vi "UHR-Fleezers Control (host) - 10.8MV_trial4.vi"() -> ()   [LabVIEW 2012]
uses:
  <vilib>/Utility/miscctls.llb/LVPoint32TypeDef.ctl
  <vilib>/Utility/miscctls.llb/LVMinMaxIncTypeDef.ctl
  <vilib>/userdefined/High Color/nirio_resource_hc.ctl
  <vilib>/Platform/TimedLoop/XDataNode/timing_clust.ctl
  <vilib>/Platform/TimedLoop/XDataNode/nitl_modes.ctl
  <vilib>/Platform/TimedLoop/XDataNode/wakeup.ctl
  <vilib>/FPGAPlugInAG/PCIe-7852R/niLvFpga_Open_PCIe-7852R.vi
  <vilib>/FPGAPlugInAG/PCIe-7852R/niLvFpga_Reset_PCIe-7852R.vi
  <vilib>/Utility/error.llb/Error Cluster From Error Code.vi
  <vilib>/rvi/errors/niLvFpgaAdjustHostInterfaceError.vi
  <vilib>/FPGAPlugInAG/PCIe-7852R/niLvFpga_Run_PCIe-7852R.vi
  <vilib>/Analysis/baseanly.llb/Mean (DBL).vi
  <vilib>/express/express analysis/Spectral/Block/exnSpectralBlock spectral measurements PSD poly.vi
  <vilib>/express/express analysis/Spectral/Block/exnSpectralBlock spectral measurements PSD WFM.vi
  <vilib>/Waveform/WDTOps.llb/WDT Append Waveforms DBL.vi
  <vilib>/FPGAPlugInAG/PCIe-7852R/niLvFpga_Abort_PCIe-7852R.vi
  <vilib>/FPGAPlugInAG/PCIe-7852R/niLvFpga_Close_PCIe-7852R.vi
  openfpgaref.8.6.ctl
  <vilib>/Platform/TimedLoop/XDataNode/XDataNode.xnode
  <vilib>/rvi/interface/nirviOpenFPGA/nirviOpenFPGA.xnode
  FPGA Bitfiles/UHR-FleezersInst_FPGATarget_UHR-FleezersCont_0F5B06C4.lvbitx
  UHR-Fleezers Control (fpga) - 10.3.vi
  <vilib>/rvi/interface/nirviMethod/nirviMethod.xnode
  <vilib>/rvi/interface/nirviReadWriteControl/nirviReadWriteControl.xnode
  <vilib>/express/express analysis/Spectral/XNode/ExpressSpectralMeasurementsBlockNode.xnode
  <vilib>/rvi/interface/nirviCloseFPGA/nirviCloseFPGA.xnode
  <vilib>/Analysis/NI_AALBase.lvlib
  <vilib>/Platform/TimedLoop/XDataNode/XDNodeRunTimeDep.lvlib
  <vilib>/vision/NI_Vision_Development_Module.lvlib
  NiFpgaLv.dll
  <vilib>/FPGAPlugInAG/PCIe-7852R/niLvFpga_ConfigureFifo_PCIe-7852R.vi
  <vilib>/rvi/errors/niLvFpgaMergeErrorWithErrorCode.vi
  <vilib>/FPGAPlugInAG/PCIe-7852R/niLvFpga_ReadFifo_PCIe-7852R.vi
panel:
  out "Location Matrix 3":string[][](array[string])=[["N.D.\r\n", "N.D.\r\n", "N.D.\r\n"], ["0.19233\r\n", "0.00156\r\n", "0.20615\r\n"], ["N.D.\r\n", "N.D.\r\n", "N.D.\r\n"], ["N.D.\r\n", "N.D.\r\n", "N.D.\r\n"]]
  out "Location Matrix 2":string[][](array[string])=[["N.D.\r\n", "N.D.\r\n", "N.D.\r\n"], ["0.19233\r\n", "0.00156\r\n", "0.20615\r\n"], ["N.D.\r\n", "N.D.\r\n", "N.D.\r\n"], ["N.D.\r\n", "N.D.\r\n", "N.D.\r\n"]]
  out "X Motion 2":string
  out "Location path":path=path "C:/Users/cwicker/Desktop/UHR-Fleezers Instrument - Charlie/Locations.txt"
  out "Location Matrix":string[][](array[string])=[["N.D.\r\n", "N.D.\r\n", "N.D.\r\n"], ["N.D.\r\n", "N.D.\r\n", "N.D.\r\n"], ["N.D.\r\n", "N.D.\r\n", "N.D.\r\n"], ["N.D.\r\n", "N.D.\r\n", "N.D.\r\n"]]
  in  "radius":i32=10 min=1 max=20
  in  "clear markers":bool
  in  "trap\nmarkers?":bool
  in  "Sample Channel Flow":bool
  in  "Pump 3 contents":string="Bottom: ADig beads" caption="contents"
  in  "Pump 1 contents":string="Top: DNA beads" caption="contents"
  in  "Scripts":T1(tab)
  in  "Take Stepping Data":bool
  in  "Got DNA bead":bool
  in  "Got ADig bead":bool
  in  "Cap 1 Flow ON":bool=TRUE
  in  "Move Cap. 1 (DNA Top)":bool
  in  "Cal/Data Acq. Spot":bool
  in  "Dump Beads":bool
  in  "Cap 1 T ON":bool=TRUE
  in  "Cap 1 Samp Flow ON":bool=TRUE
  in  "Offset 2 Set":dbl=2.0
  in  "Offset 1 Set":dbl=1.0
  in  "Cal @ (MHz)":dbl=20.0
  in  "W/ Offset 1":bool=TRUE
  in  "Offset 1 Start (MHz)":dbl=13.0
  in  "W/ Offset 2":bool
  in  "Offset 2 Start (MHz)":dbl=16.0
  in  "Pause at Closest Delta (s)":dbl
  in  "Move to Delta 2 (MHz)":dbl=41.0
  in  "Attempt Limit":dbl=30.0 caption="Limit"
  out "Attempts":dbl=1.0
  in  "Wait Before Save (s)":u32=1
  in  "Fish for Tether":bool
  in  "Closest Delta (MHz)":dbl=13.0 step=0.25
  in  "Stop F (pN)":dbl=10.0
  in  "Then...":string(combo)="2"
  in  "Move to Delta 1 (MHz)":dbl=15.0
  in  "Tether Alarm?":bool=TRUE
  out "Tether":bool
  in  "TA Cancel Save?":bool=TRUE
  in  "TA Green Off?":bool=TRUE
  in  "Raster Set Upon Tether":u32=1
  in  "Save at end (5, 6)":bool
  in  "N Steps":dbl=20.0
  in  "Step Size (nm)":dbl=0.34
  in  "Save ave factor":dbl=1.0
  in  "Dip Trap Delta 1 (MHz)":dbl=15.0
  in  "Move Trap Before?":bool
  in  "Save Data After?":bool
  in  "Green ON After?":bool
  in  "Dip Trap Delta 2 (MHz)":dbl=15.0
  in  "Move Trap After?":bool
  in  "Duration (s)":dbl=1.0
  in  "Dip for Protein":bool
  in  "APD to Watch":bool
  out "Duration (s)":dbl
  in  "Action":string(combo)="Yank"
  in  "Fl. Triggered...":bool
  in  "Fl. Delta Thresh. (kHz)":dbl=0.6
  out "Waiting":bool
  out "Fl. High":bool
  in  "N pts to average":u16=6
  in  "Yank Delay (s)":dbl=3.5
  in  "Yank to Delta Array (MHz)":dbl[](array[numeric])=[16.3, 15.85, 14.85]
  in  "N Array El":u8=3 min=1 step=1
  in  "Random Choice":bool=TRUE
  in  "Force Yank":bool
  in  "Force Reset":bool
  in  "Y change (mm)":dbl
  in  "Profile":bool
  out "Sigma/Mean 2":dbl=nan caption="Sigma/Mean" format="%#_2g"
  out "Rate sigma (Hz) 2":dbl caption="Sigma (Hz)" format="%0.2f"
  out "APD 2 Rate (Hz)":dbl format="%#_3p"
  out "Primary Video Display":T2(plugin-control)
  out "Waveform Graph":dbl[](graph) caption="APD Line Scan"
  in  "Inject Top":bool caption="Inject Pump 3"
  in  "Inject Bottom":bool caption="Inject Pump 1"
  out "Messages":string="3:52 PM\tUHR-Fleezers ready.\r"
  in  "APD Ave N":dbl=10.0
  out "Int. Time (s)":dbl=3.0
  in  "Stop All":bool
  out "Sigma/Mean":dbl=nan format="%#_2g"
  out "Rate sigma (Hz)":dbl caption="Sigma (Hz)" format="%0.2f"
  in  "Tab Control 6":T3(tab)
  in  "APD 2 Offset":dbl
  in  "APD 1 Offset":dbl
  out "RMS (Ang)":dbl=nan format="%_2g"
  in  "Bead Sep. Int. Time (s)":dbl=5.0 caption="Int. Time (s)"
  in  "Below (kHz)":dbl=0.5
  in  "Above (kHz)":dbl=2.0
  in  "Adjust Scale\nto Mean":bool
  in  "Rescale on Mean":bool
  in  "Offset (nm)":dbl
  out "Mean":dbl=0.003832945286164026 caption="Mean (V)" format="%#_3g"
  out "Force":waveform(dbl)[](graph)=[{"t0"=timestamp(68.39999999999971 s since 1904-01-01), "dt"=0.15, "Y"=[0.006501650011455353, 0.007613704960620254], "attributes"=variant("NI_ChannelName"=variant(string "T1 X"))}, {"t0"=timestamp(68.39999999999971 s since 1904-01-01), "dt"=0.15, "Y"=[-0.0011233638669916534, -9.306230558884231e-05], "attributes"=variant("NI_ChannelName"=variant(string "T2 X"))}]
  out "APD Chart":waveform(dbl)[](graph)=[{"t0"=timestamp(68.39999999999971 s since 1904-01-01), "dt"=0.02, "Y"=[0.0, 0.0, 0.0, 0.0, 0.0, 0.0, 0.0, 0.0, 0.0, 0.0, 0.0, 0.0, 0.0, 0.0, 0.0], "attributes"=variant("NI_ChannelName"=variant(string "APD 1"))}, {"t0"=timestamp(68.39999999999971 s since 1904-01-01), "dt"=0.02, "Y"=[0.0, 0.0, 0.0, 0.0, 0.0, 0.0, 0.0, 0.0, 0.0, 0.0, 0.0, 0.0, 0.0, 0.0, 0.0], "attributes"=variant("NI_ChannelName"=variant(string "APD 2"))}]
  in  "Calibration":u16(ring) items=["None", "Position", "Force"]
  out "T1 X":dbl=0.007057677486037804 caption="T1 X (V)" format="%0.2f"
  out "T2 X":dbl=-0.0006082130862902479 caption="T2 X (V)" format="%0.2f"
  out "Bead Separation":waveform(dbl)(graph)={"t0"=timestamp(68.39999999999971 s since 1904-01-01), "dt"=0.15, "Y"=[nan, nan], "attributes"=variant("NI_ChannelName"=variant(string "T1 X"))}
  in  "Amplitude (nm)":dbl=3.0
  out "Bead Mean (nm)":dbl=nan caption="Mean (nm)" format="%0.2f"
  out "Difference":dbl=0.006449464399747556 caption="Difference (V)" format="%.2g"
  in  "Take Detection Laser\nImage":bool
  out "APD 2":T2(plugin-control) caption="APD 2 (Cy5)"
  in  "Flip Green Filter":bool
  in  "Set X Only":bool
  in  "Set Y Only":bool
  out "APD 1":T2(plugin-control) caption="APD 1 (Cy3)"
  out "Detection Laser Y":T2(plugin-control)
  out "Pointer Y (V)":dbl format="%_3g"
  out "Pointer X (V)":dbl format="%_3g"
  in  "Set Confocal Spot (X-Y)":bool
  out "Detection Laser X":T2(plugin-control)
  out "Saved APD":dbl[][](graph) caption="Most Recent Time Trace"
  out "Trap Delta Graph":dbl[](graph) caption="Most Recent Time Trace"
  out "Save APD Deriv":dbl[][](graph) caption="Most Recent Time Trace"
  out "Delta Fl. 1":dbl
  out "Delta Fl. 2":dbl
  out "All Signals":waveform(dbl)[](graph)=[{"t0"=timestamp(68.39999999999971 s since 1904-01-01), "dt"=0.02, "Y"=[0.0, 0.0, 0.0, 0.0, 0.0, 0.0, 0.0, 0.0, 0.0, 0.0, 0.0, 0.0, 0.0, 0.0, 0.0], "attributes"=variant("NI_ChannelName"=variant(string "APD 1"))}, {"t0"=timestamp(68.39999999999971 s since 1904-01-01), "dt"=0.02, "Y"=[0.0, 0.0, 0.0, 0.0, 0.0, 0.0, 0.0, 0.0, 0.0, 0.0, 0.0, 0.0, 0.0, 0.0, 0.0], "attributes"=variant("NI_ChannelName"=variant(string "APD 2"))}, {"t0"=timestamp(68.39999999999971 s since 1904-01-01), "dt"=0.15, "Y"=[-0.02616851084212992, -0.0255133251155073], "attributes"=variant("NI_ChannelName"=variant(string "T1 Y"))}, {"t0"=timestamp(68.39999999999971 s since 1904-01-01), "dt"=0.15, "Y"=[0.006501650011455353, 0.007613704960620254], "attributes"=variant("NI_ChannelName"=variant(string "T1 X"))}, {"t0"=timestamp(68.39999999999971 s since 1904-01-01), "dt"=0.15, "Y"=[5.238432721945855, 5.23694863734855], "attributes"=variant("NI_ChannelName"=variant(string "T1 Sum"))}, {"t0"=timestamp(68.39999999999971 s since 1904-01-01), "dt"=0.15, "Y"=[-0.011935220655057682, -0.011271872990085285], "attributes"=variant("NI_ChannelName"=variant(string "T2 Y"))}, {"t0"=timestamp(68.39999999999971 s since 1904-01-01), "dt"=0.15, "Y"=[-0.0011233638669916534, -9.306230558884231e-05], "attributes"=variant("NI_ChannelName"=variant(string "T2 X"))}, {"t0"=timestamp(68.39999999999971 s since 1904-01-01), "dt"=0.15, "Y"=[5.494853022858362, 5.494846064638206], "attributes"=variant("NI_ChannelName"=variant(string "T2 Sum"))}, {"t0"=timestamp(68.39999999999971 s since 1904-01-01), "dt"=0.15, "Y"=[0.28818490745989345, 0.2884769879609513], "attributes"=variant("NI_ChannelName"=variant(string "T1 FB X"))}, {"t0"=timestamp(68.39999999999971 s since 1904-01-01), "dt"=0.15, "Y"=[1.7389615771965699, 1.7392489089632854], "attributes"=variant("NI_ChannelName"=variant(string "T2 FB Sum"))}, {"t0"=timestamp(68.39999999999971 s since 1904-01-01), "dt"=0.15, "Y"=[0.33831454944946326, 0.3385055215953781], "attributes"=variant("NI_ChannelName"=variant(string "T2 FB X"))}, {"t0"=timestamp(68.39999999999971 s since 1904-01-01), "dt"=0.15, "Y"=[2.000203253273112, 2.000828547013765], "attributes"=variant("NI_ChannelName"=variant(string "T2 FB Sum"))}, {"t0"=timestamp(68.39999999999971 s since 1904-01-01), "dt"=0.15, "Y"=[-10.000305185094591, -10.000305185094591], "attributes"=variant("NI_ChannelName"=variant(string "PSD Y"))}, {"t0"=timestamp(68.39999999999971 s since 1904-01-01), "dt"=0.15, "Y"=[-10.000305185094591, -10.000305185094591], "attributes"=variant("NI_ChannelName"=variant(string "PSD X"))}, {"t0"=timestamp(68.39999999999971 s since 1904-01-01), "dt"=0.15, "Y"=[-0.0074939725943783285, -0.007506576738791921], "attributes"=variant("NI_ChannelName"=variant(string "PSD Sum"))}]
  in  "Signals to Plot":i32(listbox)
  out "Trap Disp. Freq. (Hz)":dbl=6.666666666666667 caption="Freq. (Hz)" format="%#_6p"
  out "Display Period (s)":dbl=0.15 caption="Period (s)" format="%#_6p"
  in  "Trap Disp. Downsample":dbl=10000.0 caption="Downsample" max=20000.0
  in  "APD Disp. Scale":dbl=0.1 caption="Scale (Divide,\nfor above plot only)"
  in  "APD Disp. Downsample":dbl=2.0 caption="Integrate" min=1.0 max=30.0 step=1.0
  out "APD Display Freq. (Hz)":dbl=50.0 caption="Freq. (Hz)"
  out "APD Display Period (s)":dbl=0.02 caption="Period (s)"
  out "FFT 1":cluster{"f0":dbl, "df":dbl, "magnitude":dbl[]}[](graph)=[{"f0"=0.0, "df"=16.666666666666668, "magnitude"=[-331.1367572010275, -79.05506245821404, -86.61411242440559, -88.4728176091699, -90.3181253945935, -94.12566333707997, -92.52740723119955, -94.92192587982518, -99.60936585245742, -96.87568627870715, -94.02570383337763, -83.8058550151726, -97.57441397235512, -101.59968530846606, -101.523049255742, -103.35038532190343, -101.58594091014982, -102.96098031851216, -91.39759462745924, -103.75019963279499, -104.45030075054324, -103.04245334279298, -104.0720279134107, -106.06482372394834, -103.69131867828104, -104.40395035115309, -105.96420043276396, -107.6735556337804, -106.673030006608, -107.34889066208132, -108.05626565233933, -106.25659018850432, -105.29934513380842, -105.43096056709592, -108.3728498841465, -106.0555440144992, -105.78001282181421, -107.48741857324953, -108.67624970548897, -105.39976667156175, -105.91413119232612, -109.4222808198164, -107.0898971593174, -107.91164191890915, -108.26032038855709, -107.58332347164534, -108.23559688234297, -108.01271040303237, -107.66511723652701, -106.51901583170391, -109.27249501469946, -108.55647681594805, -107.93499259231463, -107.05068166453935, -109.13641475410455, -109.29679733781423, -108.19360835527803, -109.57747591546632, -109.58364591011674, -110.47061433372711, -109.8144340420426, -108.79067462293897, -107.54887553357234, -107.99559866705923, -108.85023923652685, -109.68733225238618, -108.51101278437793, -108.51620475114115, -108.22212402200637, -104.63726950302143, -110.2989919678048, -107.61796444414897, -108.68882962798736, -104.79193983043893, -103.59504263746938, -93.64633660288543, -101.9191640501395, -105.73717393151816, -108.92572458793902, -107.43962662800902, -107.79595323081325, -107.0923101993207, -108.17603277205289, -107.87074270713183, -109.20899066381877, -108.61832060412445, -109.10072003106593, -105.76480632823524, -108.60877649218978, -109.67541158970121, -110.2286232768028, -109.84952155309578, -109.33772024076384, -109.95251642394683, -110.14777282585466, -109.13825677905699, -110.05989365698167, -109.39359990189426, -110.56255614635295, -109.66477183197163, -108.9397158528824, -110.26529907650465, -109.20049464984628, -108.20183857013548, -109.09752250184418, -108.00440442238454, -108.35465963524055, -111.16774134451799, -110.34812550238405, -108.94506763426756, -108.72845542102493, -109.41512344014713, -112.44661664432377, -110.35437330889101, -111.32939440655925, -109.42989530434981, -110.98084669076195, -111.92160561143541, -108.57755551751093, -111.40042616180912, -110.15284955891853, -112.21455132279115, -111.40787773511747, -108.82949641635288, -110.13442122547907, -111.42229298204664, -112.06314940885191, -110.6015308813694, -109.51144097251623, -111.15989713761475, -110.25535755335385, -109.65868178057926, -110.51649885452997, -109.77194745285269, -108.4234206864394, -109.50892632093968, -109.46471287444389, -107.92241289271415, -109.72283805386196, -108.63426821579918, -110.37316681536255, -111.09713996884652, -110.32903619589223, -105.32012665515045, -107.36858557554393, -108.00382215905725, -110.06430686942338, -108.81666625979916, -110.01277074453823, -110.94194741225512, -109.65934609082873, -107.80979136006962, -112.81333866824724, -111.61474300955487, -109.83998277184975, -109.45953946904639, -109.79640584952526, -108.19172301667324, -109.28894656674316, -107.61471301278785, -108.83814006090513, -109.08866847726084, -108.20250571862371, -107.96222236861584, -107.03811197900873, -108.93533000393974, -107.74482548035408, -110.79811544577694, -111.1387476496877, -107.42970105883512, -109.18442281176472, -108.73546184641192, -108.71800246690864, -108.51945944378063, -108.06825856571285, -107.27210712368412, -108.12304695877637, -107.84933283677306, -109.73682373154998, -109.32284761503395, -109.31328817453769, -106.68762108642842, -109.79203616876461, -109.9020278896408, -110.27080024357275, -108.54152101558762, -111.00464391726017, -112.42244020766577, -110.82707315747889, -111.00344011890857, -109.90461839395674, -109.42877207451863, -109.73549298167016, -111.67494793393293, -108.85799077901427, -108.5348443278263, -109.803781083881, -108.30644755543659, -108.5079527456017, -111.2055351312823, -108.53089994340155, -108.01739789012176, -108.70360662855235, -107.95873456794631, -109.58297170693093, -108.9372401694271, -110.15921663527153, -109.22399119911955, -110.89883651739237, -108.92840112258382, -110.0545300523626, -109.05961065387005, -109.45831398589371, -108.61239387653227, -110.13001256174265, -108.80060224137931, -109.46327400696283, -108.0177965824709, -109.29727944627197, -110.3237255895986, -109.03258262543821, -110.97880178489321, -109.70034895077919, -111.16405638194153, -109.17324451464711, -109.65698250854277, -108.96750235822178, -112.00534231585624, -108.69274607723942, -108.98110446396657, -108.40723795464795, -111.44459094807324, -111.74799245277113, -111.1601960491512, -108.92048232753773, -110.30506377784799, -111.33145973979093, -110.91850998672503, -110.33684985776448, -108.90206518366908, -109.28458878227542, -108.98773986023751, -110.85813863075646, -109.00041591105906, -110.84543686681204, -109.84382395806176, -109.69722434763266, -108.50915601095721, -107.80829925826895, -110.59736107582401, -109.75377770317087, -109.3992084496136, -110.51151565846742, -112.49753959826434, -109.7299632589479, -109.54070743868353, -109.90314341132164, -111.05974202976806, -109.03766862152392, -109.46667095459878, -109.52800799036197, -111.3163121356807, -110.07817134522178, -108.69251657453547, -109.40472158898045, -109.71400709815576, -110.60534468715097, -109.46937396724682, -107.70342491418788, -109.86331122597839, -108.64971387994616, -110.90117371097081, -108.34928840565928, -110.04172889660904, -111.52979926554961, -110.34759300823305, -109.62712781837159, -109.24131154553284, -110.23196152450447, -108.68509612326807, -108.0246905483419, -106.61876139289784, -101.5519630114271, -80.57695480953835, -102.03744443354402, -107.1449217193017, -110.0695213407169, -106.61597783999268, -110.79221011808191, -109.58974545931426, -109.1149802216988, -109.20993813088597, -109.63768480465863, -110.10428394219181, -109.08445084271477, -108.83472375362581, -109.69508502050168, -108.05588796178941, -110.62586360101581, -109.95315261676905, -107.52208264977473, -108.80708007514875, -110.43484881098874, -110.45942171588936, -107.83804717866751, -109.98973910294193, -109.3496496054193, -108.425252911127, -110.94579264380809, -108.54181722177951, -108.67696070083541, -108.4150202151644, -109.24973583101504, -112.0454922608961, -111.29046597340738, -110.75018248960077, -109.38326363603683, -109.2033340336957, -109.45076170874889, -109.52878049853727, -109.32340869724774, -110.98123395128233, -110.75736340635505, -109.7218385823809, -107.97422606064993, -109.77313701758703, -110.95948744392717, -110.08996774172691, -108.51011830110778, -109.78063140243836, -110.65996628628228, -109.83684298615616, -110.33329049188029, -110.13755118968292, -110.3717925645783, -108.55302219178951, -106.86811628734195, -108.6302156589162, -108.75341391045045, -108.32589578384841, -108.70061474734084, -112.30742263527534, -109.16842570592085, -109.29767035534508, -108.87829025017463, -108.2255616391397, -108.4316108616088, -108.82995906929271, -110.40135575415563, -109.51623498946435, -109.79409808792403, -107.03832759632121, -108.36534528684132, -109.72010868372905, -107.90933028179892, -106.95643597294047, -111.29929166165778, -110.23001135794706, -108.98838015381585, -109.79115357104436, -108.18627479511115, -108.14988122174307, -109.12074063466532, -109.41904850488358, -111.40409873721113, -108.83156790193294, -108.77032248953847, -108.88363158686694, -108.47515048290681, -105.94172147874599, -109.38146940214403, -109.21277078848794, -108.11309390545507, -110.70840012427504, -109.5504457849329, -109.52330684534209, -110.06776026911132, -108.21949434182314, -111.21266686269992, -108.78581501170974, -108.43115799297222, -109.63260325780062, -109.84070220619535, -109.72041980780126, -110.29615941882527, -110.60316734262464, -108.79165446414692, -110.95840439895592, -109.64926233107009, -109.16526769544322, -108.65292362430982, -109.56113898129935, -109.85693046339026, -108.92316027325207, -109.79492493553914, -109.38157962945887, -110.24545136266825, -109.30031463492487, -109.0795429936869, -111.4091719525013, -108.63499083917162, -108.43863465339358, -109.23207864880891, -111.21947487191643, -109.24525201480154, -109.56842406077318, -109.46711940800672, -111.91389548262572, -108.15655736690546, -108.71882059966947, -111.26328503478568, -110.95027143873176, -108.4853106242357, -110.36902802777546, -109.9314203579182, -108.77686164101732, -108.71871020068312, -111.04829661168574, -109.95072655339462, -109.88221342875462, -109.53241732756136, -108.2625005404823, -108.00677030040697, -110.19659317581693, -108.93858924796267, -109.46817875483995, -110.78063992017232, -111.11066570318451, -110.78774336696706, -109.19199744617812, -108.54914256407436, -109.28414960420909, -110.64143585101183, -110.5855350821307, -109.47578632252726, -108.89705360836223, -109.89214013612292, -107.93271261027171, -109.32631601340563, -108.60274611341092, -109.40110159872573, -110.889237682208, -110.01391165813328, -109.99747108785071, -108.65542819213674, -110.37211847668736, -110.44656500845738, -110.8128133834973, -108.8909299260433, -110.19551227077532, -111.37647266643523, -110.83802189730321, -109.98519377913681, -110.52378970770522, -108.16970420057817, -110.70974729773344, -110.76836765494402, -110.26884275594577, -109.22041044268806, -109.87809744746195, -107.76823252107832, -109.12119474042969, -110.28066108731146, -108.55000033509207, -110.18152097767907, -110.73030521152278, -111.49470908029893, -110.2320929919509, -110.03370979233021, -109.79181668155233, -108.6673501209991, -109.86695766650877, -107.88926518046961, -110.95525003776572, -109.18130359755742, -110.42618009658618, -107.90341931158893, -111.44736855661769, -110.72634267386593, -109.29945988519303, -107.67889101961411, -108.81148059987765, -109.13375212757057, -109.8122873383549, -109.80176697684155, -109.96342275204768, -109.90406635707086, -108.75674342748256, -110.12362902701081, -109.82151095527837, -108.62543344241836, -110.09171852771195, -110.21434637862887, -109.97254504855631, -109.27043209093468, -111.35149588204125, -110.12399876776051, -111.65983675538546, -109.28788875768564, -110.86554069990251, -111.26990906470603, -108.60956517491746, -111.49613890850938, -111.79685722966795, -109.26269485364045, -110.38555615546439, -109.40641023162068, -110.966136593156, -108.78892524584494, -110.29340727375603, -111.44032043281035, -109.95212021173755, -109.79233511584334, -112.41184021118175, -109.73687851881148, -108.65493879781806, -110.76132988919045, -108.43230346094671, -110.32968175895853, -110.29890782023821, -108.77609076424456, -110.3298662333555, -109.47734504217333, -108.2677295732245, -109.21234363352882, -107.83278941978479, -108.85136784424789, -108.43241251530755, -109.76609391460555, -108.53204373005357, -110.9660641972934, -110.3152512161094, -110.72570499399905, -109.23877906286317, -111.72407743101837, -109.20311421918561, -108.06021800233717, -109.29288625761943, -108.78395253409145, -111.85250172876302, -108.78827588901797, -109.79775055719482, -109.12089297455859, -109.49896359356035, -110.34432647103819, -107.94700097960238, -109.30489238477631, -108.89170290869342, -108.82574563272509, -110.11024077194833, -107.37946433552314, -109.60167933458756, -107.80625057819019, -110.11489057210264, -107.35436859378505, -105.69819484613895, -109.11280625683739, -109.27770293057978, -107.7053735252589, -109.75022444894368, -109.3310543596577, -107.87683693707739, -108.19931495338068, -109.26462246191564, -106.71885779297867, -100.00018022217961, -92.54434511397295, -107.20472143807373, -107.39203415155283, -110.04461177268398, -108.48860496315312, -109.0057168110333, -108.37627790492552, -108.4108380728248, -109.65509454313073, -109.64243000632982, -97.04219069306761, -109.0928856629964, -107.9760697315632, -107.52611064047497, -108.87702814778996, -109.08437599027614, -110.70097118837974, -109.00969860961283, -110.38275386163214, -110.0699155421545, -106.91498895181175, -106.22178738309017, -109.36827866896039, -107.59953130968307, -109.19516217272808, -108.31502495393616, -109.384158926223, -107.11670654202719, -108.09436312738853, -110.14559230873704, -109.84997663447679, -107.83465335309926, -108.60947100624459, -108.9932479423645, -109.17174810371898, -108.79457339828916, -109.40909327982367, -109.6328723628302, -109.51081854476179, -107.63054408568418, -109.63728404010122, -108.51163794839918, -107.55002282725216, -108.97796212764939, -107.24648164623483, -112.21470452291085, -108.74294024554423, -109.62070777514892, -108.05768666239368, -109.8224946685739, -109.34575507446003, -108.53536952609525, -109.60789300457671, -107.56681538208278, -109.22777325016398, -108.79047910308894, -110.10332477250668, -108.00206387955672, -108.45604004720035, -109.00645795765472, -109.81039564269616, -108.92785144634745, -108.3978471520567, -107.94411095685999, -110.53486519304262, -108.8773780319227, -109.03345093296107, -107.30746693745031, -108.54277704832029, -108.77629108166091, -108.91111762599647, -107.74965195880401, -109.97375370738439, -109.76326492689246, -107.91717581777407, -109.0730556927617, -107.66804873204664, -110.40438871064791, -108.05794247751498, -108.80206615156494, -107.51329354700796, -108.83687012994949, -107.57713176895379, -107.94774159581414, -109.41894615439651, -107.10869425078764, -110.51480854078629, -108.92221367099775, -109.91358786461535, -110.1744263092835, -109.30795472883494, -107.91359710691006, -109.77888185049835, -109.52060975706438, -108.66686651982212, -108.71041801553639, -110.13619546359467, -108.87957097273856, -109.72150387215271, -109.00776068810654, -109.70251113927438, -110.75769213896399, -108.53234896741436, -109.69439526582246, -110.15412541604617, -108.25183374628219, -107.97402569656481, -110.34920156998648, -108.45106995186384, -108.82031145748209, -111.38690005057539, -107.01968459818563, -110.3044500039584, -110.8755481852125, -111.08915057663255, -107.94824988655199, -110.21669144934839, -109.90539774633154, -109.58985438756767, -110.12258796623348, -109.41689951612143, -109.31128210476795, -109.00258476567323, -109.11093063041056, -108.83347064311234, -108.32685287566952, -109.44770946560935, -108.40145063144861, -109.68448193892085, -108.76525439243828, -107.62837139034596, -107.39300298848994, -109.36993934990318, -109.2465218489418, -106.66307369796812, -110.15891092764934, -109.57151745419041, -108.92425698310808, -109.8036704717834, -108.79751146756549, -109.25926431818017, -108.46260574057584, -109.1967554647261, -110.63319560262356, -109.02343067385144, -111.22073171487528, -109.4731095097105, -109.69335000085164, -109.48782989577005, -107.95204227683271, -108.19468255763758, -111.36195112053247, -109.55696116543685, -110.3130767640534, -108.9621824253354, -109.99735074896789, -109.20198058456344, -108.12100614259485, -111.27227490807289, -110.09248554008288, -109.14395535060149, -110.80882692379708, -109.22632926901655, -108.64497210802793, -111.00030482190711, -111.1317849358033, -107.43140429257826, -107.9783302193555, -109.2639893652291, -108.97008485446163, -108.66556668859064, -108.12995785876932, -109.73001061107855, -108.09691302413727, -110.68391499215569, -112.78583642012705, -108.7093037763389, -110.67868795924797, -109.0190959349128, -108.36247198231372, -109.82829353258869, -108.24916379311045, -109.84154533905823, -108.55470160833775, -109.75438989348815, -108.82865632118325, -107.63622268162582, -111.00943492886312, -110.81824358463759, -109.46028423652966, -107.52479398900992, -108.99087806823736, -109.94494831750349, -110.26788355564504, -109.8954055022304, -106.9478122391182, -108.91705388158901, -107.76095584490312, -109.28456723055147, -109.7982307261767, -108.98552661346622, -109.98937979783426, -110.57907422426224, -108.68113463944836, -108.06257240208589, -110.0707224529617, -109.19515280354733, -109.35868842818849, -110.37311467065695, -109.0404734478992, -108.16686395270187, -108.61859220485148, -109.19986437876149, -108.19707189725302, -110.06564239663074, -108.87850403465154, -110.63824157544798, -107.36918104067212, -108.7008736325543, -110.9359398265406, -111.08529123080929, -108.44209934821818, -109.79529621208783, -108.38917887958179, -108.169117639508, -109.24332926356216, -110.50584058811704, -109.63592524002665, -109.32261039377495, -109.16720880524552, -109.3084314664462, -109.5812223978583, -107.70213196487856, -108.0557884982431, -110.67058020007828, -111.68459781023608, -109.66270627185824, -110.52536245663693, -109.70208409132103, -108.78645420809342, -109.23122088059863, -109.24601474121832, -111.25604763816514, -109.50225851581177, -107.32434217163818, -109.28548556764925, -107.59972621660836, -110.46928774723048, -109.25950101547609, -110.32016453935465, -107.78482761561703, -107.89462895091089, -107.51366154391481, -108.08036891159172, -109.53371809947035, -101.2452927166745, -109.32763325689056, -107.52166868423687, -109.89648659445174, -109.11350200980485, -109.81336712738089, -110.02799517445062, -108.02767143538516, -107.97850220501483, -109.50772934896838, -109.31069875721964, -108.49991657749598, -105.60880911233095, -109.79128597340213, -106.91084537903113, -107.84880087118997, -109.63628170511824, -109.03203967193224, -110.64186113413658, -110.98027990365594, -112.33841002907062, -111.01793075565425, -108.58025797022215, -110.4259296883756, -110.38643255981424, -108.93051671115133, -110.97544177116494, -108.63883100482677, -108.37581711765226, -108.90240163126536, -107.94688047875466, -109.9482937437732, -110.09097112364414, -110.09805032265376, -111.44307114024532, -109.15483789122554, -110.9713708217832, -107.8548737634672, -111.41418477109195, -109.45699779859628, -97.03595099331734, -109.16746744169623, -109.66209204485918, -112.57048704774604, -109.73989735035725, -108.16252575067017, -110.7546980664636, -108.91536673403449, -109.20509151422344, -111.0260632167785, -109.62924582406518, -110.45466277291722, -110.2973970018937, -109.67550222925419, -108.84481022020094, -107.23686414357573, -111.79004633370906, -109.85453094194085, -109.45617270081004, -110.73920606732504, -108.90879956851099, -109.67774425528265, -109.4745715721361, -110.18080454693559, -109.26079184315502, -109.41692499885505, -109.02240975088358, -107.80833423058168, -109.32657361431549, -107.87138278655101, -110.910364670719, -109.70067156846706, -108.55301754282077, -109.4243252157005, -109.77567725161107, -107.83737232063925, -110.36509412773016, -109.6371048811367, -109.49430894422814, -108.55509251499753, -108.03996302911446, -110.4385715838736, -110.08864436068788, -109.48922484379962, -109.90865554258562, -109.7491963238264, -110.04796094537969, -107.413043439116, -108.54229076126079, -108.2522516728666, -109.75464941327974, -110.26795832300996, -109.28073673851144, -108.62990200974927, -109.89408067552287, -109.09160284731726, -109.90740624925795, -109.92534708896517, -109.79578862362752, -109.97278346890566, -107.80679350393824, -112.81728446281548, -108.09689504419987, -109.89549991422173, -108.43930976031248, -109.95153099843282, -108.18277483720716, -111.89607792605433, -109.52567003805, -109.17125106979698, -109.64300739407085, -108.21045178846524, -109.64036472149706, -109.02324448538845, -109.039163008889, -110.41006510134076, -109.50289952116489, -110.4732620447796, -110.08777181504614, -110.15589511434341, -109.55705089158471, -109.2547682932589, -110.86823885471617, -109.96330502176939, -109.85995369810554, -110.63211290903473, -112.08007783432191, -110.24725218052279, -107.62861148917592, -110.08691795849435, -108.89793794632287, -111.07702220466341, -109.46946126482341, -109.19747345337464, -110.70018609416007, -109.66366205691908, -110.78032312133551, -108.05724200456513, -108.195661625627, -110.90724508408255, -110.08307674771669, -110.76863516643007, -110.46620425061583, -109.16986788877276, -109.61921294239114, -108.51159432329543, -109.96308336765689, -107.38178944242856, -111.95930944846394, -109.3329826827624, -109.59119636368249, -108.83148571828912, -110.46194288788257, -105.87694286145472, -107.985886302892, -109.2975019660806, -111.05138725716857, -109.60005889204612, -110.92871351729086, -110.73480546964537, -108.41587420326718, -109.84275465824477, -108.8249071047676, -107.65358887817105, -108.3254150042995, -111.47362100321767, -112.7287536850025, -108.8217125660507, -109.50232320231771, -110.29587061625348, -109.30644535112089, -107.69178032077258, -110.84522325672016, -109.3735891463141, -109.12506388923123, -109.65582307934665, -111.11427272192576, -112.19827973435466, -109.11306367925813, -108.19203577968261, -107.89831568266465, -108.85805249169313, -109.51100049661844, -111.71546684086955, -109.53880495724334, -107.07739286222231, -110.66836728754211, -111.5415170557177, -110.16051267940297, -110.6107546662698, -111.36389129556191, -107.77888179117923, -110.34160392509817, -109.61287125994414, -110.23791773883013, -111.00669159903549, -110.97165069538953, -109.43965413392434, -110.6813161690388, -110.31441293654314, -111.96129906273796, -108.15998218707462, -110.08095912053633, -109.41084567452768, -109.28774416263552, -110.80159950384204, -110.41956747809755, -108.85005186267244, -107.9069227847757, -108.84249369063123, -109.92569208845894, -109.34109797584448, -109.41334788055491, -108.76462023086997, -108.22069272136177, -107.0786679601274, -108.30206755098202, -108.57613406368954, -110.83330887636482, -111.93966942736989, -109.76373713473264, -108.25782074884941, -108.16490627215555, -109.93351470267982, -110.75525684428368, -108.22814762283093, -109.73442331991602, -107.53145627482685, -108.27195221226805, -110.33032779278457, -109.48951857415828, -108.12599093700939, -107.97627415508097, -108.81426859968796, -111.21764717894752, -109.80856212352333, -110.92658779118501, -109.71551885834796, -110.38682741010847, -108.87671328341361, -109.68368600774755, -108.35359806351899, -111.7519400010676, -109.89407081573103, -108.24301180922755, -110.00646944788126, -108.6685299083706, -107.52856885980722, -111.7622363038509, -111.0025144494897, -108.64719599357296, -110.62968467177518, -108.821509935539, -107.94915453463719, -111.53070432277694, -109.87282048586256, -110.71167589371663, -109.79225006081626, -109.96203471712074, -110.29921092232489, -110.10644439440416, -111.28815007382043, -111.19165661703703, -108.46024117100558, -110.22528296512183, -110.32184972386672, -110.05120383416072, -109.78792549362107, -109.00355659956696, -108.85989369286315, -113.00899556732638, -110.91756826567867, -111.25016866167897, -111.84225040552181, -110.54451635944174, -110.72722829912917, -109.60759702177283, -110.49362602516815, -108.74419542915284, -110.3379671069179, -109.66259088220754, -110.45956400953156, -109.13956157147233, -109.27130155486806, -110.83015602667983, -109.17970724944131, -109.09662765889193, -108.0447366108107, -108.9536269357457, -110.35663108940085, -108.73418835472056, -113.42965806805827, -111.81270536656905, -110.06155590173537, -108.76582224646269, -106.7488061675813, -108.5700320158723, -111.11038264410035, -110.41435767488723, -109.12763443489911, -109.30517580756394, -111.61251165371237, -109.8116632664339, -109.36845864976851, -109.00390009629231, -110.54359197165573, -109.52629258465976, -110.75932197632896, -109.50903215359567, -107.42652056246085, -107.81146496533543, -103.22224383145215, -108.53803076819163, -109.78623360072066, -109.66306634612869, -110.80245829141279, -111.87835085452016, -102.27372781471168, -111.27763038431458, -108.45838423437681, -108.79077917058028, -109.31951755762685, -110.05415097017186, -109.5535934823387, -111.62732254641111, -110.73478247119641, -109.9468722686683, -110.39698367573979, -109.30612942398305, -109.7578384694043, -109.34817295524313, -105.56944757301993, -110.1940418750125, -109.27076023513962, -111.03491935225027, -112.2980497521063, -110.65725497955563, -109.0567530102422, -110.31700596563523, -109.64508026365678, -109.6190471404421, -110.52566833759428, -109.68595899227789, -109.7431160985074, -110.4798230300751, -109.45506977604765, -110.69504157940786, -110.63067849573177, -108.06456949500138, -107.99354148885966, -108.11349194720599, -109.15944121207349, -110.61766925164031, -110.14145801314527, -110.67420842201165, -111.91532881806512, -112.15901550030345, -109.94774413630104, -109.2819568305201, -110.94623189179737, -110.17685430287735, -110.39082916961016, -109.53953238698966, -110.76940623620611, -109.89327922318515, -109.10275695043765, -110.21445972656734, -110.58968777252528, -110.57016757660259, -109.59208496373341, -109.07946946465374, -109.10762003745964, -110.36892993974607, -109.81864495218393, -112.12972189864566, -109.26185849434863, -111.56305819991357, -111.36019621828058, -110.3397604159226, -109.58675612753163, -110.58041217474447, -106.34739062044932, -108.6722699609389, -110.03906060709869, -109.16794717548382, -109.65012481802809, -109.35377624077988, -110.51889143862303, -110.03397458059777, -110.7981307056636, -110.56653507062292, -107.61367005067231, -109.99279736988825, -111.79875182878175, -108.60382315996031, -109.71381533228038, -108.60388131505613, -107.0933685540362, -107.86037690830757, -108.40980028847238, -108.83869602763895, -110.76921375395764, -109.96766364716046, -110.8256171465781, -110.13805084291067, -108.5349140035878, -110.57158437465219, -110.8920694413417, -108.71646695477324, -108.33274238445665, -108.96152108305608, -111.03750932994224, -109.48915027983756, -110.29725207211165, -110.79527247268442, -109.47969936716117, -109.79306701834035, -110.16840035577498, -110.29840230783668, -109.15306387075587, -110.72651274964761, -109.08881658764956, -110.8349724030761, -110.64653625576447, -111.40392562616867, -109.94581588927414, -108.85136340231294, -109.77228546607624, -111.48297395390018, -109.7334001251941, -109.30537415590783, -109.63937411233408, -109.69785848648013, -109.3523781030017, -112.04667421182404, -111.56311816195343, -108.18548447362308, -110.63388993686104, -111.39768634137992, -109.87157345395542, -108.6734208287271, -109.46213300216168, -111.75774769437145, -110.10245994173216, -109.52385139033495, -110.96513097775451, -111.8709319163154, -111.54948269614047, -110.29760900080463, -108.52168175904663, -111.09033925738258, -111.14752744054172, -108.83074523709202, -109.05704141259113, -111.74377805749482, -109.57200906899736, -108.84121318623825, -110.86657990204343, -109.54363603755047, -110.89448416316372, -109.58965570570145, -110.21012263847972, -110.4063470702923, -109.5021950342969, -110.33648801598177, -110.90551031296536, -109.69205870504638, -109.8648503154861, -110.28183391384131, -109.65970942950766, -108.43615680946908, -111.11790511866548, -110.89043476451553, -113.64898442872548, -113.08004494963895, -110.81525412051718, -113.91009875719509, -110.95802128672312, -110.40944585634135, -110.33464695414992, -109.98984645778987, -110.18795067005652, -110.62364351231234, -110.44029833291248, -109.01598585569788, -110.95430216511514, -109.77987141110621, -108.54452361812068, -111.41780266439777, -110.47172771858405, -109.06084635984516, -109.30794593246578, -108.8764083815745, -108.18222749506985, -110.31330487887435, -109.04176821738014, -108.8558386035048, -109.47888284507395, -110.01459604573937, -110.48596659065309, -112.6781342298378, -109.85522803775775, -109.0569534499285, -109.08991286548698, -110.89485727880403, -109.18715778948663, -111.50381433568144, -111.3545424730884, -110.07710926239977, -111.99977850157067, -109.47444853853723, -109.81605328527645, -110.74995213151195, -112.56834665925544, -108.52052472391404, -110.89121213995557, -112.02004142355113, -108.66413739656008, -111.10053848695652, -110.41241079991636, -111.80152991764473, -110.21746151515111, -110.63265128607344, -109.483042128511, -112.78639954059729, -109.47114195846122, -109.23309637902875, -108.97133643967169, -110.08909147812822, -111.01105271457081, -111.18602432128249, -110.04633990216801, -109.53453538673071, -108.81939452082017, -111.13486114285661, -111.65877073200598, -111.63763706753498, -112.14107810664572, -113.6231865196724, -109.31743865878806, -109.18551713085722, -108.74951309653638, -109.28206426212142, -112.36687029711229, -110.10933061193728, -111.29501093502684, -108.19021080564794, -109.34497312126749, -110.37228033937312, -108.63277512903049, -110.61033993911002, -111.2975761598062, -111.49780004751436, -109.91019436685814, -109.32789992989028, -111.4482538110117, -110.1538439123475, -110.66347034043578, -110.05055133068794, -108.53002033538341, -111.7522199783972, -113.49108651193104, -108.03793940563418, -110.07108694011555, -110.83958739865201, -109.62805629409038, -112.69637731014087, -109.57996950503268, -110.104850643722, -108.83376203949506, -108.69400304840181, -110.59434352922563, -110.69121011800921, -110.18694553784364, -111.90598571547098, -110.30230802494223, -109.66810649416752, -112.6017099000434, -111.00296745333219, -110.64462650261785, -111.4775358707403, -111.98753241268494, -112.26574909791167, -112.04796822399412, -110.65853064447325, -109.6623218025264, -109.40559579075378, -110.42174451813142, -109.18991987957241, -111.02050178263048, -112.77950487440032, -110.42443751566815, -111.35440372400903, -108.5263524245987, -105.07498063939795, -107.15444425741984, -110.4508720018025, -110.25163264819463, -111.1383261104107, -109.91171620173931, -110.52200560606038, -110.5299174299573, -109.34628087255733, -110.26101817411786, -109.65071853372183, -109.66953335961068, -110.83590602054682, -110.980546313788, -109.4110066989163, -111.47223607390256, -110.00281523859483, -109.4088722967626, -109.00401922839337, -109.59655302543185, -109.7359970854586, -111.46016206343049, -110.23478747568004, -109.29441275295858, -109.82941912510167, -110.43088525283673, -108.21649744751299, -108.70220592702613, -105.2334473604296, -110.60620657984927, -107.97533820921146, -110.7664079806058, -110.56406610911355, -111.76465470250328, -108.84172809688911, -111.03661078143631, -109.85351980370237, -110.70091167176791, -109.52380717508088, -108.4356492672842, -112.25498760397127, -110.69648730540193, -110.36748838594507, -109.99090797924349, -111.2678642544111, -110.42541694325627, -111.4575545259775, -109.3211175669008, -112.7465573314208, -109.56208667784249, -111.59733497772172, -109.42295730962105, -108.55804089331346, -108.71397903286748, -110.09188290952392, -108.90810063278326, -110.31333217069538, -109.69794714542728, -109.06210020835357, -112.42465112160288, -111.74630553904855, -109.99304310093493, -108.93867687355595, -113.1669287525049, -109.09193568851137, -109.27500368450697, -108.99643325722404, -110.53962759110647, -111.2052088429852, -110.05855563908841, -110.30763723153481, -110.03411001268613, -109.6161415052669, -110.6304714466923, -110.17116005754627, -109.0753171640551, -110.92564270851628, -109.60831770517053, -110.25913363817017, -107.76644895378317, -109.2619309023068, -107.64198246311884, -107.37056168314048, -107.31978563121643, -107.68171928702894, -104.57515288104209, -104.75187637758803, -105.27246893266054, -106.96524396060869, -105.93920355631757, -103.66449995825586, -104.08476660009461, -104.53081578265315, -103.0148493379086, -106.74751670818362, -104.92309629919443, -103.98320340724693, -104.81633219413234, -105.77996356028235, -107.12559309216644, -107.28196039053535, -108.84583578337953, -109.4494696919565, -109.15525441177898, -109.7634811359225, -110.79433338587495, -108.44440079452527, -108.79597700117748, -109.98590735173822, -110.72144284267539, -109.30550753718086, -109.70072152916897, -109.65801130162137, -109.65949265997646, -109.82238573025273, -110.30669821947491, -109.83394128869384, -108.90433312205332, -110.664046708231, -110.39926453734134, -110.37725911098757, -112.12508639032839, -110.26795666332589, -108.98741993218054, -107.76168841100478, -109.82334992872889, -110.83516363498563, -112.60649745671253, -111.1960726449926, -111.03919163866381, -112.05129034965563, -108.83187987662883, -109.57240688505179, -109.32857861150738, -109.54934849013647, -108.29359879300195, -111.5179112931669, -109.52702486426027, -109.95429980789645, -110.7011078611564, -109.43204524997455, -105.56031249677113, -107.70609254346495, -108.78303653454363, -108.11457060956113, -110.44215460317537, -110.78267897406572, -110.33119812901934, -109.34449539666907, -108.82636558484161, -107.1834151347969, -108.83808254322192, -108.2542825327446, -108.80298057862501, -107.59922121598055, -108.9131916496929, -109.51519107961856, -107.7704986323755, -108.79678029009878, -111.13791068210752, -110.402746275919, -111.31702623823912, -108.49812727557243, -110.63723264798182, -109.32890666586829, -110.29721723278237, -111.66560929315017, -111.04227698307153, -111.36927505376269, -112.5203298417673, -109.93967930487354, -110.14533835678606, -110.3868348991775, -110.85413569165249, -108.44519725537315, -107.93391978795047, -109.82778679299085, -109.79311153223738, -109.25261055399044, -111.47738679135526, -111.11775495397512, -108.65898844492045, -110.26505495390529, -111.02017977446526, -110.34817965403467, -107.55161094495372, -110.21667403085983, -112.43970497917284, -110.70535338255132, -110.79438078890512, -109.81809822502822, -108.99167960596515, -106.5556893069368, -97.51736665041192, -105.29926513345109, -108.72453297392224, -108.23203912463346, -109.50324111400698, -110.9939986929772, -108.05367524487318, -108.37339392211176, -109.8553291283933, -110.46179639493138, -112.48795697163695, -111.88145079973545, -110.8678969738583, -110.62677605624849, -111.83824818603244, -109.76798658735359, -109.6654742351465, -112.58543522753767, -110.3406716250781, -109.55013159400883, -108.00481229232405, -109.90793236599207, -111.28597960985334, -110.54144527494444, -110.14704702870655, -111.2652554338908, -110.97520848958668, -108.63647576273343, -110.52472680617548, -113.16137826273847, -109.62457037485827, -109.53869420402964, -110.71399284283449, -108.55435337782664, -108.09492728294455, -112.2373886856363, -110.3693019226993, -111.65116752865308, -111.3223986412311, -109.67734725401074, -111.36420709226297, -109.14293108556625, -110.5982939020188, -110.29596476096043, -112.69847120697035, -108.39052787054206, -109.06205229490357, -110.00045399262885, -110.71775009467346, -110.69530760167493, -112.54144940754935, -109.55755373438097, -107.88943697845929, -109.98578587243783, -110.14202980613851, -110.80051915904802, -109.11327182471621, -109.50637030500913, -109.77023677605327, -109.98552825925917, -110.40235854896, -109.37603004890141, -111.36989177909379, -110.8399811877331, -109.30394670937987, -112.2769814990538, -109.10893172594731, -109.17733972841754, -108.35968166480572, -112.64492569586005, -110.13779257328873, -110.64439690778532, -108.45446935516622, -108.97325006911116, -110.54637968933774, -110.66412364132371, -111.38627695224784, -109.8942998516069, -110.36392017322382, -109.92355133054227, -109.61886697310419, -109.71969465343778, -109.85627196259388, -112.1407808286419, -111.1013489416651, -110.70428953307596, -109.3454280179969, -110.22984684615578, -109.53826801613613, -107.83673208330934, -108.72742563398342, -109.5745872123195, -108.83031823548816, -110.89059911076627, -109.87842545384129, -109.21980161063786, -109.07140273870678, -109.04628915564135, -108.79255665097845, -105.20875397856382, -110.0838008881032, -109.68293832806683, -111.24644641302518, -110.01257579497496, -110.99281477454484, -108.99296184719546, -110.96495665514604, -110.70404386182749, -108.25078498739035, -100.77667501455139, -107.61479263900088, -110.06600976399395, -110.02035637581871, -111.45524052052504, -109.975541184397, -111.07333860975358, -108.4808974233161, -109.59513524582242, -110.74711589861774, -109.50005300854993, -105.23071652566294, -111.81094849223531, -109.0168079712372, -111.89029991620679, -109.90672274216391, -109.30959446424889, -108.23718655264584, -110.10868108588909, -109.21139771899594, -110.33333323577992, -110.25792318324204, -110.67825932924109, -112.33148517950511, -108.9724848367048, -110.78371843797613, -111.40913868573313, -110.2930522718577, -111.9538408094371, -108.63639312641844, -112.4462941079034, -110.40266356498321, -108.66617580940074, -109.44306834729083, -111.08962916641603, -110.52132608161017, -110.53757698855654, -111.5587344449704, -109.77722315102946, -110.40060629757771, -109.45395807961631, -108.77558572395142, -109.0151938598724, -109.80739619986889, -108.9332873172888, -112.49933978358132, -111.28667321897437, -110.40629082858706, -109.9829216820938, -108.85102919990373, -110.84179127037925, -110.27309817549309, -109.88857884367955, -112.24517967927224, -110.23377125710859, -111.26951227953063, -110.09782138347559, -109.77508406986834, -110.55359722398646, -110.09534729906368, -109.96333904888587, -110.29372855476366, -111.36651812163072, -109.97141184588116, -110.16701683369045, -112.8562627359291, -110.66651146857079, -108.78873821095968, -108.59208174618087, -110.31784275318834, -109.43177042415276, -112.80272887161644, -111.79874205007107, -111.08216899537892, -110.73699224045636, -111.04738767291953, -110.43395896705012, -111.62106163510778, -111.32599933330843, -110.29360981749807, -109.66562228449096, -109.21316193790335, -110.06363162177448, -110.54480468587292, -109.31791670875509, -112.65386492377107, -109.91857609999171, -110.57233605624137, -110.7597333064856, -111.49767138733276, -109.36548654843229, -112.34145274183716, -110.52831153822652, -111.55802243871352, -111.81399803046556, -110.17680125962372, -111.23811621944807, -110.48042049674514, -112.43786993562033, -109.56507357271987, -110.67030752598993, -110.86377249100713, -109.06001892813467, -111.37023727930494, -109.52881096984436, -112.95107295160436, -110.49467818026214, -109.29804210589607, -109.89270706931751, -109.46354468058833, -112.10350702955014, -111.06083529077077, -110.49996587015904, -111.1617248913634, -108.84725633199014, -111.42852695852422, -110.01433866707184, -109.11616968390972, -110.76961079765468, -111.80403513904453, -109.84442686379181, -109.65447921666167, -111.3378640555306, -110.8882647652338, -112.58014202075226, -109.67128881545659, -111.73429980763389, -110.82258070774773, -110.71895931098041, -112.5117489008152, -109.16182299471309, -109.71651258790612, -109.7770618808562, -111.94294809571427, -111.1629115541574, -109.57489224865171, -109.8402445779754, -111.17931450307283, -110.09045865447595, -109.23658206733491, -112.54929616847242, -110.5150381158864, -111.32296447909377, -111.64472156295191, -111.65832771066007, -111.03359562742956, -110.85303206770837, -110.80655337650862, -109.3712696310075, -110.57313454785879, -111.18525355670417, -111.67423695430561, -112.00829831274282, -111.08915434609605, -110.3298290221436, -108.68552957386795, -112.11377370993225, -110.80288297661977, -110.33640536217185, -109.5907971201988, -107.9195263775506, -108.50223113159429, -111.91191347156142, -110.29585599512956, -109.50902788911351, -110.76819145749467, -108.86899533416589, -112.09963049260891, -110.13374376572433, -110.15881393584463, -110.87392107947531, -109.18658540731009, -109.72734703956934, -110.18732487568724, -108.76554115185057, -109.94122289815374, -110.39583285609643, -111.09540935727229, -110.6618176357367, -111.6281345666718, -109.69686483639367, -110.31633402076315, -110.61246951748903, -111.73300235294965, -111.34221378834899, -109.46708370903485, -110.70412671997354, -110.7007891485379, -110.31685483435038, -111.03016917417074, -110.94517365625376, -109.46580797053619, -111.20935248224806, -109.20661126636224, -109.50147037097533, -110.14241781654353, -109.8510950344643, -111.3794198224028, -111.28966889207122, -110.43347441663424, -109.86759980279523, -111.92101892013198, -109.31594011390644, -112.92253433794441, -110.74000829597605, -110.3690783911604, -111.9386136764295, -111.04196305034188, -110.41800427558245, -110.94287511448232, -111.66035388807579, -107.53723747644062, -110.68014818358719, -111.86628806511304, -110.12097497430523, -109.69880468221378, -111.4312783987915, -109.18240866486639, -111.45649839248873, -110.1242345454651, -113.75911576151633, -112.71747598882953, -110.9614554157337, -110.92294419716129, -110.87229098694876, -111.09943759113875, -109.48107247947176, -108.62783006742795, -110.8108025857779, -111.63342408317932, -112.0221522906341, -109.96411229549527, -111.29821085030613, -110.04566676239914, -108.41674583097112, -107.50256474992416, -108.68086611003493, -110.3738906060137, -108.86763212826641, -109.81681043446049, -111.04539822346567, -111.73290882980949, -109.75238769150758, -110.55268275367449, -110.48423701377924, -112.1116140908134, -109.53952175199518, -108.538611608547, -111.3788321484912, -110.36378736224961, -110.37712171023523, -109.82150687920334, -109.17046632238393, -105.1169578108227, -110.84067642540583, -112.91626789016587, -111.32030958133453, -108.93375913686056, -112.44450956563915, -111.1596840012794, -110.17380444915341, -109.634859036508, -110.68819277718731, -110.0648098825346, -108.87385575091399, -111.99676414571755, -111.32585405719519, -110.59892045991457, -110.32589048340424, -111.1172696292077, -109.79946399891651, -110.10030723919304, -110.71841081343656, -112.23013150012054, -108.94400401141407, -109.71044551701596, -111.77560214164039, -109.68779520039777, -110.96119601299907, -113.66477058855787, -110.17794649102234, -110.30159876509862, -110.11953836266514]}, ...(2 in all)]
  out "FFT 2":cluster{"f0":dbl, "df":dbl, "magnitude":dbl[]}[](graph)=[{"f0"=0.0, "df"=16.666666666666668, "magnitude"=[-324.19011195451765, -78.1272953812706, -85.85545438627958, -89.30587144190069, -92.90590394398903, -93.63083388385274, -91.8644929119412, -95.26924857401164, -97.0710469181336, -98.01148078956652, -99.33043660296804, -95.58776817681839, -99.9570097527269, -101.45494093095093, -101.51838334751548, -101.00386616525799, -103.01963069818913, -103.20223925731209, -103.53783076500916, -103.48065647812659, -103.97797518531912, -104.58942778240602, -104.46991277190502, -104.59813972158683, -104.56685024229951, -104.69893799348945, -105.05669000016238, -106.17061117835001, -106.43303821862656, -107.39468286383597, -106.2899368267905, -105.7863846168199, -105.17170638885071, -104.53818172761852, -106.70340956723133, -106.55444321137247, -106.67654843051936, -107.79888413750199, -107.86424326005849, -106.09722609215336, -107.71648639013972, -107.79500725395155, -106.17330953637067, -105.43663624517525, -108.04970689199158, -109.92106271611999, -106.2505251183406, -110.60221373795562, -107.11377887451098, -108.4126937286195, -108.37794745021417, -113.22457316369011, -106.38281814065472, -107.55385617652075, -108.93026538982782, -106.19334142366085, -108.90462602264525, -107.63084712174981, -109.12192537022624, -107.90627042480016, -109.44472079190832, -108.91731458372392, -105.74102972706788, -105.74407510394178, -107.5989477192235, -106.2838630137392, -107.46190542725505, -107.38881299750702, -109.08024783239452, -104.97871836903269, -106.65424712290651, -107.04966019632134, -106.16202578092883, -102.98374199247179, -99.1568704142098, -87.07383781389657, -96.41471411313154, -102.65176579899618, -107.65674867775193, -102.85397890306213, -107.58658613411464, -104.79044898833125, -106.65282019869865, -108.65027966345534, -109.46169054950127, -108.69969979291741, -110.4048706652988, -108.81020193837274, -109.42808902484134, -108.85398463561398, -108.3849716744813, -109.1844457168716, -109.32787859535676, -111.01992124870878, -106.64843449415699, -108.9926343573667, -111.59837822080355, -110.57121677672183, -111.17280164669164, -110.68901970586144, -111.69013245592781, -109.90200577018311, -109.3554172126163, -110.7515368822992, -109.2863324212524, -109.66209701262974, -108.50795548698007, -110.58126481096504, -112.36093896766921, -109.78612141282203, -108.85120530917233, -109.91424431080952, -109.84698632196245, -110.93960894966105, -109.77214706089354, -110.30762971422381, -108.77791302937449, -110.79522659679036, -108.47242514643455, -111.20629758187835, -109.05996769621125, -111.13574821570619, -107.79388178889101, -111.5768481279296, -110.52058839597171, -111.58729762739313, -108.99000864386126, -111.6585121505227, -110.50715371958135, -108.87151956974363, -110.30486244367107, -108.32392040018144, -108.1769507919999, -110.43198471512189, -109.81454097966842, -110.26717009815644, -110.82924135076777, -110.34103661156989, -110.0692667126265, -109.34555682020833, -109.1694484721415, -109.9940980324044, -110.81940616215803, -108.21162003366862, -107.97087538330561, -107.55312461506225, -110.60339321606872, -110.09004629292225, -109.05860430198882, -113.1412749514818, -109.81628200948371, -108.62343219429849, -109.48172424209761, -110.85978755785311, -109.47778611557064, -108.81728552967951, -107.47864241666747, -107.61735128422292, -109.62511618983821, -110.32417726356636, -108.24287897478176, -108.60460879530194, -110.2181558494026, -107.95550802888957, -110.80234484950323, -111.09955733353904, -109.43923052503506, -108.98949130235951, -110.05778199870154, -110.36224432927585, -108.13523430027999, -110.681114579241, -110.49106131529867, -108.73493328004297, -110.07663907252234, -109.9968931372618, -112.10715231091008, -108.80994125105168, -111.63774865669372, -111.54355694032755, -111.64024217585788, -109.34986300492378, -108.88053713185408, -111.14370830146245, -111.17327416167232, -110.36311492990576, -109.99414559884396, -112.96912007380595, -111.43191437097785, -111.71327312809349, -108.77202323682606, -110.25970374932486, -112.59574277180732, -109.77247894866957, -110.09219852365874, -111.7197662726775, -109.85454092697009, -110.06789440397942, -110.38055758638309, -111.04251386932805, -111.54279434240568, -109.74385329575985, -110.98924544863415, -111.17898077762852, -110.98364252730245, -110.75024385843372, -109.24766708578407, -109.67753987004863, -110.6537235844391, -111.84436313010086, -109.12654337292446, -109.65519521121124, -111.1845162935778, -110.5009101465602, -110.22980642268818, -110.88540043278346, -110.29249073109453, -108.80459864528464, -107.49372141121728, -108.50353962704821, -110.00730069533373, -112.012876492648, -109.01283702976382, -109.07442203290057, -108.2961442983685, -111.60962842680907, -108.84312815413224, -108.6276642979969, -108.75132871638827, -109.30004903844721, -107.20359872252604, -109.12175943862074, -110.43914247337625, -109.55954680842791, -110.37116786618797, -108.55907813251434, -110.19249995041955, -106.95269845697632, -111.07027929458712, -110.1073996792702, -110.61729280468039, -109.6419175310234, -109.47995019876329, -109.66602827275211, -110.01953864498805, -108.45989120418268, -109.79778555296474, -109.94663827736616, -109.52410616839379, -110.58014441463794, -110.09182359045897, -111.0487262011397, -110.49609187214915, -110.6114701312941, -111.17752423063314, -109.74965389041003, -108.58973724447526, -108.84292130035902, -108.90689510645983, -110.69840140049361, -111.30494362640982, -111.00224390075273, -110.50848328538423, -111.59232911931113, -109.30826761863756, -108.44510893127558, -109.63744704504391, -108.95037574307332, -111.36486409910674, -112.74508631930381, -111.03952454593811, -110.57133212903979, -110.59969855145111, -108.25570461975128, -110.44617635200193, -110.32190307214704, -110.95204704643322, -112.0595421753479, -110.45342552693265, -112.50183987758867, -110.08217804938009, -108.90353583389084, -107.02032313792242, -88.3334978919524, -107.92027625495886, -109.83148570028482, -110.30427997450572, -110.92855407802753, -109.67404674397338, -111.03606345823586, -110.58277018943096, -109.77692362669393, -109.39170901729935, -110.20711662408928, -109.41601946806779, -110.34213214925832, -111.2283900972803, -111.51682597931386, -110.47069117801351, -110.93808974285523, -111.11277478000933, -112.50698886748012, -112.12918507523611, -110.46316790252011, -109.9387334819968, -109.78723249688426, -107.13037722044297, -108.16132376075751, -109.07255491017162, -108.85068428558272, -110.28038153100799, -107.77611023481016, -110.69754506886444, -110.09495581837979, -109.21214884561816, -112.62718526248648, -109.22048725312992, -109.17793923163308, -110.87372121410577, -109.71902632604333, -112.61041177225496, -109.6374750969677, -110.74738952366951, -108.93404661877067, -109.84938675700889, -112.25316361679832, -110.30788094875312, -109.26929069321925, -111.20853536783942, -110.05212566057608, -111.72448131932816, -111.55474439772887, -111.81988954424324, -108.44452452934028, -109.21897824914645, -109.55634869894358, -111.36318572800242, -110.05777399011298, -109.64458567712875, -108.73315084760529, -108.93332091319675, -108.4816455312154, -108.80120578498936, -108.1804470361839, -109.7177707524778, -109.31977709844544, -109.33603116022124, -111.46120546572519, -111.7480378245176, -109.17907150677627, -110.47970652472505, -109.73718750984082, -109.7935026884937, -110.40458408612054, -110.91781389491092, -108.39352075861481, -108.27512197925346, -109.59155075404814, -110.40183121737397, -109.25423373270381, -108.37769008625712, -107.91335995938509, -109.5576520703013, -107.27392145737491, -110.98592762117059, -108.41809950647861, -111.48163889400448, -109.70961684769624, -109.22952568656495, -109.76504719131209, -108.86928627177666, -107.97855299877004, -109.8412204399902, -109.6690048999326, -112.28329030175193, -111.54977099314607, -109.55689540119126, -107.93716711232997, -109.84247640855929, -111.5098351445789, -109.14317615215809, -110.28319116384824, -110.57901069942578, -107.2890252845352, -109.66754569546274, -110.15708115946433, -108.83782190109405, -111.60783857760667, -111.46884385151185, -109.21985333366634, -109.63605494317056, -110.87999187262697, -112.26992029775087, -111.05491095860552, -109.22795442529183, -108.99135781712076, -110.46475190704264, -109.35746113713218, -109.29125989270668, -107.40922407684049, -109.24391685563656, -110.41554602144217, -110.68952735085914, -110.62457364102458, -110.39856310555466, -108.84256124354566, -110.01614601335088, -109.8071306678428, -110.2804500736802, -108.76205061238203, -110.3962440297242, -108.98253716257014, -109.32990745926702, -111.17276766165281, -110.41113652364085, -110.36616199963426, -112.09767002991742, -108.43599666470733, -110.91876588140981, -109.05329272502944, -107.07198690769708, -108.72934463903034, -108.6666471996132, -108.97529973794413, -109.68895260146817, -109.2658844652487, -109.75690097249196, -109.38585024123027, -110.17593039468063, -107.87223111061134, -108.15261097418302, -110.09277437980633, -110.8665497655964, -108.43061614348413, -110.3052458526819, -109.22446919161898, -110.51909692711594, -110.06620699121913, -109.53439413051383, -110.31952463872884, -111.4732125902982, -110.41443606663168, -109.9579358088152, -109.930778061577, -108.5473214465574, -109.34719220288939, -109.16964653934396, -110.04824158176345, -109.42616539603762, -108.3556027482992, -110.62331917617789, -111.3652147859356, -110.12362012120938, -110.13175448595814, -111.20110099151856, -111.50643914621541, -108.11659117128028, -111.06037600347967, -109.03822892917451, -108.25678204604324, -110.82608024151122, -109.15887945314851, -109.88255674562845, -111.18322672526185, -110.95836040044516, -107.91535345885436, -110.66285812468733, -109.61906549925033, -109.58059721670746, -109.65198009505977, -109.65950565672951, -108.95264505276342, -109.23343669003113, -110.74308548011575, -106.39170014998685, -109.61471203101753, -108.24258770956924, -109.84609566640096, -107.83834185503922, -108.93052854090027, -107.55568820082641, -109.758551082242, -110.65892780872205, -111.99907420485852, -110.71043004141137, -110.62257237494617, -109.15610413532767, -106.87403836327807, -108.19175324576331, -110.27819583792918, -110.23918003777561, -108.29703377268754, -110.07182881114713, -109.60256111108491, -111.00394752430006, -110.30750337485472, -108.78309624082331, -109.24103013025798, -108.76979253891403, -109.91618737478264, -108.83915940855513, -110.92536150834754, -109.72250903746432, -108.96533939688658, -111.08949280651164, -109.20335070860871, -109.37826578362439, -109.77953166722301, -110.1867310744785, -110.07114559821346, -110.7003631567182, -107.86455899696074, -108.94113264174617, -109.35999427135138, -109.33627364788704, -108.96588828808375, -109.08716536982254, -108.73575375369026, -109.47770132070654, -109.83726171472907, -110.73516506891792, -110.56827134787686, -107.65667508354096, -109.30200115708924, -109.28406803847896, -110.55374624323233, -111.2017766725333, -108.50851279608973, -109.79494403619485, -109.08320018013063, -110.21850624918747, -108.4652936555984, -108.74837610538873, -108.81326140648238, -108.83830180036702, -108.785270477003, -110.01845876259073, -108.76030368637825, -108.57879884880157, -110.6610608456059, -108.74669367794318, -111.55956030460833, -110.22906685783455, -110.48411613865359, -109.48060880085136, -112.77556331479562, -108.2676071206087, -108.8571136162698, -108.56944905160177, -109.16406757131058, -111.42259299295839, -108.25216316582294, -110.48487127684025, -109.69532331373831, -108.13992755196784, -109.2987762526628, -109.82536192480795, -111.28650061088359, -109.12820736404241, -109.37960655471406, -108.96014976926716, -107.97535047619023, -112.31953123574708, -109.06198330523004, -107.52722515967098, -107.31555373665437, -99.89671790804692, -107.44442600896275, -110.6549218761941, -108.02265794322076, -109.63582761762919, -110.00574746987859, -109.51565124961209, -109.3550083591902, -110.4541529175301, -107.85799722437162, -105.1197113090786, -110.25038075579738, -110.39710812865657, -109.3618876098789, -107.6131301952152, -109.21529527621463, -108.7995754403799, -108.48347353145697, -106.45678488065816, -109.60427918561142, -110.81194387812535, -109.52215044127382, -109.88751598659705, -109.30205143590227, -110.74984456751768, -109.03952092986351, -110.69170786328897, -110.39236248162467, -108.65456161733339, -107.60439764386904, -109.97367926606955, -110.2754359970249, -108.81546418006434, -106.99691398176165, -108.42047325825182, -107.24499915944605, -109.28116135603187, -108.70650358781573, -108.05516916105047, -107.20893100196241, -112.07029265690055, -109.38099990478445, -111.53461820465232, -108.11312509555277, -108.76714028655223, -109.89565008459624, -107.71879172001115, -108.08434857420214, -108.79142773619792, -107.25153085963885, -110.05595039449301, -109.31604222314259, -109.94405791565286, -109.04715370361387, -108.89278831045846, -108.84682466376424, -110.0067927716526, -107.63768959294084, -108.98109382020348, -111.4720219575084, -110.76023788797733, -108.78599647633777, -106.59726674064618, -108.66715709719243, -107.99134359630926, -110.11396713841884, -107.21091759882775, -108.08576824949941, -108.80217666857972, -111.72949572713338, -107.33126296136014, -107.33731660097102, -108.04470462977443, -109.42963925921418, -111.03517778720736, -109.55293581015796, -107.99948151285162, -106.59480934999681, -107.63777243313498, -108.96490626068824, -108.8948210299064, -108.30870516747477, -109.13612869658097, -109.59971429402015, -110.2571461001396, -108.7655464686992, -109.81144209568883, -109.80796806645141, -109.20948481699544, -108.68653880881129, -109.26329796696166, -109.22428132233863, -110.12571678351438, -109.14615461144786, -107.08261621308327, -109.11338327144382, -107.75421565039201, -107.45291780756361, -109.00477000647248, -107.41031480478154, -109.98948062864928, -107.45953654921264, -106.37522884807879, -107.7786128523167, -108.03610987358499, -108.05926797128022, -108.59400205554164, -109.89620453365603, -109.03811240487515, -109.96909236705363, -109.28212981785472, -109.6772152101994, -108.26493868190678, -110.55558039199732, -106.6252818398841, -110.19075011176416, -109.56520012524705, -109.8023423576176, -111.2697570480663, -108.26752571816566, -112.00337375484828, -109.85709226796116, -109.36922081321148, -108.8424844298318, -111.2512302139209, -110.61775974680471, -110.22501328999012, -107.76874906708105, -110.71023653476604, -109.4025656165291, -107.66667684986125, -107.59759854092948, -107.94763263251238, -107.3888591871119, -108.62692803125044, -109.18012867988286, -107.78662871481455, -108.5072814073944, -109.50348958982907, -109.95177634938378, -107.78756251182895, -108.03865042797304, -110.1814993556385, -109.34937567548833, -109.52162025123161, -109.50819015441117, -108.20953105254624, -110.52154040214435, -109.3324404469266, -109.2696617050831, -109.54675609195674, -108.5940367000989, -109.40184828664549, -108.2518305610941, -108.55972691669434, -109.03647225394408, -108.48166656251695, -107.42023429066523, -109.42453054302521, -110.09532345960083, -108.78315822119662, -109.97508586102265, -108.22687406536997, -109.17110028890058, -110.15390449992647, -107.88577458651508, -108.28851074361447, -108.52030295163331, -110.03496861709483, -109.40014319167584, -107.73048113044877, -108.17571683963915, -110.34839852994926, -108.55894048192191, -108.74107339998285, -111.17734138993401, -110.22946440841412, -109.45511941802884, -108.0657300641843, -109.33797363184166, -106.95974095511333, -107.93068343723691, -109.78867669512647, -107.2087297624043, -109.542665021243, -110.05035859052961, -110.30235238883523, -109.20586170783808, -109.2796396673401, -109.14260673746566, -108.22019460542734, -109.99011886871159, -109.89103038547285, -110.36964772493243, -108.62340319923602, -109.06779821699769, -109.21830861066148, -107.7402395759509, -107.7178850938205, -113.45665085929117, -109.24039191621704, -109.30387033426037, -107.61849760982835, -109.41430582703529, -109.11482836392241, -111.89328423764577, -111.84653367963301, -109.00674896486915, -109.84488648739638, -109.41914760797953, -108.53442910169935, -109.66883322968232, -107.68762956301386, -109.82583101109167, -107.83405397804887, -108.78052031141966, -107.37842078941692, -105.40843158543845, -108.81430898189338, -109.57374640194516, -109.41111270322058, -108.82621700188898, -110.2552502368822, -110.23903890097205, -110.52171662278697, -108.21249857906324, -109.97268479379733, -108.20088823960992, -108.85682002802234, -110.11642849164285, -109.94087886999255, -111.63180946270296, -108.20899499456195, -106.73341567332112, -109.90003508676807, -110.14688274481229, -109.62259307329889, -107.57811196819495, -106.88584597822792, -109.16132624528932, -109.78677836397806, -108.59319344451784, -108.55877448618652, -109.46883711353044, -108.47309455543844, -108.09487065732198, -109.82219079158135, -109.63780237877428, -109.28348848877269, -107.62893405379826, -109.46986737961593, -108.03089712610223, -110.3931917410696, -106.06970126043262, -109.41866550703786, -105.31710372440419, -109.20218082282653, -108.28467118008108, -108.80026326744611, -107.40729224715713, -111.07322915141532, -107.1057186510818, -107.98286374205958, -108.51298722989311, -108.69632670891366, -107.96509231988331, -108.15882223414738, -106.85862416470376, -109.70705792539056, -108.64519930633055, -106.78708421443504, -109.43552377900174, -109.4474526498122, -109.10135248755788, -111.43316642580763, -109.33457343739448, -110.23547887071898, -108.95690647379442, -109.21159903769149, -108.12969562680841, -110.82751409340537, -108.55724349027832, -109.8796329603075, -108.50369978374582, -107.43145467247209, -108.60003323209516, -108.77155705999647, -109.33806063660796, -108.37500858898439, -109.65641721611547, -109.81905873737344, -108.03483220769625, -110.48028107566635, -108.60527372219985, -109.28768201151478, -99.8804125587218, -108.8913334544964, -108.23534920737794, -111.07646463287153, -108.59029790589766, -110.3405916586831, -107.66387718565608, -108.73793152614131, -110.61440166477816, -108.76211382544581, -110.23236978486065, -109.10669297094852, -109.15247609779597, -109.00539004923506, -110.14424353412238, -110.55445060661157, -109.48721312920799, -108.17040942305823, -108.77592227268228, -108.77130256578067, -107.82494496098512, -109.57266989523707, -108.75767497229612, -108.13688624150026, -107.8280716764963, -105.676279602552, -107.6370316684844, -109.73508547021689, -109.25365178573009, -108.86767843317584, -109.70969944273735, -108.91917504090888, -109.97734866522867, -112.17308993943783, -110.28356299479682, -110.7927103729386, -110.30837645846702, -107.56364161860179, -109.50188349731121, -109.36065627483853, -109.75389877587511, -109.81713476007774, -108.14524057525358, -109.43832376796216, -110.89342891210596, -108.15657882822792, -106.84106061627887, -107.83091759905821, -108.61794662682962, -109.57142366843581, -109.85402645528154, -110.12877022469837, -109.19414429724044, -110.56168468006764, -108.74720588273881, -107.90448559921305, -108.54421401507743, -105.06700039841249, -109.17937358052484, -108.94317576365822, -107.79410219455083, -109.24955437598658, -108.23334395173994, -108.98759227946937, -107.05986359444529, -107.20956512998849, -109.00295831471958, -109.43119556916457, -108.93348410522628, -108.99932477701081, -106.6448790859128, -109.06877251308666, -107.67053918439544, -109.15052780608639, -110.16878033319385, -106.55101141640301, -108.02811045752685, -111.52173447126572, -110.16854119242062, -110.93164036911654, -111.25979320890855, -108.82629030379024, -108.52004501839738, -107.09697056562636, -108.94233383169858, -107.37962568194772, -109.1239201710643, -108.93949898577122, -110.62573772949195, -110.09592372075662, -107.56136391005947, -110.45600430869621, -108.79481000016084, -109.41462449554598, -109.30248158488335, -108.70735295493108, -109.9174743694956, -109.94232543385962, -110.71725446170196, -110.0346196158573, -110.34814317845934, -110.6651078322521, -107.55409880424479, -108.71734776861287, -109.50902203986271, -110.40207542979611, -108.7847687630861, -111.10599488129682, -109.30824728923263, -108.20134064331717, -110.55959112431609, -107.77099734327174, -110.23862843385446, -108.48520797666865, -108.54205896654946, -107.79288769037599, -109.84022250170581, -108.02758364115576, -109.35132492327935, -108.87009749667932, -109.86905123364855, -109.19826752168308, -106.835240323691, -109.37910022114056, -110.80633973102931, -109.12703823829597, -111.07432699570984, -111.8064506085314, -110.09349947650527, -108.66467295777367, -108.75119108236053, -112.63983351316729, -110.90940743670113, -110.27973159222081, -109.57141664526549, -108.61645363771719, -109.31742355616147, -109.5839599160637, -110.01188998365383, -110.01923429741011, -108.94779759137936, -108.26169431000017, -109.24553201026085, -109.95709526422822, -110.68677343596859, -108.7678734483002, -110.47090469179284, -110.31604700116512, -110.10256600741997, -109.76634647265719, -110.8830805828562, -109.94609564072982, -109.20662382740542, -108.12492970530919, -110.5274435478767, -108.02351960398035, -110.6264936805739, -107.14559226383577, -109.13821777857531, -111.05324489472586, -110.15190797512811, -107.96366234783144, -110.03950681967147, -109.17476300510336, -110.41251816187909, -111.39219865477246, -111.32530426869943, -109.97369363558423, -108.98666403063845, -109.62049358645565, -109.58130494498671, -111.72738873188874, -110.39825891106616, -108.57430325757545, -111.28625510212446, -108.77421250595326, -109.75025415031793, -109.51948456745635, -108.82129398637998, -109.81362137198361, -107.86292494316123, -107.49318292857053, -109.66948564589373, -109.54288390056654, -107.99912445612077, -110.3497559614379, -108.00549349666127, -110.01361420523357, -108.4977916421456, -109.67078387286976, -109.85678367732866, -112.01237658746248, -108.4855625950998, -110.84880875737286, -110.9178674382154, -110.44187536727453, -108.75076921971127, -110.04946286646651, -109.99780941000827, -110.14242932305507, -109.56343773672316, -109.6278993388131, -108.77419573790174, -109.10543670530926, -109.7801848627463, -110.30733124104881, -113.13440550301436, -109.32709134514755, -109.74136656933283, -110.01525283266193, -109.43924662938396, -110.25325289253, -107.75460576671303, -110.60057027395933, -110.71458404922404, -110.15788509050662, -110.69167485018224, -110.96006652476157, -111.01156633983031, -111.6058448010008, -109.51364005052672, -109.76058205940885, -108.43421621088261, -109.47973949170208, -109.25533250208288, -109.47422603921065, -111.36411644613841, -107.27566171102698, -110.45098686173688, -109.93589296291184, -109.03803734663714, -110.53118128434016, -110.2408872254969, -110.0532234862915, -109.94185495614619, -110.2662004220774, -109.51094016962288, -108.5210104215432, -108.13691752270934, -110.18460088390265, -108.32609309150783, -109.89652230508281, -109.80923900768477, -109.01917388968883, -110.01248300968739, -109.43415605440147, -108.09823485138017, -107.40637725320931, -109.40632232658412, -111.97981999127656, -111.16609811629485, -111.64500793960192, -110.99793748693381, -109.55531276386903, -110.2535662621666, -108.17429802469516, -109.09425673355422, -110.23187110421917, -110.55358397926925, -109.93461124753053, -109.55604345832225, -109.44569510408274, -109.72185151080762, -109.52963702944834, -109.2303630328152, -109.74819502244243, -109.3932530349457, -109.17096788339686, -110.46153727064616, -113.1073731246639, -109.43753070459397, -108.13332547768168, -109.42294574929969, -108.45798401969856, -110.29453435046327, -112.66249403705643, -108.78314667434937, -105.9634478773668, -109.14327524669528, -108.50645190860273, -100.81571594994128, -104.4482859840643, -110.68926237051092, -109.12362553230196, -109.45234390564677, -107.91461416156068, -110.67788819353727, -110.05744935668449, -111.78333392154664, -106.83628914455993, -110.11115457346548, -109.13434608275826, -110.80006861194663, -110.35323502651462, -112.29149906501372, -109.01656376530778, -109.30871662948859, -109.79736315392456, -109.17848983603582, -108.09752397056482, -111.6039030763455, -109.27008844877828, -110.84475733314184, -109.72393917557073, -111.31060762894991, -110.78858793807466, -107.12841545099752, -109.54510865218204, -105.2805426080281, -106.28514149354733, -109.50656759582803, -110.14700878401054, -110.49737016725709, -109.19811547071924, -109.92527399676051, -110.7961615015146, -109.7447227818197, -109.49432012009893, -108.714081576733, -110.09766801550917, -109.08448507943001, -110.36154838733857, -109.86328656267403, -109.21144237434696, -112.4145136888034, -108.57567151011159, -109.66748589540896, -109.72985837578446, -109.29989238126763, -109.85868902806475, -111.01778182304162, -111.23625326328558, -110.01270868104203, -109.27067928081415, -109.71171312410247, -109.28697459293629, -110.67868067201007, -110.91353786857455, -111.21479955051575, -109.11315965407708, -109.40418681804496, -107.80511819596003, -107.37201025889816, -111.81969609169838, -109.89875624306032, -110.29328043898657, -109.74853280072202, -111.39527865400605, -109.47746221101964, -111.75141177452517, -109.31325306583483, -109.30117448911659, -109.3997781364162, -109.45356931295724, -109.60585285774386, -111.33951689512735, -107.74187210470228, -109.62706021606415, -108.72139655505221, -109.79552836110567, -110.64354037499807, -110.96138240913136, -110.02215059889615, -110.92978442698893, -110.0620778287114, -110.85019647293322, -111.77397403227091, -109.81257196800128, -109.15643451383403, -110.72777566469594, -108.7463769025616, -109.80959395914073, -111.24500986151126, -110.48863498350322, -110.30863780110901, -109.79331354195703, -110.34087081762074, -109.45183222569266, -109.6440990067103, -111.15034876658994, -112.14912485578341, -111.8886180186196, -110.57054820211916, -111.07556239924551, -110.5872832735073, -110.28912501038172, -108.91501133754849, -111.44575118962761, -109.90799859177967, -109.74421995550023, -108.70941446115883, -110.28822893097275, -109.70039554000401, -110.33701797570251, -110.79445894683306, -109.57694314608153, -108.816904416038, -109.66517126767175, -109.39501469321644, -110.85775022889956, -109.3689402795614, -112.09107318723095, -110.67985626248422, -110.32971146814747, -112.08166943494875, -109.93955548712543, -109.31722953035252, -110.2062913031861, -108.22565380081006, -110.680898028151, -111.95386604441454, -110.83354130587097, -108.5873626748948, -111.97536144124408, -109.23944159551515, -111.57859477689586, -110.80135186615524, -110.4800953731021, -110.14040729648133, -109.25873050390551, -108.87000960474569, -110.97091597211167, -110.15787270199012, -111.62434537618091, -108.5421625277294, -110.42258666403919, -110.96896115868603, -108.98253068925274, -109.54245055160168, -110.28051096122468, -109.48060498658319, -109.77618362117276, -111.64513838754992, -111.13945484239875, -110.18094280356001, -110.43757222770748, -110.81588360154201, -110.11656805555333, -108.47936291282355, -109.16476249859961, -109.3549985917136, -110.77753190334253, -111.46065694661178, -110.40387985996301, -109.95673803226478, -111.58660981285446, -108.59894875229345, -109.37333363882607, -110.26849699991793, -109.30500469266264, -109.23789020998296, -110.82000706486865, -109.25927538839868, -111.03285659417519, -111.08899832832414, -110.69361682858042, -109.45187168573815, -109.9614018482838, -109.70209527974106, -112.11903952100165, -109.59713611623246, -110.70292028698111, -110.12743849746808, -110.63315585514292, -108.60450276298175, -109.32832664986026, -109.99753023477764, -109.46644696130294, -109.1781290160558, -111.58830180575129, -111.67229040267557, -111.3750024136205, -108.33616679452298, -109.99797067800029, -110.50892429124391, -108.66074740829372, -111.17094662568759, -109.87538933985836, -109.152526628291, -110.44623159817101, -110.21603106403009, -110.64376935639365, -109.36897426842583, -108.67303022227141, -109.89327693080823, -111.50442955563923, -111.37532237834381, -109.38132821290205, -109.73509680539144, -110.53918379735906, -111.22869870340647, -109.39977573957616, -110.3674665334106, -110.5366125953241, -109.99025356764304, -109.97300035646616, -109.87631077033762, -109.64608829594286, -113.02486102973394, -108.26250283140733, -109.62234918138763, -111.18766216512655, -110.33666026406992, -110.5808115327039, -108.2971671321189, -110.10964334161903, -110.61254021379767, -109.89852549557533, -110.16562049054073, -109.41433790018287, -111.2453823439446, -110.45554802599901, -113.11454453784393, -110.7333866145056, -110.00858191882439, -108.54745315874294, -110.08430415376903, -111.9006972727596, -110.3031506154679, -110.26331790366497, -109.36797925566673, -109.04860552478912, -111.83514212681175, -111.38960737633833, -109.01429665187288, -110.96404839103826, -108.95488871107163, -109.09652004914592, -111.884304581971, -110.57566691021339, -111.95113404442795, -110.13677174050159, -108.10078686353354, -107.69442565416006, -112.42676605669463, -109.12681161784135, -109.23120766087519, -110.57649395555585, -110.22143082743162, -108.40065951773644, -109.46923168308618, -111.39095086729745, -110.46375658526013, -111.45145283328486, -112.22610823637353, -110.61090190564383, -112.22250292674809, -111.7379343196361, -110.18530386733481, -108.93867365671692, -111.89304844956082, -109.06146134986984, -110.98405731832798, -109.76366821333497, -108.08326795663608, -109.95041147835065, -112.94140614324155, -111.79814935135965, -108.07337559063119, -109.13733403265212, -111.74906646037496, -111.12228668433455, -110.02899450462209, -110.22237716929811, -109.0224776891049, -110.18135850497721, -113.32516073881047, -111.3576490243877, -110.60510094465171, -109.6935518470342, -110.36313473154901, -111.95933240129618, -109.49625308071019, -109.18827910216122, -110.54311407822692, -108.4811035913567, -112.81280225723607, -108.86530665787413, -110.85796435061886, -110.40059714639627, -108.19250716343407, -108.96956521802292, -108.61281798886506, -109.78061525370413, -111.58885511891798, -109.06279169160345, -111.43043988466789, -111.63169336321079, -109.54702536206447, -109.62860636296405, -109.47865811135546, -108.02265793654806, -109.97461304995515, -110.72549884050886, -111.57309413919933, -110.03317891949746, -110.39570411598524, -110.27606115470397, -110.63294457306095, -110.71821689302902, -110.38076268941819, -111.51223508887897, -110.40703572670697, -112.24933273737743, -109.74954300082398, -108.46020292937696, -111.05315219575881, -110.38635148390118, -109.58268303790976, -112.34211536832117, -108.45894118755307, -108.96463982695337, -110.56040438523046, -110.67803313671729, -111.07349872375121, -110.42184162876096, -111.82081126435692, -108.85923651136297, -112.57723799596502, -113.65690874668172, -112.62314325834605, -110.70357529341362, -110.959925221544, -111.26336183001875, -108.1350700630152, -107.94545932312926, -111.17610778209841, -110.20386728310686, -108.55646511121591, -109.8400922569145, -111.73466587035968, -110.47272877573613, -108.33011124048193, -107.93042857580332, -108.60928277989103, -109.25240966798974, -108.96403833602028, -106.94222615757475, -109.37086694261907, -106.72743097285155, -109.03160193412796, -107.3549903889451, -106.8543848510082, -107.83503929060929, -106.30745467433752, -108.36915807168845, -107.13065938379303, -107.84769200880969, -106.08004345082777, -108.15244601930225, -108.37254117816573, -106.57863034819223, -108.1283698227614, -108.19776505569902, -107.58283412238643, -108.17365133196301, -108.6794309781181, -107.91552140588759, -111.60122989270022, -107.04360635941174, -111.55535949001795, -109.39870426166594, -109.55937904851662, -111.81389508925734, -109.88957041098786, -110.84764586896561, -110.59130246272693, -111.15944135223884, -110.19496154041607, -111.51861903129362, -110.74798816525838, -111.37312965175558, -110.10842817220238, -110.73198099204856, -111.36708667993291, -110.30840247819665, -110.11744489669044, -110.55237850846444, -108.2073528237766, -112.70750856801911, -110.99917956040802, -109.84949484779976, -111.3403161887679, -110.08924435263565, -110.17749213365616, -112.10849123224503, -110.94270741299202, -109.29350963424746, -110.33477486966507, -112.19620157705627, -111.45484078395934, -111.86858843505124, -110.22491147345858, -108.96177661263177, -108.67862820579893, -107.55155410582937, -108.27984439169573, -108.72682528077233, -110.64231212183269, -109.32873093119183, -112.98564364754564, -110.78933114228725, -108.50921025910479, -107.91087245586935, -112.57350030929283, -111.75871577457525, -108.42095298945462, -112.31266064114303, -110.1295657579673, -109.67444664474456, -110.33749884929306, -109.16098218724147, -109.63554874360221, -109.15892392675141, -111.90580809179818, -108.81196712336858, -111.42223552606656, -109.90571484965518, -109.99739812086352, -111.64103850263211, -111.31463957090885, -110.61247447444549, -110.20960333715526, -110.1707327818923, -109.70412636554525, -110.97278093107532, -110.24386747740314, -109.81378546061525, -110.83784085086458, -109.77357954318757, -111.22663832948885, -111.14563050139252, -110.87152231402447, -110.34246044319893, -109.97174570657546, -110.23599592972218, -111.08206161770731, -110.0073315341242, -111.11748366902188, -112.04005964728601, -109.81290191679287, -109.68543639040858, -112.01143296194752, -110.13641850530031, -108.19348942447623, -109.7534468948808, -109.36697824644176, -97.56454580435337, -104.97829040517887, -108.1539132982256, -110.048991273122, -107.46172505860011, -110.49269280640675, -109.94209901400029, -109.38576869679022, -111.43699124347364, -110.89973083498887, -111.2994445418276, -109.25144782032437, -113.25676258473536, -110.82078737428088, -109.97779571182073, -113.36294799183014, -111.38584551238931, -112.17267897274873, -108.56430946159155, -112.06841286528645, -110.36822473102735, -109.54758527532016, -110.48190506674653, -110.03535695860182, -109.3951469796576, -112.41910682256774, -111.38124138857238, -109.37850389100952, -111.65544568836181, -111.55876881606889, -109.3029209617236, -109.20030046194076, -108.82610577621037, -110.53329453526098, -109.96090595542142, -109.67834229432077, -110.62303603007352, -109.8388817181171, -109.22430039793213, -108.92749786663613, -110.05794249283548, -109.58534943218437, -110.50493887507297, -109.96373022997366, -111.0645036323456, -111.28501675364454, -109.77386932343008, -108.8952247140968, -110.09242801628717, -112.90943444063141, -110.72299296247249, -109.39094335967056, -110.95165384057718, -109.59809519359453, -110.4978602309597, -109.67109981692639, -111.2489619905986, -110.0937750887109, -109.76771021128954, -108.32976315018955, -111.3058145792439, -111.09464974601362, -110.99797900696136, -109.174315000222, -109.630351559617, -110.26289147175856, -110.22688407202517, -109.96748050100612, -112.13247633583758, -110.59994952890855, -110.93023020153811, -109.22457750926695, -110.26162558926984, -110.09713110375579, -111.73858994918328, -109.78183160058515, -109.7603471824367, -110.96016892586911, -111.23309626937036, -109.83093663960678, -114.05354944347246, -111.58202863059464, -110.42281828744524, -110.9521484732059, -112.5120328206343, -111.614891937737, -109.84428787405484, -111.61119567831453, -110.43095563229411, -111.71833448430398, -110.01132196809407, -109.37558169247951, -109.14091380022785, -110.42663661754088, -110.3598013572826, -109.78207135281417, -109.94058843992468, -109.88210328447205, -108.6217811850147, -107.17834387173707, -110.6447226986756, -111.10704778101115, -111.24396771977769, -110.47849395539598, -110.75150631628034, -109.67662689396347, -109.23145032835053, -108.83780193265358, -109.43468321661163, -102.22521103859944, -106.90009867479111, -108.91580608784525, -109.58671397003187, -110.56692028436989, -108.75103142680105, -111.00795573084157, -110.75039085328763, -109.48222099288613, -111.8621134816908, -110.26507966786443, -108.885924716389, -109.30841399453053, -112.3188631425597, -111.05677697153163, -108.8268571902449, -109.63028152237679, -114.82339015806369, -107.03435216376964, -111.34847692589166, -109.61354114874855, -112.32687758049907, -109.59816404231358, -111.64248480241805, -111.84075757907273, -110.44017657636552, -110.15181635726277, -111.93813663582833, -109.11826378836209, -109.99779889778326, -109.927119030584, -109.4389650887841, -111.52448814187727, -111.38736268499642, -110.51920914917922, -108.64230614681055, -108.90307263595304, -110.57246891832371, -109.65575340646116, -109.80359672370373, -108.83368585528197, -111.09385004343437, -108.83430005497769, -112.37784208819113, -109.50005381621696, -109.67421750136593, -111.39664088797532, -109.70867599669316, -109.52498993629875, -111.12341349673187, -110.0484037026941, -109.55138667646308, -111.06614422098669, -109.4785941493091, -110.25724082617013, -110.93950616855716, -110.53487953881397, -111.45722057988401, -110.32393446412904, -110.34361936710438, -108.6610336097813, -109.53631603696368, -108.06930707969195, -107.68056561368934, -108.73860971027449, -108.87111384617579, -108.40433837098611, -110.55999576884835, -106.83832061167207, -108.28786975902513, -109.18482905697472, -107.81071696594883, -107.91047268802457, -108.79613111673706, -111.05361322310213, -109.97897453479862, -109.12920563729425, -111.20538391490288, -109.26286135293664, -111.31400407177502, -109.92167984752287, -110.70854322826071, -108.59406515713611, -109.69371333227458, -109.36664873267313, -110.35521729513704, -110.40667924006368, -112.0181844636846, -111.01529188207431, -110.59246505728431, -109.95068312717868, -110.75807466894047, -109.58596443762707, -111.12127793384956, -109.59041634463125, -111.56255571372793, -110.43405578864342, -108.39660324329928, -111.1420710307505, -113.64788483868595, -111.67645688353934, -111.36878760365944, -109.68523694561108, -110.11608766310304, -109.25670490330123, -110.73546181099229, -111.77855039399805, -107.9662794718261, -109.67483334602832, -109.891258579519, -110.24757768183042, -109.50202895993814, -110.07763831916637, -109.96891925839451, -110.97268925927641, -109.31698133827767, -112.27933593506792, -110.36206721075725, -109.47379463718867, -110.27836850941338, -110.63738280998388, -111.3611682777485, -110.72689155959884, -111.55480904927032, -111.16689658479412, -110.35555645743601, -111.56609319131051, -110.88279459952174, -114.73607246523177, -109.95813757295693, -107.64639932425493, -111.26486783320321, -112.03946356928121, -111.8915972448334, -110.35245920812773, -110.83155104803564, -110.67437747473863, -110.9959682920065, -110.7815352345103, -111.13722283763049, -112.54797265493127, -110.06894780898469, -111.65186554925783, -111.83545188116254, -110.65894756123697, -108.48458025065264, -112.43760714427981, -114.1368408201927, -110.40065777895025, -110.1066998945526, -108.60654239598591, -110.5716060205154, -110.74257357180736, -111.1136089342442, -111.53539811075092, -113.2559601458872, -109.2003227548348, -110.42285840441025, -111.4086884998834, -111.61503050693868, -110.8194303494779, -108.9701587059964, -112.58521089509063, -110.10873915265242, -112.43440038319561, -110.03468788439882, -111.57896603236308, -110.21939233582523, -109.03614470500777, -110.11738923539659, -109.55359574898291, -110.416473622654, -109.4626868574157, -111.17164025076731, -110.3579689035081, -109.04338716157822, -112.36157114517567, -109.32125615922843, -112.71105693789394, -110.11019129547768, -108.96439402555632, -111.107663418839, -111.48306369859839, -110.9317530461794, -107.98628540532181, -111.1636972328743, -110.47837837583148, -109.04649309175733, -110.27110334963734, -111.35803630614352, -110.77259078859605, -111.46352820533895, -111.16789261049541, -109.2376344776325, -111.6795794983659, -111.74292205167644, -109.40835022991612, -111.02163652600731, -108.79482078001607, -110.6718658416566, -111.08747067599332, -112.15383726791498, -109.47049126158717, -109.061574046483, -111.23993049318979, -111.02521156588335, -109.46012868444186, -110.13918914826291, -112.08180381836377, -110.61929875223015, -111.4424805369965, -111.43420275069585, -109.71347556238717, -110.24726273025648, -109.7860268673935, -109.94126895018422, -111.41948668868926, -108.90555991781676, -110.81242861886172, -109.65007052722677, -112.12672329335953, -110.01123170946096, -111.13980448279096, -113.92013682657084, -108.6000853867411, -110.66793592761913, -110.61237681642844, -110.00839105230496, -109.38083187034974, -109.46119372195675, -110.3708067287448, -108.55518656223285, -113.33935987443276, -111.92184778392033, -111.80820718236087, -107.36852757311246, -109.51077803361602, -110.066791721019, -108.756710558672, -107.91391289865918, -110.72851430959301, -111.39074956442978, -112.928843679455, -109.87348280521556, -112.21371750380071, -110.82495902297394, -109.94006136010094, -110.58757785050143, -110.2790091349881, -111.43884888223081, -108.09540986530712, -109.63783244641691, -110.19577975613292, -110.01690033746098, -112.75938920157155, -109.27158857362184, -111.19519821680541, -110.14381902425255, -110.45955291199236, -111.55660330002316, -110.75604254261134, -111.02122553784838, -111.6490091060193, -110.93362819419399, -110.49033159684308, -110.70789549836027, -110.41991882034145, -110.0264093421208, -109.18432746063652, -110.15292268755287, -112.40733942236504, -111.32869665965416, -110.95418667871114, -111.14291568823575, -111.75555369152653, -112.98146297069803, -109.73870744292117, -111.33806139459435, -110.18838799491355, -112.60408243005732, -110.26112648646833, -110.58257045107274, -109.75155437454112]}, ...(2 in all)]
  in  "FFT 1 Choice 1":u16(ring) items=["T1 Y", "T1 X", "T1 Sum", "T2 Y", "T2 X", "T2 Sum", "T1 FB X", "T1 FB Sum", "T2 FB X", "T2 FB Sum", "PSD Y", "PSD X", "PSD Y Sum", "none"]
  in  "FFT 2 Choice 1":u16(ring)=3 items=["T1 Y", "T1 X", "T1 Sum", "T2 Y", "T2 X", "T2 Sum", "T1 FB X", "T1 FB Sum", "T2 FB X", "T2 FB Sum", "PSD Y", "PSD X", "PSD Y Sum", "none"]
  in  "FFT 1 Choice 2":u16(ring)=1 items=["T1 Y", "T1 X", "T1 Sum", "T2 Y", "T2 X", "T2 Sum", "T1 FB X", "T1 FB Sum", "T2 FB X", "T2 FB Sum", "PSD Y", "PSD X", "PSD Y Sum", "none"]
  in  "FFT 2 Choice 2":u16(ring)=4 items=["T1 Y", "T1 X", "T1 Sum", "T2 Y", "T2 X", "T2 Sum", "T1 FB X", "T1 FB Sum", "T2 FB X", "T2 FB Sum", "PSD Y", "PSD X", "PSD Y Sum", "none"]
  in  "Compute FFT":bool
  in  "Reset FFT":bool
  in  "# Spectra to Ave.":dbl=25.0
  out "Ave. Time (s)":dbl=1.5
  out "1 Channel":waveform(dbl)(graph)={"t0"=timestamp(0 s since 1904-01-01), "dt"=1.4999999999999999e-05, "Y"=array[20000 elements], "attributes"=variant("NI_ChannelName"=variant(string "T1 Y"))}
  out "Slow mean":dbl=nan format="%0.2f"
  in  "Slow mean N ave.":dbl=1.0 min=1.0 step=1.0
  out "Mean Intensity":dbl=nan
  out "Sigma":dbl=nan
  out "Sigma/Mean":dbl=nan
  in  "Subtract mean":bool
  in  "High Res. Display":u16(ring) items=["T1 Y", "T1 X", "T1 Sum", "T2 Y", "T2 X", "T2 Sum", "T1 FB X", "T1 FB Sum", "T2 FB X", "T2 FB Sum", "PSD Y", "PSD X", "PSD Y Sum"]
  out "APD 1 Rate (Hz)":dbl format="%#_3p"
  in  "Tab Control":T4(tab)
  out "Stage Moving":bool
  in  "Read Cal":bool
  in  "Confocal Linescan":bool
  in  "Speed (nm/s)":dbl=100.0
  in  "Furthest Withdraw (MHz)":dbl=15.0
  in  "Confocal Image":bool
  in  "Round T1 X":bool caption="Round"
  in  "T1 offset_x (mV)":dbl=nan format="%#_2g"
  in  "T1 kappa_x (pN/nm)":dbl=nan min=0.0 step=0.001 format="%#_2g"
  out "Time (s)":dbl=6.12
  out "Total Time (s)":dbl=60.0
  in  "Start Saving":bool
  in  "Cal sets to save":u32=50 min=1 step=1
  in  "Comment (data description)":string="testing confocal setup"
  out "Calibrating Trap...":bool
  in  "Trap 2 (ON/OFF)":bool=TRUE
  in  "Trap 1 (ON/OFF)":bool=TRUE
  in  "Save Calibration":bool
  in  "N sets to save":u32=200 caption="N Sets"
  in  "Save N Sets":bool
  out "Save file name":path=path "C:/Data/110526/110526_022.dat"
  in  "Save ave N":dbl=500.0 caption="Averaging Factor"
  out "Saving...":bool
  in  "Stop Saving":bool
  out "Progress":u16(slide) scale=0.0..100.0
  out "Manipulating Trap":bool
  out "Buffer Status":dbl(slide) scale=0.0..1.0
  out "Overflow (data lost)":bool
  in  "Reset":bool
  out "Data Rate (Hz)":dbl=66666.66666666667 caption="Trap Data Rate (Hz)" format="%#_3p"
  out "Data Period (s)":dbl=1.4999999999999999e-05 caption="Trap Data Period (s)" format="%#_6p"
  out "Save Data Rate (Hz)":dbl=133.33333333333334 caption="Rate (Hz)" format="%#_6p"
  out "Save Data Period (s)":dbl=0.0075 caption="Period (s)" format="%#_6p"
  in  "T1 alpha_x (nm/V)":dbl=nan step=10.0 format="%#_3g"
  in  "T2 alpha_x (nm/V)":dbl=nan step=10.0 format="%#_3g"
  in  "T2 kappa_x (pN/nm)":dbl=nan min=0.0 step=0.001 format="%#_2g"
  in  "T2 offset_x (mV)":dbl=nan format="%#_2g"
  in  "BD 1 Frequency 2 (MHz)":dbl=80.0 caption="T2 X (MHz)" min=50.0 max=100.0 step=1.0 format="%#_6p"
  in  "Green Laser ON/Interlacing":bool=TRUE
  in  "Round T2 X":bool caption="Round"
  in  "AO1":dbl(slide) caption="Confocal Y (V)" min=0.0 max=10.0 step=0.01 scale=0.0..10.0 scale format="%_1f"
  in  "AO2":dbl(slide) caption="Confocal X (V)" min=0.0 max=10.0 step=0.01 scale=0.0..10.0 scale format="%_1f"
  in  "Trap Raster Scan":bool
  out "Raster Scanning...":bool
  in  "Trap Delta (MHz)":dbl=15.0 step=1.0
  in  "Trap Intensity\nSetpoints (V)":cluster{"Set 1":dbl, "Set 2":dbl}={"Set 1"=5.2, "Set 2"=6.6}
  in  "Index":dbl=1.0 caption="Save File Index" min=1.0 step=1.0
  in  "BD 1 Frequency 1 (MHz)":dbl=65.0 caption="T1 X (MHz)" min=50.0 max=100.0 step=1.0 format="%#_6p"
  out "Current Position":dbl[](array[numeric])=[4.2944, 4.91027471, 2.9278058] format="%7_7g"
  in  "Position Label 5":string="upper flow spot" caption="5"
  in  "Position 1 Label":string="Top capillary (SA beads)" caption="1"
  in  "Position 2 Label":string="Bottom capillary (AD) beads)" caption="2"
  in  "Position 3 Label":string="lower flow spot (ATP)" caption="3"
  in  "Position 4 Label":string="Dump beads" caption="4"
  out "Pump 3 cont disp":string="Left: ADig beads"
  out "Pump 1 cont disp":string="Right: DNA beads "
  in  "Ch 1 Inject Rate (ul/h)":dbl=50.0
  in  "Pump write delay (ms)":dbl=300.0
  in  "All Pump Parameters":T5={"Pump 1"={"Diameter (mm)"=4.61, "Units"=4.0, "Volume"=100.0, "Rate"=50.0}, "Pump 2"={"Diameter (mm)"=4.61, "Units"=3.0, "Volume"=0.0, "Rate"=0.0}, "Pump 3"={"Diameter (mm)"=4.61, "Units"=4.0, "Volume"=100.0, "Rate"=250.0}}
  in  "Ch 2 Inject Volume (uL)":dbl=100.0
  in  "Pump pause delay (ms)":u32
  in  "Ch 3 Inject Volume (uL)":dbl=100.0
  in  "Ch 3 Inject Rate (ul/h)":dbl=250.0
  in  "Flush Center Ch Volume (uL)":dbl=15.0
  in  "Flush Center Ch Rate (ul/m)":dbl=100.0
  in  "Inject Valve B":bool caption="Inject Pump 2\n(Flush Center)"
  in  "Total Volume\nFlushed (uL)":dbl
  in  "Tab Control 2":T6(tab)=enum."Feedback on Trap Intensity"
  in  "Restart RF":bool
  out "Total Counts (ticks)":u32=600
  in  "Trap ON/OFF X or Y Amp?":bool=TRUE
  in  "Oscillate Set 2":bool
  in  "Trap 1 ON":bool=TRUE
  in  "Number Interlace Sets":u8=3 min=1 max=3
  in  "DIO count 3 (ticks)":u32=200
  in  "DIO count 2 (ticks)":u32=200
  in  "DIO count 1 (ticks)":u32=200
  in  "BD 2 Amplitude 3 (%)":dbl min=0.0 max=75.0 step=1.0
  in  "BD 2 Amplitude 2 (%)":dbl min=0.0 max=75.0 step=1.0
  in  "BD 2 Amplitude 1 (%)":dbl min=0.0 max=75.0 step=1.0
  in  "BD 1 Amplitude 3 (%)":dbl min=0.0 max=75.0 step=1.0
  in  "BD 1 Amplitude 2 (%)":dbl=50.0 min=0.0 max=75.0 step=1.0
  in  "BD 1 Amplitude 1 (%)":dbl=50.0 min=0.0 max=75.0 step=1.0
  in  "BD 2 Frequency 3 (MHz)":dbl=26.0 min=50.0 max=100.0 step=1.0 format="%#_6p"
  in  "BD 1 Frequency 3 (MHz)":dbl=70.0 min=50.0 max=100.0 step=1.0 format="%#_6p"
  in  "BD 2 Frequency 2 (MHz)":dbl=26.0 min=50.0 max=100.0 step=1.0 format="%#_6p"
  in  "BD 2 Frequency 1 (MHz)":dbl=26.0 min=50.0 max=100.0 step=1.0 format="%#_6p"
  in  "Not-Interlacing Set":enum32{"Set 1", "Set 2", "Set 3"}(radio)
  in  "Interlace":bool=TRUE
  in  "Trap 2 ON":bool=TRUE
  in  "Trap 3 ON":bool
  in  "Scan axis 2":bool=TRUE
  in  "Osc. freq. (Hz)":dbl=0.25
  in  "Osc. amp. (MHz)":dbl=2.0 format="%1_3g"
  out "Coords":T7
  in  "Manipulation Scaling":cluster{"Horizontal":dbl, "Vertical":dbl}={"Horizontal"=0.075, "Vertical"=0.01}
  in  "Freq or Amp switch first":bool=TRUE
  in  "Swap F1 and F2":bool
  in  "Freq switch delay":u16
  in  "Amp switch delay":u16=5
  in  "Period":i64=2
  in  "MCL Step Increment (V_int)":dbl=3.0
  out "Time to Finish All (min)":dbl=0.122877 format="%#_2p"
  in  "Scan Speed (nm/s)":dbl=100.0
  in  "Scan Range (nm)":dbl=369.00000000000034
  in  "Step Size (nm)":dbl=1.0
  in  "MCL/AOM Scale Tweak":dbl=1.0
  in  "MCL Step Position Ratio":dbl=0.5
  in  "Move MCL Also?":bool=TRUE
  out "Final sep (nm)":dbl=114.0
  out "Initial sep (nm)":dbl=2943.0
  out "Save index":dbl=22.0
  out "Final delta (MHz)":dbl=18.0
  out "Initial delta (MHz)":dbl=41.0
  out "Final freq. (MHz)":dbl=62.0
  out "Initial freq. (MHz)":dbl=65.0
  in  "Saved AOD Raster Scan Parameter Sets":T8(array[cluster])=[{"Scan Range AOD (nm) 2"=500.0, "Step Size AOD (nm) 2"=1.0, "Scan Speed AOD (nm/s) 2"=100.0, "Number of scans (AOD) 2"=1, "Label"="offset curve"}, {"Scan Range AOD (nm) 2"=420.0, "Step Size AOD (nm) 2"=1.0, "Scan Speed AOD (nm/s) 2"=100.0, "Number of scans (AOD) 2"=1, "Label"="hp raster check"}, {"Scan Range AOD (nm) 2"=6.8, "Step Size AOD (nm) 2"=0.34, "Scan Speed AOD (nm/s) 2"=0.34, "Number of scans (AOD) 2"=1, "Label"="3.4 kbp - 1 bp steps"}]
  in  "Load parameters":bool
  out "Scan Range (MHz)":dbl=-3.0000000000000027
  in  "Restart DMA? (AOD)":bool=TRUE caption="Restart DMA?"
  out "Incr. int (AOD)":i64=-7759651845
  out "Time/Scan (s) (AOD)":dbl=3.68631 format="%#_2p"
  out "Data points/scans":dbl=491508.0
  out "Data points/scan (f/b)":dbl=491508.0
  in  "Save scans":bool=TRUE
  out "AOD Scan I":u64 caption="Scan I"
  in  "Continuous AOD Scanning":bool caption="Continuous Scanning"
  in  "Abort AOD Scan":bool caption="Abort Scan"
  in  "Scan BD":bool=TRUE
  out "Cycles/step (AOD)":u64=666 format="%.3p"
  in  "Number of F/B Scans (AOD)":u16=1 min=1
  out "Scan steps (AOD)":u64=369
  out "Scan Increment (MHz)":dbl=-0.008152173913043485
  out "AOD Scanning":bool caption="Scanning"
  in  "Start AOD Scan":bool caption="Start Scan"
  out "N sets should be saved":dbl=24.5754
  out "Progress 2":u16(slide) caption="Progress" scale=0.0..100.0
  in  "Abort save 2":bool caption="Abort save"
  in  "Trap 1 Bead Size (nm)":dbl=2100.0
  in  "Trap 2 Bead Size (nm)":dbl=2100.0
  out "MCL Count":dbl=230502201.82069838
  in  "All FB On/Off":bool
  in  "AI2 to Setpoint":cluster{"Set 1":bool, "Set 2":bool}
  out "AI2 (V)":cluster{"Set 1":dbl, "Set 2":dbl}={"Set 1"=5.203711050752282, "Set 2"=5.442060609759819}
  in  "Reset Feedback":cluster{"Set 1":bool, "Set 2":bool}
  in  "PID Gains":T9={"Set 1"={"proportional gain (Kc)"=0, "integral gain (Kc*Ts/Ti)"=5, "derivative gain (Kc*Td/Ts)"=0}, "Set 2"={"proportional gain (Kc)"=0, "integral gain (Kc*Ts/Ti)"=5, "derivative gain (Kc*Td/Ts)"=0}}
  in  "Feedback On/Off":cluster{"Set 1":bool, "Set 2":bool}={"Set 1"=TRUE, "Set 2"=TRUE}
  in  "Set SP to Reading":bool
  out "Trap X (AI1)":T10={"Trap 1"=0.00885009765625, "Trap 2"=0.001068115234375}
  in  "Trap Pos FB SP":fxp<+/-,16,1>=-0.092803955078125 caption="Setpoint"
  in  "Trap Pos. FB ON":bool
  in  "Reset Trap Pos. FB":bool
  out "Trap Positions":waveform(dbl)[](graph)=[{"t0"=timestamp(68.39999999999971 s since 1904-01-01), "dt"=0.15, "Y"=[3.495870259939693e-12, 3.495870259939693e-12], "attributes"=variant("NI_ChannelName"=variant(string "Trap 1 Pos."))}, {"t0"=timestamp(68.39999999999971 s since 1904-01-01), "dt"=0.15, "Y"=[-1.7479351299698465e-12, -1.7479351299698465e-12], "attributes"=variant("NI_ChannelName"=variant(string "Trap 2 Pos."))}]
  in  "Tab Control 8":enum32{"Main Setting", "Details"}(tab)
  in  "Trap Pos FB Int Count":u16=100
  in  "Trap Pos. FB Gains":T11={"proportional gain (Kc)"=10.0, "integral gain (Kc*Ts/Ti)"=10.0, "derivative gain (Kc*Td/Ts)"=0.0} {"proportional gain (Kc)" format="%.11g"; "integral gain (Kc*Ts/Ti)" format="%.11g"; "derivative gain (Kc*Td/Ts)" format="%.11g"}
  in  "Trap Pos. FB Offset Factor":i64
  in  "Trap Pos FB Negate Action":bool
  in  "Trap Pos. FB Mult Factor":i64=33554432
  in  "Trap Pos. AI1 X Pre-scale":u16
  in  "Trap Pos. FB Range":T12={"output high"=0.999969482421875, "output low"=-1.0}
  out "Trap Pos FB Int Signal":fxp<+/-,24,9> format="%.18g"
  out "Trap Pos FB Int-Norm Signal":fxp<+/-,16,1> format="%.16g"
  in  "Set SP Using...":bool
  in  "Trap Pos FB Monitor\nT1 or T2":bool
  out "Trap X AI1 (DMA)":T13={"Set 1"=0.007598876953125, "Set 2"=-9.1552734375e-05}
  in  "N El. to Ave.":dbl=10000.0
  out "Trap Pos FB Action":i64
  out "Action (%)":dbl(knob) scale=-100.0..100.0
  in  "Trap Pos. FB Out Scale 2^n":u8=23 caption="Action Scale"
  out "Mean T1 Position (nm)":dbl=3.495870259939693e-12 caption="Mean T1 (nm)" format="%0.2f"
  out "Trap 1 Position RMS (A)":dbl caption="RMS (Ang)"
  in  "Tab Control 3":enum32{"Timing", "MCL Scan", "Analog Out"}(tab)
  out "APD 2 Gate Late Counter":u32
  out "APD 2 Gate Relative Phase":i16
  in  "Phase Adj. (APD 2 Gate)":i16=20
  in  "Initial Phase Adjustment (APD 2 Gate)":i16=55
  out "APD 1 Gate Late Counter":u32
  in  "- phase (APD 1 Gate)":bool
  in  "+ phase (APD 1 Gate)":bool
  out "APD 1 Gate Relative Phase":i16
  in  "Phase Adj. (APD 1 Gate)":i16=20
  in  "Initial Phase Adjustment (APD 1 Gate)":i16=60
  in  "Save APD Data\nwith Trap Data":bool=TRUE
  out "APD FIFO Elements Remaining":u32
  in  "- phase (APD Acq)":bool
  in  "+ phase (APD Acq)":bool
  out "APD Acq Late Counter":u32
  out "APD Acq Relative Phase":i16
  in  "Phase Adj. (APD Acq)":i16=20
  in  "Initial Phase Adjustment (APD Acq)":i16
  in  "Invert APD Gate":bool caption="Invert Gate"
  in  "APD Gate OFF Count":u32=450 caption="Gate OFF Count"
  in  "APD Gate ON Count":u32=150 caption="Gate ON Count"
  in  "APD Gate":enum32{"ON", "OFF", "Interlace"}(radio)=enum."Interlace"
  in  "APD Integration Time (s)":dbl=0.01 caption="Integration Time (s)"
  out "APD Acq Rate (Hz)":dbl=100.0 caption="Rate (Hz)"
  out "APD Samples/FIFO Acq.":dbl=30.0
  out "APD Elements/DMA read":u32=60
  out "APD Int. Count":u32=400000 format="%.0p"
  in  "+ phase (APD 2 Gate)":bool
  in  "- phase (APD 2 Gate)":bool
  in  "Tab Control 5":enum32{"PSD X", "PSD Y", "Other Data Channel"}(tab)
  out "Data map":dbl[][](graph)
  in  "Channel":i32=4
  in  "Abort MCL Scan":bool
  out "MCL Scan I":u64
  out "MCL Scanning":bool
  in  "Start MCL Scan":bool
  out "wait to reset values":bool
  in  "Tab Control 4":enum32{"Scan Settings", "MCL FPGA Loop Timing"}(tab)
  out "Total Time (s)":dbl=48.0
  in  "Scan lines (y)":u64=20
  in  "Fast Scan Dir":bool=TRUE
  in  "2D or 1D Scan":bool=TRUE
  out "Initial X":dbl
  out "Initial Y":dbl
  out "Time/f+b scan (s) (MCL)":dbl=2.4 caption="Time/scan (s)"
  in  "Number of scans (MCL)":u64=1 caption="Scans"
  in  "Scan steps (MCL)":u64=40 caption="Scan steps (x)"
  in  "N APD Samp/step":dbl=3.0
  in  "Scan Range (V)\n(of steps)":dbl=3.5
  in  "Restart DMA? (MCL)":bool=TRUE caption="Restart DMA?"
  in  "Continuous MCL Scanning":bool caption="Cont. Scanning"
  in  "Center Scan":bool=TRUE
  in  "Save Data (MCL)":bool=TRUE caption="Save Data"
  out "Actual Incr. int (MCL)":i16=294 caption="Incr. int"
  out "Desired incr (int)":dbl=294.0628205128205
  out "Desired Scan Incr (V)":dbl=0.08974358974358974
  out "N sets should be saved (MCL)":dbl=160.0 caption="N sets should be saved"
  out "Data points/scans (MCL)":dbl=4800.0 caption="Data points/scans"
  out "Data points/scan (f+b)":dbl=240.0 caption="points/scan (f+b)"
  out "Cycles/step (MCL)":u64=2000 caption="Cycles/step" format="%.0p"
  out "Actual MCL Inc (V)":dbl=0.08972441785943175
  in  "Phase adjust (MCL)":i16 caption="Phase adjust"
  out "Relative Phase (MCL)":i16 caption="Relative Phase"
  in  "Initial Phase Adj. (MCL)":i16 caption="Initial Phase Adj."
  in  "Update Count (MCL)":u32=600
  in  "+ phase (MCL)":bool
  in  "- phase (MCL)":bool
  out "MCL Late Counter":u32
  in  "APD 1 AO Mult.":i16=1 min=1
  in  "APD 2 AO Mult.":i16=1 min=1
  in  "Tab Control 7":enum32{"Green FB Signals", "Slow MCL Scan"}(tab)
  out "Green FB Plot":dbl(graph)=-10.00030518509476
  out "MCL Scan 2":cluster{"Begin (V)":dbl, dbl, dbl[]}(graph)
  out "MCL Scan":cluster{"Begin (V)":dbl, dbl, dbl[]}(graph)
  in  "Green laser mode":enum32{"Laser ON", "Laser OFF", "Interlace"}(radio)
  in  "GI Frequency, ON count":u32=150 min=1 step=1
  in  "Invert GI":bool
  out "GI Late Counter":u32
  in  "Phase adj. (GI)":i16=5
  out "GI relative phase":i16
  in  "+ phase (GI)":bool
  in  "Initial Phase Adjustment (GI)":i16=19
  in  "GI Frequency, OFF count":u32=450 min=1 step=1
  in  "- phase (GI)":bool
  out "Green FB Signals (V)":cluster{"Y":dbl, "X":dbl, "Sum":dbl}={"Y"=-0.999969482421875, "X"=1.0, "Sum"=-10.00030518509476}
  out "Relative phase (Green FB)":i16
  in  "+ phase (Green FB)":bool
  in  "- phase (Green FB)":bool
  in  "Green FB Count":u32=600
  in  "Phase adj. (Green FB)":i16=10
  in  "Initial Phase Adjustment (Green FB)":i16=50
  in  "Green FB On/Off":bool
  in  "Current When FB OFF (%)":dbl=10.0 min=0.0 max=100.0 step=1.0
  in  "Green int current ON count adj":u32=150
  in  "Green FB Gains":T14={"proportional gain (Kc)"=10, "integral gain (Kc*Ts/Ti)"=5, "derivative gain (Kc*Td/Ts)"=0}
  in  "Green FB Setpoint (mV)":dbl=100.0
  in  "- phase (GI) 2":bool
  in  "Initial Phase Adjustment (GI) 2":i16=-100
  in  "+ phase (GI) 2":bool
  out "GI relative phase 2":i16
  in  "Phase adj. (GI) 2":i16=20
  out "GI Late Counter 2":u32
  in  "Trap Position FIFO Depth":u32=300000 format="%.0p"
  in  "# Samples/trap":u32=20000 format="%.0p"
  out "Trap AI Elements/DMA read":u32=320000 format="%.0p"
  out "Ave. Rate (Hz)":dbl=200000.0 format="%#_6p"
  out "Trap AI FIFO El. Rem.":u32 format="%.0p"
  in  "Phase adj. (AI1)":i16
  out "Relative phase (AI1)":i16
  in  "+ phase (AI1)":bool
  in  "- phase (AI1)":bool
  out "Late Counter (AI1)":u32
  in  "Initial Phase Adjustment (AI1)":i16=180
  out "AI rate (Hz)":dbl=200000.0 format="%#_6p"
  in  "AI Count (ticks)":u32=200
  out "# Samples/channel":u32=40000 format="%.0p"
  in  "Trap AI FIFO Depth":u32=340000 format="%.0p"
  in  "Detector Type":string(combo)="UCB Fleezers 052511"
  in  "N Acq Sets (Traps + Fl.)":i16=3
  in  "Sets to FIFO (Traps)":T15={"Set 1"=TRUE, "Set 2"=TRUE, "Set 3"=FALSE}
  in  "FPGA Ave.":dbl=1.0 min=1.0 step=1.0
  out "Ave. Period (s)":dbl=5e-06 format="%#_6p"
  out "DMA Update Period (s)":dbl=0.3
  out "FPGA Averaging":bool
  out "Trap Sets":u32=2
  out "Counts/DMA":dbl=12000000.0 format="%#_6p"
  out "Trap Pos FIFO El Remaining":u32=153
  out "Trap Pos Elements/DMA read":u32=120000 format="%.0p"
  out "Trap AI FIFO Timeout":u16
  out "Trap Pos FIFO Timeout":u16
  out "Waveform Chart":i32(graph)=320000
  out "error out 2":errorcluster
  in  "Lost Tether Alarm Threshold (pN)":dbl=0.5
  in  "AOM X Cal (nm/MHz)":dbl=123.0
  in  "MCL X Cal (nm/V)":dbl=1070.0
  out "X RF Amplitude Limits (%)":T16={"Minimum"=0.0, "Maximum"=75.0, "Increment"=1.0}
  out "X RF Frequency Limits (MHz)":T16={"Minimum"=50.0, "Maximum"=100.0, "Increment"=1.0}
  out "Y RF Frequency Limits (MHz)":T16={"Minimum"=50.0, "Maximum"=100.0, "Increment"=1.0}
  out "Y RF Amplitude Limits (%)":T16={"Minimum"=0.0, "Maximum"=75.0, "Increment"=1.0}
  in  "Manip. X?":bool=TRUE
  in  "Manip. Y?":bool
  in  "Force Manip Abort":bool
  out "Read cal error":errorcluster
  in  "DAQ Delay (ms)":u32=1000
  in  "Start Scan":bool
  in  "Scan axis":bool
  in  "Osc. amp. (V)":dbl=5.0
  in  "Osc. center (V)":dbl=5.0
  in  "Osc. freq. (Hz) 2":dbl=1.0
  in  "MCL Mode":u16(ring) items=["Manual Positioning", "Sinusoidal Wave", "Linear Scan"]
  in  "Begin (V)":dbl
  in  "End (V)":dbl=10.0
  in  "N Points":dbl=20.0
  in  "Delay to Interlace (s)":dbl
  in  "Delayed Interlace Start":bool
  in  "Read Lateness and Rel Phase":bool
  out "Vec Mean of T1 T2":dbl[](array[numeric])=[0.003812506939223503, 0.003853383633104548]
  in  "Cal read wait (s)":u32=5
  out "Time tether formed":timestamp=timestamp(3371146929.513132 s since 1904-01-01)
  in  "Chemyx Syringe Pump Serial Port":refnum<visa-resource-name>="ASRL3::INSTR"
  in  "Limit Min (MHz)":dbl=10.0 caption="Min (MHz)"
  in  "Limit Max (MHz)":dbl=16.0 caption="Max (MHz)"
  in  "Limits Enable":bool=TRUE caption="Enable"
  out "AI labels":string[](array[string])=["T1 Y", "T1 X", "T1 Sum", "T2 Y", "T2 X", "T2 Sum", "T1 FB X", "T2 FB Sum", "T2 FB X", "T2 FB Sum", "PSD Y", "PSD X", "PSD Sum"]
  in  "Save Trap Pos. Data":bool=TRUE
  in  "ESP Port":refnum<visa-resource-name>="COM22"
  in  "Locations":i32(listbox)=1
  out "Selected Location":cluster{"x":string, "y":string, "z":string}={"x"="N.D.\r\n", "y"="N.D.\r\n", "z"="N.D.\r\n"}
  in  "Capture":bool
  in  "Save":bool
  in  "Goto Top (F6)":bool
  in  "Goto Exp (F8)":bool
  in  "Goto Bottom (F7)":bool
  in  "Axis 3":string="0.00500\r\n"
  in  "Axis 2":string="0.00500\r\n"
  in  "Axis 1":string="0.00500\r\n"
  in  "Axis 3":string="0.20000\r\n"
  in  "Axis 2":string="0.20000\r\n"
  in  "Axis 1":string="0.20000\r\n"
  in  "Activate Joystick":bool
  in  "ESP ZL-Limit":string="-0.09900"
  in  "ESP ZR-Limit":string="0.09900"
  out "Z Pos Pos":string="1\r\n"
  out "Y Pos":string="0.00000\r\n"
  out "X Pos":string="0.00000\r\n"
  in  "error in":errorcluster
  out "error out":errorcluster
  out "Z motion":string="0.00000\r\n"
  out "Y Motion":string="1\r\n"
  out "X Motion":string="1\r\n"
  # "After"
  # "During"
  # "Trap On?"
  # "BD Flow ON?"
  # "Samp Flow ON?"
  # "1"
  # "2"
  # "Trap Display:"
  # "APD Display:"
  # "originally 10k"
  # "Trap Manipulation"
  # "DAQ"
  # "Data Saving"
  # "F9"
  # "Bead Calibration"
  # "F10"
  # "F4"
  # "Press F12 to move stage\nwith the mouse. F12 to cancel."
  # "F5"
  # "F6"
  # "F7"
  # "F8"
  # "Harvard Pump\n(sample channel for flow exp)"
  # "Chemyx Pump 2"
  # "Units: \n1 = ml/m\n2 = ml/h\n3 = ul/m\n4 = ul/h"
  # "Rate param is ul/h\nVolume param is ul"
  # "X"
  # "Y"
  # "Oscillate Set 2 freq. (debugging)"
  # "BD 1"
  # "BD 2"
  # "AOD Raster Scan"
  # "Approx. trap separations"
  # "X"
  # "Y"
  # "DON'T TURN ON\nUNTIL YOU CLOSE\nTHE LOOP"
  # "FPGA\nreading"
  # "DMA\ntransfer"
  # "APD Gates"
  # "APD 2"
  # "APD 1"
  # "X"
  # "2D"
  # "Y"
  # "1D"
  # "Green Laser Interlacing"
  # "Green FB Measurement"
  # "Digital Gate"
  # "Current Analog Control"
  # "was 87"
  # "originally 600k"
  # "Total AI Rates (NOT rates/trap)"
  # "originally 20k"
  # "(Samples/trap x Trap Sets)"
  # "(Samples/channel x\n8 if averaging (8 channels)\n4 if no averaging)"
  # "Trap 1"
  # "Trap 2"
  # "Flour./Trap 3"
  # "External Video Window"
  # "MCL Position Debugging"
  # "Temporary Control Storage\n(these used to be somewhere else, still want to keep them)"
  # "Y"
  # "X"
  # "Trap Position Difference Limits"
  # "Joystick Control"
  # "Setting Limit for the z-axis"
  # "Current Location"
  # "Save Positions of Cambers"
  # "Errors detected in determing Current Location"
  # "High Jog Velocity"
  # "Low Jog Velocity"
  # "Select the chamber to go to"
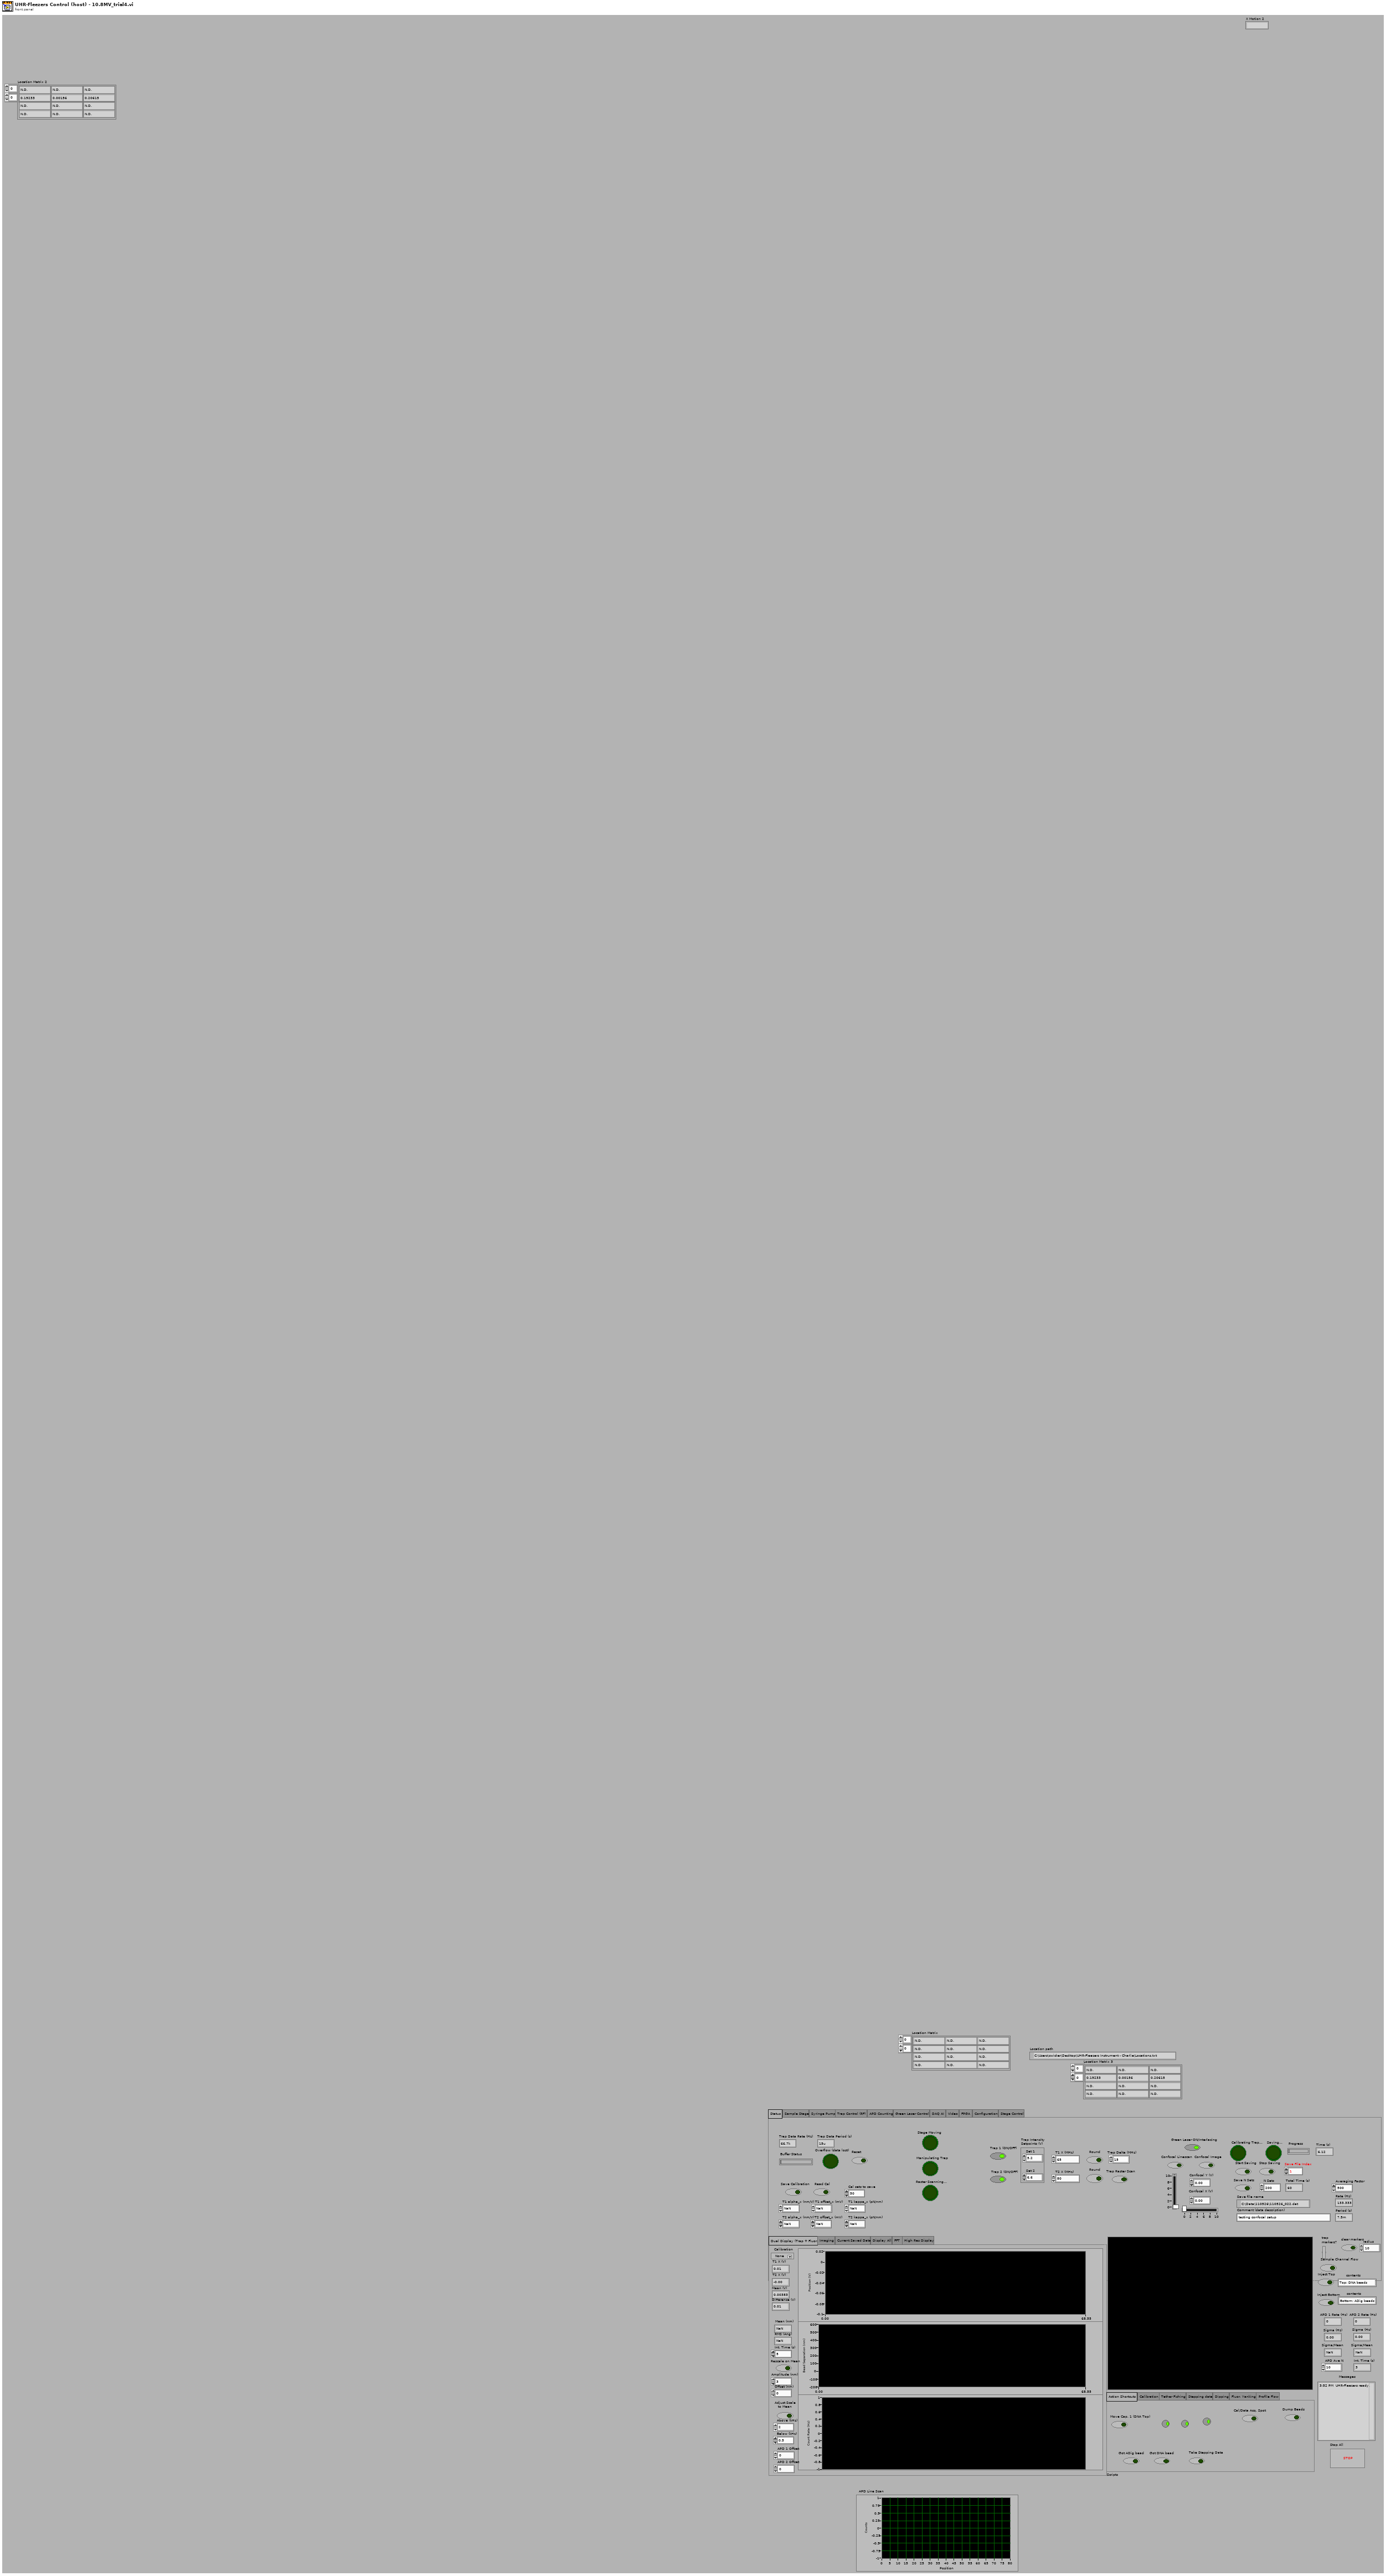
[diagram p1: front panel]
types:
  T1 = enum32{"Action Shortcuts", "Calibration", "Tether Fishing", "Stepping data", "Dipping", "Fluor. Yanking", "Profile Flow"}
  T2 = typedef "IMAQ Image.ctl" = refnum<image>
  T3 = enum32{"Dual Display (Trap + Fluor.)", "Imaging", "Current Saved Data", "Display All", "FFT", "High Res Display"}
  T4 = enum32{"Status", "Sample Stage", "Syringe Pump", "Trap Control (RF)", "APD Counting", "Green Laser Control", "DAQ AI", "Video", "FPGA", "Configuration", "Stage Control"}
  T5 = cluster{"Pump 1":cluster{"Diameter (mm)":dbl, "Units":dbl, "Volume":dbl, "Rate":dbl}, "Pump 2":cluster{"Diameter (mm)":dbl, "Units":dbl, "Volume":dbl, "Rate":dbl}, "Pump 3":cluster{"Diameter (mm)":dbl, "Units":dbl, "Volume":dbl, "Rate":dbl}}
  T6 = enum32{"IR Laser Interlacing (Direct RF Board Control Method)", "AOD Raster Scan", "Feedback on Trap Intensity", "Feedback on Trap Position"}
  T7 = typedef "LVPoint32TypeDef.ctl" = cluster{"Horizontal":i32, "Vertical":i32}
  T8 = cluster{"Scan Range AOD (nm) 2":dbl, "Step Size AOD (nm) 2":dbl, "Scan Speed AOD (nm/s) 2":dbl, "Number of scans (AOD) 2":u16, "Label":string}[]
  T9 = cluster{"Set 1":cluster{"proportional gain (Kc)":i16, "integral gain (Kc*Ts/Ti)":i16, "derivative gain (Kc*Td/Ts)":i16}, "Set 2":cluster{"proportional gain (Kc)":i16, "integral gain (Kc*Ts/Ti)":i16, "derivative gain (Kc*Td/Ts)":i16}}
  T10 = cluster{"Trap 1":fxp<+/-,16,1>, "Trap 2":fxp<+/-,16,1>}
  T11 = cluster{"proportional gain (Kc)":fxp<+/-,16,8>, "integral gain (Kc*Ts/Ti)":fxp<+/-,16,8>, "derivative gain (Kc*Td/Ts)":fxp<+/-,16,8>}
  T12 = cluster{"output high":fxp<+/-,16,1>, "output low":fxp<+/-,16,1>}
  T13 = cluster{"Set 1":fxp<+/-,16,1>, "Set 2":fxp<+/-,16,1>}
  T14 = cluster{"proportional gain (Kc)":i16, "integral gain (Kc*Ts/Ti)":i16, "derivative gain (Kc*Td/Ts)":i16}
  T15 = cluster{"Set 1":bool, "Set 2":bool, "Set 3":bool}
  T16 = typedef "LVMinMaxIncTypeDef.ctl" = cluster{"Minimum":dbl, "Maximum":dbl, "Increment":dbl}
  T17 = typedef "Image Type" = u32
  T18 = typedef "nirio_resource_hc.ctl" = tag
  T19 = typedef "openfpgaref.8.6.ctl" = refnum<k20>
  T20 = enum16{"CONNECT", "INITIALIZE VALVES", "DISCONNECT", "MOVE VALVE"}
  T21 = cluster{"New Image":T2, "New Image":T2, "New Image":T2, "New Image":T2}
  T22 = cluster{"Location Matrix[0]":string, "Location Matrix[1]":string, "Location Matrix[2]":string}
  T23 = enum16{"open", "replace", "create", "open or create", "replace or create", "replace or create with confirmation"}
  T24 = typedef "XDNodeRunTimeDep.lvlib/timing_clust.ctl" = cluster{"Expected End [f-1]":u64, "Actual End [f-1]":u64, "Finished Late? [f-1]":bool, "Expected End [i-1]":u64, "Actual End [i-1]":u64, "Finished Late? [i-1]":bool, "Expected Start [i]":u64, "Actual Start [i]":u64, "Expected Start [f]":u64, "Actual Start [f]":u64, "Source Name":string, "Structure Name":string, "Period":i64, "Deadline":i64, "Offset":i64, "Start":i64, "Priority":i32, "Timeout":i32, "Mode":T25, "Wakeup Reason":T26, "Error":errorcluster, "Source Type":string, "Secondary Source Type":string, "Global End Time":u64, "Global Start Time":u64, "Frame Duration":u64, "Iteration Duration":u64, "Assigned CPU":i32, "I/O Scan Engine Mode":u32}
  T25 = typedef "XDNodeRunTimeDep.lvlib/nitl_modes.ctl" = enum32{"No Change", "Process missed periods, maintain original phase", "Discard missed periods, maintain original phase", "Process missed periods, ignore original phase", "Discard missed periods, ignore original phase"}
  T26 = typedef "XDNodeRunTimeDep.lvlib/wakeup.ctl" = enum32{"Normal", "Aborted", "Asynchronous wakeup", "Timing source error", "Timed loop error", "Timeout"}
  T27 = cluster{"[0]":i32, "[1]":i32, "[2]":i32, "[3]":i32}
  T28 = cluster{"[0]":i32, "[1]":i32, "[2]":i32, "[3]":i32}[]
  T29 = enum16{"big-endian, network order", "native, host order", "little-endian"}
  T30 = cluster{"Scan Range AOD (nm) 2":dbl, "Step Size AOD (nm) 2":dbl, "Scan Speed AOD (nm/s) 2":dbl, "Number of scans (AOD) 2":u16, "Label":string}
  T31 = cluster{"[0]":dbl, "[1]":dbl, "[2]":dbl, "[3]":dbl, "[4]":dbl, "[5]":dbl}
  T32 = cluster{"Diameter (mm)":dbl, "Units":dbl, "Volume":dbl, "Rate":dbl}
  T33 = cluster{"Left":i32, "Top":i32, "Width":u32, "Height":u32}
  T34 = cluster{cluster{"Left":i32, "Top":i32, "Width":u32, "Height":u32}}[]
  T35 = enum32{"Normal Display", "Dual Display (APD)", "FFT", "High Res Display"}
  T36 = cluster{"Origin Pixel":cluster{"X":sgl, "Y":sgl}, "Angle Relative to Horizontal (deg)":sgl, "Axis Reference":u32}
  T37 = typedef "Simple Grid Descriptor" = cluster{"X Step":sgl, "Y Step":sgl, "Unit":T38}
  T38 = typedef "Image Unit" = enum32{"Undefined", "Angström", "Micrometer", "Millimeter", "Centimeter", "Meter", "Kilometer", "Microinch", "Inch", "Feet", "Nautical miles", "Standard miles", "Steps"}
  T39 = cluster{"averaging mode":u16, "weighting mode":u16, "number of averages":u32}
  T40 = cluster{"dB On (F)":bool, "unwrap phase (F)":bool, "convert to degree (F)":bool}
  T41 = cluster{string, string, string, string, string, string, string, string}
  T42 = cluster{string, string, string, string, string, string, string, string, string, string, string, string}
  T43 = cluster{string, string, string, string, string, string, string, string, string, string, string, string, string}
  T44 = cluster{string, string, string, string, string, string, string, string, string, string, string, string, string, string}
  T45 = cluster{"BD 1 Frequency 1 (MHz)":dbl, "BD 1 Frequency 2 (MHz)":dbl}
  T46 = cluster{"f0":dbl, "df":dbl, "magnitude":dbl[]}[][]
  T47 = cluster{"Green FB Ch 0":i16, "Green FB Ch 1":i16, "Green FB Ch 2":i16}
  T48 = cluster{"Green FB Ch 0":dbl, "Green FB Ch 1":dbl, "Green FB Ch 2":dbl}
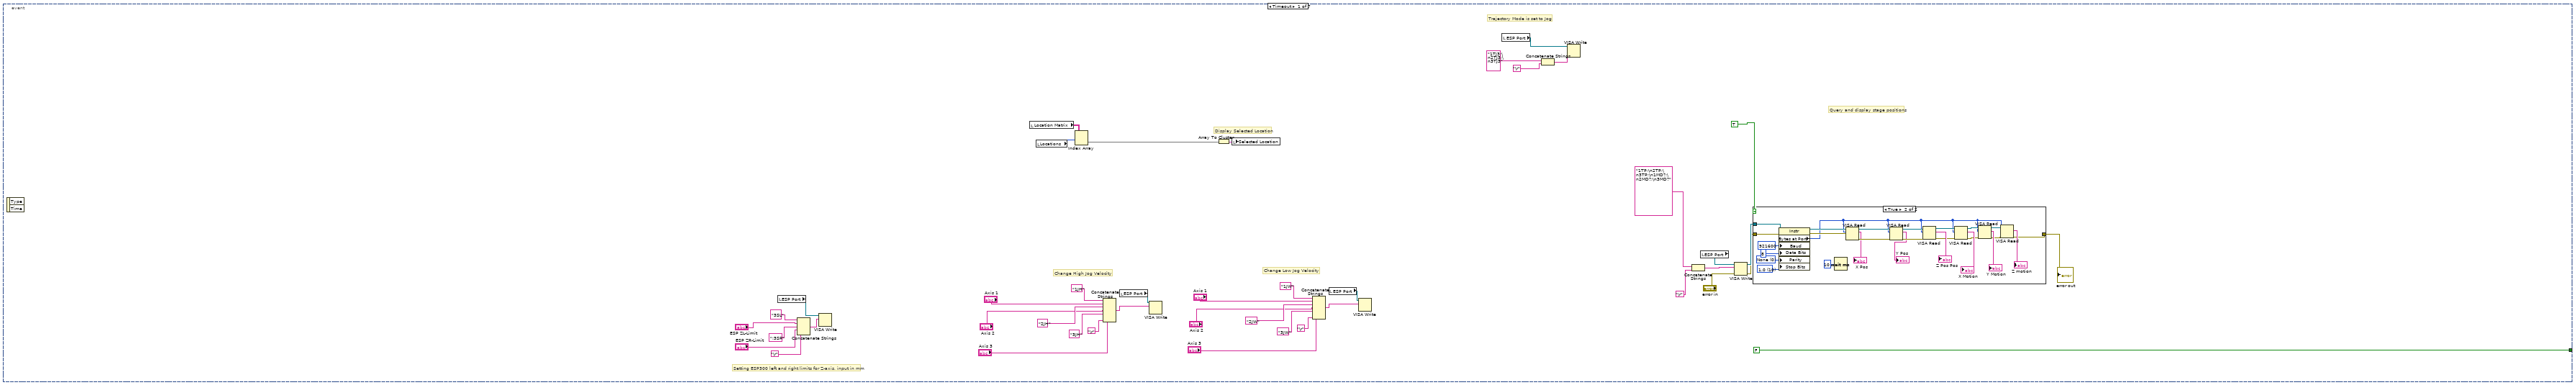
[diagram p2: hidden frame]
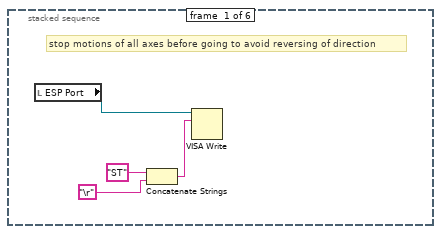
[diagram p4: hidden frame]
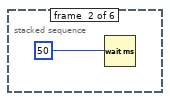
[diagram p5: hidden frame]
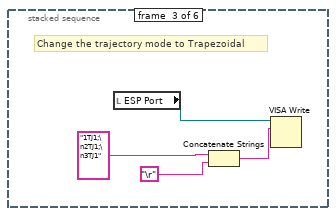
[diagram p6: hidden frame]
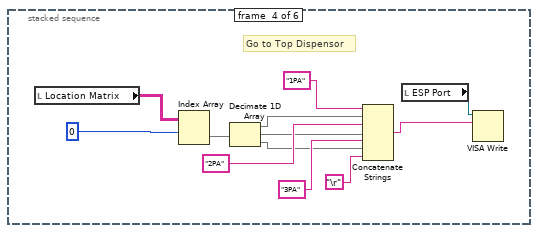
[diagram p7: hidden frame]
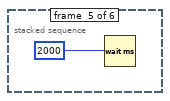
[diagram p8: hidden frame]
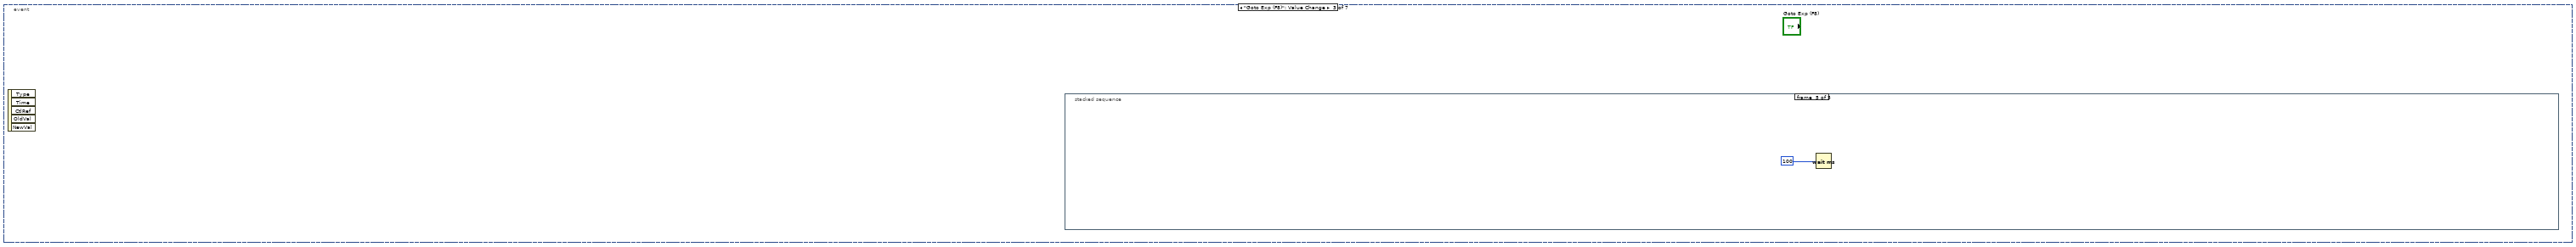
[diagram p9: hidden frame]
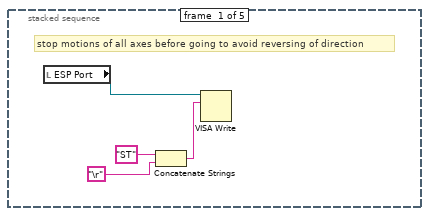
[diagram p10: hidden frame]
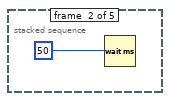
[diagram p11: hidden frame]
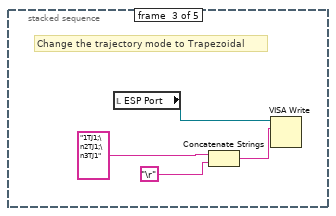
[diagram p12: hidden frame]
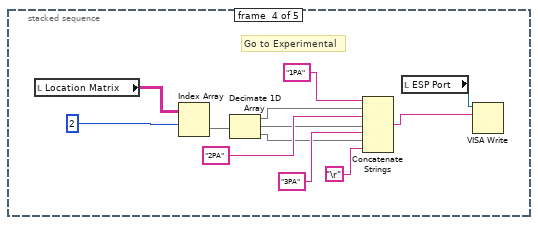
[diagram p13: hidden frame]
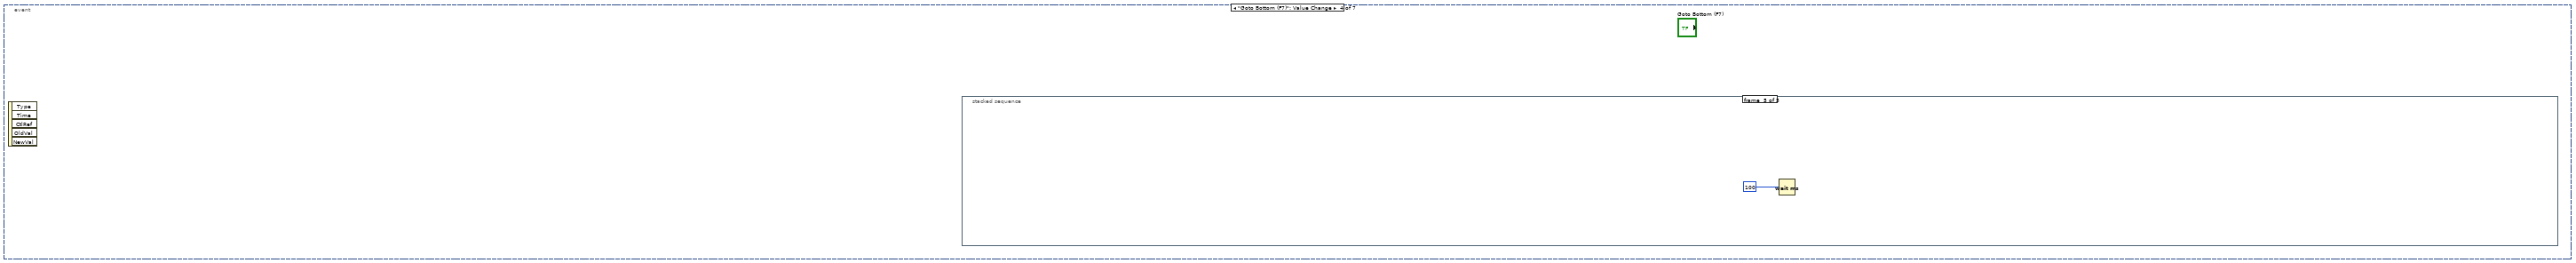
[diagram p14: hidden frame]
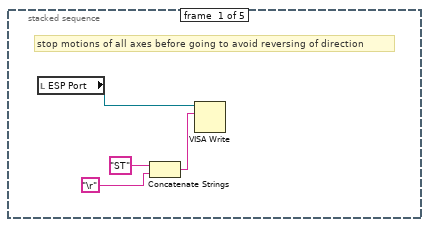
[diagram p15: hidden frame]
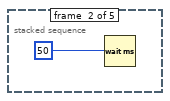
[diagram p16: hidden frame]
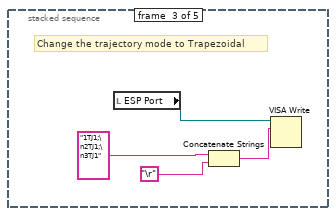
[diagram p17: hidden frame]
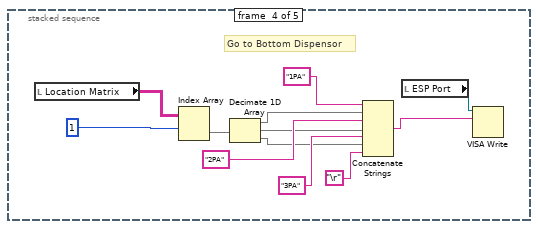
[diagram p18: hidden frame]
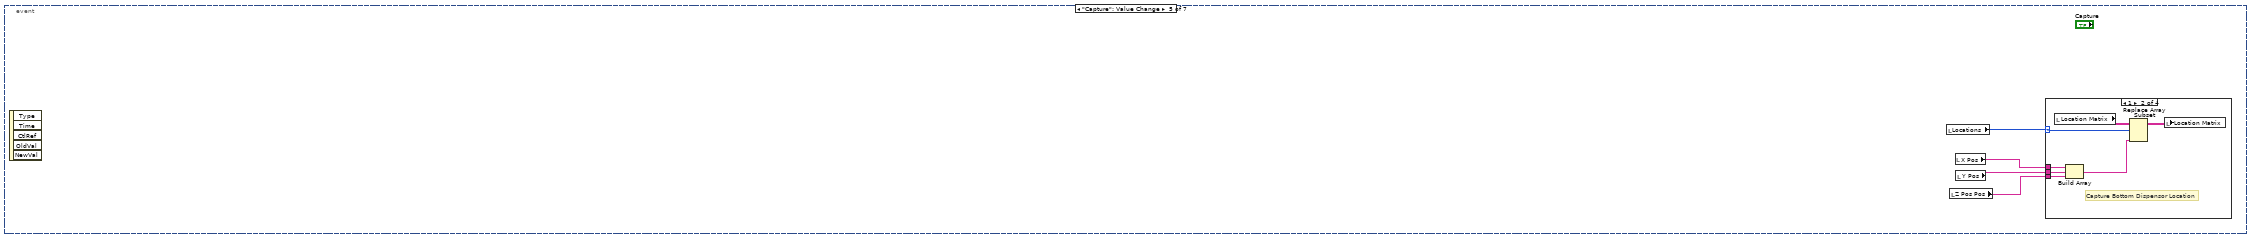
[diagram p19: hidden frame]
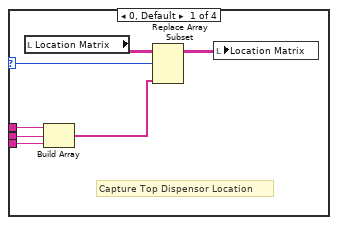
[diagram p20: hidden frame]
diagram:
  w64 = T17 2 items=["Grayscale (U8)", "Grayscale (I16)", "Grayscale (SGL)", "Complex (CSG)", "RGB (U32)", "HSL (U32)", "RGB (U64)", "Grayscale (U16)"] ("Image Type")
  w121 = cluster{"output high":i16, "output low":i16} {"output high"=3000, "output low"=0} ("FB output range 1")
  w196 = 10.0 ("y")
  w195 = 32767.0 ("y")
  w211 = 6.0  # clock mult.
  w212 = 49152000.0  # TCXO frequ.
  # "Initialize location matrix"
  n1 = Build Array("DIO count 1 (ticks)", "DIO count 2 (ticks)", "DIO count 3 (ticks)") -> (w110:u32[])
  n2 = Multiply(x="APD Integration Time (s)", y=40000000.0) -> (x*y=w128:dbl)
  n3 = Reciprocal(x="APD Integration Time (s)") -> (1/x=w125:dbl)
  n4 = local write "APD Acq Rate (Hz)"(w125) -> ()
  n5 = local read "AO1"() -> (w190:dbl)
  n6 = local read "AO2"() -> (w189:dbl)
  n7 = To Unsigned Long Integer(number=w128) -> (unsigned 32bit integer=w127:u32)
  "APD Int. Count" <- w127
  n8 = local read "Scan Increment (MHz)"() -> (w207:dbl)
  n9 = local read "Continuous MCL Scanning"() -> (w177:bool)
  n10 = local read "Fast Scan Dir"() -> (w176:bool)
  n11 = local read "Trap Intensity\nSetpoints (V)"() -> (w226:cluster{"Set 1":dbl, "Set 2":dbl})
  n12 = local read "Number of scans (MCL)"() -> (w178:u64)
  n13 = Multiply(x=w190, y=w195) -> (x*y=w192:dbl)
  n14 = Multiply(x=w189, y=w195) -> (x*y=w194:dbl)
  n15 = Divide(x=w192, y=w196) -> (x/y=w191:dbl)
  n16 = Divide(x=w194, y=w196) -> (x/y=w193:dbl)
  n17 = To Word Integer(number=w191) -> (16bit integer=w188:i16)
  n18 = To Word Integer(number=w193) -> (16bit integer=w187:i16)
  n19 = Not(x=w176) -> (.not. x?=w171:bool)
  n20 = local read "Cycles/step (MCL)"() -> (w179:u64)
  n21 = Multiply(x=w207, y=1000.0) -> (x*y=w214:dbl)
  n22 = local read "Scan steps (MCL)"() -> (w180:u64)
  n23 = local write "Trap Pos FIFO Timeout"(u16 0 ("Trap Pos FIFO Timeout")) -> ()
  n24 = local read "Desired Scan Incr (V)"() -> (w182:dbl)
  n25 = Scale By Power Of 2(n=48, x=w214) -> (x*2^n=w215:dbl)
  n26 = Multiply(x=w212, y=w211) -> (x*y=w210:dbl)
  n27 = Divide(x=w215, y=w210) -> (x/y=w209:dbl)
  n28 = local read "Number Interlace Sets"() -> (w103:u8)
  n29 = Split 1D Array(array=w110, index=w103) -> (first subarray=w112:u32[])  [unwired: 1 out]
  n30 = Add Array Elements(numeric array=w112) -> (sum=w111:u32)
  n31 = property on="AI Count (ticks)" class="DigNum (strict)"("Val(Sgnl)"="AI Count (ticks)") -> ()  [unwired: 2 in, 2 out]
  n32 = local read "# Samples/channel"() -> (w199:u32)
  n33 = local read "Number of F/B Scans (AOD)"() -> (w200:u16)
  n34 = To Quad Integer(1:w209) -> (0:w206:i64)
  n35 = local read "Not-Interlacing Set"() -> (w102:enum32{"Set 1", "Set 2", "Set 3"})
  n36 = To Unsigned Byte Integer(number=w102) -> (unsigned 8bit integer=w108:u8)
  n37 = Index Array(array=w110, index=w108) -> (element=w109:u32)
  n38 = local read "Feedback On/Off"() -> (w229:cluster{"Set 1":bool, "Set 2":bool})
  n39 = local read "PID Gains"() -> (w221:T9)
  n40 = Divide(x=40000000.0, y="AI Count (ticks)") -> (x/y=w168:dbl)
  n41 = Multiply(x=w182, y=32767.0) -> (x*y=w184:dbl)
  n42 = local read "Scan steps (AOD)"() -> (w205:u64)
  n43 = local read "All FB On/Off"() -> (w230:bool)
  n44 = local read "Cycles/step (AOD)"() -> (w204:u64)
  n45 = local write "AI rate (Hz)"(w168) -> ()
  n46 = Divide(x=w184, y=10.0) -> (x/y=w183:dbl)
  n47 = Multiply(x=w205, y=w204) -> (x*y=w203:u64)
  n48 = Multiply(x=3276.7, y=w226) -> (x*y=w225:cluster{"Set 1":dbl, "Set 2":dbl})
  n49 = To Word Integer(number=w183) -> (16bit integer=w181:i16)
  n50 = Multiply(x=w203, y=u64 2) -> (x*y=w201:u64)
  n51 = local read "Sets to FIFO (Traps)"() -> (w233:T15)
  n52 = Divide(x=w168, y="FPGA Ave.") -> (x/y=w169:dbl)
  n53 = To Word Integer(number=w225) -> (16bit integer=w224:cluster{"Set 1":i16, "Set 2":i16})
  n54 = xnode "Open FPGA VI Reference"("resource name"=T18 "750kHzDAQ") -> ("FPGA VI Reference Out"=w218:T19)  [unwired: 1 in, 1 out]
  n55 = Unbundle By Name(w221) -> ("Set 1"=w220:T14, "Set 2"=w219:T14)
  n56 = Multiply(x=w201, y=w200) -> (x*y=w198:u64)
  n57 = local write "Ave. Rate (Hz)"(w169) -> ()
  n58 = Divide(x=w198, y=w199) -> (x/y=w197:dbl)
  n59 = Unbundle By Name(w224) -> ("Set 1"=w223:i16, "Set 2"=w222:i16)
  n60 = local read "2D or 1D Scan"() -> (w122:bool)
  n61 = local write "Data points/scans"(w198) -> ()
  n62 = local read "Scan BD"() -> (w216:bool)
  n63 = And(x=w229, y=w230) -> (x .and. y?=w228:cluster{"Set 1":bool, "Set 2":bool})
  n64 = local write "Data points/scan (f/b)"(w201) -> ()
  n65 = Reciprocal(x=w169) -> (1/x=w170:dbl)
  n66 = local read "N Acq Sets (Traps + Fl.)"() -> (w161:i16)
  n67 = local write "N sets should be saved"(w197) -> ()
  n68 = Unbundle By Name(w228) -> ("Set 1"=w232:bool, "Set 2"=w231:bool)
  n69 = local read "Interlace"() -> (w104:bool)
  n70 = Select(t=w111, s=w104, f=w109) -> (s? t:f=w101:u32)
  n71 = local write "Update Count (MCL)"(w101) -> ()
  n72 = local write "Total Counts (ticks)"(w101) -> ()
  n73 = xnode "Invoke Method"("FPGA VI Reference In"=w218) -> ("FPGA VI Reference Out"=w120:T19, "error out"=w139:errorcluster)  [unwired: 1 in]
  n74 = local write "Ave. Period (s)"(w170) -> ()
  n75 = property on="2D or 1D Scan" class="Bool (strict)"("Val(Sgnl)"=w122) -> ()  [unwired: 2 in, 2 out]
  n76 = xnode "Read/Write Control"("FPGA VI Reference In"=w119, "error in"=w139, "ai count"="AI Count (ticks)", "Interlace ON/OFF"=w104, "Number Interlace Cycles"=w103, "AI1 Sets to FIFO"=w233, "FB On/Off Set 1"=w232, "FB On/Off Set 2"=w231, "Interlace Off Parameters"=w102, "FB Setpoint Set 1"=w223, "FB Setpoint Set 2"=w222, "FB Gains Set 1"=w220, "FB Gains Set 2"=w219, "FB output range 1"=w121, "FB output range 2"=w121, "Cycles per step"=w204, "Scan BD"=w216, "Number of scans"=w200, "Scan steps"=w205, "Scan freq.  increment"=w206, "AO1"=w188, "AO2"=w187, "Scan freq.  increment (MCL)"=w181, "Scan steps (MCL)"=w180, "Cycles per step (MCL)"=w179, "Number of scans (MCL)"=w178, "MCL count"=w101, "Cont. Scan (MCL)"=w177, "MCL Scan Axis"=w171, "1D or 2D Scan?"=w122, "N of AI1 Int Acq Sets"=w161, "Freq or Amp switch first"="Freq or Amp switch first", "Freq switch delay"="Freq switch delay", "Amp switch delay"="Amp switch delay", "Swap F1 and F2"="Swap F1 and F2", "APD Acq Rate Count"=w127, "APD to FIFO"=FALSE, "APD Gate Operating Mode"="APD Gate", "APD Gate ON Count"="APD Gate ON Count", "APD Gate OFF Count"="APD Gate OFF Count", "Invert APD Gate"="Invert APD Gate", "DIO count 1 (ticks)"="DIO count 1 (ticks)", "DIO count 2 (ticks)"="DIO count 2 (ticks)", "DIO count 3 (ticks)"="DIO count 3 (ticks)", "APD 1 AO scale factor"="APD 1 AO Mult.", "APD 2 AO scale factor"="APD 2 AO Mult.") -> ("FPGA VI Reference Out"=w96:T19, "error out"=w98:errorcluster)  [unwired: 1 in]
  n77 = local read "Green Laser ON/Interlacing"() -> (w99:bool)
  n78 = local read "Green laser mode"() -> (w100:enum32{"Laser ON", "Laser OFF", "Interlace"})
  n79 = local read "GI Frequency, OFF count"() -> (w92:u32)
  n80 = local read "GI Frequency, ON count"() -> (w91:u32)
  n81 = Multiply(x="Current When FB OFF (%)", y=655.35) -> (x*y=w82:dbl)
  n82 = local read "Green FB Count"() -> (w90:u32)
  n83 = Multiply(x="Green FB Setpoint (mV)", y=3.2767) -> (x*y=w79:dbl)
  n84 = To Unsigned Word Integer(number=w82) -> (unsigned 16bit integer=w80:u16)
  n85 = local read "Invert GI"() -> (w94:bool)
  n86 = To Word Integer(number=w79) -> (16bit integer=w77:i16)
  n87 = case shown="True" w99 {
    tunnel: w100 -> [_ w253]
    tunnel: [enum32{"Laser ON", "Laser OFF", "Interlace"}."Laser OFF" ("Green laser mode") w253] -> w93
    frame False {
    }
    frame True {
    }
  }
  n88 = local read "Trap Pos. AI1 X Pre-scale"() -> (w48:u16)
  n89 = local read "Trap Pos FB Monitor\nT1 or T2"() -> (w55:bool)
  n90 = local read "Trap Pos FB Int Count"() -> (w43:u16)
  n91 = local read "Trap Pos FB Negate Action"() -> (w54:bool)
  n92 = local read "Trap Pos. FB Offset Factor"() -> (w53:i64)
  n93 = local read "Trap Pos. FB Mult Factor"() -> (w52:i64)
  n94 = local read "Trap Pos. FB Gains"() -> (w50:T11)
  n95 = local read "Trap Pos. FB Range"() -> (w51:T12)
  n96 = xnode "Read/Write Control"("FPGA VI Reference In"=w96, "error in"=w98, "Green interlace ON count 2"=w91, "Green interlace OFF count 2"=w92, "Invert GI 2"=w94, "Operating Mode 2"=w93, "Green FB Gains"="Green FB Gains", "Green FB Setpoint"=w77, "Green FB On/Off"="Green FB On/Off", "Current Out"=w80, "Green int current ON count adj"="Green int current ON count adj", "Green FB Count"=w90, "Operating Mode"=w93, "Green interlace OFF count"=w92, "Green interlace ON count"=w91, "Invert GI"=w94, "Trap Pos FB Monitor T1 or T2"=w55, "Trap Pos FB Negate Action"=w54, "Trap Pos. FB Offset Factor"=w53, "Trap Pos. FB Mult Factor"=w52, "Trap Pos. FB Range"=w51, "Trap Pos. FB Gains"=w50, "Force feedback"=FALSE, "AI1 X Scale"=w48, "Trap Pos to FIFO"=TRUE, "Trap Pos FB Int Count"=w43) -> ("FPGA VI Reference Out"=w95:T19, "error out"=w97:errorcluster)
  n97 = xnode "Invoke Method"("FPGA VI Reference In"=w95, "error in"=w97, "Requested Depth"="Trap AI FIFO Depth") -> ("FPGA VI Reference Out"=w58:T19, "error out"=w57:errorcluster)  [unwired: 1 out]
  n98 = xnode "Invoke Method"("FPGA VI Reference In"=w58, "error in"=w57, "Requested Depth"="Trap Position FIFO Depth") -> ("FPGA VI Reference Out"=w45:T19, "error out"=w44:errorcluster)  [unwired: 1 out]
  n99 = flat-sequence {
    tunnel: w120 -> [w258]
    tunnel: [w258] -> w119
    tunnel: [w257] -> w118
    tunnel: [w256] -> w117
    tunnel: [w254] -> w115
    tunnel: [w255] -> w116
    frame #0 {
      w255 = T16 {"Minimum"=50.0, "Maximum"=100.0, "Increment"=1.0} ("Min Max Inc")
      w254 = T16 {"Minimum"=0.0, "Maximum"=75.0, "Increment"=1.0} ("Data Entry Limits")
      w257 = T16 {"Minimum"=50.0, "Maximum"=100.0, "Increment"=1.0} ("Min Max Inc")
      w256 = T16 {"Minimum"=0.0, "Maximum"=75.0, "Increment"=1.0} ("Data Entry Limits")
      n100 = property on="BD 2 Frequency 1 (MHz)" class="DigNum (strict)"("Data Range"=w255) -> ()  [unwired: 2 in, 2 out]
      n101 = property on="BD 2 Frequency 3 (MHz)" class="DigNum (strict)"("Data Range"=w255) -> ()  [unwired: 2 in, 2 out]
      n102 = property on="BD 2 Frequency 2 (MHz)" class="DigNum (strict)"("Data Range"=w255) -> ()  [unwired: 2 in, 2 out]
      n103 = property on="BD 1 Frequency 1 (MHz)" class="DigNum (strict)"("Data Range"=w257) -> ()  [unwired: 2 in, 2 out]
      n104 = property on="BD 1 Frequency 2 (MHz)" class="DigNum (strict)"("Data Range"=w257) -> ()  [unwired: 2 in, 2 out]
      n105 = property on="BD 1 Frequency 3 (MHz)" class="DigNum (strict)"("Data Range"=w257) -> ()  [unwired: 2 in, 2 out]
      n106 = property on="BD 2 Amplitude 1 (%)" class="DigNum (strict)"("Data Range"=w254) -> ()  [unwired: 2 in, 2 out]
      n107 = property on="BD 2 Amplitude 2 (%)" class="DigNum (strict)"("Data Range"=w254) -> ()  [unwired: 2 in, 2 out]
      n108 = property on="BD 2 Amplitude 3 (%)" class="DigNum (strict)"("Data Range"=w254) -> ()  [unwired: 2 in, 2 out]
      n109 = property on="BD 1 Amplitude 3 (%)" class="DigNum (strict)"("Data Range"=w256) -> ()  [unwired: 2 in, 2 out]
      n110 = property on="BD 1 Amplitude 2 (%)" class="DigNum (strict)"("Data Range"=w256) -> ()  [unwired: 2 in, 2 out]
      n111 = property on="BD 1 Amplitude 1 (%)" class="DigNum (strict)"("Data Range"=w256) -> ()  [unwired: 2 in, 2 out]
      "X RF Frequency Limits (MHz)" <- w257
      "X RF Amplitude Limits (%)" <- w256
      "Y RF Amplitude Limits (%)" <- w254
      "Y RF Frequency Limits (MHz)" <- w255
    }
  }
  n112 = xnode "Invoke Method"("FPGA VI Reference In"=w45, "error in"=w44) -> ("FPGA VI Reference Out"=w22:T19, "error out"=w21:errorcluster)  [unwired: 1 in]
  n113 = flat-sequence "Initial FPGA Loop Relative Phase Adjustment" {
    tunnel: "Initial Phase Adjustment (APD 2 Gate)" -> [w260]
    tunnel: "Initial Phase Adjustment (GI) 2" -> [w261]
    tunnel: "Initial Phase Adj. (MCL)" -> [w262]
    tunnel: w21 -> [w263]
    tunnel: w22 -> [w264]
    tunnel: "Initial Phase Adjustment (GI)" -> [w265]
    tunnel: "Initial Phase Adjustment (AI1)" -> [w266]
    tunnel: [w266] -> w31
    tunnel: [w265] -> w30
    tunnel: [w264] -> w29
    tunnel: [w263] -> w28
    tunnel: [w262] -> w27
    tunnel: [w261] -> w26
    tunnel: [w260] -> w25
    tunnel: [w278] -> w145
    tunnel: [w272] -> w143
    tunnel: "Initial Phase Adjustment (APD Acq)" -> [w271]
    tunnel: "Initial Phase Adjustment (APD 1 Gate)" -> [w270]
    tunnel: "Initial Phase Adjustment (Green FB)" -> [w269]
    tunnel: w31 -> [w277]
    tunnel: w30 -> [w276]
    tunnel: w29 -> [w275]
    tunnel: w28 -> [w274]
    tunnel: w27 -> [w273]
    tunnel: w26 -> [w268]
    tunnel: w25 -> [w267]
    tunnel: w145 -> [w280]
    tunnel: [w281] -> w144
    tunnel: w143 -> [w281]
    tunnel: [w280] -> w142
    tunnel: w144 -> [w284]
    tunnel: w142 -> [w283]
    tunnel: [w286] -> w141
    tunnel: [w285] -> w140
    tunnel: [w288] -> w20
    tunnel: [w289] -> w23
    tunnel: w141 -> [w289]
    tunnel: w140 -> [w288]
    frame #0 {
      n114 = Wait (ms)(milliseconds to wait=u32 1000) -> ()  [unwired: 1 out]
    }
    frame #1 {
      n115 = xnode "Read/Write Control"("FPGA VI Reference In"=w275, "error in"=w274, "Phase count adjustment"=w277, "Phase count adjustment (GI)"=w276, "Phase count adjustment (MCL)"=w273, "Phase Count Adjustment (APD Acq)"=w271, "Phase count adjustment (APD 1 Gate)"=w270, "Phase count adjustment (APD 2 Gate)"=w267, "Phase count adjustment (Green FB)"=w269, "Phase count adjustment (GI) 2"=w268) -> ("FPGA VI Reference Out"=w272:T19, "error out"=w278:errorcluster)
    }
    frame #2 {
      n116 = Wait (ms)(milliseconds to wait=u32 1000) -> ()  [unwired: 1 out]
    }
    frame #3 {
      w282 = TRUE
      n117 = xnode "Read/Write Control"("FPGA VI Reference In"=w284, "error in"=w283, "+ phase"=w282, "+ phase (GI)"=w282, "+ phase (MCL)"=w282, "+ phase (APD Acq)"=w282, "+ phase (APD 1 Gate)"=w282, "+ phase (APD 2 Gate)"=w282, "+ phase (Green FB)"=w282, "+ phase (GI) 2"=w282) -> ("FPGA VI Reference Out"=w285:T19, "error out"=w286:errorcluster)
    }
    frame #4 {
      n118 = Wait (ms)(milliseconds to wait=u32 1000) -> ()  [unwired: 1 out]
    }
  }
  n119 = local read "Phase adj. (Green FB)"() -> (w113:i16)
  n120 = local read "Phase adj. (GI) 2"() -> (w83:i16)
  n121 = local read "Phase adjust (MCL)"() -> (w172:i16)
  n122 = local read "Phase adj. (AI1)"() -> (w174:i16)
  n123 = local read "Phase adj. (GI)"() -> (w173:i16)
  n124 = xnode "Read/Write Control"("FPGA VI Reference In"=w20, "error in"=w23, "Phase count adjustment"=w174, "Phase count adjustment (GI)"=w173, "Phase count adjustment (MCL)"=w172, "Phase Count Adjustment (APD Acq)"="Phase Adj. (APD Acq)", "Phase count adjustment (APD 1 Gate)"="Phase Adj. (APD 1 Gate)", "Phase count adjustment (APD 2 Gate)"="Phase Adj. (APD 2 Gate)", "Phase count adjustment (Green FB)"=w113, "Phase count adjustment (GI) 2"=w83) -> ("FPGA VI Reference Out"=w19:T19, "error out"=w18:errorcluster)
  n125 = call "Initialize RF boards - interlace 3.vi"("error in"=w18, "FPGA VI Reference In"=w19) -> ("FPGA VI Reference Out"=w150:T19)  [unwired: 1 out]
  n126 = call "set RF board frequency - interlace.vi"("Board 2 Frequency Limits"=w116, "Board 1 Frequency Limits"=w118, "FPGA VI Reference In"=w150, "Board 2 Frequency 3 (MHz)"="BD 2 Frequency 3 (MHz)", "Board 1 Frequency 3 (MHz)"="BD 1 Frequency 3 (MHz)", "Board 2 Frequency 2 (MHz)"="BD 2 Frequency 2 (MHz)", "Board 2 Frequency 1 (MHz)"="BD 2 Frequency 1 (MHz)", "Board 1 Frequency 2 (MHz)"="BD 1 Frequency 2 (MHz)", "Board 1 Frequency 1  (MHz)"="BD 1 Frequency 1 (MHz)") -> ("error out"=w244:errorcluster, "FPGA VI Reference Out"=w245:T19)  [unwired: 1 in]
  n127 = call "set RF board amplitude - interlace.vi"("Board 2 Amplitude Limits"=w115, "Board 1 Amplitude Limits"=w117, "error in"=w244, "FPGA VI Reference In"=w245, "Board 2 Amplitude 3 (%)"="BD 2 Amplitude 3 (%)", "Board 1 Amplitude 3 (%)"="BD 1 Amplitude 3 (%)", "Board 2 Amplitude 2 (%)"="BD 2 Amplitude 2 (%)", "Board 2 Amplitude 1 (%)"="BD 2 Amplitude 1 (%)", "Board 1 Amplitude 2 (%)"="BD 1 Amplitude 2 (%)", "Board 1 Amplitude 1 (%)"="BD 1 Amplitude 1 (%)") -> ("error out"=w16:errorcluster, "FPGA VI Reference Out"=w17:T19)
  n128 = flat-sequence {
    tunnel: w17 -> [w298]
    tunnel: w16 -> [w297]
    tunnel: [w296] -> w237
    tunnel: [w295] -> w236
    tunnel: [w302] -> w235
    tunnel: w237 -> [w302]
    tunnel: [w301] -> w234
    tunnel: w236 -> [w301]
    tunnel: w235 -> [w311]
    tunnel: w234 -> [w310]
    tunnel: [w309] -> w12
    tunnel: [w304] -> w11
    tunnel: [w314] -> w40
    tunnel: [w318] -> w24
    tunnel: w12 -> [w318]
    tunnel: w11 -> [w313]
    frame #0 {
      n129 = local read "Trap 1 (ON/OFF)"() -> (w290:bool)
      n130 = xnode "Read/Write Control"("FPGA VI Reference In"=w298, "error in"=w297, "Direct RF Box  Communication"=FALSE) -> ("FPGA VI Reference Out"=w296:T19, "error out"=w295:errorcluster)
      n131 = local write "Saving..."(FALSE ("Saving Data")) -> ()
      n132 = local write "Stop All"(FALSE ("Stop All")) -> ()
      n133 = local write "Index"(1.0 ("Index")) -> ()
      n134 = property on="Trap 1 ON" class="Bool (strict)"("Value"=w290) -> ()  [unwired: 2 in, 2 out]
      "Manipulating Trap" <- FALSE ("Manipulating Trap")
    }
    frame #1 {
      n135 = local read "Trap 2 (ON/OFF)"() -> (w300:bool)
      n136 = Wait (ms)(milliseconds to wait=u32 50) -> ()  [unwired: 1 out]
      n137 = property on="Trap 2 ON" class="Bool (strict)"("Val(Sgnl)"=w300) -> ()  [unwired: 2 in, 2 out]
    }
    frame #2 {
      n138 = local read "Scan Range (nm)"() -> (w305:dbl)
      n139 = xnode "Read/Write Control"("FPGA VI Reference In"=w311, "error in"=w310, "FPGA Controls  RF Box"=TRUE ("Direct RF Box  Communication")) -> ("FPGA VI Reference Out"=w309:T19, "error out"=w304:errorcluster)
      n140 = call "Update messages.vi"("Message to add"="UHR-Fleezers ready.", "Old message string"="") -> ("New message string"=w308:string)
      n141 = local write "Messages"(w308) -> ()
      n142 = property on="Scan Range (nm)" class="DigNum (strict)"("Val(Sgnl)"=w305) -> ()  [unwired: 2 in, 2 out]
    }
    frame #3 {
      n143 = call "hamilton_controller.vi"("error in"=w313, "action"=T20."CONNECT") -> ("error out"=w315:errorcluster)  [unwired: 9 in]
      n144 = call "hamilton_controller.vi"("error in"=w315, "action"=T20."INITIALIZE VALVES") -> ("error out"=w314:errorcluster)  [unwired: 9 in]
    }
  }
  n145 = Subtract(x="BD 1 Frequency 1 (MHz)", y="BD 1 Frequency 2 (MHz)") -> (x-y=w160:dbl)
  n146 = Subtract(x="BD 2 Frequency 1 (MHz)", y="BD 2 Frequency 2 (MHz)") -> (x-y=w159:dbl)
  n147 = Square(x=w159) -> (x^2=w157:dbl)
  n148 = Square(x=w160) -> (x^2=w158:dbl)
  n149 = Add(x=w158, y=w157) -> (x+y=w156:dbl)
  n150 = Square Root(x=w156) -> (sqrt(x)=w155:dbl)
  n151 = local write "Trap Delta (MHz)"(w155) -> ()
  n152 = Current VI's Path() -> (path=w1:path)
  n153 = Strip Path(path=w1) -> (stripped path=w2:path)  [unwired: 1 out]
  n154 = Build Path(base path=w2, name or relative path="Locations.txt") -> (appended path=→"Location path":path)
  n155 = Concatenate Strings("N.D.", "\r\n") -> (w5:string)
  n156 = Initialize Array(w5, 4, 3) -> (w8:string[][])
  n157 = local write "Location Matrix"(w8) -> ()
  n158 = call "IMAQ Create"("Image Name"="APD 1 Image", "Image Type"=w64) -> ("New Image"=w63:T2)  [unwired: 3 in, 1 out]
  n159 = call "IMAQ Create"("Image Name"="APD 2 Image", "Image Type"=w64) -> ("New Image"=w62:T2)  [unwired: 3 in, 1 out]
  n160 = call "IMAQ Create"("Image Name"="Det. X Image", "Image Type"=w64) -> ("New Image"=w61:T2)  [unwired: 3 in, 1 out]
  n161 = call "IMAQ Create"("Image Name"="Det. Y Image", "Image Type"=w64) -> ("New Image"=w60:T2)  [unwired: 3 in, 1 out]
  n162 = Bundle("New Image"=w63, "New Image"=w62, "New Image"=w61, "New Image"=w60) -> (w59:T21)  [unwired: 1 in]
  n163 = while {
    stop <- w319 stop-if-true
    n164 = event shown="[1] \"Goto Top (F6)\": Value Change" {
      selector: _ -> [_ _ _ _ _ _ _]
      dyn-events: _ -> [_ _ _ _ _ _ _]
      timeout: 10 -> [_ _ _ _ _ _ _]
      tunnel: [FALSE _ _ _ _ _ _] -> w319
      event Timeout {
        # "Query and display stage positions"
        # "Trajectory Mode is set to Jog"
        # "Setting ESP300 left and right limits for Z-axis, input in mm"
        # "Change Low Jog Velocity"
        # "Change High Jog Velocity"
        # "Display Selected Location"
        n165 = event-data() -> ()  [unwired: 1 in, 2 out]
        n166 = local read "ESP Port"() -> (w340:refnum<visa-resource-name>)
        n167 = Concatenate Strings("3SL" ("Substring"), "ESP ZL-Limit", ";3SR", "ESP ZR-Limit", "\r") -> (w339:string)
        n168 = VISA Write(VISA resource name=w340, write buffer=w339) -> ()  [unwired: 1 in, 3 out]
        n169 = local read "Location Matrix"() -> (w363:string[][])
        n170 = local read "Locations"() -> (w362:i32)
        n171 = Index Array(array=w363, index (row)=w362) -> (element=w361:string[])  [unwired: 1 in]
        n172 = Concatenate Strings("1JH" ("Substring"), "Axis 1", "2JH" ("Substring"), "Axis 2", "3JH" ("Substring"), "Axis 3", "\r") -> (w358:string)
        n173 = local read "ESP Port"() -> (w357:refnum<visa-resource-name>)
        n174 = VISA Write(VISA resource name=w357, write buffer=w358) -> ()  [unwired: 1 in, 3 out]
        n175 = Array To Cluster(array=w361) -> (cluster=w360:T22)
        n176 = local write "Selected Location"(w360) -> ()
        n177 = Concatenate Strings("1JW" ("Substring"), "Axis 1", "2JW" ("Substring"), "Axis 2", "3JW" ("Substring"), "Axis 3", "\r") -> (w349:string)
        n178 = local read "ESP Port"() -> (w348:refnum<visa-resource-name>)
        n179 = VISA Write(VISA resource name=w348, write buffer=w349) -> ()  [unwired: 1 in, 3 out]
        n180 = local read "ESP Port"() -> (w330:refnum<visa-resource-name>)
        n181 = Concatenate Strings("1TJ3;\n2TJ3;\n3TJ3" ("Substring"), "\r") -> (w333:string)
        n182 = VISA Write(VISA resource name=w330, write buffer=w333) -> ()  [unwired: 1 in, 3 out]
        n183 = Concatenate Strings("1TP;\n2TP;\n3TP;\n1MD?;\n2MD?;\n3MD?" ("Substring"), "\r") -> (w324:string)
        n184 = local read "ESP Port"() -> (w327:refnum<visa-resource-name>)
        n185 = VISA Write(VISA resource name=w327, write buffer=w324, error in (no error)="error in") -> (VISA resource name out=w325:refnum<visa-resource-name>, error out=w323:errorcluster)  [unwired: 1 out]
        n186 = case shown="True" TRUE ("Case Constant\n(See Context Help)") {
          tunnel: w325 -> [_ w383]
          tunnel: w323 -> [w364 w382]
          tunnel: [w364 w366] -> w329
          frame False {
          }
          frame True {
            w376 = u16 10 items=["1.0"=10, "1.5"=15, "2.0"=20] ("Serial Settings:Stop Bits")
            w377 = u16 0 items=["None", "Odd", "Even", "Mark", "Space"] ("Serial Settings:Parity")
            n187 = property class="Instr"(reference=w383, error in=w382, "Baud"=u32 921600 ("Serial Settings:Baud Rate"), "Data Bits"=u16 8 ("Serial Settings:Data Bits"), "Parity"=w377, "Stop Bits"=w376) -> (reference out=w381:refnum<visa-resource-name>, error out=w380:errorcluster, "Bytes at Port"=w365:u32)
            n188 = Wait (ms)(milliseconds to wait=u32 10) -> ()  [unwired: 1 out]
            n189 = VISA Read(VISA resource name=w381, byte count=w365, error in (no error)=w380) -> (VISA resource name out=w389:refnum<visa-resource-name>, read buffer=→"X Pos":string, error out=w390:errorcluster)  [unwired: 1 out]
            n190 = VISA Read(VISA resource name=w389, byte count=w365, error in (no error)=w390) -> (VISA resource name out=w387:refnum<visa-resource-name>, read buffer=→"Y Pos":string, error out=w388:errorcluster)  [unwired: 1 out]
            n191 = VISA Read(VISA resource name=w387, byte count=w365, error in (no error)=w388) -> (VISA resource name out=w375:refnum<visa-resource-name>, read buffer=→"Z Pos Pos":string, error out=w374:errorcluster)  [unwired: 1 out]
            n192 = VISA Read(VISA resource name=w375, byte count=w365, error in (no error)=w374) -> (VISA resource name out=w371:refnum<visa-resource-name>, read buffer=→"X Motion":string, error out=w372:errorcluster)  [unwired: 1 out]
            n193 = VISA Read(VISA resource name=w371, byte count=w365, error in (no error)=w372) -> (VISA resource name out=w370:refnum<visa-resource-name>, read buffer=→"Y Motion":string, error out=w368:errorcluster)  [unwired: 1 out]
            n194 = VISA Read(VISA resource name=w370, byte count=w365, error in (no error)=w368) -> (read buffer=→"Z motion":string, error out=w366:errorcluster)  [unwired: 2 out]
          }
        }
        "error out" <- w329
      }
      event "Goto Top (F6)": Value Change {
        n195 = event-data() -> ()  [unwired: 1 in, 5 out]
        n196 = stacked-sequence {
          frame #0 {
            # "stop motions of all axes before going to avoid reversing of direction"
            n197 = local read "ESP Port"() -> (w395:refnum<visa-resource-name>)
            n198 = Concatenate Strings("ST" ("Substring"), "\r") -> (w392:string)
            n199 = VISA Write(VISA resource name=w395, write buffer=w392) -> ()  [unwired: 1 in, 3 out]
          }
          frame #1 {
            n200 = Wait (ms)(milliseconds to wait=u32 50) -> ()  [unwired: 1 out]
          }
          frame #2 {
            # "Change the trajectory mode to Trapezoidal"
            n201 = local read "ESP Port"() -> (w400:refnum<visa-resource-name>)
            n202 = Concatenate Strings("1TJ1;\n2TJ1;\n3TJ1" ("Substring"), "\r") -> (w397:string)
            n203 = VISA Write(VISA resource name=w400, write buffer=w397) -> ()  [unwired: 1 in, 3 out]
          }
          frame #3 {
            # "Go to Top Dispensor"
            n204 = local read "Location Matrix"() -> (w412:string[][])
            n205 = Index Array(array=w412, index (row)=0) -> (element=w408:string[])  [unwired: 1 in]
            n206 = Decimate 1D Array(w408) -> (w406:string[], w404:string[], w402:string[])
            n207 = Concatenate Strings("1PA" ("Substring"), w406, "2PA" ("Substring"), w404, "3PA" ("Substring"), w402, "\r") -> (w410:string)
            n208 = local read "ESP Port"() -> (w409:refnum<visa-resource-name>)
            n209 = VISA Write(VISA resource name=w409, write buffer=w410) -> ()  [unwired: 1 in, 3 out]
          }
          frame #4 {
            n210 = Wait (ms)(milliseconds to wait=u32 2000) -> ()  [unwired: 1 out]
          }
          frame #5 {
            n211 = local read "Location Matrix"() -> (→"Location Matrix 3":string[][])
          }
        }
      }
      event "Goto Exp (F8)": Value Change {
        n212 = event-data() -> ()  [unwired: 1 in, 5 out]
        n213 = stacked-sequence {
          frame #0 {
            # "stop motions of all axes before going to avoid reversing of direction"
            n214 = local read "ESP Port"() -> (w418:refnum<visa-resource-name>)
            n215 = Concatenate Strings("ST" ("Substring"), "\r") -> (w415:string)
            n216 = VISA Write(VISA resource name=w418, write buffer=w415) -> ()  [unwired: 1 in, 3 out]
          }
          frame #1 {
            n217 = Wait (ms)(milliseconds to wait=u32 50) -> ()  [unwired: 1 out]
          }
          frame #2 {
            # "Change the trajectory mode to Trapezoidal"
            n218 = local read "ESP Port"() -> (w423:refnum<visa-resource-name>)
            n219 = Concatenate Strings("1TJ1;\n2TJ1;\n3TJ1" ("Substring"), "\r") -> (w420:string)
            n220 = VISA Write(VISA resource name=w423, write buffer=w420) -> ()  [unwired: 1 in, 3 out]
          }
          frame #3 {
            # "Go to Experimental"
            n221 = local read "Location Matrix"() -> (w435:string[][])
            n222 = Index Array(array=w435, index (row)=2) -> (element=w431:string[])  [unwired: 1 in]
            n223 = Decimate 1D Array(w431) -> (w429:string[], w427:string[], w425:string[])
            n224 = Concatenate Strings("1PA" ("Substring"), w429, "2PA" ("Substring"), w427, "3PA" ("Substring"), w425, "\r") -> (w433:string)
            n225 = local read "ESP Port"() -> (w432:refnum<visa-resource-name>)
            n226 = VISA Write(VISA resource name=w432, write buffer=w433) -> ()  [unwired: 1 in, 3 out]
          }
          frame #4 {
            n227 = Wait (ms)(milliseconds to wait=u32 100) -> ()  [unwired: 1 out]
          }
        }
      }
      event "Goto Bottom (F7)": Value Change {
        n228 = event-data() -> ()  [unwired: 1 in, 5 out]
        n229 = stacked-sequence {
          frame #0 {
            # "stop motions of all axes before going to avoid reversing of direction"
            n230 = local read "ESP Port"() -> (w440:refnum<visa-resource-name>)
            n231 = Concatenate Strings("ST" ("Substring"), "\r") -> (w437:string)
            n232 = VISA Write(VISA resource name=w440, write buffer=w437) -> ()  [unwired: 1 in, 3 out]
          }
          frame #1 {
            n233 = Wait (ms)(milliseconds to wait=u32 50) -> ()  [unwired: 1 out]
          }
          frame #2 {
            # "Change the trajectory mode to Trapezoidal"
            n234 = local read "ESP Port"() -> (w445:refnum<visa-resource-name>)
            n235 = Concatenate Strings("1TJ1;\n2TJ1;\n3TJ1" ("Substring"), "\r") -> (w442:string)
            n236 = VISA Write(VISA resource name=w445, write buffer=w442) -> ()  [unwired: 1 in, 3 out]
          }
          frame #3 {
            # "Go to Bottom Dispensor"
            n237 = local read "Location Matrix"() -> (w457:string[][])
            n238 = Index Array(array=w457, index (row)=1) -> (element=w453:string[])  [unwired: 1 in]
            n239 = Decimate 1D Array(w453) -> (w451:string[], w449:string[], w447:string[])
            n240 = Concatenate Strings("1PA" ("Substring"), w451, "2PA" ("Substring"), w449, "3PA" ("Substring"), w447, "\r") -> (w455:string)
            n241 = local read "ESP Port"() -> (w454:refnum<visa-resource-name>)
            n242 = VISA Write(VISA resource name=w454, write buffer=w455) -> ()  [unwired: 1 in, 3 out]
          }
          frame #4 {
            n243 = Wait (ms)(milliseconds to wait=u32 100) -> ()  [unwired: 1 out]
          }
        }
      }
      event "Capture": Value Change {
        n244 = event-data() -> ()  [unwired: 1 in, 5 out]
        n245 = local read "Locations"() -> (w459:i32)
        n246 = local read "Z Pos Pos"() -> (w460:string)
        n247 = local read "X Pos"() -> (w462:string)
        n248 = local read "Y Pos"() -> (w461:string)
        n249 = case shown="1" w459 {
          selector: w459 -> [w466 w473 w480 w487]
          tunnel: w462 -> [w469 w476 w483 w490]
          tunnel: w461 -> [w468 w475 w482 w489]
          tunnel: w460 -> [w467 w474 w481 w488]
          frame 0, Default {
            # "Capture Top Dispensor Location"
            n250 = local read "Location Matrix"() -> (w465:string[][])
            n251 = Build Array(w469, w468, w467) -> (w464:string[])
            n252 = Replace Array Subset(array=w465, new element=w464, index (row)=w466) -> (w463:string[][])  [unwired: 1 in]
            n253 = local write "Location Matrix"(w463) -> ()
          }
          frame 1 {
            # "Capture Bottom Dispensor Location"
            n254 = local read "Location Matrix"() -> (w472:string[][])
            n255 = Build Array(w476, w475, w474) -> (w471:string[])
            n256 = Replace Array Subset(array=w472, new element=w471, index (row)=w473) -> (w470:string[][])  [unwired: 1 in]
            n257 = local write "Location Matrix"(w470) -> ()
          }
          frame 2 {
            # "Capture Experimental Region Location"
            n258 = local read "Location Matrix"() -> (w479:string[][])
            n259 = Build Array(w483, w482, w481) -> (w478:string[])
            n260 = Replace Array Subset(array=w479, new element=w478, index (row)=w480) -> (w477:string[][])  [unwired: 1 in]
            n261 = local write "Location Matrix"(w477) -> ()
          }
          frame 3 {
            # "Capture Other Location"
            n262 = local read "Location Matrix"() -> (w486:string[][])
            n263 = Build Array(w490, w489, w488) -> (w485:string[])
            n264 = Replace Array Subset(array=w486, new element=w485, index (row)=w487) -> (w484:string[][])  [unwired: 1 in]
            n265 = local write "Location Matrix"(w484) -> ()
          }
        }
      }
      event "Save": Value Change {
        # "reshape Location Matrix to 1-D array to write"
        n266 = event-data() -> ()  [unwired: 1 in, 5 out]
        n267 = local read "Location Matrix"() -> (w494:string[][])
        n268 = local read "Location path"() -> (w491:path)
        n269 = Reshape Array(w494, 12) -> (w492:string[])
        n270 = Write to Text File(file (use dialog)=w491, text=w492) -> ()  [unwired: 2 in, 3 out]
      }
      event "Activate Joystick": Value Change {
        n271 = event-data() -> ()  [unwired: 1 in, 5 out]
        n272 = case shown="True" "Activate Joystick" {
          frame False {
          }
          frame True {
            # "Change the trajectory mode to Jog"
            n273 = local read "ESP Port"() -> (w499:refnum<visa-resource-name>)
            n274 = Concatenate Strings("1TJ3;\n2TJ3;\n3TJ3" ("Substring"), "\r") -> (w496:string)
            n275 = VISA Write(VISA resource name=w499, write buffer=w496) -> ()  [unwired: 1 in, 3 out]
          }
        }
      }
    }
  }
  n276 = disable-structure shown="Disabled" {
    disable-tunnel: w24 -> [w528 _]
    frame Disabled {
      w523 = T17 0 items=["Grayscale (U8)", "Grayscale (I16)", "Grayscale (SGL)", "Complex (CSG)", "RGB (U32)", "HSL (U32)", "RGB (U64)", "Grayscale (U16)"] ("Image Type")
      n277 = call <vilib>:"IMAQ Init.vi"("Interface Name"="img0") -> ("error out"=w525:errorcluster, "IMAQ Session Out"=w527:refnum<k11>)  [unwired: 9 in]
      n278 = call <vilib>:"IMAQ Grab Setup.vi"("error in (no error)"=w525, "IMAQ Session In"=w527) -> ("error out"=w521:errorcluster, "IMAQ Session Out"=w522:refnum<k11>)  [unwired: 8 in]
      n279 = call "IMAQ Create"("Image Name"="untitled", "Image Type"=w523) -> ("New Image"=w520:T2)  [unwired: 3 in, 1 out]
      n280 = call <vilib>:"Application Directory.vi"() -> ("Application Directory"=w507:path)
      n281 = Build Path(base path=w507, name or relative path="_trap_screen_positions") -> (appended path=w515:path)
      n282 = Open/Create/Replace File(file path (use dialog)=w515, operation (0:open)=T23."open or create", access (0:read/write)=enum16{"read/write", "read-only", "write-only"}."read/write") -> (refnum out=w517:refnum<file>)  [unwired: 3 in, 2 out]
      n283 = local read "Trap Sets"() -> (w509:u32)
      n284 = for "Load trap positions on video screen from file." {
        N: w509 -> [_]
        tunnel: [w535] -> w510
        tunnel: w517 -> [w534]
        tunnel: [w531] -> w506 mode=indexing
        w533 = 4
        n285 = for {
          N: w533 -> [_]
          tunnel: [w539] -> w535
          tunnel: w534 -> [w538]
          tunnel: w533 -> [w537]
          tunnel: [w536] -> w532 mode=indexing
          n286 = Read from Binary File(5:w537, 11:w538) -> (2:w536:i32, 3:w539:refnum<file>)  [unwired: 4 in, 2 out]
        }
        n287 = Array To Cluster(array=w532) -> (cluster=w531:T27)
      }
      n288 = node-c288() -> (w530:T24)  [unwired: 4 in]
      n289 = timed-loop "acquire video and stage position" {
        timing: w530 -> [_]
        timing-out: [_] -> w529
        tunnel: w522 -> [w558]
        tunnel: w521 -> [w557]
        tunnel: w520 -> [w556]
        tunnel: [w555] -> w502
        tunnel: [w552] -> w503
        tunnel: [w553] -> w501
        tunnel: w528 -> [_]
        shift-right: [w549] -> w519
        shift-left: w506 -> [w550]
        tunnel: w509 -> [w547]
        stop <- w554 stop-if-true
        n290 = node-c288() -> ()  [unwired: 1 in, 1 out]
        n291 = event shown="[2] \"Primary Video Display\": Mouse Down" {
          selector: _ -> [_ _ _ _]
          dyn-events: _ -> [_ _ _ _]
          timeout: 10 -> [_ _ _ _]
          tunnel: w558 -> [w569 w584 w593 w612]
          tunnel: w557 -> [w568 w586 w591 w614]
          tunnel: w556 -> [w567 w585 w592 w613]
          tunnel: [w566 w584 w593 w612] -> w555
          tunnel: [w559 w588 FALSE FALSE] -> w554
          tunnel: [w563 w586 w591 w614] -> w553
          tunnel: [w562 w585 w592 w613] -> w552
          tunnel: "radius" -> [_ _ w598 _]
          tunnel: w550 -> [w560 w587 w596 _]
          tunnel: [w560 w587 w597 cluster{i32, i32, i32, i32}[] []] -> w549
          tunnel: w547 -> [_ _ w589 _]
          event Timeout {
            n292 = event-data() -> ()  [unwired: 1 in, 2 out]
            n293 = call <vilib>:"IMAQ Grab Acquire.vi"("error in (no error)"=w568, "Image In"=w567, "IMAQ Session In"=w569) -> ("error out"=w564:errorcluster, "Image Out"=w565:T2, "IMAQ Session Out"=w566:refnum<k11>)  [unwired: 5 in, 1 out]
            n294 = case shown="True" "trap\nmarkers?" {
              tunnel: w560 -> [_ w577]
              tunnel: w565 -> [w571 w576]
              tunnel: w564 -> [w570 w575]
              tunnel: [w570 w574] -> w563
              tunnel: [w571 w572] -> w562
              frame False {
              }
              frame True {
                n295 = for {
                  tunnel: w577 -> [w583] mode=indexing
                  shift-right: [w581] -> w572
                  shift-left: w576 -> [w582]
                  tunnel: w575 -> [w580]
                  tunnel: [w579] -> w574
                  tunnel: u32 16711680 ("Color") -> [w578]
                  n296 = call "IMAQ Overlay Oval"("Color"=w578, "error in (no error)"=w580, "Bounding Rectangle"=w583, "Image"=w582) -> ("error out"=w579:errorcluster, "Image Out"=w581:T2)  [unwired: 6 in]
                }
              }
            }
            "Primary Video Display" <- w562
            n297 = Unbundle By Name(w564) -> ("status"=w559:bool)
          }
          event "Stop All": Value Change {
            n298 = event-data() -> ()  [unwired: 1 in, 5 out]
            n299 = local read "Stop All"() -> (w588:bool)
          }
          event "Primary Video Display": Mouse Down {
            n300 = event-data() -> ()  [unwired: 1 in, 7 out]
            n301 = Array Size(array=w596) -> (size(s)=w595:i32)
            n302 = Less?(x=w595, y=w589) -> (x < y?=w594:bool)
            n303 = case shown="True" w594 {
              tunnel: w598 -> [_ w608]
              tunnel: w596 -> [w599 w602]
              tunnel: [w599 w601] -> w597
              frame False {
              }
              frame True {
                n304 = property on="Primary Video Display" class="ImageControl"() -> ("Last Mouse Position"=w600:cluster{"X":i32, "Y":i32})  [unwired: 2 in, 2 out]
                n305 = Unbundle By Name(w600) -> ("X"=w610:i32, "Y"=w609:i32)
                n306 = Add(x=w609, y=w608) -> (x+y=w606:i32)
                n307 = Subtract(x=w609, y=w608) -> (x-y=w604:i32)
                n308 = Add(x=w610, y=w608) -> (x+y=w605:i32)
                n309 = Subtract(x=w610, y=w608) -> (x-y=w607:i32)
                n310 = Bundle(w607, w606, w605, w604) -> (w603:cluster{i32, i32, i32, i32})  [unwired: 1 in]
                n311 = Build Array (concatenate)(w602, w603) -> (w601:T28)
              }
            }
          }
          event "clear markers": Value Change {
            n312 = event-data() -> ()  [unwired: 1 in, 5 out]
          }
        }
        n313 = node-c288() -> ()  [unwired: 1 in, 1 out]
      }
      n314 = node-c288(w529) -> ()  [unwired: 1 out]
      n315 = Set File Position(offset (in bytes) (0)=i64 0, refnum=w510, from (0:start)=enum16{"start", "end", "current"}."start") -> (refnum out=w511:refnum<file>)  [unwired: 1 in, 1 out]
      n316 = for "Write trap positions to file so they can be remembered\nwhen program is removed from memory" {
        tunnel: w519 -> [w543] mode=indexing
        tunnel: [w541] -> w518
        tunnel: w511 -> [w540]
        n317 = Cluster To Array(cluster=w543) -> (array=w542:i32[])
        n318 = for {
          tunnel: w542 -> [w546] mode=indexing
          tunnel: [w545] -> w541
          tunnel: w540 -> [w544]
          n319 = Write to Binary File(file (use dialog)=w544, data=w546) -> (refnum out=w545:refnum<file>)  [unwired: 4 in, 2 out]
        }
      }
      n320 = Close File(refnum=w518) -> ()  [unwired: 1 in, 2 out]
      n321 = call "IMAQ Dispose"("Image"=w503, "error in (no error)"=w501) -> ("error out"=w500:errorcluster)  [unwired: 4 in]
      n322 = call <vilib>:"IMAQ Stop.vi"("error in (no error)"=w500, "IMAQ Session In"=w502) -> ("error out"=w504:errorcluster, "IMAQ Session Out"=w505:refnum<k11>)  [unwired: 8 in]
      n323 = call <vilib>:"IMAQ Close.vi"("error in (no error)"=w504, "IMAQ Session In"=w505) -> ()  [unwired: 9 in, 1 out]
    }
    frame Enabled {
    }
  }
  n324 = node-c288(2 ("Processor")) -> (w15:T24)  [unwired: 3 in]
  n325 = node-c288() -> (w69:T24)  [unwired: 4 in]
  n326 = disable-structure shown="Enabled" {
    disable-tunnel: [w621 _] -> w35
    disable-tunnel: w24 -> [w620 _]
    frame Enabled {
      n327 = node-c288() -> (w623:T24)  [unwired: 4 out]
      n328 = timed-loop "Rough control of MCL mirror stage (debugging)" {
        tunnel: w620 -> [w626]
        tunnel: [w625] -> w621
        timing: w623 -> [_]
        timing-out: [_] -> w622
        stop <- w625 stop-if-true
        n329 = node-c288() -> ()  [unwired: 2 out]
        n330 = case shown="1" "MCL Mode" {
          tunnel: w626 -> [_ w629 w676]
          frame 0, Default {
            # "manual positioning"
          }
          frame 1 {
            # "sinusoidal wave"
            n331 = node-c288() -> (w631:T24)  [unwired: 4 out]
            n332 = timed-loop "Oscillate MCL mirror" {
              timing: w631 -> [_]
              timing-out: [_] -> w630
              tunnel: w629 -> [w670]
              i -> [w669]
              stop <- w632 stop-if-true
              n333 = node-c288() -> (w668:i64)  [unwired: 1 out]
              n334 = Multiply(x="AO1", y=32767.0) -> (x*y=w664:dbl)
              n335 = Multiply(x="AO2", y=32767.0) -> (x*y=w659:dbl)
              n336 = Divide(x=w664, y=10.0) -> (x/y=w665:dbl)
              n337 = Divide(x=w659, y=10.0) -> (x/y=w660:dbl)
              n338 = To Word Integer(number=w665) -> (16bit integer=w657:i16)
              n339 = To Word Integer(number=w660) -> (16bit integer=w656:i16)
              n340 = Divide(x=w668, y=i64 1000) -> (x/y=w639:dbl)
              n341 = Multiply(x=w639, y=w669) -> (x*y=w650:dbl)
              n342 = Multiply(x="Osc. freq. (Hz) 2", y=6.283185307179586) -> (x*y=w651:dbl)
              n343 = Multiply(x=w651, y=w650) -> (x*y=w649:dbl)
              n344 = Sine(x=w649) -> (sin(x)=w648:dbl)
              n345 = Multiply(x=w648, y="Osc. amp. (V)") -> (x*y=w646:dbl)
              n346 = Add(x=w646, y="Osc. center (V)") -> (x+y=w644:dbl)
              n347 = Divide(x=w644, y=10.0) -> (x/y=w642:dbl)
              n348 = Multiply(x=w642, y=32767.0) -> (x*y=w637:dbl)
              n349 = Select(t=w637, s="Scan axis", f=w657) -> (s? t:f=w655:dbl)
              n350 = Select(t=w656, s="Scan axis", f=w637) -> (s? t:f=w654:dbl)
              n351 = local read "MCL Mode"() -> (w636:u16)
              n352 = Not Equal?(x=w636, y=u16 1) -> (x != y?=w633:bool)
              n353 = local read "Stop All"() -> (w634:bool)
              n354 = xnode "Read/Write Control"("FPGA VI Reference In"=w670, "AO1"=w655, "AO2"=w654) -> ()  [unwired: 1 in, 2 out]
              n355 = Compound Arithmetic op=OR(w634, w633) -> (w632:bool)
              n356 = node-c288() -> ()  [unwired: 2 out]
            }
            n357 = node-c288(w630) -> ()  [unwired: 1 out]
          }
          frame 2 {
            # "linear scan"
            n358 = case shown="True" "Start Scan" {
              tunnel: w676 -> [_ w688]
              frame False {
              }
              frame True {
                n359 = Subtract(x="End (V)", y="Begin (V)") -> (x-y=w684:dbl)
                n360 = Decrement(x="N Points") -> (x-1=w683:dbl)
                n361 = Divide(x=w684, y=w683) -> (x/y=w681:dbl)
                n362 = for {
                  N: "N Points" -> [_]
                  tunnel: "Begin (V)" -> [w701]
                  tunnel: w688 -> [w693]
                  tunnel: [w692] -> w687 mode=indexing
                  tunnel: w681 -> [w691]
                  tunnel: [w689] -> w680 mode=indexing
                  i -> [w700]
                  n363 = Multiply(x=w691, y=w700) -> (x*y=w699:dbl)
                  n364 = Add(x=w701, y=w699) -> (x+y=w696:dbl)
                  n365 = local read "Scan axis"() -> (w690:bool)
                  n366 = local read "AO1"() -> (w698:dbl)
                  n367 = local read "AO2"() -> (w697:dbl)
                  n368 = Select(t=w696, s=w690, f=w698) -> (s? t:f=w695:dbl)
                  n369 = Select(t=w697, s=w690, f=w696) -> (s? t:f=w694:dbl)
                  n370 = flat-sequence {
                    tunnel: w695 -> [w705]
                    tunnel: w694 -> [w704]
                    tunnel: w693 -> [w702]
                    tunnel: [w715] -> w692
                    tunnel: [w714] -> w689
                    frame #0 {
                      w708 = 10.0 ("y")
                      w703 = 32767.0 ("y")
                      n371 = Multiply(x=w705, y=w703) -> (x*y=w711:dbl)
                      n372 = Multiply(x=w704, y=w703) -> (x*y=w709:dbl)
                      n373 = Divide(x=w711, y=w708) -> (x/y=w712:dbl)
                      n374 = Divide(x=w709, y=w708) -> (x/y=w710:dbl)
                      n375 = To Word Integer(number=w712) -> (16bit integer=w706:i16)
                      n376 = To Word Integer(number=w710) -> (16bit integer=w707:i16)
                      n377 = xnode "Read/Write Control"("FPGA VI Reference In"=w702, "AO1"=w706, "AO2"=w707) -> ()  [unwired: 1 in, 2 out]
                    }
                    frame #1 {
                      n378 = Wait (ms)(milliseconds to wait="DAQ Delay (ms)") -> ()  [unwired: 1 out]
                    }
                    frame #2 {
                      n379 = local read "Slow mean"() -> (w715:dbl)
                      n380 = local read "Sigma"() -> (w714:dbl)
                    }
                  }
                }
                n381 = Bundle("Begin (V)"="Begin (V)", w681, w687) -> (→"MCL Scan":cluster{"Begin (V)":dbl, dbl, dbl[]})  [unwired: 1 out]
                n382 = Bundle("Begin (V)"="Begin (V)", w681, w680) -> (→"MCL Scan 2":cluster{"Begin (V)":dbl, dbl, dbl[]})  [unwired: 1 out]
              }
            }
          }
        }
        n383 = local read "Stop All"() -> (w625:bool)
        n384 = node-c288() -> ()  [unwired: 2 out]
      }
      n385 = node-c288(w622) -> ()  [unwired: 1 out]
    }
    frame Disabled {
    }
  }
  n386 = timed-loop "Control parameters (event loop)" {
    tunnel: w24 -> [w721]
    shift-right: [w720] -> _
    shift-left: errorcluster {"status"=FALSE, "code"=0, "source"=""} ("error out") -> [w719]
    tunnel: [w718] -> w37
    timing: w15 -> [_]
    timing-out: [_] -> w14
    stop <- w718 stop-if-true
    n387 = node-c288() -> ()  [unwired: 1 in, 1 out]
    n388 = event shown="[6] \"BD 1 Frequency 1 (MHz)\", \"BD 1 Frequency 2 (MHz)\", \"BD 1 Frequency 3 (MHz)\", \"BD 2 Frequency 1 (MHz)\", \"BD 2 Frequency 2 (MHz)\", \"BD 2 Frequency 3 (MHz)\", \"Trap Delta (MHz)\": Value Change" {
      selector: _ -> [_ _ _ _ _ _ _ _ _ _ _ _ _ _ _ _ _ _ _ _ _ _ _ _ _ _ _ _ _ _ _ _ _ _ _ _ _ _ _ _ _ _ _ _ _ _ _ _ _ _ _ _ _ _ _]
      dyn-events: _ -> [_ _ _ _ _ _ _ _ _ _ _ _ _ _ _ _ _ _ _ _ _ _ _ _ _ _ _ _ _ _ _ _ _ _ _ _ _ _ _ _ _ _ _ _ _ _ _ _ _ _ _ _ _ _ _]
      timeout: _ -> [_ _ _ _ _ _ _ _ _ _ _ _ _ _ _ _ _ _ _ _ _ _ _ _ _ _ _ _ _ _ _ _ _ _ _ _ _ _ _ _ _ _ _ _ _ _ _ _ _ _ _ _ _ _ _]
      tunnel: w721 -> [w759 _ _ _ w796 _ w818 _ w882 _ _ _ w925 _ _ w968 w974 w979 w985 w1021 w1039 w1046 w1064 w1075 w1086 w1097 w1108 w1119 w1137 w1143 w1237 _ w1246 w1284 _ w1319 w1323 w1334 w1338 w1342 _ w1350 _ _ _ _ w1484 _ w1501 w1504 w1513 w1516 w1520 _ w1537]
      tunnel: [w758 _ _ _ w786 _ w817 _ w845 _ w890 _ w904 _ _ w967 w970 w976 w982 w1020 w1037 w1045 w1058 w1069 w1080 w1091 w1102 w1113 w1135 w1142 w1235 _ w1244 w1282 _ w1317 w1321 w1324 w1336 w1340 _ w1348 _ _ _ _ w1482 _ _ _ _ _ _ _ _] -> w720
      tunnel: w719 -> [w757 _ _ _ w795 _ w816 _ w877 _ w890 _ w924 _ _ w966 w969 w975 w981 w1019 w1038 w1044 w1063 w1074 w1085 w1096 w1107 w1118 w1136 w1141 w1236 _ w1245 w1283 _ w1318 w1322 w1333 w1337 w1341 _ w1349 _ _ _ _ w1483 _ w1500 w1503 w1512 w1515 w1519 _ w1536]
      tunnel: [_ _ _ _ _ _ _ _ _ _ w889 _ _ _ _ _ _ _ _ _ _ _ _ _ _ _ _ _ _ _ _ _ _ _ _ _ _ _ _ _ _ _ _ _ _ _ _ _ _ _ _ _ _ _ _] -> w718
      tunnel: [_ _ _ _ _ _ _ "Round T1 X" _ _ _ _ _ _ _ _ _ _ _ _ _ _ _ _ _ _ _ _ _ _ _ _ _ _ _ _ _ _ _ _ _ _ _ _ _ _ _ _ _ _ _ _ _ _ _] -> _
      tunnel: [_ _ _ "Adjust Scale\nto Mean" _ _ _ _ _ _ _ _ _ _ _ _ _ _ _ _ _ _ _ _ _ _ _ _ _ _ _ _ _ _ _ _ _ _ _ _ _ _ _ _ _ _ _ _ _ _ _ _ "Set SP to Reading" _ _] -> _
      tunnel: [_ _ _ _ _ _ _ _ _ "Round T2 X" _ "Delayed Interlace Start" _ _ _ _ _ _ _ _ _ _ _ _ _ _ _ _ _ _ _ _ _ _ _ _ _ _ _ _ _ _ _ _ _ _ _ _ _ _ _ _ _ _ _] -> _
      event "AI Count (ticks)", "Sets to FIFO (Traps)", "Save ave N", "FPGA Ave.", "# Samples/channel", "N sets to save": Value Change {
        # "So that if 'Save ave N' is updated, the AOD scanning code updates too."
        n389 = event-data() -> ()  [unwired: 6 out]
        n390 = local read "AI Count (ticks)"() -> (w739:u32)
        n391 = Boolean To (0,1)(Boolean="Sets to FIFO (Traps)") -> (0, 1=w749:cluster{"Set 1":i16, "Set 2":i16, "Set 3":i16})
        n392 = xnode "Read/Write Control"("FPGA VI Reference In"=w759, "error in"=w757, "ai count"=w739, "AI1 Sets to FIFO"="Sets to FIFO (Traps)", "N of AI1 Int Acq Sets"="N Acq Sets (Traps + Fl.)") -> ("error out"=w758:errorcluster)  [unwired: 1 out]
        n393 = Cluster To Array(cluster=w749) -> (array=w748:i16[])
        n394 = To Unsigned Long Integer(number=w748) -> (unsigned 32bit integer=w728:u32[])
        n395 = local read "Scan steps (AOD)"() -> (w750:u64)
        n396 = Multiply(x=w739, y="N Acq Sets (Traps + Fl.)") -> (x*y=w737:u32)
        n397 = Divide(x=40000000.0, y=w739) -> (x/y=w731:dbl)
        "AI rate (Hz)" <- w731
        "Ave. Rate (Hz)" <- w731
        n398 = Add Array Elements(numeric array=w728) -> (sum=w740:u32)
        "Trap Sets" <- w740
        n399 = Reciprocal(x=w731) -> (1/x=→"Ave. Period (s)":dbl)
        n400 = property on="Scan steps (AOD)" class="DigNum (strict)"("Val(Sgnl)"=w750) -> ()  [unwired: 2 in, 2 out]
        n401 = Divide(x=w731, y="N Acq Sets (Traps + Fl.)") -> (x/y=w754:dbl)
        "Data Rate (Hz)" <- w754
        n402 = Reciprocal(x=w754) -> (1/x=→"Data Period (s)":dbl)
        n403 = local read "Save ave N"() -> (w753:dbl)
        n404 = Divide(x=w754, y=w753) -> (x/y=w752:dbl)
        "Save Data Rate (Hz)" <- w752
        n405 = Reciprocal(x=w752) -> (1/x=→"Save Data Period (s)":dbl)
        n406 = Multiply(x=w737, y="# Samples/trap") -> (x*y=w735:u32)
        "Counts/DMA" <- w735
        n407 = property on="Trap Disp. Downsample" class="DigNum (strict)"("Maximum"="# Samples/trap") -> ()  [unwired: 2 in, 2 out]
        n408 = Multiply(x=w740, y="# Samples/trap") -> (x*y=w729:u32)
        "# Samples/channel" <- w729
        n409 = Multiply(x=w729, y=u32 8) -> (x*y=→"Trap AI Elements/DMA read":u32)
        n410 = local read "APD Int. Count"() -> (w736:u32)
        n411 = Multiply(x=w729, y=u32 3) -> (x*y=→"Trap Pos Elements/DMA read":u32)
        n412 = Divide(x=w735, y=w736) -> (x/y=w726:dbl)
        "APD Samples/FIFO Acq." <- w726
        n413 = Divide(x=w735, y=40000000.0) -> (x/y=w733:dbl)
        "DMA Update Period (s)" <- w733
        n414 = Multiply(x=2.0, y=w726) -> (x*y=→"APD Elements/DMA read":dbl)
        n415 = property on="APD Disp. Downsample" class="DigNum (strict)"("Maximum"=w726) -> ()  [unwired: 2 in, 2 out]
        n416 = local read "N sets to save"() -> (w746:u32)
        n417 = Multiply(x=w733, y=w746) -> (x*y=→"Total Time (s)":dbl)
        "FPGA Averaging" <- FALSE ("FPGA Averaging")
      }
      event "Rescale on Mean": Value Change {
        n418 = event-data() -> ()  [unwired: 7 out]
        n419 = And(x=FALSE, y="Rescale on Mean") -> (x .and. y?=w761:bool)
        n420 = local write "Rescale on Mean"(w761) -> ()
        n421 = local read "Bead Mean (nm)"() -> (w766:dbl)
        n422 = Add(x="Amplitude (nm)", y=w766) -> (x+y=w764:dbl)
        n423 = Subtract(x=w766, y="Amplitude (nm)") -> (x-y=w763:dbl)
        n424 = property on="Bead Separation" class="WFChart (strict)"("YScale.Minimum"=w763) -> ()  [unwired: 2 in, 2 out]
        n425 = property on="Bead Separation" class="WFChart (strict)"("YScale.Maximum"=w764) -> ()  [unwired: 2 in, 2 out]
      }
      event "Detector Type": Value Change {
        n426 = event-data() -> ()  [unwired: 7 out]
        n427 = local read "AI labels"() -> (w767:string[])
        n428 = property on="High Res. Display" class="Ring (strict)"("Strings []"=w767) -> ()  [unwired: 2 in, 2 out]
        n429 = Build Array (concatenate)(w767, "none") -> (w768:string[])
        n430 = property on="FFT 1 Choice 1" class="Ring (strict)"("Strings []"=w768) -> ()  [unwired: 2 in, 2 out]
        n431 = property on="FFT 1 Choice 2" class="Ring (strict)"("Strings []"=w768) -> ()  [unwired: 2 in, 2 out]
        n432 = property on="FFT 2 Choice 1" class="Ring (strict)"("Strings []"=w768) -> ()  [unwired: 2 in, 2 out]
        n433 = property on="FFT 2 Choice 2" class="Ring (strict)"("Strings []"=w768) -> ()  [unwired: 2 in, 2 out]
        n434 = Bundle("APD 1", "APD 2") -> (w771:cluster{string, string})  [unwired: 1 out]
        n435 = Cluster To Array(cluster=w771) -> (array=w769:string[])
        n436 = Build Array (concatenate)(w769, w768) -> (w773:string[])
        n437 = Array Size(array=w773) -> (size(s)=w774:i32)
        n438 = property on="Signals to Plot" class="LstBox (strict)"("Item Names"=w773) -> ()  [unwired: 2 in, 2 out]
        n439 = property on="Signals to Plot" class="LstBox (strict)"("Number of Rows"=w774) -> ()  [unwired: 2 in, 2 out]
        n440 = property on="All Signals" class="WFChart (strict)"("LegNumRows"=w774) -> ()  [unwired: 2 in, 2 out]
      }
      event "Adjust Scale\nto Mean": Value Change {
        n441 = event-data() -> ()  [unwired: 7 out]
        n442 = local read "APD 1 Rate (Hz)"() -> (w783:dbl)
        n443 = Multiply(x=1000.0, y="Above (kHz)") -> (x*y=w781:dbl)
        n444 = Multiply(x=1000.0, y="Below (kHz)") -> (x*y=w779:dbl)
        n445 = Add(x=w781, y=w783) -> (x+y=w776:dbl)
        n446 = Subtract(x=w783, y=w779) -> (x-y=w777:dbl)
        n447 = property on="APD Chart" class="WFChart (strict)"("YScale.Minimum"=w777) -> ()  [unwired: 2 in, 2 out]
        n448 = property on="APD Chart" class="WFChart (strict)"("YScale.Maximum"=w776) -> ()  [unwired: 2 in, 2 out]
      }
      event "Phase adj. (AI1)", "+ phase (AI1)", "- phase (AI1)": Value Change {
        n449 = event-data() -> ()  [unwired: 7 out]
        n450 = Negate(x="Phase adj. (AI1)") -> (-x=w793:i16)
        n451 = Select(t=w793, s="- phase (AI1)", f="Phase adj. (AI1)") -> (s? t:f=w792:i16)
        n452 = xnode "Read/Write Control"("FPGA VI Reference In"=w796, "error in"=w795, "Phase count adjustment"=w792) -> ("FPGA VI Reference Out"=w791:T19, "error out"=w790:errorcluster)
        n453 = Or(x="- phase (AI1)", y="+ phase (AI1)") -> (x .or. y?=w787:bool)
        n454 = xnode "Read/Write Control"("FPGA VI Reference In"=w791, "error in"=w790, "+ phase"=w787) -> ("error out"=w786:errorcluster)  [unwired: 1 out]
      }
      event "Signals to Plot": Double Click {
        w799 = u32 9868950 ("Color Box")
        n455 = event-data() -> ("Row"=w801:i32)  [unwired: 9 out]
        n456 = property on="All Signals" class="WFChart (strict)"("Active Plot"=w801) -> (error out=w812:errorcluster)  [unwired: 2 in, 1 out]
        n457 = property on="All Signals" class="WFChart (strict)" props=["Plot", "Visible?", "Plot", "Plot Color"](error in=w812) -> (error out=w811:errorcluster, "Plot.Visible?"=w810:bool)  [unwired: 1 in, 2 out]
        n458 = Select(t=FALSE ("Plot.Visible"), s=w810, f=TRUE ("Plot.Visible")) -> (s? t:f=w805:bool)
        n459 = property on="All Signals" class="WFChart (strict)"(error in=w811, "Plot.Visible?"=w805) -> (error out=w807:errorcluster)  [unwired: 1 in, 1 out]
        n460 = property on="All Signals" class="WFChart (strict)"(error in=w807) -> (error out=w802:errorcluster, "Plot.Plot Color"=w806:u32)  [unwired: 1 in, 1 out]
        n461 = property on="Signals to Plot" class="LstBox (strict)"(error in=w802, "Active Row"=w801) -> (error out=w800:errorcluster)  [unwired: 1 in, 1 out]
        n462 = Select(t=w806, s=w805, f=u32 0) -> (s? t:f=w803:u32)
        n463 = property on="Signals to Plot" class="LstBox (strict)"(error in=w800, "CellFontColor"=w803, "SelColor"=w799, "CellBG"=w799, "CellFontSize"=u32 20 ("Active Row:Cell Font:Size"), "CellFontBold"=TRUE ("Active Row:Cell Font:Bold")) -> ()  [unwired: 1 in, 2 out]
      }
      event "BD 1 Frequency 1 (MHz)", "BD 1 Frequency 2 (MHz)", "BD 1 Frequency 3 (MHz)", "BD 2 Frequency 1 (MHz)", "BD 2 Frequency 2 (MHz)", "BD 2 Frequency 3 (MHz)", "Trap Delta (MHz)": Value Change {
        # "anytime one of the frequencies is changed, write it to the RF board UNLESS Set 2 is being oscillated. The oscillation\nscript writes the frequencies to the RF board."
        n464 = event-data() -> ("CtlRef"=w815:refnum<vi>)  [unwired: 6 out]
        n465 = control-ref of="Trap Delta (MHz)"() -> (w814:refnum<vi>)
        n466 = Equal?(x=w814, y=w815) -> (x = y?=w813:bool)
        n467 = case shown="False" "Oscillate Set 2" {
          tunnel: w818 -> [w838 _]
          tunnel: [w837 w841] -> w817
          tunnel: w816 -> [w836 w841]
          tunnel: w813 -> [w822 _]
          frame False {
            n468 = local read "BD 1 Frequency 1 (MHz)"() -> (w820:dbl)
            n469 = local read "BD 1 Frequency 2 (MHz)"() -> (w824:dbl)
            n470 = Add(x=w820, y="Trap Delta (MHz)") -> (x+y=w823:dbl)
            n471 = Select(t=w823, s=w822, f=w824) -> (s? t:f=w821:dbl)
            n472 = local read "Y RF Frequency Limits (MHz)"() -> (w826:T16)
            n473 = local read "X RF Frequency Limits (MHz)"() -> (w827:T16)
            n474 = local read "BD 1 Frequency 3 (MHz)"() -> (w839:dbl)
            n475 = local write "BD 1 Frequency 2 (MHz)"(w821) -> ()
            n476 = local read "BD 2 Frequency 1 (MHz)"() -> (w830:dbl)
            n477 = local read "BD 2 Frequency 2 (MHz)"() -> (w829:dbl)
            n478 = local read "BD 2 Frequency 3 (MHz)"() -> (w840:dbl)
            n479 = call "set RF board frequency - interlace.vi"("Board 2 Frequency Limits"=w826, "Board 1 Frequency Limits"=w827, "error in"=w836, "FPGA VI Reference In"=w838, "Board 2 Frequency 3 (MHz)"=w840, "Board 1 Frequency 3 (MHz)"=w839, "Board 2 Frequency 2 (MHz)"=w829, "Board 2 Frequency 1 (MHz)"=w830, "Board 1 Frequency 2 (MHz)"=w821, "Board 1 Frequency 1  (MHz)"=w820) -> ("error out"=w837:errorcluster)  [unwired: 1 out]
            n480 = Subtract(x=w830, y=w829) -> (x-y=w834:dbl)
            n481 = Subtract(x=w821, y=w820) -> (x-y=w835:dbl)
            n482 = Square(x=w834) -> (x^2=w832:dbl)
            n483 = Square(x=w835) -> (x^2=w833:dbl)
            n484 = Add(x=w833, y=w832) -> (x+y=w831:dbl)
            n485 = Square Root(x=w831) -> (sqrt(x)=w828:dbl)
            n486 = local write "Trap Delta (MHz)"(w828) -> ()
            n487 = property on="Initial delta (MHz)" class="DigNum (strict)"("Val(Sgnl)"=w828) -> ()  [unwired: 2 in, 2 out]
          }
          frame True {
          }
        }
      }
      event "Round T1 X": Value Change {
        n488 = event-data() -> ()  [unwired: 7 out]
        n489 = local read "BD 1 Frequency 1 (MHz)"() -> (w844:dbl)
        n490 = Round To Nearest(number=w844) -> (nearest integer value=w843:dbl)
        n491 = property on="BD 1 Frequency 1 (MHz)" class="DigNum (strict)"("Val(Sgnl)"=w843) -> ()  [unwired: 2 in, 2 out]
      }
      event "Restart RF": Value Change {
        n492 = event-data() -> ()  [unwired: 7 out]
        n493 = xnode "Read/Write Control"("FPGA VI Reference In"=w882, "error in"=w877, "FPGA Controls  RF Box"=FALSE) -> ("FPGA VI Reference Out"=w881:T19, "error out"=w876:errorcluster)
        n494 = local read "Y RF Amplitude Limits (%)"() -> (w857:T16)
        n495 = local read "X RF Amplitude Limits (%)"() -> (w858:T16)
        n496 = local read "X RF Frequency Limits (MHz)"() -> (w860:T16)
        n497 = local read "Y RF Frequency Limits (MHz)"() -> (w859:T16)
        n498 = xnode "Read/Write Control"("FPGA VI Reference In"=w881, "error in"=w876, "Direct RF Box  Communication"=TRUE) -> ("FPGA VI Reference Out"=w880:T19, "error out"=w875:errorcluster)
        n499 = local read "BD 2 Frequency 3 (MHz)"() -> (w867:dbl)
        n500 = local read "BD 2 Frequency 2 (MHz)"() -> (w868:dbl)
        n501 = local read "BD 1 Frequency 3 (MHz)"() -> (w871:dbl)
        n502 = local read "BD 1 Frequency 1 (MHz)"() -> (w872:dbl)
        n503 = local read "BD 2 Frequency 1 (MHz)"() -> (w869:dbl)
        n504 = local read "BD 1 Frequency 2 (MHz)"() -> (w870:dbl)
        n505 = call "Initialize RF boards - interlace 3.vi"("error in"=w875, "FPGA VI Reference In"=w880) -> ("error out"=w874:errorcluster, "FPGA VI Reference Out"=w879:T19)
        n506 = local read "BD 2 Amplitude 2 (%)"() -> (w862:dbl)
        n507 = local read "BD 2 Amplitude 1 (%)"() -> (w863:dbl)
        n508 = local read "BD 2 Amplitude 3 (%)"() -> (w861:dbl)
        n509 = local read "BD 1 Amplitude 3 (%)"() -> (w866:dbl)
        n510 = local read "BD 1 Amplitude 1 (%)"() -> (w865:dbl)
        n511 = local read "BD 1 Amplitude 2 (%)"() -> (w864:dbl)
        n512 = call "set RF board frequency - interlace.vi"("Board 2 Frequency Limits"=w859, "Board 1 Frequency Limits"=w860, "error in"=w874, "FPGA VI Reference In"=w879, "Board 2 Frequency 3 (MHz)"=w867, "Board 1 Frequency 3 (MHz)"=w871, "Board 2 Frequency 2 (MHz)"=w868, "Board 2 Frequency 1 (MHz)"=w869, "Board 1 Frequency 2 (MHz)"=w870, "Board 1 Frequency 1  (MHz)"=w872) -> ("error out"=w873:errorcluster, "FPGA VI Reference Out"=w878:T19)
        n513 = call "set RF board amplitude - interlace.vi"("Board 2 Amplitude Limits"=w857, "Board 1 Amplitude Limits"=w858, "error in"=w873, "FPGA VI Reference In"=w878, "Board 2 Amplitude 3 (%)"=w861, "Board 1 Amplitude 3 (%)"=w866, "Board 2 Amplitude 2 (%)"=w862, "Board 2 Amplitude 1 (%)"=w863, "Board 1 Amplitude 2 (%)"=w864, "Board 1 Amplitude 1 (%)"=w865) -> ("error out"=w850:errorcluster, "FPGA VI Reference Out"=w854:T19)
        n514 = xnode "Read/Write Control"("FPGA VI Reference In"=w854, "error in"=w850, "Direct RF Box  Communication"=FALSE) -> ("FPGA VI Reference Out"=w853:T19, "error out"=w852:errorcluster)
        n515 = flat-sequence {
          tunnel: w852 -> [w883]
          tunnel: [w883] -> w851
          frame #0 {
            n516 = Wait (ms)(milliseconds to wait=u32 50) -> ()  [unwired: 1 out]
          }
        }
        n517 = xnode "Read/Write Control"("FPGA VI Reference In"=w853, "error in"=w851, "FPGA Controls  RF Box"=TRUE) -> ("error out"=w846:errorcluster)  [unwired: 1 out]
        n518 = property on="Restart RF" class="Bool (strict)"(error in=w846, "Value"=FALSE ("Restart RF")) -> (error out=w845:errorcluster)  [unwired: 1 in, 1 out]
      }
      event "Round T2 X": Value Change {
        n519 = event-data() -> ()  [unwired: 7 out]
        n520 = local read "BD 1 Frequency 2 (MHz)"() -> (w886:dbl)
        n521 = Round To Nearest(number=w886) -> (nearest integer value=w885:dbl)
        n522 = property on="BD 1 Frequency 2 (MHz)" class="DigNum (strict)"("Val(Sgnl)"=w885) -> ()  [unwired: 2 in, 2 out]
      }
      event "Stop All": Value Change {
        n523 = event-data() -> ()  [unwired: 7 out]
        n524 = call "hamilton_controller.vi"("action"=T20."DISCONNECT") -> ()  [unwired: 10 in, 1 out]
        n525 = local read "Stop All"() -> (w889:bool)
      }
      event "Delayed Interlace Start": Value Change {
        n526 = event-data() -> ()  [unwired: 7 out]
        n527 = flat-sequence {
          frame #0 {
            n528 = Multiply(x="Delay to Interlace (s)", y=1000.0) -> (x*y=w892:dbl)
            n529 = Wait (ms)(milliseconds to wait=w892) -> ()  [unwired: 1 out]
          }
          frame #1 {
            n530 = property on="Green laser mode" class="RadioBtnsControl (strict)"("Val(Sgnl)"=enum32{"Laser ON", "Laser OFF", "Interlace"}."Interlace" ("Value (Signaling)")) -> ()  [unwired: 2 in, 2 out]
          }
        }
      }
      event "BD 1 Amplitude 1 (%)", "BD 1 Amplitude 2 (%)", "BD 1 Amplitude 3 (%)", "BD 2 Amplitude 1 (%)", "BD 2 Amplitude 2 (%)", "BD 2 Amplitude 3 (%)", "Trap 1 ON", "Trap 2 ON", "Trap 3 ON", "Feedback On/Off", "All FB On/Off": Value Change {
        w916 = i16 1 ("f")
        n531 = event-data() -> ()  [unwired: 7 out]
        n532 = local write "Trap 1 (ON/OFF)"("Trap 1 ON") -> ()
        n533 = local write "Trap 2 (ON/OFF)"("Trap 2 ON") -> ()
        n534 = Boolean To (0,1)(Boolean="Trap 3 ON") -> (0, 1=w917:i16)
        n535 = Boolean To (0,1)(Boolean="Trap 1 ON") -> (0, 1=w918:i16)
        n536 = Boolean To (0,1)(Boolean="Trap 2 ON") -> (0, 1=w919:i16)
        n537 = Select(t=w919, s="Trap ON/OFF X or Y Amp?", f=w916) -> (s? t:f=w914:i16)
        n538 = Select(t=w918, s="Trap ON/OFF X or Y Amp?", f=w916) -> (s? t:f=w915:i16)
        n539 = Select(t=w917, s="Trap ON/OFF X or Y Amp?", f=w916) -> (s? t:f=w913:i16)
        n540 = Select(t=w916, s="Trap ON/OFF X or Y Amp?", f=w919) -> (s? t:f=w911:i16)
        n541 = Select(t=w916, s="Trap ON/OFF X or Y Amp?", f=w918) -> (s? t:f=w912:i16)
        n542 = Select(t=w916, s="Trap ON/OFF X or Y Amp?", f=w917) -> (s? t:f=w910:i16)
        n543 = And(x="All FB On/Off", y="Feedback On/Off") -> (x .and. y?=w908:cluster{"Set 1":bool, "Set 2":bool})
        n544 = local read "BD 1 Amplitude 1 (%)"() -> (w928:dbl)
        n545 = local read "BD 1 Amplitude 2 (%)"() -> (w927:dbl)
        n546 = local read "BD 1 Amplitude 3 (%)"() -> (w926:dbl)
        n547 = Unbundle By Name(w908) -> ("Set 1"=w903:bool, "Set 2"=w900:bool)
        n548 = local read "Y RF Amplitude Limits (%)"() -> (w896:T16)
        n549 = local read "X RF Amplitude Limits (%)"() -> (w897:T16)
        n550 = local read "BD 2 Amplitude 1 (%)"() -> (w929:dbl)
        n551 = local read "BD 2 Amplitude 2 (%)"() -> (w930:dbl)
        n552 = local read "BD 2 Amplitude 3 (%)"() -> (w931:dbl)
        n553 = And(x="Trap 2 ON", y=w900) -> (x .and. y?=w898:bool)
        n554 = And(x="Trap 1 ON", y=w903) -> (x .and. y?=w901:bool)
        n555 = Multiply(x=w915, y=w928) -> (x*y=w923:dbl)
        n556 = Multiply(x=w927, y=w914) -> (x*y=w921:dbl)
        n557 = Multiply(x=w926, y=w913) -> (x*y=w922:dbl)
        n558 = Multiply(x=w929, y=w912) -> (x*y=w932:dbl)
        n559 = Multiply(x=w930, y=w911) -> (x*y=w933:dbl)
        n560 = Multiply(x=w931, y=w910) -> (x*y=w934:dbl)
        n561 = call "set RF board amplitude - interlace.vi"("Board 2 Amplitude Limits"=w896, "Board 1 Amplitude Limits"=w897, "error in"=w924, "FPGA VI Reference In"=w925, "Board 2 Amplitude 3 (%)"=w934, "Board 1 Amplitude 3 (%)"=w922, "Board 2 Amplitude 2 (%)"=w933, "Board 2 Amplitude 1 (%)"=w932, "Board 1 Amplitude 2 (%)"=w921, "Board 1 Amplitude 1 (%)"=w923) -> ("error out"=w905:errorcluster, "FPGA VI Reference Out"=w906:T19)
        n562 = xnode "Read/Write Control"("FPGA VI Reference In"=w906, "error in"=w905, "FB On/Off Set 1"=w901, "FB On/Off Set 2"=w898) -> ("error out"=w904:errorcluster)  [unwired: 1 out]
      }
      event "Load parameters": Value Change {
        n563 = event-data() -> ()  [unwired: 7 out]
        n564 = property on="Saved AOD Raster Scan Parameter Sets" class="Arr (strict)"() -> ("Index Values"=w945:u32[])  [unwired: 2 in, 2 out]
        n565 = Index Array(array=w945, index=0) -> (element=w942:u32)
        n566 = local write "Load parameters"(FALSE ("Load parameters")) -> ()
        n567 = Index Array(array="Saved AOD Raster Scan Parameter Sets", index=w942) -> (element=w941:T30)
        n568 = Unbundle By Name(w941) -> ("Scan Range AOD (nm) 2"=w940:dbl, "Step Size AOD (nm) 2"=w939:dbl, "Scan Speed AOD (nm/s) 2"=w938:dbl, "Number of scans (AOD) 2"=w937:u16)
        n569 = flat-sequence {
          tunnel: w940 -> [w948]
          tunnel: w939 -> [w947]
          tunnel: w938 -> [w946]
          tunnel: w937 -> [w949]
          frame #0 {
            n570 = local write "Scan Speed (nm/s)"(w946) -> ()
            n571 = local write "Scan Range (nm)"(w948) -> ()
            n572 = local write "Step Size (nm)"(w947) -> ()
          }
          frame #1 {
            n573 = property on="Number of F/B Scans (AOD)" class="DigNum (strict)"("Val(Sgnl)"=w949) -> ()  [unwired: 2 in, 2 out]
          }
        }
      }
      event "Trap 1 (ON/OFF)", "Trap 2 (ON/OFF)": Value Change {
        n574 = event-data() -> ()  [unwired: 7 out]
        n575 = property on="Trap 2 ON" class="Bool (strict)"("Val(Sgnl)"="Trap 2 (ON/OFF)") -> ()  [unwired: 2 in, 2 out]
        n576 = property on="Trap 1 ON" class="Bool (strict)"("Val(Sgnl)"="Trap 1 (ON/OFF)") -> ()  [unwired: 2 in, 2 out]
      }
      event "DIO count 1 (ticks)", "DIO count 2 (ticks)", "DIO count 3 (ticks)", "Interlace", "Number Interlace Sets", "Not-Interlacing Set": Value Change {
        n577 = event-data() -> ()  [unwired: 7 out]
        n578 = local read "DIO count 3 (ticks)"() -> (w962:u32)
        n579 = local read "DIO count 1 (ticks)"() -> (w964:u32)
        n580 = local read "DIO count 2 (ticks)"() -> (w963:u32)
        n581 = To Unsigned Byte Integer(number="Not-Interlacing Set") -> (unsigned 8bit integer=w953:u8)
        n582 = Add(x=w953, y=u8 1) -> (x+y=w957:u8)
        n583 = xnode "Read/Write Control"("FPGA VI Reference In"=w968, "error in"=w966, "DIO count 1 (ticks)"=w964, "DIO count 2 (ticks)"=w963, "DIO count 3 (ticks)"=w962, "Interlace ON/OFF"="Interlace", "Number Interlace Cycles"="Number Interlace Sets", "Interlace Off Parameters"=w957) -> ("error out"=w967:errorcluster)  [unwired: 1 out]
        n584 = Build Array(w964, w963, w962) -> (w955:u32[])
        n585 = Split 1D Array(array=w955, index="Number Interlace Sets") -> (first subarray=w965:u32[])  [unwired: 1 out]
        n586 = Index Array(array=w955, index=w953) -> (element=w954:u32)
        n587 = Add Array Elements(numeric array=w965) -> (sum=w959:u32)
        n588 = Select(t=w959, s="Interlace", f=w954) -> (s? t:f=→"Total Counts (ticks)":u32)
      }
      event "Reset Feedback": Value Change {
        n589 = event-data() -> ()  [unwired: 7 out]
        n590 = Unbundle By Name("Reset Feedback") -> ("Set 1"=w972:bool, "Set 2"=w971:bool)
        n591 = xnode "Read/Write Control"("FPGA VI Reference In"=w974, "error in"=w969, "FB Reset Set 1"=w972, "FB Reset Set 2"=w971) -> ("error out"=w970:errorcluster)  [unwired: 1 out]
      }
      event "PID Gains": Value Change {
        n592 = event-data() -> ()  [unwired: 7 out]
        n593 = Unbundle By Name("PID Gains") -> ("Set 1"=w978:T14, "Set 2"=w977:T14)
        n594 = xnode "Read/Write Control"("FPGA VI Reference In"=w979, "error in"=w975, "FB Gains Set 1"=w978, "FB Gains Set 2"=w977) -> ("error out"=w976:errorcluster)  [unwired: 1 out]
      }
      event "AI2 to Setpoint", "Trap Intensity\nSetpoints (V)": Value Change {
        n595 = event-data() -> ()  [unwired: 7 out]
        n596 = xnode "Read/Write Control"("FPGA VI Reference In"=w985, "error in"=w981) -> ("FPGA VI Reference Out"=w984:T19, "error out"=w983:errorcluster, "AI2 Y Sum Set 1"=w992:i16, "AI2 Y Sum Set 2"=w991:i16)
        n597 = Cluster To Array(cluster="AI2 to Setpoint") -> (array=w995:bool[])
        n598 = local read "AI2 (V)"() -> (w993:cluster{"Set 1":dbl, "Set 2":dbl})
        n599 = Or Array Elements(Boolean array=w995) -> (logical OR=w996:bool)
        n600 = Bundle By Name(cluster=w993, "Set 1"=w992, "Set 2"=w991) -> (w990:cluster{"Set 1":dbl, "Set 2":dbl})
        n601 = Divide(x=w990, y=3276.7) -> (x/y=w989:cluster{"Set 1":dbl, "Set 2":dbl})
        "AI2 (V)" <- w989
        n602 = case shown="True" w996 {
          tunnel: [w999 w1016] -> w988
          tunnel: "AI2 to Setpoint" -> [_ w1012]
          tunnel: "Trap Intensity\nSetpoints (V)" -> [w1000 w1015]
          tunnel: w989 -> [_ w1009]
          frame False {
            n603 = Multiply(x=3276.7, y=w1000) -> (x*y=w1001:cluster{"Set 1":dbl, "Set 2":dbl})
            n604 = To Word Integer(number=w1001) -> (16bit integer=w999:cluster{"Set 1":i16, "Set 2":i16})
          }
          frame True {
            n605 = Unbundle By Name(w1009) -> ("Set 1"=w1008:dbl, "Set 2"=w1007:dbl)
            n606 = Unbundle By Name(w1015) -> ("Set 1"=w1014:dbl, "Set 2"=w1013:dbl)
            n607 = Unbundle By Name(w1012) -> ("Set 1"=w1011:bool, "Set 2"=w1010:bool)
            n608 = Select(t=w1008, s=w1011, f=w1014) -> (s? t:f=w1006:dbl)
            n609 = Select(t=w1007, s=w1010, f=w1013) -> (s? t:f=w1005:dbl)
            n610 = Bundle By Name(cluster=w1015, "Set 1"=w1006, "Set 2"=w1005) -> (w1003:cluster{"Set 1":dbl, "Set 2":dbl})
            n611 = local write "Trap Intensity\nSetpoints (V)"(w1003) -> ()
            n612 = Multiply(x=3276.7, y=w1003) -> (x*y=w1004:cluster{"Set 1":dbl, "Set 2":dbl})
            n613 = To Word Integer(number=w1004) -> (16bit integer=w1016:cluster{"Set 1":i16, "Set 2":i16})
          }
        }
        n614 = Unbundle By Name(w988) -> ("Set 1"=w987:i16, "Set 2"=w986:i16)
        n615 = xnode "Read/Write Control"("FPGA VI Reference In"=w984, "error in"=w983, "FB Setpoint Set 1"=w987, "FB Setpoint Set 2"=w986) -> ("error out"=w982:errorcluster)  [unwired: 1 out]
      }
      event "Invert GI": Value Change {
        n616 = event-data() -> ()  [unwired: 7 out]
        n617 = xnode "Read/Write Control"("FPGA VI Reference In"=w1021, "error in"=w1019, "Invert GI"="Invert GI", "Invert GI 2"="Invert GI") -> ("error out"=w1020:errorcluster)  [unwired: 1 out]
      }
      event "Green FB Setpoint (mV)", "Green FB Gains", "Green FB On/Off", "Current When FB OFF (%)", "Green int current ON count adj": Value Change {
        n618 = event-data() -> ()  [unwired: 7 out]
        n619 = local read "Green FB Setpoint (mV)"() -> (w1028:dbl)
        n620 = local read "Current When FB OFF (%)"() -> (w1031:dbl)
        n621 = Multiply(x=w1028, y=3.2767) -> (x*y=w1027:dbl)
        n622 = Multiply(x=w1031, y=655.35) -> (x*y=w1032:dbl)
        n623 = To Unsigned Word Integer(number=w1032) -> (unsigned 16bit integer=w1030:u16)
        n624 = local read "Green int current ON count adj"() -> (w1035:u32)
        n625 = local read "Green FB Gains"() -> (w1034:T14)
        n626 = local read "Green Laser ON/Interlacing"() -> (w1025:bool)
        n627 = local read "Green laser mode"() -> (w1024:enum32{"Laser ON", "Laser OFF", "Interlace"})
        n628 = local read "Green FB On/Off"() -> (w1036:bool)
        n629 = Equal?(x=w1024, y=enum32{"Laser ON", "Laser OFF", "Interlace"}."Interlace") -> (x = y?=w1022:bool)
        n630 = Compound Arithmetic op=AND(w1022, w1036, w1025) -> (w1026:bool)
        n631 = xnode "Read/Write Control"("FPGA VI Reference In"=w1039, "error in"=w1038, "Green FB Setpoint"=w1027, "Green FB On/Off"=w1026, "Current Out"=w1030, "Green int current ON count adj"=w1035, "Green FB Gains"=w1034) -> ("error out"=w1037:errorcluster)  [unwired: 1 out]
      }
      event "Green laser mode", "Green Laser ON/Interlacing": Value Change {
        n632 = event-data() -> ()  [unwired: 7 out]
        n633 = case shown="True" "Green Laser ON/Interlacing" {
          tunnel: "Green laser mode" -> [_ w1053]
          tunnel: [enum32{"Laser ON", "Laser OFF", "Interlace"}."Laser OFF" ("Green laser mode") w1053] -> w1041
          tunnel: [FALSE w1049] -> w1040
          frame False {
          }
          frame True {
            n634 = local read "Green FB On/Off"() -> (w1050:bool)
            n635 = Equal?(x=w1053, y=enum32{"Laser ON", "Laser OFF", "Interlace"}."Interlace") -> (x = y?=w1051:bool)
            n636 = And(x=w1051, y=w1050) -> (x .and. y?=w1049:bool)
          }
        }
        n637 = xnode "Read/Write Control"("FPGA VI Reference In"=w1046, "error in"=w1044, "Operating Mode"=w1041, "Operating Mode 2"=w1041, "Green FB On/Off"=w1040) -> ("error out"=w1045:errorcluster)  [unwired: 1 out]
      }
      event "- phase (APD 1 Gate)", "+ phase (APD 1 Gate)": Value Change {
        n638 = event-data() -> ()  [unwired: 7 out]
        n639 = local read "Phase Adj. (APD 1 Gate)"() -> (w1054:i16)
        n640 = Negate(x=w1054) -> (-x=w1062:i16)
        n641 = Select(t=w1062, s="- phase (APD 1 Gate)", f=w1054) -> (s? t:f=w1061:i16)
        n642 = Or(x="- phase (APD 1 Gate)", y="+ phase (APD 1 Gate)") -> (x .or. y?=w1057:bool)
        n643 = xnode "Read/Write Control"("FPGA VI Reference In"=w1064, "error in"=w1063, "Phase count adjustment (APD 1 Gate)"=w1061) -> ("FPGA VI Reference Out"=w1059:T19, "error out"=w1060:errorcluster)
        n644 = xnode "Read/Write Control"("FPGA VI Reference In"=w1059, "error in"=w1060, "+ phase (APD 1 Gate)"=w1057) -> ("error out"=w1058:errorcluster)  [unwired: 1 out]
      }
      event "+ phase (APD 2 Gate)", "- phase (APD 2 Gate)": Value Change {
        n645 = event-data() -> ()  [unwired: 7 out]
        n646 = local read "Phase Adj. (APD 2 Gate)"() -> (w1065:i16)
        n647 = Negate(x=w1065) -> (-x=w1073:i16)
        n648 = Select(t=w1073, s="- phase (APD 2 Gate)", f=w1065) -> (s? t:f=w1072:i16)
        n649 = Or(x="- phase (APD 2 Gate)", y="+ phase (APD 2 Gate)") -> (x .or. y?=w1068:bool)
        n650 = xnode "Read/Write Control"("FPGA VI Reference In"=w1075, "error in"=w1074, "Phase count adjustment (APD 2 Gate)"=w1072) -> ("FPGA VI Reference Out"=w1070:T19, "error out"=w1071:errorcluster)
        n651 = xnode "Read/Write Control"("FPGA VI Reference In"=w1070, "error in"=w1071, "+ phase (APD 2 Gate)"=w1068) -> ("error out"=w1069:errorcluster)  [unwired: 1 out]
      }
      event "Phase Adj. (APD Acq)", "+ phase (APD Acq)", "- phase (APD Acq)": Value Change {
        n652 = event-data() -> ()  [unwired: 7 out]
        n653 = local read "Phase Adj. (APD Acq)"() -> (w1078:i16)
        n654 = Negate(x=w1078) -> (-x=w1084:i16)
        n655 = Select(t=w1084, s="+ phase (APD Acq)", f=w1078) -> (s? t:f=w1083:i16)
        n656 = Or(x="+ phase (APD Acq)", y="- phase (APD Acq)") -> (x .or. y?=w1079:bool)
        n657 = xnode "Read/Write Control"("FPGA VI Reference In"=w1086, "error in"=w1085, "Phase Count Adjustment (APD Acq)"=w1083) -> ("FPGA VI Reference Out"=w1081:T19, "error out"=w1082:errorcluster)
        n658 = xnode "Read/Write Control"("FPGA VI Reference In"=w1081, "error in"=w1082, "+ phase (APD Acq)"=w1079) -> ("error out"=w1080:errorcluster)  [unwired: 1 out]
      }
      event "Phase adj. (GI)", "+ phase (GI)", "- phase (GI)": Value Change {
        n659 = event-data() -> ()  [unwired: 7 out]
        n660 = Negate(x="Phase adj. (GI)") -> (-x=w1095:i16)
        n661 = Select(t=w1095, s="+ phase (GI)", f="Phase adj. (GI)") -> (s? t:f=w1094:i16)
        n662 = Or(x="+ phase (GI)", y="- phase (GI)") -> (x .or. y?=w1090:bool)
        n663 = xnode "Read/Write Control"("FPGA VI Reference In"=w1097, "error in"=w1096, "Phase count adjustment (GI)"=w1094) -> ("FPGA VI Reference Out"=w1092:T19, "error out"=w1093:errorcluster)
        n664 = xnode "Read/Write Control"("FPGA VI Reference In"=w1092, "error in"=w1093, "+ phase (GI)"=w1090) -> ("error out"=w1091:errorcluster)  [unwired: 1 out]
      }
      event "Phase adj. (GI) 2", "+ phase (GI) 2", "- phase (GI) 2": Value Change {
        n665 = event-data() -> ()  [unwired: 7 out]
        n666 = Negate(x="Phase adj. (GI) 2") -> (-x=w1106:i16)
        n667 = Select(t=w1106, s="+ phase (GI) 2", f="Phase adj. (GI) 2") -> (s? t:f=w1105:i16)
        n668 = Or(x="+ phase (GI) 2", y="- phase (GI) 2") -> (x .or. y?=w1101:bool)
        n669 = xnode "Read/Write Control"("FPGA VI Reference In"=w1108, "error in"=w1107, "Phase count adjustment (GI) 2"=w1105) -> ("FPGA VI Reference Out"=w1103:T19, "error out"=w1104:errorcluster)
        n670 = xnode "Read/Write Control"("FPGA VI Reference In"=w1103, "error in"=w1104, "+ phase (GI) 2"=w1101) -> ("error out"=w1102:errorcluster)  [unwired: 1 out]
      }
      event "Phase adj. (Green FB)", "- phase (Green FB)", "+ phase (Green FB)": Value Change {
        n671 = event-data() -> ()  [unwired: 7 out]
        n672 = Negate(x="Phase adj. (Green FB)") -> (-x=w1117:i16)
        n673 = Select(t=w1117, s="+ phase (Green FB)", f="Phase adj. (Green FB)") -> (s? t:f=w1116:i16)
        n674 = Or(x="+ phase (Green FB)", y="- phase (Green FB)") -> (x .or. y?=w1112:bool)
        n675 = xnode "Read/Write Control"("FPGA VI Reference In"=w1119, "error in"=w1118, "Phase count adjustment (Green FB)"=w1116) -> ("FPGA VI Reference Out"=w1114:T19, "error out"=w1115:errorcluster)
        n676 = xnode "Read/Write Control"("FPGA VI Reference In"=w1114, "error in"=w1115, "+ phase (Green FB)"=w1112) -> ("error out"=w1113:errorcluster)  [unwired: 1 out]
      }
      event "Invert APD Gate", "APD Gate ON Count", "APD Gate OFF Count", "APD Gate", "APD Integration Time (s)", "APD 1 AO Mult.", "APD 2 AO Mult.": Value Change {
        n677 = event-data() -> ()  [unwired: 7 out]
        n678 = local read "APD Integration Time (s)"() -> (w1120:dbl)
        n679 = local read "APD Gate ON Count"() -> (w1133:u32)
        n680 = local read "APD Gate OFF Count"() -> (w1132:u32)
        n681 = local read "Invert APD Gate"() -> (w1134:bool)
        n682 = local read "APD Gate"() -> (w1131:enum32{"ON", "OFF", "Interlace"})
        n683 = Multiply(x=w1120, y=40000000.0) -> (x*y=w1129:dbl)
        n684 = Reciprocal(x=w1120) -> (1/x=→"APD Acq Rate (Hz)":dbl)
        n685 = To Unsigned Long Integer(number=w1129) -> (unsigned 32bit integer=w1128:u32)
        n686 = local read "DMA Update Period (s)"() -> (w1121:dbl)
        n687 = Divide(x=w1121, y=w1120) -> (x/y=w1124:dbl)
        n688 = local read "APD 1 AO Mult."() -> (w1126:i16)
        n689 = local read "APD 2 AO Mult."() -> (w1125:i16)
        n690 = Multiply(x=2.0, y=w1124) -> (x*y=w1123:dbl)
        n691 = local write "APD Samples/FIFO Acq."(w1124) -> ()
        n692 = local write "APD Elements/DMA read"(w1123) -> ()
        n693 = xnode "Read/Write Control"("FPGA VI Reference In"=w1137, "error in"=w1136, "Invert APD Gate"=w1134, "APD Gate ON Count"=w1133, "APD Gate OFF Count"=w1132, "APD Acq Rate Count"=w1128, "APD Gate Operating Mode"=w1131, "APD 1 AO scale factor"=w1126, "APD 2 AO scale factor"=w1125) -> ("error out"=w1135:errorcluster)  [unwired: 1 out]
      }
      event "GI Frequency, ON count", "Green FB Count", "GI Frequency, OFF count": Value Change {
        n694 = event-data() -> ()  [unwired: 7 out]
        n695 = xnode "Read/Write Control"("FPGA VI Reference In"=w1143, "error in"=w1141, "Green interlace ON count"="GI Frequency, ON count", "Green interlace OFF count"="GI Frequency, OFF count", "Green interlace ON count 2"="GI Frequency, ON count", "Green interlace OFF count 2"="GI Frequency, OFF count", "Green FB Count"="Green FB Count") -> ("error out"=w1142:errorcluster)  [unwired: 1 out]
      }
      event "Number of F/B Scans (AOD)", "Scan Speed (nm/s)", "Scan BD", "Initial delta (MHz)", "Step Size (nm)", "Scan Range (nm)": Value Change {
        w1205 = 123.0  # AOM cal (nm/MHz)
        n696 = event-data() -> ()  [unwired: 7 out]
        n697 = local read "BD 1 Frequency 1 (MHz)"() -> (w1188:dbl)
        n698 = local read "AOM X Cal (nm/MHz)"() -> (w1180:dbl)
        n699 = local read "X RF Frequency Limits (MHz)"() -> (w1192:T16)
        n700 = local read "Y RF Frequency Limits (MHz)"() -> (w1189:T16)
        n701 = local read "BD 2 Frequency 1 (MHz)"() -> (w1194:dbl)
        n702 = Negate(x="Scan Range (nm)") -> (-x=w1158:dbl)
        n703 = Divide(x=w1158, y=w1180) -> (x/y=w1162:dbl)
        n704 = Select(t=w1192, s="Scan BD", f=w1189) -> (s? t:f=w1191:T16)
        n705 = Select(t=w1188, s="Scan BD", f=w1194) -> (s? t:f=w1193:dbl)
        n706 = Unbundle By Name(w1191) -> ("Maximum"=w1200:dbl, "Minimum"=w1199:dbl)
        n707 = Add(x=w1162, y=w1193) -> (x+y=w1197:dbl)
        n708 = Divide(x=w1158, y="Step Size (nm)") -> (x/y=w1177:dbl)
        n709 = Divide(x="Step Size (nm)", y=w1180) -> (x/y=w1186:dbl)
        n710 = Absolute Value(x=w1177) -> (abs(x)=w1161:dbl)
        n711 = Sign(1:w1158) -> (0:w1159:dbl)
        n712 = In Range and Coerce(upper limit=w1200, x=w1197, lower limit=w1199) -> (coerced(x)=w1196:dbl, In Range?=w1198:bool)
        n713 = To Unsigned Quad Integer(1:w1161) -> (0:w1176:u64)
        "Scan steps (AOD)" <- w1176
        n714 = call "IR AOM freq to word.vi"("Frequency In (MHz)"=w1186) -> ("Frequency Word Out (double)"=w1183:dbl)
        n715 = Multiply(x=w1159, y=w1183) -> (x*y=w1160:dbl)
        n716 = Subtract(x=w1197, y=w1196) -> (x-y=w1195:dbl)
        n717 = To Quad Integer(1:w1160) -> (0:w1182:i64)
        "Incr. int (AOD)" <- w1182
        n718 = Subtract(x=w1162, y=w1195) -> (x-y=w1181:dbl)
        "Scan Range (MHz)" <- w1181
        n719 = Select(t=w1162, s=w1198, f=w1181) -> (s? t:f=w1201:dbl)
        n720 = Multiply(x=w1181, y=w1180) -> (x*y=w1179:dbl)
        n721 = Decrement(x=w1176) -> (x-1=w1229:u64)
        n722 = Negate(x=w1179) -> (-x=w1175:dbl)
        n723 = local write "Scan Range (nm)"(w1175) -> ()
        n724 = Divide(x=w1201, y=w1229) -> (x/y=w1185:dbl)
        "Scan Increment (MHz)" <- w1185
        n725 = call "IR AOM freq to word.vi"("Frequency In (MHz)"=w1185) -> ("Frequency Word Out (double)"=w1184:dbl)
        n726 = Divide(x="Step Size (nm)", y="Scan Speed (nm/s)") -> (x/y=w1172:dbl)
        n727 = To Quad Integer(1:w1184) -> ()  [unwired: 1 out]
        n728 = local read "Number Interlace Sets"() -> (w1156:u8)
        n729 = local read "AI Count (ticks)"() -> (w1157:u32)
        n730 = local read "Total Counts (ticks)"() -> (w1155:u32)
        n731 = local read "# Samples/trap"() -> (w1187:u32)
        n732 = Multiply(x=w1157, y=w1156) -> (x*y=w1154:u32)
        n733 = Divide(x=w1155, y=w1154) -> (x/y=w1153:dbl)
        n734 = Select(t=w1188, s="Scan BD", f=w1194) -> (s? t:f=w1226:dbl)
        "Initial freq. (MHz)" <- w1226
        n735 = Add(x=w1201, y=w1226) -> (x+y=→"Final freq. (MHz)":dbl)
        n736 = Divide(x=w1155, y=40000000.0) -> (x/y=w1171:dbl)
        n737 = Divide(x=w1172, y=w1171) -> (x/y=w1170:dbl)
        n738 = To Unsigned Quad Integer(1:w1170) -> (0:w1145:u64)
        n739 = Quotient & Remainder(x=w1145, y=u64 2) -> (x-y*floor(x/y)=w1149:u64)  [unwired: 1 out]
        n740 = Equal?(x=w1149, y=u64 0) -> (x = y?=w1147:bool)
        n741 = Decrement(x=w1145) -> (x-1=w1146:u64)
        n742 = Select(t=w1145, s=w1147, f=w1146) -> (s? t:f=w1144:u64)
        "Cycles/step (AOD)" <- w1144
        n743 = xnode "Read/Write Control"("FPGA VI Reference In"=w1237, "error in"=w1236, "Scan steps"=w1176, "Number of scans"="Number of F/B Scans (AOD)", "Cycles per step"=w1144, "Scan freq.  increment"=w1182, "Scan BD"="Scan BD") -> ("error out"=w1235:errorcluster)  [unwired: 1 out]
        n744 = Multiply(x=w1176, y=w1144) -> (x*y=w1230:u64)
        n745 = Multiply(x=w1230, y=u64 2) -> (x*y=w1152:u64)
        n746 = Multiply(x=w1153, y=w1152) -> (x*y=w1151:dbl)
        "Data points/scan (f/b)" <- w1151
        n747 = Multiply(x=w1151, y="Number of F/B Scans (AOD)") -> (x*y=w1233:dbl)
        "Data points/scans" <- w1233
        n748 = Divide(x=w1233, y=w1187) -> (x/y=→"N sets should be saved":dbl)
        n749 = Multiply(x=w1230, y=w1171) -> (x*y=w1169:dbl)
        "Time/Scan (s) (AOD)" <- w1169
        n750 = Select(t=w1201, s="Scan BD", f=0.0) -> (s? t:f=w1227:dbl)
        n751 = Select(t=0.0, s="Scan BD", f=w1201) -> (s? t:f=w1223:dbl)
        n752 = local read "BD 2 Frequency 2 (MHz)"() -> (w1219:dbl)
        n753 = local read "BD 1 Frequency 2 (MHz)"() -> (w1222:dbl)
        n754 = Add(x=w1223, y=w1194) -> (x+y=w1220:dbl)
        n755 = Add(x=w1188, y=w1227) -> (x+y=w1221:dbl)
        n756 = Multiply(x=w1169, y=2.0) -> (x*y=w1168:dbl)
        n757 = Multiply(x=w1168, y="Number of F/B Scans (AOD)") -> (x*y=w1165:dbl)
        n758 = Divide(x=w1165, y=60.0) -> (x/y=→"Time to Finish All (min)":dbl)
        n759 = Add(x="Trap 2 Bead Size (nm)", y="Trap 1 Bead Size (nm)") -> (x+y=w1209:dbl)
        n760 = local read "Initial delta (MHz)"() -> (w1206:dbl)
        n761 = Divide(x=w1209, y=2.0) -> (x/y=w1203:dbl)
        n762 = Subtract(x=w1220, y=w1219) -> (x-y=w1217:dbl)
        n763 = Subtract(x=w1221, y=w1222) -> (x-y=w1218:dbl)
        n764 = Square(x=w1217) -> (x^2=w1216:dbl)
        n765 = Square(x=w1218) -> (x^2=w1215:dbl)
        n766 = Add(x=w1215, y=w1216) -> (x+y=w1214:dbl)
        n767 = Square Root(x=w1214) -> (sqrt(x)=w1213:dbl)
        "Final delta (MHz)" <- w1213
        n768 = Multiply(x=w1205, y=w1213) -> (x*y=w1212:dbl)
        n769 = Multiply(x=w1206, y=w1205) -> (x*y=w1204:dbl)
        n770 = Subtract(x=w1204, y=w1203) -> (x-y=→"Initial sep (nm)":dbl)
        n771 = Subtract(x=w1212, y=w1203) -> (x-y=→"Final sep (nm)":dbl)
      }
      event "Raster Scanning...": Value Change {
        n772 = event-data() -> ("NewVal"=w1238:bool)  [unwired: 6 out]
        n773 = case shown="True" w1238 {
          frame False {
          }
          frame True {
            n774 = property on="BD 1 Frequency 1 (MHz)" class="DigNum (strict)"("Val(Sgnl)"=65.0 ("Value (Signaling)")) -> ()  [unwired: 2 in, 2 out]
          }
        }
      }
      event "Freq or Amp switch first", "Swap F1 and F2", "Freq switch delay", "Amp switch delay": Value Change {
        n775 = event-data() -> ()  [unwired: 7 out]
        n776 = local read "Freq or Amp switch first"() -> (w1240:bool)
        n777 = local read "Amp switch delay"() -> (w1241:u16)
        n778 = local read "Freq switch delay"() -> (w1243:u16)
        n779 = local read "Swap F1 and F2"() -> (w1242:bool)
        n780 = xnode "Read/Write Control"("FPGA VI Reference In"=w1246, "error in"=w1245, "Freq switch delay"=w1243, "Swap F1 and F2"=w1242, "Amp switch delay"=w1241, "Freq or Amp switch first"=w1240) -> ("error out"=w1244:errorcluster)  [unwired: 1 out]
      }
      event "Scan steps (MCL)", "Number of scans (MCL)", "Scan Range (V)\n(of steps)", "2D or 1D Scan", "N APD Samp/step", "Fast Scan Dir", "Continuous MCL Scanning", "Scan lines (y)": Value Change {
        w1248 = 32767.0 ("y")
        n781 = event-data() -> ()  [unwired: 7 out]
        n782 = Select(t="Scan lines (y)", s="2D or 1D Scan", f="Number of scans (MCL)") -> (s? t:f=w1253:u64)
        n783 = Decrement(x="Scan steps (MCL)") -> (x-1=w1269:u64)
        n784 = Divide(x="Scan Range (V)\n(of steps)", y=w1269) -> (x/y=w1268:dbl)
        "Desired Scan Incr (V)" <- w1268
        n785 = local read "APD Integration Time (s)"() -> (w1261:dbl)
        n786 = Multiply(x=w1268, y=w1248) -> (x*y=w1277:dbl)
        n787 = Divide(x=w1277, y=10.0) -> (x/y=w1267:dbl)
        "Desired incr (int)" <- w1267
        n788 = local read "Update Count (MCL)"() -> (w1273:u32)
        n789 = Round Toward -Infinity(1:w1267) -> (0:w1276:dbl)
        n790 = To Word Integer(number=w1276) -> (16bit integer=w1251:i16)
        "Actual Incr. int (MCL)" <- w1251
        n791 = Multiply(x=w1261, y=40000000.0) -> (x*y=w1274:dbl)
        n792 = Divide(x=w1274, y=w1273) -> (x/y=w1272:dbl)
        n793 = Multiply(x=i16 10, y=w1251) -> (x*y=w1249:i16)
        n794 = Multiply(x="N APD Samp/step", y=w1272) -> (x*y=w1271:dbl)
        "Cycles/step (MCL)" <- w1271
        n795 = Divide(x=w1249, y=w1248) -> (x/y=→"Actual MCL Inc (V)":dbl)
        n796 = Multiply(x="N APD Samp/step", y="Scan steps (MCL)") -> (x*y=w1263:dbl)
        n797 = local read "APD Samples/FIFO Acq."() -> (w1260:dbl)
        n798 = Multiply(x=w1263, y=u64 2) -> (x*y=w1262:dbl)
        "Data points/scan (f+b)" <- w1262
        n799 = Multiply(x=w1262, y=w1253) -> (x*y=w1280:dbl)
        "Data points/scans (MCL)" <- w1280
        n800 = Multiply(x=w1261, y=w1262) -> (x*y=w1254:dbl)
        "Time/f+b scan (s) (MCL)" <- w1254
        n801 = Divide(x=w1280, y=w1260) -> (x/y=→"N sets should be saved (MCL)":dbl)
        n802 = Multiply(x=w1254, y=w1253) -> (x*y=→"Total Time (s)":dbl)
        n803 = Not(x="Fast Scan Dir") -> (.not. x?=w1258:bool)
        n804 = xnode "Read/Write Control"("FPGA VI Reference In"=w1284, "error in"=w1283, "Scan steps (MCL)"="Scan steps (MCL)", "Number of scans (MCL)"=w1253, "Cycles per step (MCL)"=w1271, "Scan freq.  increment (MCL)"=w1251, "1D or 2D Scan?"="2D or 1D Scan", "MCL Scan Axis"=w1258, "Cont. Scan (MCL)"="Continuous MCL Scanning") -> ("error out"=w1282:errorcluster)  [unwired: 1 out]
      }
      event "Read Cal": Value Change {
        w1286 = 1000.0 ("y")
        n805 = event-data() -> ()  [unwired: 7 out]
        n806 = local read "Save file name"() -> (w1311:path)
        n807 = local write "Read Cal"(FALSE ("Read Cal")) -> ()
        n808 = Strip Path(path=w1311) -> (stripped path=w1310:path)  [unwired: 1 out]
        n809 = Path To String(path=w1310) -> (string=w1309:string)
        n810 = Concatenate Strings(w1309, "\\current.cal" ("string")) -> (w1307:string)
        n811 = String To Path(string=w1307) -> (path=w1306:path)
        n812 = Open/Create/Replace File(file path (use dialog)=w1306, operation (0:open)=T23."open", access (0:read/write)=enum16{"read/write", "read-only", "write-only"}."read-only") -> (refnum out=w1314:refnum<file>, error out=w1300:errorcluster)  [unwired: 1 in, 3 out]
        n813 = Deny Access(4:w1300, 7:w1314) -> (0:w1299:errorcluster, 3:w1305:refnum<file>)  [unwired: 1 out]
        n814 = Read from Binary File(5:0.0, 8:w1299, 9:T29."big-endian, network order" ("byte order (0:big-endian, network order)"), 10:-1 ("count (1)"), 11:w1305) -> (0:w1298:errorcluster, 2:w1296:dbl[], 3:w1301:refnum<file>)  [unwired: 2 out]
        n815 = Array To Cluster(array=w1296) -> (cluster=w1295:T31)
        n816 = Unbundle(w1295) -> ("[0]"=w1294:dbl, "[1]"=w1293:dbl, "[2]"=w1292:dbl, "[3]"=w1291:dbl, "[4]"=w1290:dbl, "[5]"=w1289:dbl)
        n817 = Close File(refnum=w1301, error in=w1298) -> (error out=→"Read cal error":errorcluster)  [unwired: 1 out]
        n818 = Multiply(x=w1289, y=w1286) -> (x*y=w1287:dbl)
        n819 = local write "T2 kappa_x (pN/nm)"(w1291) -> ()
        n820 = local write "T1 kappa_x (pN/nm)"(w1292) -> ()
        n821 = local write "T1 alpha_x (nm/V)"(w1294) -> ()
        n822 = local write "T2 alpha_x (nm/V)"(w1293) -> ()
        n823 = Multiply(x=w1290, y=w1286) -> (x*y=w1288:dbl)
        n824 = local write "T1 offset_x (mV)"(w1288) -> ()
        n825 = local write "T2 offset_x (mV)"(w1287) -> ()
      }
      event "Abort MCL Scan": Value Change {
        n826 = event-data() -> ()  [unwired: 7 out]
        n827 = local write "MCL Scanning"(FALSE ("MCL Scanning")) -> ()
        n828 = xnode "Read/Write Control"("FPGA VI Reference In"=w1319, "error in"=w1318, "Abort scan (MCL)"="Abort MCL Scan") -> ("error out"=w1317:errorcluster)  [unwired: 1 out]
      }
      event "Update Count (MCL)": Value Change {
        n829 = event-data() -> ()  [unwired: 7 out]
        n830 = xnode "Read/Write Control"("FPGA VI Reference In"=w1323, "error in"=w1322, "MCL count"="Update Count (MCL)") -> ("error out"=w1321:errorcluster)  [unwired: 1 out]
      }
      event "Phase adjust (MCL)", "+ phase (MCL)", "- phase (MCL)": Value Change {
        n831 = event-data() -> ()  [unwired: 7 out]
        n832 = Negate(x="Phase adjust (MCL)") -> (-x=w1332:i16)
        n833 = Select(t=w1332, s="- phase (MCL)", f="Phase adjust (MCL)") -> (s? t:f=w1330:i16)
        n834 = Or(x="- phase (MCL)", y="+ phase (MCL)") -> (x .or. y?=w1325:bool)
        n835 = xnode "Read/Write Control"("FPGA VI Reference In"=w1334, "error in"=w1333, "Phase count adjustment (MCL)"=w1330) -> ("FPGA VI Reference Out"=w1326:T19, "error out"=w1327:errorcluster)
        n836 = xnode "Read/Write Control"("FPGA VI Reference In"=w1326, "error in"=w1327, "+ phase (MCL)"=w1325) -> ("error out"=w1324:errorcluster)  [unwired: 1 out]
      }
      event "Abort AOD Scan": Value Change {
        n837 = event-data() -> ()  [unwired: 7 out]
        n838 = xnode "Read/Write Control"("FPGA VI Reference In"=w1338, "error in"=w1337, "Abort scan"="Abort AOD Scan") -> ("error out"=w1336:errorcluster)  [unwired: 1 out]
      }
      event "Continuous AOD Scanning": Value Change {
        n839 = event-data() -> ()  [unwired: 7 out]
        n840 = xnode "Read/Write Control"("FPGA VI Reference In"=w1342, "error in"=w1341, "Cont. Scan"="Continuous AOD Scanning") -> ("error out"=w1340:errorcluster)  [unwired: 1 out]
      }
      event "Index": Value Change {
        n841 = event-data() -> ()  [unwired: 7 out]
        n842 = call "Create new save file.vi"("Insert"="", "Ext"=".dat" ("string"), "Index In"="Index") -> ("Path Out"=→"Save file name":path, "Index Out"=w1343:dbl)
        "Save index" <- w1343
        n843 = local write "Index"(w1343) -> ()
      }
      event "AO1", "AO2": Value Change {
        w1358 = 10.0 ("y")
        w1357 = 32767.0 ("y")
        n844 = event-data() -> ()  [unwired: 7 out]
        n845 = local read "AO2"() -> (w1356:dbl)
        n846 = local read "AO1"() -> (w1353:dbl)
        n847 = Multiply(x=w1353, y=w1357) -> (x*y=w1352:dbl)
        n848 = Multiply(x=w1356, y=w1357) -> (x*y=w1355:dbl)
        n849 = Divide(x=w1352, y=w1358) -> (x/y=w1351:dbl)
        n850 = Divide(x=w1355, y=w1358) -> (x/y=w1354:dbl)
        n851 = To Word Integer(number=w1351) -> (16bit integer=w1359:i16)
        n852 = To Word Integer(number=w1354) -> (16bit integer=w1360:i16)
        n853 = xnode "Read/Write Control"("FPGA VI Reference In"=w1350, "error in"=w1349, "AO1"=w1359, "AO2"=w1360) -> ("error out"=w1348:errorcluster)  [unwired: 1 out]
      }
      event "Inject Bottom": Value Change {
        n854 = event-data() -> ()  [unwired: 7 out]
        n855 = disable-structure shown="Enabled" {
          disable-tunnel: "Inject Bottom" -> [w1362 w1402]
          frame Disabled {
            n856 = local read "Chemyx Syringe Pump Serial Port"() -> (w1363:refnum<visa-resource-name>)
            n857 = local read "Pump write delay (ms)"() -> (w1364:dbl)
            n858 = case shown="True" w1362 {
              tunnel: w1364 -> [w1370 w1384]
              tunnel: w1363 -> [w1367 w1383]
              frame False {
                n859 = flat-sequence {
                  tunnel: w1367 -> [w1371]
                  tunnel: [w1371] -> w1368
                  tunnel: w1370 -> [_]
                  tunnel: [w1374] -> w1369
                  tunnel: w1368 -> [w1374]
                  tunnel: w1369 -> [w1375]
                  tunnel: [w1375] -> w1365
                  tunnel: [w1377] -> w1366
                  tunnel: w1365 -> [w1377]
                  tunnel: w1366 -> [w1379]
                  frame #0 {
                    n860 = call "Write to pump.vi"("string"="enter pump1", "VISA resource name"=w1371) -> ()  [unwired: 1 out]
                  }
                  frame #1 {
                    n861 = Wait (ms)(milliseconds to wait="Pump pause delay (ms)") -> ()  [unwired: 1 out]
                  }
                  frame #2 {
                    n862 = call "Write to pump.vi"("string"="stop", "VISA resource name"=w1375) -> ()  [unwired: 1 out]
                  }
                  frame #3 {
                    n863 = Wait (ms)(milliseconds to wait=u32 500) -> ()  [unwired: 1 out]
                  }
                  frame #4 {
                    n864 = call "Write to pump.vi"("string"="stop", "VISA resource name"=w1379) -> ()  [unwired: 1 out]
                  }
                }
              }
              frame True {
                n865 = flat-sequence {
                  tunnel: w1383 -> [w1393]
                  tunnel: w1384 -> [w1388]
                  tunnel: w1384 -> [w1395]
                  tunnel: w1383 -> [w1396]
                  tunnel: [w1396] -> w1381
                  tunnel: [w1398] -> w1382
                  tunnel: w1381 -> [w1398]
                  tunnel: w1382 -> [w1400]
                  frame #0 {
                    n866 = local read "All Pump Parameters"() -> (w1387:T5)
                    n867 = Unbundle By Name(w1387) -> ("Pump 1"=w1394:T32)
                    n868 = call "Set pump parameters.vi"("Pump write delay (ms)"=w1388, "Volume (uL)"="Ch 2 Inject Volume (uL)", "Rate (uL/h)"="Ch 1 Inject Rate (ul/h)", "Units"=4.0, "Pump #"=1.0, "Pump Parameters In"=w1394, "VISA resource name"=w1393) -> ("Pump Parameters Out"=w1386:T32)  [unwired: 3 in]
                    n869 = Bundle By Name(cluster=w1387, "Pump 1"=w1386) -> (w1385:T5)
                    n870 = local write "All Pump Parameters"(w1385) -> ()
                  }
                  frame #1 {
                    n871 = Wait (ms)(milliseconds to wait=w1395) -> ()  [unwired: 1 out]
                  }
                  frame #2 {
                    n872 = call "Write to pump.vi"("string"="start", "VISA resource name"=w1396) -> ()  [unwired: 1 out]
                  }
                  frame #3 {
                    n873 = Wait (ms)(milliseconds to wait=u32 500) -> ()  [unwired: 1 out]
                  }
                  frame #4 {
                    n874 = call "Write to pump.vi"("string"="start", "VISA resource name"=w1400) -> ()  [unwired: 1 out]
                  }
                }
              }
            }
          }
          frame Enabled {
            n875 = call "hamilton_controller.vi"("Open?"=w1402, "valve"=enum16{"A", "B", "C", "D", "ALL"}."B", "action"=T20."MOVE VALVE") -> ()  [unwired: 8 in, 1 out]
          }
        }
      }
      event "Inject Top": Value Change {
        n876 = event-data() -> ()  [unwired: 7 out]
        n877 = disable-structure shown="Disabled" {
          disable-tunnel: "Inject Top" -> [_ w1446]
          frame Disabled {
            n878 = local read "Pump write delay (ms)"() -> (w1407:dbl)
            n879 = case shown="False" w1408 {
              tunnel: w1407 -> [w1414 w1428]
              tunnel: "Chemyx Syringe Pump Serial Port" -> [w1411 w1427]
              frame False {
                n880 = flat-sequence {
                  tunnel: w1411 -> [w1415]
                  tunnel: [w1415] -> w1412
                  tunnel: w1414 -> [_]
                  tunnel: [w1418] -> w1413
                  tunnel: w1412 -> [w1418]
                  tunnel: w1413 -> [w1419]
                  tunnel: [w1419] -> w1409
                  tunnel: [w1421] -> w1410
                  tunnel: w1409 -> [w1421]
                  tunnel: w1410 -> [w1423]
                  frame #0 {
                    n881 = call "Write to pump.vi"("string"="enter pump3", "VISA resource name"=w1415) -> ()  [unwired: 1 out]
                  }
                  frame #1 {
                    n882 = local read "Pump pause delay (ms)"() -> (w1417:u32)
                    n883 = Wait (ms)(milliseconds to wait=w1417) -> ()  [unwired: 1 out]
                  }
                  frame #2 {
                    n884 = call "Write to pump.vi"("string"="stop", "VISA resource name"=w1419) -> ()  [unwired: 1 out]
                  }
                  frame #3 {
                    n885 = Wait (ms)(milliseconds to wait=u32 0) -> ()  [unwired: 1 out]
                  }
                  frame #4 {
                    n886 = call "Write to pump.vi"("string"="stop", "VISA resource name"=w1423) -> ()  [unwired: 1 out]
                  }
                }
              }
              frame True {
                n887 = flat-sequence {
                  tunnel: w1427 -> [w1437]
                  tunnel: w1428 -> [w1432]
                  tunnel: w1428 -> [w1439]
                  tunnel: w1427 -> [w1440]
                  tunnel: [w1440] -> w1425
                  tunnel: [w1443] -> w1426
                  tunnel: w1425 -> [w1443]
                  tunnel: w1426 -> [w1444]
                  frame #0 {
                    n888 = local read "All Pump Parameters"() -> (w1431:T5)
                    n889 = Unbundle By Name(w1431) -> ("Pump 3"=w1438:T32)
                    n890 = call "Set pump parameters.vi"("Pump write delay (ms)"=w1432, "Volume (uL)"="Ch 3 Inject Volume (uL)", "Rate (uL/h)"="Ch 3 Inject Rate (ul/h)", "Units"=4.0, "Pump #"=3.0, "Pump Parameters In"=w1438, "VISA resource name"=w1437) -> ("Pump Parameters Out"=w1430:T32)  [unwired: 3 in]
                    n891 = Bundle By Name(cluster=w1431, "Pump 3"=w1430) -> (w1429:T5)
                    n892 = local write "All Pump Parameters"(w1429) -> ()
                  }
                  frame #1 {
                    n893 = Wait (ms)(milliseconds to wait=w1439) -> ()  [unwired: 1 out]
                  }
                  frame #2 {
                    n894 = call "Write to pump.vi"("string"="start", "VISA resource name"=w1440) -> ()  [unwired: 1 out]
                  }
                  frame #3 {
                    n895 = Wait (ms)(milliseconds to wait=u32 500) -> ()  [unwired: 1 out]
                  }
                  frame #4 {
                    n896 = call "Write to pump.vi"("string"="start", "VISA resource name"=w1444) -> ()  [unwired: 1 out]
                  }
                }
              }
            }
          }
          frame Enabled {
            n897 = call "hamilton_controller.vi"("Open?"=w1446, "valve"=enum16{"A", "B", "C", "D", "ALL"}."A", "action"=T20."MOVE VALVE") -> ()  [unwired: 8 in, 1 out]
          }
        }
      }
      event "Inject Valve B": Value Change {
        n898 = event-data() -> ()  [unwired: 7 out]
        n899 = disable-structure shown="Enabled" {
          disable-tunnel: "Inject Valve B" -> [w1450 w1470]
          frame Disabled {
            n900 = local read "Pump write delay (ms)"() -> (w1452:dbl)
            n901 = flat-sequence {
              tunnel: w1451 -> [w1465]
              tunnel: w1452 -> [w1461]
              tunnel: w1450 -> [_]
              tunnel: w1452 -> [w1467]
              tunnel: w1451 -> [w1468]
              frame #0 {
                n902 = local read "All Pump Parameters"() -> (w1460:T5)
                n903 = Multiply(x=60.0, y="Flush Center Ch Rate (ul/m)") -> (x*y=w1457:dbl)
                n904 = Unbundle By Name(w1460) -> ("Pump 2"=w1466:T32)
                n905 = call "Set pump parameters.vi"("Pump write delay (ms)"=w1461, "Volume (uL)"="Flush Center Ch Volume (uL)", "Rate (uL/h)"=w1457, "Units"=3.0, "Pump #"=2.0, "Pump Parameters In"=w1466, "VISA resource name"=w1465) -> ("Pump Parameters Out"=w1459:T32)  [unwired: 3 in]
                n906 = Bundle By Name(cluster=w1460, "Pump 2"=w1459) -> (w1458:T5)
                n907 = local write "All Pump Parameters"(w1458) -> ()
                n908 = Add(x="Flush Center Ch Volume (uL)", y="Total Volume\nFlushed (uL)") -> (x+y=w1454:dbl)
                n909 = local write "Total Volume\nFlushed (uL)"(w1454) -> ()
              }
              frame #1 {
                n910 = Wait (ms)(milliseconds to wait=w1467) -> ()  [unwired: 1 out]
              }
              frame #2 {
                n911 = call "Write to pump.vi"("string"="start", "VISA resource name"=w1468) -> ()  [unwired: 1 out]
              }
            }
            n912 = local read "Chemyx Syringe Pump Serial Port"() -> (w1451:refnum<visa-resource-name>)
          }
          frame Enabled {
            n913 = call "hamilton_controller.vi"("Open?"=w1470, "valve"=enum16{"A", "B", "C", "D", "ALL"}."B", "action"=T20."MOVE VALVE") -> ()  [unwired: 8 in, 1 out]
          }
        }
      }
      event "Sample Channel Flow": Value Change {
        n914 = event-data() -> ()  [unwired: 7 out]
        n915 = call "hamilton_controller.vi"("Open?"="Sample Channel Flow", "valve"=enum16{"A", "B", "C", "D", "ALL"}."C", "action"=T20."MOVE VALVE") -> ()  [unwired: 8 in, 1 out]
      }
      event "Flip Green Filter": Value Change {
        n916 = event-data() -> ()  [unwired: 7 out]
        n917 = Not(x="Flip Green Filter") -> (.not. x?=w1476:bool)
        n918 = local write "Flip Green Filter"(w1476) -> ()
        n919 = flat-sequence {
          tunnel: w1484 -> [w1489]
          tunnel: w1483 -> [w1488]
          tunnel: [w1486] -> w1481
          tunnel: [w1485] -> w1480
          tunnel: [w1491] -> w1479
          tunnel: w1481 -> [w1491]
          tunnel: [w1490] -> w1478
          tunnel: w1480 -> [w1490]
          tunnel: w1479 -> [w1495]
          tunnel: w1478 -> [w1494]
          tunnel: [w1493] -> w1482
          frame #0 {
            n920 = xnode "Read/Write Control"("FPGA VI Reference In"=w1489, "error in"=w1488, "Green Filter Flipper"=TRUE) -> ("FPGA VI Reference Out"=w1486:T19, "error out"=w1485:errorcluster)
          }
          frame #1 {
            n921 = Wait (ms)(milliseconds to wait=u32 100) -> ()  [unwired: 1 out]
          }
          frame #2 {
            n922 = xnode "Read/Write Control"("FPGA VI Reference In"=w1495, "error in"=w1494, "Green Filter Flipper"=FALSE) -> ("error out"=w1493:errorcluster)  [unwired: 1 out]
          }
        }
      }
      event "Pump 1 contents", "Pump 3 contents": Value Change {
        n923 = event-data() -> ()  [unwired: 7 out]
        n924 = local read "Pump 1 contents"() -> (→"Pump 1 cont disp":string)
        n925 = local read "Pump 3 contents"() -> (→"Pump 3 cont disp":string)
      }
      event "Reset Trap Pos. FB": Value Change {
        n926 = event-data() -> ()  [unwired: 7 out]
        n927 = xnode "Read/Write Control"("FPGA VI Reference In"=w1501, "error in"=w1500, "Trap Pos. FB Reset"="Reset Trap Pos. FB") -> ()  [unwired: 2 out]
      }
      event "Trap Pos. FB ON": Value Change {
        n928 = event-data() -> ()  [unwired: 7 out]
        n929 = xnode "Read/Write Control"("FPGA VI Reference In"=w1504, "error in"=w1503, "Force feedback"="Trap Pos. FB ON") -> ()  [unwired: 2 out]
      }
      event "Trap Pos. FB Range", "Trap Pos. FB Gains", "Trap Pos. FB Mult Factor", "Trap Pos. FB Offset Factor", "Trap Pos FB Negate Action", "Trap Pos FB Monitor\nT1 or T2": Value Change {
        n930 = event-data() -> ()  [unwired: 7 out]
        n931 = xnode "Read/Write Control"("FPGA VI Reference In"=w1513, "error in"=w1512, "Trap Pos. FB Range"="Trap Pos. FB Range", "Trap Pos. FB Gains"="Trap Pos. FB Gains", "Trap Pos. FB Mult Factor"="Trap Pos. FB Mult Factor", "Trap Pos. FB Offset Factor"="Trap Pos. FB Offset Factor", "Trap Pos FB Negate Action"="Trap Pos FB Negate Action", "Trap Pos FB Monitor T1 or T2"="Trap Pos FB Monitor\nT1 or T2", "AI1 X Scale"="Trap Pos. AI1 X Pre-scale") -> ()  [unwired: 2 out]
      }
      event "Trap Pos FB SP": Value Change {
        n932 = event-data() -> ()  [unwired: 7 out]
        n933 = xnode "Read/Write Control"("FPGA VI Reference In"=w1516, "error in"=w1515, "Trap Pos. FB SP"="Trap Pos FB SP") -> ()  [unwired: 2 out]
      }
      event "Set SP to Reading": Value Change {
        n934 = event-data() -> ()  [unwired: 7 out]
        n935 = local read "Trap Pos FB Monitor\nT1 or T2"() -> (w1524:bool)
        n936 = local read "Trap X AI1 (DMA)"() -> (w1527:T13)
        n937 = local read "Trap X (AI1)"() -> (w1530:T10)
        n938 = Unbundle By Name(w1530) -> ("Trap 1"=w1529:fxp<+/-,16,1>, "Trap 2"=w1528:fxp<+/-,16,1>)
        n939 = Unbundle By Name(w1527) -> ("Set 1"=w1526:fxp<+/-,16,1>, "Set 2"=w1525:fxp<+/-,16,1>)
        n940 = Select(t=w1529, s=w1524, f=w1528) -> (s? t:f=w1523:fxp<+/-,16,1>)
        n941 = Select(t=w1526, s=w1524, f=w1525) -> (s? t:f=w1522:fxp<+/-,16,1>)
        n942 = Not(x="Set SP Using...") -> (.not. x?=w1517:bool)
        n943 = Select(t=w1523, s=w1517, f=w1522) -> (s? t:f=w1518:fxp<+/-,16,1>)
        n944 = xnode "Read/Write Control"("FPGA VI Reference In"=w1520, "error in"=w1519, "Trap Pos. FB SP"=w1518) -> ()  [unwired: 2 out]
        n945 = local write "Trap Pos FB SP"(w1518) -> ()
      }
      event "Trap Pos. FB Out Scale 2^n": Value Change {
        n946 = event-data() -> ()  [unwired: 7 out]
        n947 = Scale By Power Of 2(n="Trap Pos. FB Out Scale 2^n", x=ext 1.0) -> (x*2^n=w1532:ext)
        n948 = property on="Trap Pos. FB Mult Factor" class="DigNum (strict)"("Val(Sgnl)"=w1532) -> ()  [unwired: 2 in, 2 out]
      }
      event "Trap Pos FB Int Count": Value Change {
        n949 = event-data() -> ()  [unwired: 7 out]
        n950 = xnode "Read/Write Control"("FPGA VI Reference In"=w1537, "error in"=w1536, "Trap Pos FB Int Count"="Trap Pos FB Int Count") -> ()  [unwired: 2 out]
      }
    }
    "error out 2" <- w720
    n951 = node-c288() -> ()  [unwired: 1 in, 1 out]
  }
  n952 = timed-loop "Run Scripts, including: stage motion" {
    timing: w69 -> [_]
    timing-out: [_] -> w68
    tunnel: w24 -> [_]
    stop <- w1539 stop-if-true
    n953 = node-c288() -> ()  [unwired: 1 in, 1 out]
    n954 = event shown="[8] \"Take Stepping Data\": Value Change" {
      selector: _ -> [_ _ _ _ _ _ _ _ _ _ _ _]
      dyn-events: _ -> [_ _ _ _ _ _ _ _ _ _ _ _]
      timeout: 50 -> [_ _ _ _ _ _ _ _ _ _ _ _]
      tunnel: ["Move Cap. 1 (DNA Top)" _ "Cal/Data Acq. Spot" "Dump Beads" "Dip for Protein" _ "Got ADig bead" "Got DNA bead" "Take Stepping Data" _ "Take Detection Laser\nImage" _] -> _
      tunnel: [_ _ _ _ _ _ _ _ _ _ _ w1747] -> w1539
      event "Move Cap. 1 (DNA Top)": Value Change {
        n955 = event-data() -> ()  [unwired: 1 in, 5 out]
        n956 = local write "Move Cap. 1 (DNA Top)"(FALSE ("Move Cap. 1 (DNA Right)")) -> ()
        n957 = flat-sequence {
          tunnel: "Cap 1 Samp Flow ON" -> [w1545]
          frame #0 {
            n958 = local write "Stage Moving"(FALSE ("Stage Moving")) -> ()
            n959 = case "stop flow" shown="True" w1545 {
              frame False {
              }
              frame True {
                n960 = call "hamilton_controller.vi"("Open?"=FALSE, "valve"=enum16{"A", "B", "C", "D", "ALL"}."C", "action"=T20."MOVE VALVE") -> ()  [unwired: 8 in, 1 out]
              }
            }
            n961 = case shown="True" TRUE {
              tunnel: "Cap 1 T ON" -> [w1554 w1555]
              frame False {
                n962 = property on="Trap 1 (ON/OFF)" class="Bool (strict)"("Val(Sgnl)"=w1554) -> ()  [unwired: 2 in, 2 out]
              }
              frame True {
                n963 = property on="Trap 2 (ON/OFF)" class="Bool (strict)"("Val(Sgnl)"=w1555) -> ()  [unwired: 2 in, 2 out]
              }
            }
            n964 = call <vilib>:"Beep.vi"() -> ()  [unwired: 3 in, 9 out]
            n965 = case shown="True" "Cap 1 Flow ON" {
              frame False {
              }
              frame True {
                n966 = property on="Inject Top" class="Bool (strict)"("Val(Sgnl)"=TRUE ("Value (Signaling)")) -> ()  [unwired: 2 in, 2 out]
              }
            }
          }
        }
      }
      event Timeout {
        n967 = event-data() -> ()  [unwired: 1 in, 2 out]
      }
      event "Cal/Data Acq. Spot": Value Change {
        # "wait for calibration file\nto be written"
        # "signal save cal true\nthis tells the data \nacquisition loop to\nstart sending the data\nto a calibration file"
        # "separate traps to\nthe desired trap delta"
        # "move stage to data acquisition spot"
        # "CHANGE FISH FOR TETHER BACK\nTO TRUE VALUE HERE."
        n968 = event-data() -> ()  [unwired: 1 in, 5 out]
        n969 = local write "Cal/Data Acq. Spot"(FALSE ("Cal/Data Acq. Spot")) -> ()
        n970 = flat-sequence {
          tunnel: ["Cal @ (MHz)"] -> w1556
          tunnel: w1556 -> [w1566]
          tunnel: w1556 -> [w1587]
          frame #0 {
            n971 = property on="Trap Delta (MHz)" class="DigNum (strict)"("Val(Sgnl)"="Cal @ (MHz)") -> ()  [unwired: 2 in, 2 out]
            n972 = call <vilib>:"Beep.vi"() -> ()  [unwired: 3 in, 9 out]
          }
          frame #1 {
            n973 = Wait (ms)(milliseconds to wait=u32 100) -> ()  [unwired: 1 out]
          }
          frame #2 {
            n974 = property on="Save Calibration" class="Bool (strict)"("Val(Sgnl)"=TRUE ("Value (Signaling)")) -> ()  [unwired: 2 in, 2 out]
          }
          frame #3 {
            n975 = Wait (ms)(milliseconds to wait=u32 4000) -> ()  [unwired: 1 out]
          }
          frame #4 {
            n976 = while {
              stop <- w1563 stop-if-true
              n977 = local read "Saving..."() -> (w1564:bool)
              n978 = Wait (ms)(milliseconds to wait=u32 100) -> ()  [unwired: 1 out]
              n979 = Not(x=w1564) -> (.not. x?=w1563:bool)
            }
          }
          frame #5 {
            n980 = case shown="True" "W/ Offset 1" {
              tunnel: w1566 -> [_ w1568]
              frame False {
              }
              frame True {
                n981 = stacked-sequence {
                  tunnel: w1568 -> [_ _ _ _ _ _ _ w1585]
                  frame #0 {
                    n982 = Replace Array Subset(array=u32[] [0] ("Index Values"), new element="Offset 1 Set", index=0) -> (w1569:u32[])
                    n983 = property on="Saved AOD Raster Scan Parameter Sets" class="Arr (strict)"("Index Values"=w1569) -> ()  [unwired: 2 in, 2 out]
                    n984 = property on="Trap Delta (MHz)" class="DigNum (strict)"("Val(Sgnl)"="Offset 1 Start (MHz)") -> ()  [unwired: 2 in, 2 out]
                  }
                  frame #1 {
                    n985 = Wait (ms)(milliseconds to wait=u32 200) -> ()  [unwired: 1 out]
                  }
                  frame #2 {
                    n986 = property on="Load parameters" class="Bool (strict)"("Val(Sgnl)"=TRUE ("Value (Signaling)")) -> ()  [unwired: 2 in, 2 out]
                  }
                  frame #3 {
                    n987 = Wait (ms)(milliseconds to wait=u32 200) -> ()  [unwired: 1 out]
                  }
                  frame #4 {
                    n988 = property on="Trap Raster Scan" class="Bool (strict)"("Val(Sgnl)"=TRUE ("Value (Signaling)")) -> ()  [unwired: 2 in, 2 out]
                  }
                  frame #5 {
                    n989 = Wait (ms)(milliseconds to wait=u32 2000) -> ()  [unwired: 1 out]
                  }
                  frame #6 {
                    n990 = while {
                      stop <- w1582 stop-if-true
                      n991 = local read "Raster Scanning..."() -> (w1584:bool)
                      n992 = local read "Saving..."() -> (w1580:bool)
                      n993 = Wait (ms)(milliseconds to wait=u32 100) -> ()  [unwired: 1 out]
                      n994 = Not(x=w1580) -> (.not. x?=w1579:bool)
                      n995 = Not(x=w1584) -> (.not. x?=w1581:bool)
                      n996 = And(x=w1581, y=w1579) -> (x .and. y?=w1582:bool)
                    }
                  }
                  frame #7 {
                    n997 = property on="Trap Delta (MHz)" class="DigNum (strict)"("Val(Sgnl)"=w1585) -> ()  [unwired: 2 in, 2 out]
                  }
                }
              }
            }
          }
          frame #6 {
            n998 = local read "Save ave N"() -> (w1586:dbl)
            n999 = case shown="True" "W/ Offset 2" {
              tunnel: w1587 -> [_ w1593]
              tunnel: w1586 -> [_ w1592]
              frame False {
                n1000 = Multiply(x="Cal read wait (s)", y=u32 1000 ("milliseconds to wait")) -> (x*y=w1590:u32)
                n1001 = Wait (ms)(milliseconds to wait=w1590) -> ()  [unwired: 1 out]
              }
              frame True {
                n1002 = stacked-sequence {
                  tunnel: w1593 -> [_ _ _ _ _ _ _ _ _ w1614 _ _]
                  tunnel: w1592 -> [_ _ _ _ _ _ _ _ _ w1612 _ _]
                  frame #0 {
                    n1003 = property on="Save ave N" class="DigNum (strict)"("Val(Sgnl)"=1.0 ("Value (Signaling)")) -> ()  [unwired: 2 in, 2 out]
                  }
                  frame #1 {
                    n1004 = Wait (ms)(milliseconds to wait=u32 500) -> ()  [unwired: 1 out]
                  }
                  frame #2 {
                    n1005 = property on="Trap Delta (MHz)" class="DigNum (strict)"("Val(Sgnl)"="Offset 2 Start (MHz)") -> ()  [unwired: 2 in, 2 out]
                    n1006 = Replace Array Subset(array=u32[] [0] ("Index Values"), new element="Offset 2 Set", index=0) -> (w1598:u32[])
                    n1007 = property on="Saved AOD Raster Scan Parameter Sets" class="Arr (strict)"("Index Values"=w1598) -> ()  [unwired: 2 in, 2 out]
                  }
                  frame #3 {
                    n1008 = Wait (ms)(milliseconds to wait=u32 500) -> ()  [unwired: 1 out]
                  }
                  frame #4 {
                    n1009 = property on="Load parameters" class="Bool (strict)"("Val(Sgnl)"=TRUE ("Value (Signaling)")) -> ()  [unwired: 2 in, 2 out]
                  }
                  frame #5 {
                    n1010 = Wait (ms)(milliseconds to wait=u32 500) -> ()  [unwired: 1 out]
                  }
                  frame #6 {
                    n1011 = property on="Trap Raster Scan" class="Bool (strict)"("Val(Sgnl)"=TRUE ("Value (Signaling)")) -> ()  [unwired: 2 in, 2 out]
                  }
                  frame #7 {
                    n1012 = Wait (ms)(milliseconds to wait=u32 2000) -> ()  [unwired: 1 out]
                  }
                  frame #8 {
                    n1013 = while {
                      stop <- w1607 stop-if-true
                      n1014 = local read "Raster Scanning..."() -> (w1610:bool)
                      n1015 = local read "Saving..."() -> (w1608:bool)
                      n1016 = Wait (ms)(milliseconds to wait=u32 100) -> ()  [unwired: 1 out]
                      n1017 = Not(x=w1608) -> (.not. x?=w1606:bool)
                      n1018 = Not(x=w1610) -> (.not. x?=w1609:bool)
                      n1019 = And(x=w1609, y=w1606) -> (x .and. y?=w1607:bool)
                    }
                  }
                  frame #9 {
                    n1020 = property on="Trap Delta (MHz)" class="DigNum (strict)"("Val(Sgnl)"=w1614) -> ()  [unwired: 2 in, 2 out]
                    n1021 = property on="Saved AOD Raster Scan Parameter Sets" class="Arr (strict)"("Index Values"=u32[] [0]) -> ()  [unwired: 2 in, 2 out]
                    n1022 = property on="Save ave N" class="DigNum (strict)"("Val(Sgnl)"=w1612) -> ()  [unwired: 2 in, 2 out]
                  }
                  frame #10 {
                    n1023 = Wait (ms)(milliseconds to wait=u32 500) -> ()  [unwired: 1 out]
                  }
                  frame #11 {
                    n1024 = property on="Load parameters" class="Bool (strict)"("Val(Sgnl)"=TRUE ("Value (Signaling)")) -> ()  [unwired: 2 in, 2 out]
                  }
                }
              }
            }
          }
          frame #7 {
            n1025 = property on="Read Cal" class="Bool (strict)"("Val(Sgnl)"=TRUE ("Value (Signaling)")) -> ()  [unwired: 2 in, 2 out]
          }
          frame #8 {
            n1026 = Wait (ms)(milliseconds to wait=u32 500) -> ()  [unwired: 1 out]
          }
          frame #9 {
            n1027 = property on="Fish for Tether" class="Bool (strict)"("Val(Sgnl)"=FALSE ("Value (Signaling)")) -> ()  [unwired: 2 in, 2 out]
          }
        }
      }
      event "Dump Beads": Value Change {
        # "SCRIPT TO REMOVE BOTH BEADS FROM THE TRAPS. TURNS ON LIGHT WHICH INDICATES THAT STAGE IS MOVING. THEN STOPS SAVING DATA. \nSETS Sample Channel Flow TO TRUE. STOPS INTERLACING GREEN FLUORESCENCE. TURNS OFF Tether INDICATOR BECAUSE WE ARE THROWING IT\nAWAY. SHUTS OFF TRAP POSITION FEEDBACK."
        n1028 = event-data() -> ()  [unwired: 1 in, 5 out]
        n1029 = flat-sequence {
          frame #0 {
            w1621 = FALSE ("Fl. Triggered...")
            w1622 = TRUE ("Stage Moving")
            n1030 = local read "Saving..."() -> (w1623:bool)
            n1031 = local write "Fl. Triggered..."(w1621) -> ()
            n1032 = local write "Stage Moving"(w1622) -> ()
            n1033 = local write "Tether"(w1621) -> ()
            n1034 = property on="Green Laser ON/Interlacing" class="Bool (strict)"("Val(Sgnl)"=w1621) -> ()  [unwired: 2 in, 2 out]
            n1035 = property on="Trap Pos. FB ON" class="Bool (strict)"("Val(Sgnl)"=w1621) -> ()  [unwired: 2 in, 2 out]
            n1036 = property on="Sample Channel Flow" class="Bool (strict)"("Val(Sgnl)"=w1622) -> ()  [unwired: 2 in, 2 out]
            n1037 = local write "Stop Saving"(w1623) -> ()
          }
          frame #1 {
            w1624 = FALSE ("Value (Signaling)")
            # "TURNS TRAPS OFF SO THAT\nBEADS REMAIN AT DUMP \nBEADS POSITION"
            n1038 = property on="Trap 1 (ON/OFF)" class="Bool (strict)"("Val(Sgnl)"=w1624) -> ()  [unwired: 2 in, 2 out]
            n1039 = property on="Trap 2 (ON/OFF)" class="Bool (strict)"("Val(Sgnl)"=w1624) -> ()  [unwired: 2 in, 2 out]
            n1040 = call <vilib>:"Beep.vi"() -> ()  [unwired: 3 in, 9 out]
          }
          frame #2 {
            n1041 = property on="Goto Bottom (F7)" class="Bool (strict)"("Val(Sgnl)"=TRUE ("Value (Signaling)")) -> ()  [unwired: 2 in, 2 out]
          }
          frame #3 {
            n1042 = Wait (ms)(milliseconds to wait=u32 8000) -> ()  [unwired: 1 out]
          }
          frame #4 {
            n1043 = property on="Trap Delta (MHz)" class="DigNum (strict)"("Val(Sgnl)"=20.0 ("Value (Signaling)")) -> ()  [unwired: 2 in, 2 out]
          }
          frame #5 {
            n1044 = property on="Trap 2 (ON/OFF)" class="Bool (strict)"("Val(Sgnl)"=TRUE ("Value (Signaling)")) -> ()  [unwired: 2 in, 2 out]
          }
          frame #6 {
            n1045 = property on="Sample Channel Flow" class="Bool (strict)"("Val(Sgnl)"=FALSE ("Value (Signaling)")) -> ()  [unwired: 2 in, 2 out]
          }
        }
      }
      event "Dip for Protein": Value Change {
        n1046 = event-data() -> ()  [unwired: 1 in, 5 out]
        n1047 = flat-sequence {
          frame #0 {
            n1048 = case shown="True" "Move Trap Before?" {
              frame False {
              }
              frame True {
                n1049 = property on="Trap Delta (MHz)" class="DigNum (strict)"("Val(Sgnl)"="Dip Trap Delta 1 (MHz)") -> ()  [unwired: 2 in, 2 out]
              }
            }
          }
          frame #1 {
            n1050 = Multiply(x="Duration (s)", y=1000.0) -> (x*y=w1633:dbl)
            n1051 = Wait (ms)(milliseconds to wait=w1633) -> ()  [unwired: 1 out]
          }
          frame #2 {
            n1052 = case shown="True" "Move Trap After?" {
              frame False {
              }
              frame True {
                n1053 = property on="Trap Delta (MHz)" class="DigNum (strict)"("Val(Sgnl)"="Dip Trap Delta 2 (MHz)") -> ()  [unwired: 2 in, 2 out]
              }
            }
          }
          frame #3 {
            n1054 = case shown="True" "Green ON After?" {
              frame False {
              }
              frame True {
                n1055 = property on="Green Laser ON/Interlacing" class="Bool (strict)"("Val(Sgnl)"=TRUE ("Value (Signaling)")) -> ()  [unwired: 2 in, 2 out]
              }
            }
          }
          frame #4 {
            n1056 = Wait (ms)(milliseconds to wait=u32 500) -> ()  [unwired: 1 out]
          }
          frame #5 {
            n1057 = case shown="True" "Save Data After?" {
              frame False {
              }
              frame True {
                n1058 = property on="Start Saving" class="Bool (strict)"("Val(Sgnl)"=TRUE ("Value (Signaling)")) -> ()  [unwired: 2 in, 2 out]
              }
            }
          }
        }
      }
      event "Profile": Value Change {
        n1059 = event-data() -> ()  [unwired: 1 in, 5 out]
        n1060 = flat-sequence {
          frame #0 {
            w1643 = 0.0 ("element")
            n1061 = Build Array(w1643, "Y change (mm)", w1643) -> ()  [unwired: 1 out]
          }
          frame #1 {
            # "stop saving"
            n1062 = local write "Stop Saving"(TRUE ("Stop Saving")) -> ()
            n1063 = local write "Stage Moving"(FALSE ("Stage Moving")) -> ()
          }
        }
      }
      event "Got ADig bead": Value Change {
        n1064 = event-data() -> ()  [unwired: 1 in, 5 out]
        n1065 = property on="Move Cap. 1 (DNA Top)" class="Bool (strict)"("Val(Sgnl)"=TRUE ("Value (Signaling)")) -> ()  [unwired: 2 in, 2 out]
        n1066 = property on="Inject Bottom" class="Bool (strict)"("Val(Sgnl)"=FALSE ("Value (Signaling)")) -> ()  [unwired: 2 in, 2 out]
      }
      event "Got DNA bead": Value Change {
        n1067 = event-data() -> ()  [unwired: 1 in, 5 out]
        n1068 = property on="Cal/Data Acq. Spot" class="Bool (strict)"("Val(Sgnl)"=TRUE ("Value (Signaling)")) -> ()  [unwired: 2 in, 2 out]
        n1069 = property on="Inject Top" class="Bool (strict)"("Val(Sgnl)"=FALSE ("Value (Signaling)")) -> ()  [unwired: 2 in, 2 out]
      }
      event "Take Stepping Data": Value Change {
        n1070 = event-data() -> ()  [unwired: 1 in, 5 out]
        n1071 = local read "Save ave N"() -> (w1661:dbl)
        n1072 = flat-sequence {
          tunnel: w1661 -> [w1663]
          tunnel: [w1663] -> w1656
          tunnel: [w1665] -> w1657
          tunnel: w1656 -> [w1665]
          tunnel: [w1667] -> w1658
          tunnel: w1657 -> [w1667]
          tunnel: [w1670] -> w1659
          tunnel: w1658 -> [w1670]
          tunnel: [w1672] -> w1660
          tunnel: w1659 -> [w1672]
          tunnel: [w1674] -> w1654
          tunnel: w1660 -> [w1674]
          tunnel: w1654 -> [w1677]
          tunnel: [w1677] -> w1653
          tunnel: w1653 -> [w1678]
          tunnel: [w1678] -> w1655
          tunnel: w1655 -> [w1684]
          frame #0 {
            n1073 = property on="Save ave N" class="DigNum (strict)"("Val(Sgnl)"="Save ave factor") -> ()  [unwired: 2 in, 2 out]
          }
          frame #1 {
            n1074 = Wait (ms)(milliseconds to wait=u32 100) -> ()  [unwired: 1 out]
          }
          frame #2 {
            n1075 = local read "Offset 2 Start (MHz)"() -> (w1669:dbl)
            n1076 = property on="Saved AOD Raster Scan Parameter Sets" class="Arr (strict)"("Index Values"=u32[] [2]) -> ()  [unwired: 2 in, 2 out]
            n1077 = property on="Trap Delta (MHz)" class="DigNum (strict)"("Val(Sgnl)"=w1669) -> ()  [unwired: 2 in, 2 out]
          }
          frame #3 {
            n1078 = property on="Load parameters" class="Bool (strict)"("Val(Sgnl)"=TRUE ("Value (Signaling)")) -> ()  [unwired: 2 in, 2 out]
          }
          frame #4 {
            n1079 = Wait (ms)(milliseconds to wait=u32 100) -> ()  [unwired: 1 out]
          }
          frame #5 {
            n1080 = property on="Trap Raster Scan" class="Bool (strict)"("Val(Sgnl)"=TRUE ("Value (Signaling)")) -> ()  [unwired: 2 in, 2 out]
          }
          frame #6 {
            n1081 = Wait (ms)(milliseconds to wait=u32 1000) -> ()  [unwired: 1 out]
          }
          frame #7 {
            n1082 = while {
              stop <- w1681 stop-if-true
              n1083 = local read "Raster Scanning..."() -> (w1683:bool)
              n1084 = local read "Saving..."() -> (w1682:bool)
              n1085 = Not(x=w1682) -> (.not. x?=w1679:bool)
              n1086 = Not(x=w1683) -> (.not. x?=w1680:bool)
              n1087 = And(x=w1680, y=w1679) -> (x .and. y?=w1681:bool)
            }
          }
          frame #8 {
            n1088 = property on="Save ave N" class="DigNum (strict)"("Val(Sgnl)"=w1684) -> ()  [unwired: 2 in, 2 out]
          }
        }
      }
      event "Step Size (nm)": Value Change {
        n1089 = event-data() -> ()  [unwired: 1 in, 5 out]
        n1090 = flat-sequence {
          frame #0 {
            n1091 = property on="Saved AOD Raster Scan Parameter Sets" class="Arr (strict)"("Index Values"=u32[] [1]) -> ()  [unwired: 2 in, 2 out]
          }
          frame #1 {
            n1092 = Multiply(x="N Steps", y="Step Size (nm)") -> (x*y=w1686:dbl)
            n1093 = property on="Scan Speed AOD (nm/s) 2" class="DigNum (strict)"("Value"="Step Size (nm)") -> ()  [unwired: 2 in, 2 out]
            n1094 = property on="Step Size AOD (nm) 2" class="DigNum (strict)"("Value"="Step Size (nm)") -> ()  [unwired: 2 in, 2 out]
            n1095 = property on="Scan Range AOD (nm) 2" class="DigNum (strict)"("Value"=w1686) -> ()  [unwired: 2 in, 2 out]
          }
        }
      }
      event "Take Detection Laser\nImage": Value Change {
        n1096 = event-data() -> ()  [unwired: 1 in, 5 out]
        n1097 = flat-sequence {
          tunnel: [w1714] -> w1704
          tunnel: [w1713] -> w1697
          tunnel: [w1712] -> w1689
          tunnel: [w1717] -> w1705
          tunnel: w1704 -> [w1717]
          tunnel: [w1716] -> w1698
          tunnel: w1697 -> [w1716]
          tunnel: [w1715] -> w1690
          tunnel: w1689 -> [w1715]
          tunnel: [w1721] -> w1706
          tunnel: w1705 -> [w1721]
          tunnel: [w1720] -> w1699
          tunnel: w1698 -> [w1720]
          tunnel: [w1719] -> w1691
          tunnel: w1690 -> [w1719]
          tunnel: [w1727] -> w1707
          tunnel: w1706 -> [w1727]
          tunnel: [w1726] -> w1700
          tunnel: w1699 -> [w1726]
          tunnel: [w1725] -> w1692
          tunnel: w1691 -> [w1725]
          tunnel: [w1731] -> w1708
          tunnel: w1707 -> [w1731]
          tunnel: [w1730] -> w1701
          tunnel: w1700 -> [w1730]
          tunnel: [w1729] -> w1693
          tunnel: w1692 -> [w1729]
          tunnel: [w1735] -> w1709
          tunnel: w1708 -> [w1735]
          tunnel: [w1734] -> w1702
          tunnel: w1701 -> [w1734]
          tunnel: [w1733] -> w1694
          tunnel: w1693 -> [w1733]
          tunnel: [w1739] -> w1710
          tunnel: w1709 -> [w1739]
          tunnel: [w1738] -> w1703
          tunnel: w1702 -> [w1738]
          tunnel: [w1737] -> w1695
          tunnel: w1694 -> [w1737]
          tunnel: w1710 -> [w1745]
          tunnel: w1703 -> [w1744]
          tunnel: [w1742] -> w1696
          tunnel: w1695 -> [w1742]
          tunnel: w1696 -> [w1746]
          frame #0 {
            n1098 = local read "Green Laser ON/Interlacing"() -> (w1714:bool)
            n1099 = local read "Green laser mode"() -> (w1713:enum32{"Laser ON", "Laser OFF", "Interlace"})
            n1100 = local read "Green FB On/Off"() -> (w1712:bool)
          }
          frame #1 {
            n1101 = property on="Green FB On/Off" class="Bool (strict)"("Val(Sgnl)"=FALSE ("Value (Signaling)")) -> ()  [unwired: 2 in, 2 out]
          }
          frame #2 {
            n1102 = property on="Green Laser ON/Interlacing" class="Bool (strict)"("Val(Sgnl)"=TRUE ("Value (Signaling)")) -> ()  [unwired: 2 in, 2 out]
            n1103 = property on="Flip Green Filter" class="Bool (strict)"("Val(Sgnl)"=TRUE ("Value (Signaling)")) -> ()  [unwired: 2 in, 2 out]
            n1104 = property on="Green laser mode" class="RadioBtnsControl (strict)"("Val(Sgnl)"=enum32{"Laser ON", "Laser OFF", "Interlace"}."Laser ON" ("Value (Signaling)")) -> ()  [unwired: 2 in, 2 out]
          }
          frame #3 {
            n1105 = Wait (ms)(milliseconds to wait=u32 500) -> ()  [unwired: 1 out]
          }
          frame #4 {
            n1106 = property on="Confocal Image" class="Bool (strict)"("Val(Sgnl)"=TRUE ("Value (Signaling)")) -> ()  [unwired: 2 in, 2 out]
          }
          frame #5 {
            n1107 = Wait (ms)(milliseconds to wait=u32 2000) -> ()  [unwired: 1 out]
          }
          frame #6 {
            n1108 = while {
              stop <- w1740 stop-if-true
              n1109 = local read "Saving..."() -> (w1741:bool)
              n1110 = Not(x=w1741) -> (.not. x?=w1740:bool)
            }
          }
          frame #7 {
            n1111 = property on="Flip Green Filter" class="Bool (strict)"("Val(Sgnl)"=TRUE ("Value (Signaling)")) -> ()  [unwired: 2 in, 2 out]
            n1112 = property on="Green Laser ON/Interlacing" class="Bool (strict)"("Val(Sgnl)"=w1745) -> ()  [unwired: 2 in, 2 out]
            n1113 = property on="Green laser mode" class="RadioBtnsControl (strict)"("Val(Sgnl)"=w1744) -> ()  [unwired: 2 in, 2 out]
          }
          frame #8 {
            n1114 = property on="Green FB On/Off" class="Bool (strict)"("Val(Sgnl)"=w1746) -> ()  [unwired: 2 in, 2 out]
          }
        }
      }
      event "Stop All": Value Change {
        n1115 = event-data() -> ()  [unwired: 1 in, 5 out]
        n1116 = local read "Stop All"() -> (w1747:bool)
      }
    }
    n1117 = node-c288() -> ()  [unwired: 1 in, 1 out]
  }
  n1118 = node-c288() -> (w76:T24)  [unwired: 4 out]
  n1119 = timed-loop "Mouse control: trap position (AOM deflection), set confocal spot from image" {
    tunnel: [w1749] -> w34
    tunnel: w24 -> [w1748]
    timing: w76 -> [_]
    timing-out: [_] -> w75
    stop <- w1749 stop-if-true
    n1120 = node-c288() -> ()  [unwired: 2 out]
    n1121 = event shown="[0] \"Pane\": Mouse Down" {
      selector: _ -> [_ _]
      dyn-events: _ -> [_ _]
      timeout: _ -> [_ _]
      tunnel: w1748 -> [w1752 _]
      event Mouse Down {
        n1122 = event-data() -> ("Time"=w1754:u32, "Coords"=w1753:T7, "Button"=w1755:u16)  [unwired: 6 out]
        n1123 = case shown="1" w1755 {
          tunnel: w1754 -> [_ _ w1858]
          tunnel: w1753 -> [_ w1792 w1856]
          tunnel: w1752 -> [_ _ w1854]
          frame 0, Default {
          }
          frame 1 {
            n1124 = property on="APD 2" class="ImageControl"() -> ("Displayed Image Position"=w1762:cluster{"Left":i32, "Top":i32})  [unwired: 2 in, 2 out]
            n1125 = property on="APD 1" class="ImageControl"() -> ("Displayed Image Position"=w1791:cluster{"Left":i32, "Top":i32})  [unwired: 2 in, 2 out]
            n1126 = property on="Detection Laser X" class="ImageControl"() -> ("Displayed Image Position"=w1788:cluster{"Left":i32, "Top":i32})  [unwired: 2 in, 2 out]
            n1127 = property on="Detection Laser Y" class="ImageControl"() -> ("Displayed Image Position"=w1787:cluster{"Left":i32, "Top":i32})  [unwired: 2 in, 2 out]
            n1128 = property on="APD 2" class="ImageControl"() -> ("Displayed Image Size"=w1761:cluster{"Width":u32, "Height":u32})  [unwired: 2 in, 2 out]
            n1129 = property on="APD 1" class="ImageControl"() -> ("Displayed Image Size"=w1789:cluster{"Width":u32, "Height":u32})  [unwired: 2 in, 2 out]
            n1130 = property on="Detection Laser X" class="ImageControl"() -> ("Displayed Image Size"=w1790:cluster{"Width":u32, "Height":u32})  [unwired: 2 in, 2 out]
            n1131 = property on="Detection Laser Y" class="ImageControl"() -> ("Displayed Image Size"=w1786:cluster{"Width":u32, "Height":u32})  [unwired: 2 in, 2 out]
            n1132 = Unbundle By Name(w1761) -> ("Width"=w1758:u32, "Height"=w1757:u32)
            n1133 = Unbundle By Name(w1762) -> ("Left"=w1760:i32, "Top"=w1759:i32)
            n1134 = Unbundle By Name(w1789) -> ("Width"=w1783:u32, "Height"=w1782:u32)
            n1135 = Unbundle By Name(w1790) -> ("Width"=w1779:u32, "Height"=w1778:u32)
            n1136 = Unbundle By Name(w1786) -> ("Width"=w1775:u32, "Height"=w1774:u32)
            n1137 = Unbundle By Name(w1791) -> ("Left"=w1785:i32, "Top"=w1784:i32)
            n1138 = Unbundle By Name(w1788) -> ("Left"=w1781:i32, "Top"=w1780:i32)
            n1139 = Unbundle By Name(w1787) -> ("Left"=w1777:i32, "Top"=w1776:i32)
            n1140 = Bundle("Left"=w1760, "Top"=w1759, "Width"=w1758, "Height"=w1757) -> (w1756:T33)  [unwired: 1 in]
            n1141 = Bundle("Left"=w1785, "Top"=w1784, "Width"=w1783, "Height"=w1782) -> (w1773:T33)  [unwired: 1 in]
            n1142 = Bundle("Left"=w1781, "Top"=w1780, "Width"=w1779, "Height"=w1778) -> (w1772:T33)  [unwired: 1 in]
            n1143 = Bundle("Left"=w1777, "Top"=w1776, "Width"=w1775, "Height"=w1774) -> (w1771:T33)  [unwired: 1 in]
            n1144 = Build Cluster Array(w1756, w1773, w1772, w1771) -> (w1770:T34)
            n1145 = for {
              tunnel: w1792 -> [w1803]
              tunnel: w1770 -> [w1804] mode=indexing
              shift-right: [w1801] -> w1768
              shift-left: TRUE -> [w1802]
              shift-right: [w1800] -> w1766
              shift-left: _ -> [w1796]
              shift-right: [w1799] -> w1765
              shift-left: _ -> [w1795]
              shift-right: [w1798] -> w1764
              shift-left: _ -> [w1794]
              shift-right: [w1797] -> w1763
              shift-left: _ -> [w1793]
              n1146 = case shown="True" w1802 {
                selector: w1802 -> [w1809 _]
                tunnel: w1804 -> [_ w1818]
                tunnel: w1803 -> [_ w1816]
                tunnel: [w1809 w1814] -> w1801
                tunnel: [w1808 w1813] -> w1800
                tunnel: [w1807 w1812] -> w1799
                tunnel: [w1806 w1811] -> w1798
                tunnel: [w1805 w1810] -> w1797
                tunnel: w1796 -> [w1808 _]
                tunnel: w1795 -> [w1807 _]
                tunnel: w1794 -> [w1806 _]
                tunnel: w1793 -> [w1805 _]
                frame False {
                }
                frame True {
                  n1147 = Unbundle(w1818) -> (w1817:T33)
                  n1148 = call "isclickinwindow.vi"("Image Param"=w1817, "Point32"=w1816) -> ("4 Y"=w1810:i32, "3 Height"=w1811:i32, "2 X"=w1812:i32, "1 Width"=w1813:i32, "In image?"=w1815:bool)  [unwired: 1 in]
                  n1149 = Not(x=w1815) -> (.not. x?=w1814:bool)
                }
              }
            }
            n1150 = Not(x=w1768) -> (.not. x?=w1767:bool)
            n1151 = case shown="True" w1767 {
              tunnel: w1765 -> [_ w1831]
              tunnel: w1763 -> [_ w1830]
              tunnel: w1766 -> [_ w1829]
              tunnel: w1764 -> [_ w1828]
              frame False {
              }
              frame True {
                w1824 = FALSE ("Get Point")
                n1152 = local read "Scan lines (y)"() -> (w1833:u64)
                n1153 = local read "Actual MCL Inc (V)"() -> (w1825:dbl)
                n1154 = local read "Scan steps (MCL)"() -> (w1832:u64)
                n1155 = Divide "Y Pix/step"(x=w1828, y=w1833) -> (x/y=w1840:dbl)
                n1156 = Divide "Y V/pix"(x=w1825, y=w1840) -> (x/y=w1839:dbl)
                n1157 = Divide "Y half step offset"(x=w1825, y=2.0) -> (x/y=w1841:dbl)
                n1158 = Divide "X pix/step"(x=w1829, y=w1832) -> (x/y=w1838:dbl)
                n1159 = Negate(x=w1841) -> (-x=w1842:dbl)
                n1160 = local read "Initial Y"() -> (w1848:dbl)
                n1161 = Multiply(x=w1830, y=w1839) -> (x*y=w1849:dbl)
                n1162 = Divide "X half step offset"(x=w1825, y=2.0) -> (x/y=w1835:dbl)
                n1163 = Divide "X V/pix"(x=w1825, y=w1838) -> (x/y=w1837:dbl)
                n1164 = Multiply(x=w1825, y=w1832) -> (x*y=w1844:dbl)
                n1165 = Compound Arithmetic op=ADD(w1842, w1849, w1848) -> (w1826:dbl)
                "Pointer Y (V)" <- w1826
                n1166 = Multiply(x=w1837, y=w1831) -> (x*y=w1846:dbl)
                n1167 = Negate(x=w1835) -> (-x=w1834:dbl)
                n1168 = local read "Initial X"() -> (w1847:dbl)
                n1169 = Negate(x=w1846) -> (-x=w1845:dbl)
                n1170 = Compound Arithmetic op=ADD(w1834, w1844, w1847, w1845) -> (w1827:dbl)
                "Pointer X (V)" <- w1827
                n1171 = Or(x="Set X Only", y="Set Confocal Spot (X-Y)") -> (x .or. y?=w1820:bool)
                n1172 = Or(x="Set Confocal Spot (X-Y)", y="Set Y Only") -> (x .or. y?=w1819:bool)
                n1173 = case shown="True" w1820 {
                  tunnel: w1827 -> [_ w1850]
                  frame False {
                  }
                  frame True {
                    n1174 = property on="AO2" class="Slide (strict)"("Val(Sgnl)"=w1850) -> ()  [unwired: 2 in, 2 out]
                  }
                }
                n1175 = case shown="True" w1819 {
                  tunnel: w1826 -> [_ w1851]
                  frame False {
                  }
                  frame True {
                    n1176 = property on="AO1" class="Slide (strict)"("Val(Sgnl)"=w1851) -> ()  [unwired: 2 in, 2 out]
                  }
                }
                n1177 = local write "Set Confocal Spot (X-Y)"(w1824) -> ()
                n1178 = local write "Set X Only"(w1824) -> ()
                n1179 = local write "Set Y Only"(w1824) -> ()
              }
            }
          }
          frame 3 {
            n1180 = local read "BD 2 Frequency 1 (MHz)"() -> (w1852:dbl)
            n1181 = local read "BD 1 Frequency 1 (MHz)"() -> (w1853:dbl)
            n1182 = local write "Manipulating Trap"(TRUE ("Manipulating Trap")) -> ()
            n1183 = local write "Coords"(T7 {"Horizontal"=0, "Vertical"=0} ("Coords")) -> ()
            n1184 = while {
              tunnel: w1858 -> [w1863]
              tunnel: w1856 -> [w1862]
              tunnel: w1854 -> [w1861]
              tunnel: w1853 -> [w1860]
              tunnel: w1852 -> [w1859]
              stop <- w1864 stop-if-true
              n1185 = event shown="[0] \"Pane\": Mouse Move" {
                selector: _ -> [_ _]
                dyn-events: _ -> [_ _]
                timeout: _ -> [_ _]
                tunnel: ["Force Manip Abort" w1928] -> w1864
                tunnel: w1863 -> [w1871 _]
                tunnel: w1862 -> [w1869 _]
                tunnel: w1861 -> [w1868 _]
                tunnel: w1860 -> [w1867 _]
                tunnel: w1859 -> [w1866 _]
                event Mouse Move {
                  n1186 = event-data() -> ("Time"=w1872:u32, "Coords"=w1873:T7)  [unwired: 3 out]
                  n1187 = Less?(x=w1872, y=w1871) -> (x < y?=w1870:bool)
                  n1188 = case "Makes sure old motion events prior to mouse click aren't used" shown="False" w1870 {
                    tunnel: w1873 -> [w1915 _]
                    tunnel: w1869 -> [w1916 _]
                    tunnel: w1868 -> [w1893 _]
                    tunnel: w1867 -> [w1889 _]
                    tunnel: w1866 -> [w1888 _]
                    frame False {
                      n1189 = Subtract(x=w1915, y=w1916) -> (x-y=w1914:T7)
                      "Coords" <- w1914
                      n1190 = local read "Y RF Frequency Limits (MHz)"() -> (w1874:T16)
                      n1191 = To Double Precision Float(number=w1914) -> (double precision float=w1913:cluster{"Horizontal":dbl, "Vertical":dbl})
                      n1192 = Multiply(x=cluster{"Horizontal":dbl, "Vertical":dbl} {"Horizontal"=-1.0, "Vertical"=1.0}, y="Manipulation Scaling") -> (x*y=w1909:cluster{"Horizontal":dbl, "Vertical":dbl})
                      n1193 = local read "X RF Frequency Limits (MHz)"() -> (w1875:T16)
                      n1194 = Multiply(x=w1913, y=w1909) -> (x*y=w1911:cluster{"Horizontal":dbl, "Vertical":dbl})
                      n1195 = Unbundle By Name(w1911) -> ("Horizontal"=w1906:dbl, "Vertical"=w1910:dbl)
                      n1196 = Unbundle By Name(w1874) -> ("Maximum"=w1877:dbl, "Minimum"=w1876:dbl)
                      n1197 = Boolean To (0,1)(Boolean="Manip. X?") -> (0, 1=w1904:i16)
                      n1198 = Boolean To (0,1)(Boolean="Manip. Y?") -> (0, 1=w1901:i16)
                      n1199 = local read "BD 1 Frequency 2 (MHz)"() -> (w1891:dbl)
                      n1200 = Multiply(x=w1910, y=w1901) -> (x*y=w1903:dbl)
                      n1201 = Multiply(x=w1904, y=w1906) -> (x*y=w1907:dbl)
                      n1202 = local read "BD 2 Frequency 2 (MHz)"() -> (w1890:dbl)
                      n1203 = Unbundle By Name(w1875) -> ("Maximum"=w1879:dbl, "Minimum"=w1878:dbl)
                      n1204 = Add(x=w1888, y=w1903) -> (x+y=w1881:dbl)
                      n1205 = Add(x=w1889, y=w1907) -> (x+y=w1883:dbl)
                      n1206 = In Range and Coerce(upper limit=w1879, x=w1883, lower limit=w1878) -> (coerced(x)=w1882:dbl)  [unwired: 1 out]
                      n1207 = In Range and Coerce(upper limit=w1877, x=w1881, lower limit=w1876) -> (coerced(x)=w1880:dbl)  [unwired: 1 out]
                      n1208 = Subtract(x=w1882, y=w1891) -> (x-y=w1900:dbl)
                      n1209 = Subtract(x=w1880, y=w1890) -> (x-y=w1899:dbl)
                      n1210 = Square(x=w1900) -> (x^2=w1898:dbl)
                      n1211 = Square(x=w1899) -> (x^2=w1897:dbl)
                      n1212 = Add(x=w1898, y=w1897) -> (x+y=w1896:dbl)
                      n1213 = Square Root(x=w1896) -> (sqrt(x)=w1892:dbl)
                      n1214 = In Range and Coerce(upper limit="Limit Max (MHz)", x=w1892, lower limit="Limit Min (MHz)") -> (In Range?=w1885:bool)  [unwired: 1 out]
                      n1215 = Not(x="Limits Enable") -> (.not. x?=w1884:bool)
                      n1216 = Or(x=w1885, y=w1884) -> (x .or. y?=w1886:bool)
                      n1217 = case shown="True" w1886 {
                        tunnel: w1893 -> [_ w1926]
                        tunnel: w1892 -> [_ w1917]
                        tunnel: w1882 -> [_ w1924]
                        tunnel: w1891 -> [_ w1923]
                        tunnel: w1880 -> [_ w1922]
                        tunnel: w1890 -> [_ w1921]
                        tunnel: w1875 -> [_ w1919]
                        tunnel: w1874 -> [_ w1918]
                        frame False {
                        }
                        frame True {
                          n1218 = local read "BD 1 Frequency 3 (MHz)"() -> (w1925:dbl)
                          n1219 = local read "BD 2 Frequency 3 (MHz)"() -> (w1920:dbl)
                          n1220 = local write "Trap Delta (MHz)"(w1917) -> ()
                          n1221 = property on="Initial delta (MHz)" class="DigNum (strict)"("Val(Sgnl)"=w1917) -> ()  [unwired: 2 in, 2 out]
                          n1222 = call "set RF board frequency - interlace.vi"("Board 2 Frequency Limits"=w1918, "Board 1 Frequency Limits"=w1919, "FPGA VI Reference In"=w1926, "Board 2 Frequency 3 (MHz)"=w1920, "Board 1 Frequency 3 (MHz)"=w1925, "Board 2 Frequency 2 (MHz)"=w1921, "Board 2 Frequency 1 (MHz)"=w1922, "Board 1 Frequency 2 (MHz)"=w1923, "Board 1 Frequency 1  (MHz)"=w1924) -> ()  [unwired: 1 in, 2 out]
                          n1223 = local write "BD 2 Frequency 1 (MHz)"(w1922) -> ()
                          n1224 = local write "BD 1 Frequency 1 (MHz)"(w1924) -> ()
                        }
                      }
                    }
                    frame True {
                    }
                  }
                }
                event Mouse Up {
                  n1225 = event-data() -> ("Button"=w1927:u16)  [unwired: 8 out]
                  n1226 = case shown="3" w1927 {
                    tunnel: [FALSE TRUE] -> w1928
                    frame 0, Default {
                    }
                    frame 3 {
                      n1227 = local write "Manipulating Trap"(FALSE ("Manipulating Trap")) -> ()
                    }
                  }
                }
              }
            }
          }
        }
      }
      event Mouse Move {
        n1228 = event-data() -> ()  [unwired: 6 out]
      }
    }
    n1229 = local read "Stop All"() -> (w1749:bool)
    n1230 = node-c288() -> ()  [unwired: 2 out]
  }
  n1231 = node-c288(i64 1 ("Period"), 1 ("Processor")) -> (w164:T24)  [unwired: 2 out]
  n1232 = timed-loop "Acquire Data" {
    tunnel: w24 -> [w2186]
    tunnel: w40 -> [w2185]
    tunnel: [w2216] -> w33
    tunnel: [w2210] -> w32
    timing: w164 -> [_]
    timing-out: [_] -> w163
    tunnel: w59 -> [w2014]
    stop <- "Stop All" stop-if-true
    (unwired) u32 0 ("Number of Elements")
    w2001 = "NI_ChannelName" ("name")
    n1233 = node-c288() -> ()  [unwired: 2 out]
    n1234 = First Call?() -> (First Call?: T/F=w1967:bool)
    n1235 = Or(x="Reset", y=w1967) -> (x .or. y?=w1968:bool)
    n1236 = case "Reset data stream" shown="True" w1968 {
      tunnel: w2186 -> [w2232 w2240]
      tunnel: w2185 -> [w2231 w2239]
      tunnel: [w2232 w2234] -> w2181
      tunnel: [w2231 w2233] -> w2180
      frame False {
      }
      frame True {
        w2237 = TRUE ("AI to FIFO")
        n1237 = local write "Overflow (data lost)"(FALSE ("Overflow (data lost)")) -> ()
        n1238 = call "reset FPGA DMA.vi"("error in"=w2239, "FPGA VI Reference In"=w2240) -> ("error out"=w2235:errorcluster, "FPGA VI Reference Out"=w2236:T19)
        n1239 = xnode "Read/Write Control"("FPGA VI Reference In"=w2236, "error in"=w2235, "AI to FIFO"=w2237, "APD to FIFO"=w2237) -> ("FPGA VI Reference Out"=w2234:T19, "error out"=w2233:errorcluster)
      }
    }
    n1240 = Or(x="Start AOD Scan", y="Trap Raster Scan") -> (x .or. y?=w2131:bool)
    n1241 = case "Start AOM raster scan" shown="True" w2131 {
      tunnel: w2181 -> [w2969 w2979]
      tunnel: w2180 -> [w2968 w2978]
      tunnel: [w2969 w2972] -> w2179
      tunnel: [w2968 w2971] -> w2178
      frame False {
      }
      frame True {
        n1242 = case shown="True" "Restart DMA? (AOD)" {
          tunnel: [w3017 w3019] -> w2973
          tunnel: [w3016 w3018] -> w2974
          tunnel: w2979 -> [w3017 w3021]
          tunnel: w2978 -> [w3016 w3020]
          frame False {
          }
          frame True {
            n1243 = local write "Overflow (data lost)"(FALSE ("Overflow (data lost)")) -> ()
            n1244 = call "reset FPGA DMA.vi"("error in"=w3020, "FPGA VI Reference In"=w3021) -> ("error out"=w3018:errorcluster, "FPGA VI Reference Out"=w3019:T19)
          }
        }
        n1245 = local write "Trap Raster Scan"(FALSE ("Trap Raster Scan")) -> ()
        n1246 = case shown="False" "Move MCL Also?" {
          tunnel: w2974 -> [w2982 w3011]
          tunnel: w2973 -> [w2983 w3012]
          tunnel: [w2981 w3015] -> w2972
          tunnel: [w2980 w3014] -> w2971
          frame False {
            w2984 = TRUE ("AI to FIFO")
            n1247 = xnode "Read/Write Control"("FPGA VI Reference In"=w2983, "error in"=w2982, "AI to FIFO"=w2984, "APD to FIFO"=w2984, "Start scan"=w2984) -> ("FPGA VI Reference Out"=w2981:T19, "error out"=w2980:errorcluster)
          }
          frame True {
            w3008 = FALSE ("1D or 2D Scan?")
            w3013 = TRUE ("AI to FIFO")
            # "Count for MCL loop"
            # "N total cycles"
            # "N steps"
            # "V_int"
            n1248 = local read "Scan Range (nm)"() -> (w2990:dbl)
            n1249 = local read "Number of F/B Scans (AOD)"() -> (w3007:u16)
            n1250 = Sign(1:w2990) -> (0:w2989:dbl)
            n1251 = Compound Arithmetic op=MULTIPLY(w2990, "MCL Step Position Ratio", "MCL/AOM Scale Tweak") -> (w2994:dbl)
            n1252 = Negate(x=w2989) -> (-x=w2986:dbl)
            n1253 = Multiply(x=w2986, y="MCL Step Increment (V_int)") -> (x*y=w2988:dbl)
            n1254 = Divide(x=w2994, y="MCL X Cal (nm/V)") -> (x/y=w3000:dbl)
            n1255 = Multiply(x=32767.0 ("y"), y=w3000) -> (x*y=w3006:dbl)
            n1256 = local read "Total Counts (ticks)"() -> (w2991:u32)
            n1257 = local read "Cycles/step (AOD)"() -> (w3002:u64)
            n1258 = local read "Scan steps (AOD)"() -> (w3003:u64)
            n1259 = Divide(x=w3006, y=10.0) -> (x/y=w2999:dbl)
            n1260 = Divide(x=w2999, y="MCL Step Increment (V_int)") -> (x/y=w2997:dbl)
            n1261 = Absolute Value(x=w2997) -> (abs(x)=w2985:dbl)
            n1262 = Compound Arithmetic op=MULTIPLY(w3003, w3002, w2991) -> (w2998:u64)
            n1263 = local write "wait to reset values"(w3013) -> ()
            n1264 = local write "MCL Scanning"(w3013) -> ()
            n1265 = Divide(x=w2998, y=w2985) -> (x/y=w2995:dbl)
            "MCL Count" <- w2995
            n1266 = xnode "Read/Write Control"("FPGA VI Reference In"=w3012, "error in"=w3011, "Scan steps (MCL)"=w2985, "Number of scans (MCL)"=w3007, "Cycles per step (MCL)"=u64 1, "Scan freq.  increment (MCL)"=w2988, "1D or 2D Scan?"=w3008, "MCL Scan Axis"=w3008, "Cont. Scan (MCL)"=w3008, "MCL count"=w2995) -> ("FPGA VI Reference Out"=w3010:T19, "error out"=w3009:errorcluster)
            n1267 = xnode "Read/Write Control"("FPGA VI Reference In"=w3010, "error in"=w3009, "AI to FIFO"=w3013, "APD to FIFO"=w3013, "Start scan"=w3013, "Start scan (MCL)"=w3013) -> ("FPGA VI Reference Out"=w3015:T19, "error out"=w3014:errorcluster)
          }
        }
        "Raster Scanning..." <- TRUE ("Scanning...")
      }
    }
    n1268 = And(x="Save scans", y=w2131) -> (x .and. y?=w2177:bool)
    n1269 = Compound Arithmetic op=OR("Start MCL Scan", "Confocal Image", "Confocal Linescan") -> (w2129:bool)
    n1270 = And(x="Save Data (MCL)", y=w2129) -> (x .and. y?=w2176:bool)
    n1271 = case "Start MCL raster scan" shown="True" w2129 {
      tunnel: w2179 -> [w2523 w2538]
      tunnel: w2178 -> [w2522 w2537]
      tunnel: [w2523 w2533] -> w1936
      tunnel: [w2522 w2532] -> w1935
      tunnel: [FALSE w2531] -> w2162
      tunnel: "Start MCL Scan" -> [_ w2526]
      tunnel: "Confocal Image" -> [_ w2525]
      tunnel: "Confocal Linescan" -> [_ _]
      frame False {
      }
      frame True {
        w2531 = TRUE
        n1272 = case shown="True" "Restart DMA? (MCL)" {
          tunnel: [w2583 w2585] -> w2536
          tunnel: [w2582 w2584] -> w2535
          tunnel: w2538 -> [w2583 w2588]
          tunnel: w2537 -> [w2582 w2587]
          frame False {
          }
          frame True {
            n1273 = call "reset FPGA DMA.vi"("error in"=w2587, "FPGA VI Reference In"=w2588) -> ("error out"=w2584:errorcluster, "FPGA VI Reference Out"=w2585:T19)
            n1274 = local write "Overflow (data lost)"(FALSE ("Overflow (data lost)")) -> ()
          }
        }
        n1275 = case shown="False" w2526 {
          selector: w2526 -> [_ w2542]
          tunnel: w2525 -> [w2541 _]
          tunnel: [w2541 w2542] -> w2524
          frame False {
            n1276 = property on="2D or 1D Scan" class="Bool (strict)"("Val(Sgnl)"=w2541) -> ()  [unwired: 2 in, 2 out]
            n1277 = property on="Confocal Image" class="Bool (strict)"("Value"=FALSE ("Start Confocal Map")) -> ()  [unwired: 2 in, 2 out]
          }
          frame True {
          }
        }
        n1278 = local write "MCL Scanning"(w2531) -> ()
        n1279 = local read "AO1"() -> (w2528:dbl)
        n1280 = local read "AO2"() -> (w2527:dbl)
        n1281 = case shown="True" "Center Scan" {
          tunnel: w2536 -> [w2549 w2581]
          tunnel: w2535 -> [w2548 w2580]
          tunnel: [w2547 w2579] -> w2533
          tunnel: [w2546 w2578] -> w2532
          tunnel: [w2544 w2565] -> w2530
          tunnel: [w2543 w2564] -> w2529
          tunnel: w2528 -> [w2544 w2570]
          tunnel: w2527 -> [w2543 w2573]
          tunnel: w2524 -> [_ _]
          frame False {
            w2545 = TRUE ("AI to FIFO")
            n1282 = xnode "Read/Write Control"("FPGA VI Reference In"=w2549, "error in"=w2548, "AI to FIFO"=w2545, "APD to FIFO"=w2545, "Start scan (MCL)"=w2545) -> ("FPGA VI Reference Out"=w2547:T19, "error out"=w2546:errorcluster)
          }
          frame True {
            w2577 = TRUE ("AI to FIFO")
            n1283 = local read "Scan steps (MCL)"() -> (w2556:u64)
            n1284 = local read "Scan lines (y)"() -> (w2552:u64)
            n1285 = local read "Fast Scan Dir"() -> (w2563:bool)
            n1286 = local read "Actual MCL Inc (V)"() -> (w2553:dbl)
            n1287 = Decrement(x=w2552) -> (x-1=w2551:u64)
            n1288 = Decrement(x=w2556) -> (x-1=w2555:u64)
            n1289 = Multiply(x=w2553, y=w2551) -> (x*y=w2550:dbl)
            n1290 = Divide(x=w2550, y=2.0) -> (x/y=w2560:dbl)
            n1291 = Multiply(x=w2553, y=w2555) -> (x*y=w2554:dbl)
            n1292 = Divide(x=w2554, y=2.0) -> (x/y=w2559:dbl)
            n1293 = Select(t=w2559, s=w2563, f=w2560) -> (s? t:f=w2558:dbl)
            n1294 = Select(t=w2560, s=w2563, f=w2559) -> (s? t:f=w2562:dbl)
            n1295 = Subtract(x=w2570, y=w2562) -> (x-y=w2561:dbl)
            n1296 = Subtract(x=w2573, y=w2558) -> (x-y=w2557:dbl)
            n1297 = local read "2D or 1D Scan"() -> (w2575:bool)
            n1298 = Not(x=w2563) -> (.not. x?=w2569:bool)
            n1299 = Not(x=w2575) -> (.not. x?=w2571:bool)
            n1300 = And(x=w2563, y=w2571) -> (x .and. y?=w2572:bool)
            n1301 = And(x=w2571, y=w2569) -> (x .and. y?=w2574:bool)
            n1302 = Select(t=w2573, s=w2574, f=w2557) -> (s? t:f=w2564:dbl)
            n1303 = Select(t=w2570, s=w2572, f=w2561) -> (s? t:f=w2565:dbl)
            n1304 = call "Volt to I16.vi"("Voltage In"=w2565) -> ("I16 Voltage Out"=w2568:i16)
            n1305 = call "Volt to I16.vi"("Voltage In"=w2564) -> ("I16 Voltage Out"=w2567:i16)
            n1306 = xnode "Read/Write Control"("FPGA VI Reference In"=w2581, "error in"=w2580, "AI to FIFO"=w2577, "APD to FIFO"=w2577, "Start scan (MCL)"=w2577, "AO1"=w2568, "AO2"=w2567) -> ("FPGA VI Reference Out"=w2579:T19, "error out"=w2578:errorcluster)
          }
        }
        "Initial Y" <- w2530
        "Initial X" <- w2529
        "wait to reset values" <- w2531
      }
    }
    n1307 = local read "Trap Pos Elements/DMA read"() -> (w2010:u32)
    n1308 = local read "Trap AI Elements/DMA read"() -> (w1934:u32)
    n1309 = local read "APD Elements/DMA read"() -> (w2053:u32)
    n1310 = local read "Trap AI FIFO Depth"() -> (w2226:u32)
    n1311 = xnode "Invoke Method"("FPGA VI Reference In"=w1936, "error in"=w1935, "Number of Elements"=w2010, "Timeout (ms)"=-1) -> ("Data"=w1974:u16[], "Elements Remaining"=→"Trap Pos FIFO El Remaining":u32)  [unwired: 2 out]
    n1312 = xnode "Invoke Method"("FPGA VI Reference In"=w1936, "error in"=w1935, "Number of Elements"=w1934, "Timeout (ms)"=-1 ("Timeout")) -> ("FPGA VI Reference Out"=w1938:T19, "error out"=w1937:errorcluster, "Data"=w1933:i16[], "Elements Remaining"=w1939:u32)
    "Trap AI FIFO El. Rem." <- w1939
    n1313 = xnode "Get APD Data"("FPGA VI Reference In"=w1936, "error in"=w1935, "Number of Elements"=w2053, "Timeout (ms)"=-1) -> ("Data"=w2052:u32[], "Elements Remaining"=→"APD FIFO Elements Remaining":u32)  [unwired: 2 out]
    n1314 = Subtract(x=w2226, y=w1934) -> (x-y=w2225:u32)
    n1315 = Decimate 1D Array(w1974) -> (w1971:u16[], w1973:u16[], w1972:u16[])
    n1316 = Divide(x=w1939, y=w2225) -> (x/y=w2224:dbl)
    "Buffer Status" <- w2224
    n1317 = To Unsigned Long Integer(number=w1971) -> (unsigned 32bit integer=w1970:u32[])
    n1318 = Join Numbers(hi=w1973, lo=w1972) -> ((hi.lo)=w1969:u32[])
    n1319 = Equal?(x=w2224, y=1.0) -> (x = y?=w2222:bool)
    n1320 = Join Numbers(hi=w1970, lo=w1969) -> ((hi.lo)=w1963:u64[])
    n1321 = call "IR AOM word to freq - vec.vi"("Frequency Word In (double vec)"=w1963) -> ("Frequency Out"=w2009:dbl[])
    n1322 = case "Alert buffer overflow" shown="True" w2222 {
      frame False {
      }
      frame True {
        n1323 = call <vilib>:"Beep.vi"() -> ()  [unwired: 3 in, 9 out]
        "Overflow (data lost)" <- TRUE ("Overflow (data lost)")
      }
    }
    n1324 = Decimate 1D Array(w2009) -> (w2008:dbl[], w2007:dbl[])
    n1325 = Array Size(array=w1933) -> (size(s)=→"Waveform Chart":i32)
    n1326 = Build Array(w2008, w2007) -> (w2006:dbl[][])
    n1327 = local read "Trap Sets"() -> (w2090:u32)
    n1328 = case "Deinterlace trap data, average down PSD" shown="2" w2090 {
      tunnel: w1933 -> [w2618 w2683]
      tunnel: [w2615 w2680] -> w2083
      tunnel: [w2618 w2682] -> w1966
      tunnel: "Detector Type" -> [w2617 w2678]
      tunnel: [w2616 w2681] -> w2082
      tunnel: [w2614 w2679] -> w2197
      frame 1, Default {
        n1329 = Divide(x=w2618, y=3276.7) -> (x/y=w2619:dbl[])
        n1330 = Decimate 1D Array(w2619) -> (w2628:dbl[], w2627:dbl[], w2626:dbl[], w2625:dbl[], w2624:dbl[], w2623:dbl[], w2622:dbl[], w2621:dbl[])
        n1331 = case shown="\"IR-QPD + PSD + FB-QPD position\"" w2617 {
          tunnel: w2628 -> [w2652 w2677]
          tunnel: w2627 -> [w2651 w2676]
          tunnel: w2626 -> [w2636 w2654]
          tunnel: w2625 -> [w2637 w2664]
          tunnel: w2624 -> [w2650 w2675]
          tunnel: w2623 -> [w2649 w2674]
          tunnel: w2622 -> [w2633 w2655]
          tunnel: w2621 -> [w2632 w2653]
          tunnel: [w2631 w2661] -> w2616
          tunnel: [w2630 w2660] -> w2615
          tunnel: [w2629 w2659] -> w2614
          frame "IR-QPD + PSD + FB-QPD", Default {
            w2629 = 0  # Channel pattern
            n1332 = Divide(x=w2652, y=w2637) -> (x/y=w2639:dbl[])
            n1333 = Divide(x=w2651, y=w2637) -> (x/y=w2638:dbl[])
            n1334 = Divide(x=w2650, y=w2633) -> (x/y=w2635:dbl[])
            n1335 = Divide(x=w2649, y=w2632) -> (x/y=w2634:dbl[])
            n1336 = Build Array(w2639, w2638, w2637, w2636, w2635, w2634, w2633, w2632) -> (w2630:dbl[][])
            n1337 = Bundle("T1 Y", "T1 X", "T1 Sum", "FB Sum", "PSD Y", "PSD X", "PSD Y Sum", "PSD X Sum") -> (w2648:T41)  [unwired: 1 out]
            n1338 = Cluster To Array(cluster=w2648) -> (array=w2631:string[])
          }
          frame "IR-QPD + PSD + FB-QPD position" {
            w2659 = 3  # Channel pattern
            n1339 = Negate(x=w2655) -> (-x=w2656:dbl[])
            n1340 = Divide(x=w2677, y=w2664) -> (x/y=w2666:dbl[])
            n1341 = Divide(x=w2676, y=w2664) -> (x/y=w2665:dbl[])
            n1342 = Divide(x=w2675, y=w2655) -> (x/y=w2663:dbl[])
            n1343 = Divide(x=w2674, y=w2656) -> (x/y=w2662:dbl[])
            n1344 = Build Array(w2666, w2665, w2664, w2653, w2654, w2663, w2662, w2655) -> (w2660:dbl[][])
            n1345 = Bundle("T1 Y", "T1 X", "T1 Sum", "FB X", "FB Sum", "PSD Y", "PSD X", "PSD Y Sum") -> (w2673:T41)  [unwired: 1 out]
            n1346 = Cluster To Array(cluster=w2673) -> (array=w2661:string[])
          }
        }
      }
      frame 2 {
        n1347 = case shown="\"UCB Fleezers 052511\"" w2678 {
          tunnel: w2683 -> [w2745 w2812 w2840 w2947]
          tunnel: [w2684 w2804 w2835 w2878] -> w2682
          tunnel: [w2711 w2795 w2837 w2925] -> w2681
          tunnel: [w2710 w2759 w2814 w2892] -> w2680
          tunnel: [w2704 w2794 w2877 w2923] -> w2679
          frame "IR-QPD + PSD + FB-QPD", Default {
            w2704 = 1  # Channel pattern
            # "time average x2 the 4th signal and the 4 psd signals (detection laser)"
            # "deinterlace 3 signals from qpd"
            n1348 = Decimate 1D Array(w2745) -> (w2744:i16[], w2743:i16[], w2709:i16[], w2742:i16[], w2732:i16[], w2730:i16[], w2729:i16[], w2727:i16[])
            n1349 = call "downsample 1D array - double.vi"("Ave N"=2.0, "Array In"=w2732) -> ("Array Out"=w2731:dbl[])  [unwired: 1 out]
            n1350 = call "downsample 1D array - double.vi"("Ave N"=2.0, "Array In"=w2727) -> ("Array Out"=w2726:dbl[])  [unwired: 1 out]
            n1351 = call "downsample 1D array - double.vi"("Ave N"=2.0, "Array In"=w2729) -> ("Array Out"=w2728:dbl[])  [unwired: 1 out]
            n1352 = call "downsample 1D array - double.vi"("Ave N"=2.0, "Array In"=w2730) -> ("Array Out"=w2712:dbl[])  [unwired: 1 out]
            n1353 = Decimate 1D Array(w2744) -> (w2741:i16[], w2713:i16[])
            n1354 = Decimate 1D Array(w2743) -> (w2740:i16[], w2738:i16[])
            n1355 = Decimate 1D Array(w2742) -> (w2739:i16[], w2737:i16[])
            n1356 = Decimate 1D Array(w2709) -> (w2708:i16[], w2707:i16[])
            n1357 = Interleave 1D Arrays(w2741, w2740, w2739, w2713, w2738, w2737, w2708, w2707, w2731, w2712, w2728, w2726) -> (w2725:dbl[])
            n1358 = To Word Integer(number=w2725) -> (16bit integer=w2684:i16[])
            n1359 = Divide(x=w2725, y=3276.7) -> (x/y=w2724:dbl[])
            n1360 = Decimate 1D Array(w2724) -> (w2723:dbl[], w2722:dbl[], w2721:dbl[], w2720:dbl[], w2719:dbl[], w2718:dbl[], w2706:dbl[], w2705:dbl[], w2717:dbl[], w2716:dbl[], w2715:dbl[], w2714:dbl[])
            n1361 = Divide(x=w2723, y=w2721) -> (x/y=w2691:dbl[])
            n1362 = Divide(x=w2722, y=w2721) -> (x/y=w2690:dbl[])
            n1363 = Divide(x=w2720, y=w2718) -> (x/y=w2689:dbl[])
            n1364 = Divide(x=w2719, y=w2718) -> (x/y=w2688:dbl[])
            n1365 = Divide(x=w2717, y=w2715) -> (x/y=w2687:dbl[])
            n1366 = Divide(x=w2716, y=w2714) -> (x/y=w2686:dbl[])
            n1367 = Bundle("T1 Y", "T1 X", "T1 Sum", "T2 Y", "T2 X", "T2 Sum", "T1 FB Sum", "T2 FB Sum", "PSD Y", "PSD X", "PSD Y Sum", "PSD X Sum") -> (w2692:T42)  [unwired: 1 out]
            n1368 = Build Array(w2691, w2690, w2721, w2689, w2688, w2718, w2706, w2705, w2687, w2686, w2715, w2714) -> (w2710:dbl[][])
            n1369 = Cluster To Array(cluster=w2692) -> (array=w2711:string[])
          }
          frame "IR-QPD + PSD + FB-QPD X position" {
            w2794 = 2  # Channel pattern
            # "convert\nADC numbers\nto volts"
            # "time average x2 the 3 psd signals (detection laser)"
            # "deinterlace 3 signals from qpds"
            n1370 = Decimate 1D Array(w2812) -> (w2811:i16[], w2810:i16[], w2747:i16[], w2748:i16[], w2757:i16[], w2754:i16[], w2751:i16[], w2782:i16[])
            n1371 = Decimate 1D Array(w2811) -> (w2809:i16[], w2796:i16[])
            n1372 = call "downsample 1D array - I16.vi"("Ave N"=2.0, "Array In"=w2757) -> ("Array Out"=w2755:i16[])  [unwired: 1 in]
            n1373 = call "downsample 1D array - I16.vi"("Ave N"=2.0, "Array In"=w2754) -> ("Array Out"=w2752:i16[])  [unwired: 1 in]
            n1374 = Decimate 1D Array(w2810) -> (w2808:i16[], w2806:i16[])
            n1375 = Decimate 1D Array(w2748) -> (w2807:i16[], w2805:i16[])
            n1376 = Decimate 1D Array(w2782) -> (w2781:i16[], w2779:i16[])
            n1377 = Decimate 1D Array(w2747) -> (w2780:i16[], w2778:i16[])
            n1378 = call "downsample 1D array - I16.vi"("Ave N"=2.0, "Array In"=w2751) -> ("Array Out"=w2749:i16[])  [unwired: 1 in]
            n1379 = Interleave 1D Arrays(w2809, w2808, w2807, w2796, w2806, w2805, w2781, w2780, w2779, w2778, w2755, w2752, w2749) -> (w2804:i16[])
            n1380 = Divide(x=w2804, y=3276.7) -> (x/y=w2803:dbl[])
            n1381 = Decimate 1D Array(w2803) -> (w2802:dbl[], w2801:dbl[], w2800:dbl[], w2799:dbl[], w2798:dbl[], w2797:dbl[], w2770:dbl[], w2768:dbl[], w2767:dbl[], w2765:dbl[], w2764:dbl[], w2763:dbl[], w2760:dbl[])
            n1382 = Divide(x=w2802, y=w2800) -> (x/y=w2786:dbl[])
            n1383 = Divide(x=w2801, y=w2800) -> (x/y=w2785:dbl[])
            n1384 = Divide(x=w2799, y=w2797) -> (x/y=w2784:dbl[])
            n1385 = Divide(x=w2798, y=w2797) -> (x/y=w2783:dbl[])
            n1386 = Divide(x=w2770, y=w2768) -> (x/y=w2769:dbl[])
            n1387 = Divide(x=w2767, y=w2765) -> (x/y=w2766:dbl[])
            n1388 = Divide(x=w2764, y=w2760) -> (x/y=w2762:dbl[])
            n1389 = Negate(x=w2760) -> (-x=w2758:dbl[])
            n1390 = Divide(x=w2763, y=w2758) -> (x/y=w2761:dbl[])
            n1391 = Bundle("T1 Y", "T1 X", "T1 Sum", "T2 Y", "T2 X", "T2 Sum", "T1 FB X", "T1 FB Sum", "T2 FB X", "T2 FB Sum", "PSD Y", "PSD X", "PSD Y Sum") -> (w2787:T43)  [unwired: 1 out]
            n1392 = Build Array(w2786, w2785, w2800, w2784, w2783, w2797, w2769, w2768, w2766, w2765, w2762, w2761, w2760) -> (w2759:dbl[][])
            n1393 = Cluster To Array(cluster=w2787) -> (array=w2795:string[])
          }
          frame "UCB Fleezers 052511" {
            w2877 = 2  # Channel pattern
            n1394 = Decimate 1D Array(w2840) -> (w2875:i16[], w2874:i16[], w2839:i16[], w2838:i16[], w2832:i16[], w2829:i16[], w2828:i16[], w2827:i16[])
            n1395 = Decimate 1D Array(w2875) -> (w2873:i16[], w2858:i16[])
            n1396 = Decimate 1D Array(w2874) -> (w2872:i16[], w2870:i16[])
            n1397 = Decimate 1D Array(w2839) -> (w2871:i16[], w2869:i16[])
            n1398 = Decimate 1D Array(w2838) -> (w2834:i16[], w2833:i16[])
            n1399 = Decimate 1D Array(w2832) -> (w2831:i16[], w2830:i16[])
            n1400 = call "downsample 1D array - I16.vi"("Ave N"=2.0, "Array In"=w2829) -> ("Array Out"=w2826:i16[])  [unwired: 1 in]
            n1401 = call "downsample 1D array - I16.vi"("Ave N"=2.0, "Array In"=w2828) -> ("Array Out"=w2825:i16[])  [unwired: 1 in]
            n1402 = call "downsample 1D array - I16.vi"("Ave N"=2.0, "Array In"=w2827) -> ("Array Out"=w2824:i16[])  [unwired: 1 in]
            n1403 = Interleave 1D Arrays(w2873, w2872, w2871, w2858, w2870, w2869, w2834, w2831, w2833, w2830, w2826, w2825, w2824) -> (w2835:i16[])
            n1404 = Divide(x=w2835, y=3276.7) -> (x/y=w2865:dbl[])
            n1405 = Decimate 1D Array(w2865) -> (w2864:dbl[], w2863:dbl[], w2862:dbl[], w2861:dbl[], w2860:dbl[], w2859:dbl[], w2823:dbl[], w2821:dbl[], w2820:dbl[], w2818:dbl[], w2817:dbl[], w2816:dbl[], w2815:dbl[])
            n1406 = Divide(x=w2864, y=w2862) -> (x/y=w2845:dbl[])
            n1407 = Divide(x=w2863, y=w2862) -> (x/y=w2844:dbl[])
            n1408 = Divide(x=w2861, y=w2859) -> (x/y=w2843:dbl[])
            n1409 = Divide(x=w2860, y=w2859) -> (x/y=w2842:dbl[])
            n1410 = Divide(x=w2823, y=w2821) -> (x/y=w2822:dbl[])
            n1411 = Divide(x=w2820, y=w2818) -> (x/y=w2819:dbl[])
            n1412 = Bundle("T1 Y", "T1 X", "T1 Sum", "T2 Y", "T2 X", "T2 Sum", "T1 FB X", "T2 FB Sum", "T2 FB X", "T2 FB Sum", "PSD Y", "PSD X", "PSD Sum") -> (w2846:T43)  [unwired: 1 out]
            n1413 = Build Array(w2845, w2844, w2862, w2843, w2842, w2859, w2822, w2821, w2819, w2818, w2817, w2816, w2815) -> (w2814:dbl[][])
            n1414 = Cluster To Array(cluster=w2846) -> (array=w2837:string[])
          }
          frame "IR-QPD + PSD + FB-QPD XY positions" {
            w2923 = 4  # Channel pattern
            # "time average x2 the 3 psd signals (detection laser)"
            # "deinterlace 3 signals from qpds"
            n1415 = Decimate 1D Array(w2947) -> (w2946:i16[], w2945:i16[], w2924:i16[], w2944:i16[], w2890:i16[], w2936:i16[], w2935:i16[], w2912:i16[])
            n1416 = Decimate 1D Array "QPD Y"(w2946) -> (w2943:i16[], w2926:i16[])
            n1417 = call "downsample 1D array - double.vi"("Ave N"=2.0, "Array In"=w2936) -> ("Array Out"=w2911:dbl[])  [unwired: 1 out]
            n1418 = call "downsample 1D array - double.vi"("Ave N"=2.0, "Array In"=w2935) -> ("Array Out"=w2910:dbl[])  [unwired: 1 out]
            n1419 = Decimate 1D Array "Feedback Sum"(w2924) -> (w2908:i16[], w2906:i16[])
            n1420 = Decimate 1D Array "Feedback Y"(w2890) -> (w2889:i16[], w2888:i16[])
            n1421 = Decimate 1D Array "Feedback X"(w2912) -> (w2909:i16[], w2907:i16[])
            n1422 = Decimate 1D Array "QPD Sum"(w2944) -> (w2941:i16[], w2939:i16[])
            n1423 = Decimate 1D Array "QPD X"(w2945) -> (w2942:i16[], w2940:i16[])
            n1424 = Interleave 1D Arrays(w2943, w2942, w2941, w2926, w2940, w2939, w2889, w2909, w2908, w2888, w2907, w2906, w2911, w2910) -> (w2934:dbl[])
            n1425 = To Word Integer(number=w2934) -> (16bit integer=w2878:i16[])
            n1426 = Divide(x=w2934, y=3276.7) -> (x/y=w2933:dbl[])
            n1427 = Decimate 1D Array(w2933) -> (w2932:dbl[], w2931:dbl[], w2930:dbl[], w2929:dbl[], w2928:dbl[], w2927:dbl[], w2885:dbl[], w2899:dbl[], w2883:dbl[], w2884:dbl[], w2897:dbl[], w2881:dbl[], w2895:dbl[], w2893:dbl[])
            n1428 = Divide(x=w2932, y=w2930) -> (x/y=w2916:dbl[])
            n1429 = Divide(x=w2931, y=w2930) -> (x/y=w2915:dbl[])
            n1430 = Divide(x=w2929, y=w2927) -> (x/y=w2914:dbl[])
            n1431 = Divide(x=w2928, y=w2927) -> (x/y=w2913:dbl[])
            n1432 = Divide(x=w2885, y=w2883) -> (x/y=w2882:dbl[])
            n1433 = Divide(x=w2899, y=w2883) -> (x/y=w2898:dbl[])
            n1434 = Divide(x=w2884, y=w2881) -> (x/y=w2880:dbl[])
            n1435 = Divide(x=w2897, y=w2881) -> (x/y=w2896:dbl[])
            n1436 = Negate(x=w2893) -> (-x=w2891:dbl[])
            n1437 = Divide(x=w2895, y=w2891) -> (x/y=w2894:dbl[])
            n1438 = Bundle("T1 Y", "T1 X", "T1 Sum", "T2 Y", "T2 X", "T2 Sum", "T1 FB Y", "T1 FB X", "T1 FB Sum", "T2 FB Y", "T2 FB X", "T2 FB Sum", "PSD X", "PSD Y Sum") -> (w2879:T44)  [unwired: 1 out]
            n1439 = Build Array(w2916, w2915, w2930, w2914, w2913, w2927, w2882, w2898, w2883, w2880, w2896, w2881, w2894, w2893) -> (w2892:dbl[][])
            n1440 = Cluster To Array(cluster=w2879) -> (array=w2925:string[])
          }
        }
      }
    }
    "AI labels" <- w2082
    n1441 = Decimate 1D Array(w2052) -> (w2080:u32[], w2016:u32[])
    n1442 = local read "DMA Update Period (s)"() -> (w2091:dbl)
    n1443 = local read "BD 1 Frequency 2 (MHz)"() -> (w1958:dbl)
    n1444 = local read "BD 1 Frequency 1 (MHz)"() -> (w1959:dbl)
    n1445 = Build Array(w2080, w2016) -> (w2159:u32[][])
    n1446 = local read "Data Period (s)"() -> (w2065:dbl)
    n1447 = Decimate 1D Array(w1966) -> (w1989:i16[], w1988:i16[], w1986:i16[], w1985:i16[])  [unwired: 9 out]
    n1448 = To Double Precision Float(number=w2159) -> (double precision float=w2160:dbl[][])
    n1449 = local read "APD Integration Time (s)"() -> (w2029:dbl)
    n1450 = Divide(x=w1989, y=w1988) -> (x/y=w1990:dbl[])
    n1451 = Divide(x=w1986, y=w1985) -> (x/y=w1987:dbl[])
    n1452 = feedback #1(0.0) -> (w2003:dbl)
    n1453 = Add(x=w2091, y=w2003) -> (x+y=w2199:dbl)
    n1454 = feedback-in #1(w2199) -> ()
    n1455 = local read "AOM X Cal (nm/MHz)"() -> (w1956:dbl)
    n1456 = To Time Stamp(1:w2003) -> (0:w2002:timestamp)
    n1457 = Split 1D Array(array=w1990, index="N El. to Ave.") -> (second subarray=w1993:dbl[])  [unwired: 1 out]
    n1458 = Split 1D Array(array=w1987, index="N El. to Ave.") -> (second subarray=w1992:dbl[])  [unwired: 1 out]
    n1459 = local read "Trap X AI1 (DMA)"() -> (w1991:T13)
    n1460 = Multiply(x=w2065, y="Trap Disp. Downsample") -> (x*y=w2004:dbl)
    "Display Period (s)" <- w2004
    n1461 = Bundle("BD 1 Frequency 1 (MHz)"=w1959, "BD 1 Frequency 2 (MHz)"=w1958) -> (w1960:T45)  [unwired: 1 out]
    n1462 = for "Trap AI" {
      tunnel: [w2613] -> w2193 mode=indexing
      tunnel: w2002 -> [w2603]
      tunnel: "Trap Disp. Downsample" -> [w2611]
      tunnel: w2083 -> [w2609] mode=indexing
      tunnel: w2065 -> [w2608]
      tunnel: w2082 -> [w2607] mode=indexing
      tunnel: w2001 -> [w2606]
      tunnel: [w2605] -> w2040 mode=indexing
      tunnel: w2004 -> [w2604]
      n1463 = Bundle By Name("Y"=w2609, "dt"=w2608) -> (w2610:waveform(dbl))  [unwired: 1 out]
      n1464 = Set Waveform Attribute(5:w2607, 6:w2606, 7:w2610) -> (3:w2605:waveform(dbl))  [unwired: 1 in, 2 out]
      n1465 = call "downsample 1D array - double.vi"("Ave N"=w2611, "Array In"=w2609) -> ("Array Out"=w2612:dbl[])  [unwired: 1 out]
      n1466 = Bundle By Name(cluster=w2605, "t0"=w2603, "Y"=w2612, "dt"=w2604) -> (w2613:waveform(dbl))
    }
    n1467 = call-poly <vilib>:"Mean.vi"("X"=w1992) -> ("mean"=w1980:dbl)  [unwired: 1 out]
    n1468 = call-poly <vilib>:"Mean.vi"("X"=w1993) -> ("mean"=w1981:dbl)  [unwired: 1 out]
    n1469 = Cluster To Array(cluster=w1960) -> (array=w1957:dbl[])
    n1470 = Reciprocal(x=w2004) -> (1/x=→"Trap Disp. Freq. (Hz)":dbl)
    n1471 = local read "Data points/scans (MCL)"() -> (w2171:dbl)
    n1472 = To Fixed-Point(number=w1980) -> (fixed-point=w1978:fxp<+/-,16,1>)  [unwired: 1 in]
    n1473 = To Fixed-Point(number=w1981) -> (fixed-point=w1979:fxp<+/-,16,1>)  [unwired: 1 in]
    n1474 = Bundle("Trap 1 Pos.", "Trap 2 Pos.") -> (w2000:cluster{string, string})  [unwired: 1 out]
    n1475 = Bundle By Name(cluster=w1991, "Set 1"=w1979, "Set 2"=w1978) -> (→"Trap X AI1 (DMA)":T13)
    n1476 = Cluster To Array(cluster=w2000) -> (array=w1997:string[])
    n1477 = for "Trap Position" {
      tunnel: w2006 -> [w2253] mode=indexing
      tunnel: "Trap Disp. Downsample" -> [w2252]
      tunnel: w2004 -> [w2250]
      tunnel: w2002 -> [w2249]
      tunnel: w2001 -> [w2247]
      tunnel: w1997 -> [w2246] mode=indexing
      tunnel: [w2245] -> w1955 mode=indexing
      tunnel: w1957 -> [w2243] mode=indexing
      tunnel: w1956 -> [w2241]
      n1478 = call "downsample 1D array - double.vi"("Ave N"=w2252, "Array In"=w2253) -> ("Array Out"=w2251:dbl[])  [unwired: 1 out]
      n1479 = Subtract(x=w2251, y=w2243) -> (x-y=w2244:dbl[])
      n1480 = Multiply(x=w2241, y=w2244) -> (x*y=w2242:dbl[])
      n1481 = Bundle By Name("Y"=w2242, "dt"=w2250, "t0"=w2249) -> (w2248:waveform(dbl))  [unwired: 1 out]
      n1482 = Set Waveform Attribute(5:w2246, 6:w2247, 7:w2248) -> (3:w2245:waveform(dbl))  [unwired: 1 in, 2 out]
    }
    "Trap Positions" <- w1955
    n1483 = Bundle("APD 1", "APD 2") -> (w2192:cluster{string, string})  [unwired: 1 out]
    n1484 = Cluster To Array(cluster=w2192) -> (array=w2189:string[])
    n1485 = for "APD" {
      tunnel: w2160 -> [w2592] mode=indexing
      tunnel: w2029 -> [w2600]
      tunnel: [w2596] -> w2036 mode=indexing
      tunnel: "APD Disp. Scale" -> [w2597]
      tunnel: w2001 -> [w2595]
      tunnel: w2189 -> [w2594] mode=indexing
      tunnel: "APD Disp. Downsample" -> [w2590]
      tunnel: [w2593] -> w2188
      tunnel: w2002 -> [w2589]
      n1486 = call "integrate 1D array interval - double.vi"("Ave N"=w2590, "Array In"=w2592) -> ("Array Out"=w2591:dbl[])  [unwired: 1 out]
      n1487 = Multiply(x=w2600, y=w2590) -> (x*y=w2593:dbl)
      n1488 = Divide(x=w2591, y=w2597) -> (x/y=w2598:dbl[])
      n1489 = Bundle By Name("t0"=w2589, "Y"=w2598, "dt"=w2593) -> (w2599:waveform(dbl))  [unwired: 1 out]
      n1490 = Set Waveform Attribute(5:w2594, 6:w2595, 7:w2599) -> (3:w2596:waveform(dbl))  [unwired: 1 in, 2 out]
    }
    "APD Display Period (s)" <- w2188
    n1491 = Reciprocal(x=w2188) -> (1/x=→"APD Display Freq. (Hz)":dbl)
    n1492 = local read "Display Period (s)"() -> (w2064:dbl)
    n1493 = Increment(x=w2171) -> (x+1=w2172:dbl)
    n1494 = Index Array(array=w1955, index=0) -> (element=w1953:waveform(dbl))
    n1495 = To Double Precision Float(number=w2080) -> (double precision float=w2079:dbl[])
    n1496 = feedback #2(w2172) -> (w2175:dbl)
    n1497 = Select(t=0, s=w2162, f=w2175) -> (s? t:f=w2168:dbl)
    n1498 = Array Size(array=w2079) -> (size(s)=w2174:i32)
    n1499 = Add(x=w2174, y=w2168) -> (x+y=w2169:dbl)
    n1500 = Unbundle By Name(w1953) -> ("Y"=w1951:dbl[])
    n1501 = feedback #3(w2080) -> (w2158:u32[])
    n1502 = Build Array (concatenate)(w2158, w2080) -> (w2155:u32[])
    n1503 = feedback #4(w2016) -> (w2035:u32[])
    n1504 = Divide(x="Bead Sep. Int. Time (s)", y=w2064) -> (x/y=w1949:dbl)
    n1505 = Build Array (concatenate)(w2035, w2016) -> (w2034:u32[])
    n1506 = Greater?(x=w2169, y=w2171) -> (0:w2170:bool)
    n1507 = feedback #5(w1951) -> (w1952:dbl[])
    n1508 = Build Array (concatenate)(w1951, w1952) -> (w1950:dbl[])
    n1509 = Select(t=w2168, s=w2170, f=w2169) -> (s? t:f=w2167:dbl)
    n1510 = feedback-in #2(w2167) -> ()
    n1511 = Array Size(array=w2155) -> (size(s)=w2152:i32)
    n1512 = Array Size(array=w2080) -> (size(s)=w2154:i32)
    n1513 = local read "MCL Scanning"() -> (w2165:bool)
    n1514 = local read "APD Integration Time (s)"() -> (w2043:dbl)
    n1515 = Build Array (concatenate)(w2036, w2193) -> (w2038:waveform(dbl)[])
    "All Signals" <- w2038
    n1516 = Split 1D Array(array=w1950, index=w1949) -> (first subarray=w1943:dbl[])  [unwired: 1 out]
    n1517 = feedback-in #5(w1943) -> ()
    n1518 = Multiply(x=w2154, y="APD Ave N") -> (x*y=w2153:dbl)
    n1519 = Greater?(x=w2152, y=w2153) -> (0:w2156:bool)
    n1520 = Not(x=w2170) -> (.not. x?=w2164:bool)
    n1521 = To Double Precision Float(number=w2016) -> (double precision float=w2015:dbl[])
    n1522 = call-poly <vilib>:"Mean.vi"("X"=w1943) -> ("mean"=w1942:dbl)  [unwired: 1 out]
    "Mean T1 Position (nm)" <- w1942
    n1523 = Subtract(x=w1943, y=w1942) -> (x-y=w1948:dbl[])
    n1524 = Square(x=w1948) -> (x^2=w1947:dbl[])
    n1525 = And(x=w2164, y=w2165) -> (x .and. y?=w2166:bool)
    n1526 = call-poly <vilib>:"Mean.vi"("X"=w1947) -> ("mean"=w1946:dbl)  [unwired: 1 out]
    n1527 = case shown="True" w2156 {
      tunnel: w2155 -> [w2373 w2380]
      tunnel: [w2373 w2378] -> w2096
      tunnel: w2153 -> [_ w2375]
      tunnel: w2152 -> [_ w2379]
      tunnel: w2034 -> [w2372 w2377]
      tunnel: [w2372 w2374] -> w2031
      frame False {
      }
      frame True {
        n1528 = Subtract(x=w2379, y=w2375) -> (x-y=w2376:dbl)
        n1529 = Array Subset(array=w2380, index=w2376, length=w2375) -> (w2378:u32[])
        n1530 = Array Subset(array=w2377, index=w2376, length=w2375) -> (w2374:u32[])
      }
    }
    n1531 = feedback-in #3(w2096) -> ()
    n1532 = feedback-in #4(w2031) -> ()
    n1533 = Or(x=w2166, y=w2162) -> (x .or. y?=w2163:bool)
    n1534 = Square Root(x=w1946) -> (sqrt(x)=w1945:dbl)
    n1535 = Equal?(x="Tab Control 6", y=T35."High Res Display") -> (x = y?=w2086:bool)
    n1536 = Multiply(x="APD Disp. Scale", y=w2036) -> (x*y=w2045:waveform(dbl)[])
    n1537 = Multiply(x="APD Disp. Downsample", y=w2043) -> (x*y=w2041:dbl)
    n1538 = Multiply(x=10.0, y=w1945) -> (x*y=→"Trap 1 Position RMS (A)":dbl)
    n1539 = Divide(x=w2045, y=w2041) -> (x/y=w2013:waveform(dbl)[])
    n1540 = Index Array(array=w2013, index=0) -> (element=w2023:waveform(dbl))
    n1541 = case "For computing FFTs for display" shown="True" "Compute FFT" {
      tunnel: w2040 -> [_ w3050]
      frame False {
      }
      frame True {
        n1542 = Build Array("FFT 1 Choice 1", "FFT 1 Choice 2", "FFT 2 Choice 1", "FFT 2 Choice 2") -> (w3043:u16[])
        n1543 = Array Size(array=w3050) -> (size(s)=w3049:i32)
        n1544 = feedback-in #6(w3043) -> ()
        n1545 = feedback #6(u16[] [100, 100, 100, 100]) -> (w3044:u16[])
        n1546 = feedback-in #7("# Spectra to Ave.") -> ()
        n1547 = feedback #7("# Spectra to Ave.") -> (w3041:dbl)
        n1548 = Not Equal?(x="# Spectra to Ave.", y=w3041) -> (x != y?=w3040:bool)
        n1549 = Not Equal?(x=w3043, y=w3044) -> (x != y?=w3042:bool)
        n1550 = feedback #8(1.0) -> (w3027:dbl)
        n1551 = Compound Arithmetic op=OR("Reset FFT", w3042, w3040) -> (w3025:bool)
        n1552 = Select(t=1.0, s=w3025, f=w3027) -> (s? t:f=w3029:dbl)
        n1553 = Greater?(x=w3029, y="# Spectra to Ave.") -> (0:w3048:bool)
        n1554 = Increment(x=w3029) -> (x+1=w3028:dbl)
        n1555 = feedback-in #8(w3028) -> ()
        n1556 = local read "DMA Update Period (s)"() -> (w3023:dbl)
        n1557 = Multiply(x="# Spectra to Ave.", y=w3023) -> (x*y=→"Ave. Time (s)":dbl)
        n1558 = Build Array(cluster{"f0":dbl, "df":dbl, "magnitude":dbl[]} {"f0"=0.0, "df"=0.0, "magnitude"=[]} ("PSD")) -> (w3032:cluster{"f0":dbl, "df":dbl, "magnitude":dbl[]}[])
        n1559 = Build Array(w3032, w3032, w3032, w3032) -> (w3034:T46)
        n1560 = feedback #9(w3034) -> (w3039:T46)
        n1561 = for {
          N: 4 -> [_]
          tunnel: w3043 -> [w3072] mode=indexing
          tunnel: w3050 -> [w3073]
          tunnel: w3049 -> [w3075]
          tunnel: w3025 -> [w3068]
          tunnel: w3048 -> [w3067]
          tunnel: "# Spectra to Ave." -> [w3066]
          tunnel: [w3065] -> w3038 mode=indexing
          tunnel: w3039 -> [w3070] mode=indexing
          tunnel: [w3069] -> w3026 mode=indexing
          tunnel: w3029 -> [w3064]
          n1562 = Less?(x=w3072, y=w3075) -> (x < y?=w3074:bool)
          n1563 = Index Array(array=w3073, index=w3072) -> (element=w3071:waveform(dbl))
          n1564 = case shown="True" w3074 {
            tunnel: w3071 -> [_ w3092]
            tunnel: w3070 -> [w3077 w3090]
            tunnel: [w3077 w3078] -> w3069
            tunnel: w3068 -> [_ w3089]
            tunnel: w3067 -> [_ w3082]
            tunnel: w3066 -> [_ w3081]
            tunnel: [cluster{"f0":dbl, "df":dbl, "magnitude":dbl[]} {"f0"=0.0, "df"=0.0, "magnitude"=[]} ("PSD") w3083] -> w3065
            tunnel: w3064 -> [_ w3080]
            frame False {
            }
            frame True {
              n1565 = call <vilib>:"Std Deviation and Variance.vi"("X"=w3092) -> ("mean"=w3093:dbl)  [unwired: 1 in, 2 out]
              n1566 = Subtract(x=w3092, y=w3093) -> (x-y=w3091:waveform(dbl))
              n1567 = xnode "Spectral Measurements"("Signals"=w3091) -> ("PSD"=w3085:cluster{"f0":dbl, "df":dbl, "magnitude":dbl[]})  [unwired: 1 in, 1 out]
              n1568 = case shown="False" w3089 {
                tunnel: w3090 -> [w3102 _]
                tunnel: [w3098 w3107] -> w3078
                tunnel: w3085 -> [w3101 w3108]
                tunnel: w3082 -> [w3100 _]
                frame False {
                  n1569 = Build Array (concatenate)(w3102, w3101) -> (w3099:cluster{"f0":dbl, "df":dbl, "magnitude":dbl[]}[])
                  n1570 = case shown="True" w3100 {
                    tunnel: w3099 -> [w3103 w3106]
                    tunnel: [w3103 w3104] -> w3098
                    frame False {
                    }
                    frame True {
                      n1571 = Delete From Array(array=w3106, index=0) -> (array with subset deleted=w3104:cluster{"f0":dbl, "df":dbl, "magnitude":dbl[]}[])  [unwired: 1 in, 1 out]
                    }
                  }
                }
                frame True {
                  n1572 = Build Array(w3108) -> (w3107:cluster{"f0":dbl, "df":dbl, "magnitude":dbl[]}[])
                }
              }
              n1573 = for {
                tunnel: w3078 -> [w3097] mode=indexing
                tunnel: [w3096] -> w3088 mode=indexing
                workers-P: _ -> [_]
                n1574 = Unbundle By Name(w3097) -> ("magnitude"=w3096:dbl[])
              }
              n1575 = Transpose 2D Array(2D array=w3088) -> (transposed array=w3087:dbl[][])
              n1576 = for {
                tunnel: w3087 -> [w3095] mode=indexing
                tunnel: [w3094] -> w3086 mode=indexing
                workers-P: _ -> [_]
                n1577 = Add Array Elements(numeric array=w3095) -> (sum=w3094:dbl)
              }
              n1578 = Select(t=w3081, s=w3082, f=w3080) -> (s? t:f=w3079:dbl)
              n1579 = Divide(x=w3086, y=w3079) -> (x/y=w3084:dbl[])
              n1580 = Bundle By Name(cluster=w3085, "magnitude"=w3084) -> (w3083:cluster{"f0":dbl, "df":dbl, "magnitude":dbl[]})
            }
          }
        }
        n1581 = case shown="True" w3025 {
          tunnel: w3026 -> [w3057 w3063]
          tunnel: [w3057 w3058] -> w3024
          frame False {
          }
          frame True {
            n1582 = Array Subset(array=w3063, index (row)=0 ("index"), length (row)=4 ("length"), index (col)=0 ("index"), length (col)=1 ("length")) -> (w3058:T46)
          }
        }
        n1583 = feedback-in #9(w3024) -> ()
        n1584 = Split 1D Array(array=w3038, index=2) -> (first subarray=→"FFT 1":cluster{"f0":dbl, "df":dbl, "magnitude":dbl[]}[], second subarray=→"FFT 2":cluster{"f0":dbl, "df":dbl, "magnitude":dbl[]}[])
      }
    }
    n1585 = Index Array(array=w2013, index=1) -> (element=w2021:waveform(dbl))
    n1586 = case "For displaying the high resolution display (no downsampling)" shown="True" w2086 {
      tunnel: w2040 -> [_ w2273]
      frame False {
      }
      frame True {
        n1587 = Index Array(array=w2273, index="High Res. Display") -> (element=w2274:waveform(dbl))
        n1588 = call <vilib>:"Std Deviation and Variance.vi"("X"=w2274) -> ("mean"=w2281:dbl, "standard deviation"=w2286:dbl)  [unwired: 1 in, 1 out]
        "Mean Intensity" <- w2281
        "Sigma" <- w2286
        n1589 = Subtract(x=w2274, y=w2281) -> (x-y=w2280:waveform(dbl))
        n1590 = Select(t=w2280, s="Subtract mean", f=w2274) -> (s? t:f=→"1 Channel":waveform(dbl))
        n1591 = Divide(x=w2286, y=w2281) -> (x/y=→"Sigma/Mean":dbl)
        n1592 = feedback #10(1) -> (w2275:i32)
        n1593 = Greater Or Equal?(x=w2275, y="Slow mean N ave.") -> (x >= y?=w2288:bool)
        n1594 = Increment(x=w2275) -> (x+1=w2290:i32)
        n1595 = Select(t=1, s=w2288, f=w2290) -> (s? t:f=w2277:i32)
        n1596 = feedback-in #10(w2277) -> ()
        n1597 = feedback #11() -> (w2278:waveform(dbl))  [unwired: 1 out]
        n1598 = case shown="Default" w2275 {
          tunnel: [w2293 w2296] -> w2279
          tunnel: w2278 -> [w2295 _]
          tunnel: w2274 -> [w2294 w2296]
          frame Default {
            n1599 = call-poly <vilib>:"Append Waveforms.vi"("waveform B"=w2294, "waveform A"=w2295) -> ("waveform out"=w2293:waveform(dbl))  [unwired: 1 in, 8 out]
          }
          frame 1 {
          }
        }
        n1600 = feedback-in #11(w2279) -> ()
        n1601 = case shown="True" w2288 {
          tunnel: w2279 -> [_ w2292]
          frame False {
          }
          frame True {
            n1602 = call-poly <vilib>:"Mean.vi"("X"=w2292) -> ("mean"=→"Slow mean":dbl)  [unwired: 1 out]
          }
        }
      }
    }
    n1603 = case "For plotting results of scanning MCL" shown="True" w2163 {
      tunnel: w2162 -> [_ w2413]
      tunnel: w2079 -> [_ w2509]
      tunnel: w2171 -> [_ _]
      tunnel: w2040 -> [_ w2483]
      tunnel: w2015 -> [_ w2414]
      tunnel: w2014 -> [_ w2387]
      frame False {
      }
      frame True {
        w2394 = u32 0 items=["Horizontal", "Vertical", "Central", "1st Diagonal", "2nd Diagonal"] ("Type of Symmetry")
        w2422 = u32 0 items=["Horizontal", "Vertical", "Central", "1st Diagonal", "2nd Diagonal"] ("Type of Symmetry")
        w2425 = u32 0 items=["Horizontal", "Vertical", "Central", "1st Diagonal", "2nd Diagonal"] ("Type of Symmetry")
        w2454 = u32 0 items=["Horizontal", "Vertical", "Central", "1st Diagonal", "2nd Diagonal"] ("Type of Symmetry")
        n1604 = Index Array(array=w2483, index=10) -> (element=w2489:waveform(dbl))
        n1605 = Index Array(array=w2483, index=11) -> (element=w2486:waveform(dbl))
        n1606 = local read "Cycles/step (MCL)"() -> (w2439:u64)
        n1607 = Index Array(array=w2483, index="Channel") -> (element=w2485:waveform(dbl))
        n1608 = Unbundle(w2387) -> ("New Image"=w2386:T2, "New Image"=w2385:T2, "New Image"=w2384:T2, "New Image"=w2383:T2)
        n1609 = Unbundle By Name(w2489) -> ("Y"=w2441:dbl[])
        n1610 = Unbundle By Name(w2486) -> ("Y"=w2443:dbl[])
        n1611 = Unbundle By Name(w2485) -> ("Y"=w2448:dbl[])
        n1612 = call "downsample 1D array - double.vi"("Ave N"=w2439, "Array In"=w2441) -> ("Array Out"=w2440:dbl[])  [unwired: 1 out]
        n1613 = call "downsample 1D array - double.vi"("Ave N"=w2439, "Array In"=w2443) -> ("Array Out"=w2442:dbl[])  [unwired: 1 out]
        n1614 = call "downsample 1D array - double.vi"("Ave N"=w2439, "Array In"=w2448) -> ("Array Out"=w2447:dbl[])  [unwired: 1 out]
        n1615 = feedback #12(w2509) -> (w2510:dbl[])
        n1616 = Build Array (concatenate)(w2510, w2509) -> (w2491:dbl[])
        n1617 = feedback #13(w2414) -> (w2416:dbl[])
        n1618 = Build Array (concatenate)(w2416, w2414) -> (w2415:dbl[])
        n1619 = local read "Scan steps (MCL)"() -> (w2396:u64)
        n1620 = Select(t=w2509, s=w2413, f=w2491) -> (s? t:f=w2495:dbl[])
        n1621 = feedback-in #12(w2495) -> ()
        n1622 = Select(t=w2414, s=w2413, f=w2415) -> (s? t:f=w2397:dbl[])
        n1623 = feedback-in #13(w2397) -> ()
        n1624 = local read "Scan lines (y)"() -> (w2382:u64)
        n1625 = local read "N APD Samp/step"() -> (w2398:dbl)
        n1626 = feedback #14(w2440) -> (w2497:dbl[])
        n1627 = Build Array (concatenate)(w2497, w2440) -> (w2488:dbl[])
        n1628 = feedback #15(w2447) -> (w2507:dbl[])
        n1629 = Build Array (concatenate)(w2507, w2447) -> (w2506:dbl[])
        n1630 = feedback #16(w2442) -> (w2499:dbl[])
        n1631 = Build Array (concatenate)(w2499, w2442) -> (w2500:dbl[])
        n1632 = Select(t=w2440, s=w2413, f=w2488) -> (s? t:f=w2444:dbl[])
        n1633 = feedback-in #14(w2444) -> ()
        n1634 = Select(t=w2447, s=w2413, f=w2506) -> (s? t:f=w2446:dbl[])
        n1635 = feedback-in #15(w2446) -> ()
        n1636 = Select(t=w2442, s=w2413, f=w2500) -> (s? t:f=w2445:dbl[])
        n1637 = feedback-in #16(w2445) -> ()
        n1638 = Multiply(x=w2396, y=u64 2) -> (x*y=w2381:u64)
        n1639 = call "integrate 1D array interval - double.vi"("Ave N"=w2398, "Array In"=w2397) -> ("Array Out"=w2409:dbl[])  [unwired: 1 out]
        n1640 = call "integrate 1D array interval - double.vi"("Ave N"=w2398, "Array In"=w2495) -> ("Array Out"=w2494:dbl[])  [unwired: 1 out]
        n1641 = Array Size(array=w2409) -> (size(s)=w2410:i32)
        n1642 = Array Size(array=w2494) -> (size(s)=w2496:i32)
        n1643 = Multiply(x=w2382, y=w2381) -> (x*y=w2412:u64)
        n1644 = Multiply(x=w2382, y=w2381) -> (x*y=w2504:u64)
        n1645 = call-poly <vilib>:"Mean.vi"("X"=w2444) -> ("mean"=w2428:dbl)  [unwired: 1 out]
        n1646 = Subtract(x=w2412, y=w2410) -> (x-y=w2403:u64)
        n1647 = call-poly <vilib>:"Mean.vi"("X"=w2446) -> ("mean"=w2433:dbl)  [unwired: 1 out]
        n1648 = call-poly <vilib>:"Mean.vi"("X"=w2445) -> ("mean"=w2431:dbl)  [unwired: 1 out]
        n1649 = call-poly <vilib>:"Mean.vi"("X"=w2409) -> ("mean"=w2400:dbl)  [unwired: 1 out]
        n1650 = Subtract(x=w2504, y=w2496) -> (x-y=w2438:u64)
        n1651 = call-poly <vilib>:"Mean.vi"("X"=w2494) -> ("mean"=w2435:dbl)  [unwired: 1 out]
        n1652 = Initialize Array(1.0 ("element"), w2403) -> (w2399:dbl[])
        n1653 = Initialize Array(1.0 ("element"), w2438) -> (w2429:dbl[])
        n1654 = Multiply(x=w2399, y=w2400) -> (x*y=w2401:dbl[])
        n1655 = Multiply(x=w2429, y=w2431) -> (x*y=w2432:dbl[])
        n1656 = Multiply(x=w2429, y=w2433) -> (x*y=w2434:dbl[])
        n1657 = Multiply(x=w2429, y=w2428) -> (x*y=w2430:dbl[])
        n1658 = Multiply(x=w2429, y=w2435) -> (x*y=w2436:dbl[])
        n1659 = Build Array (concatenate)(w2444, w2430) -> (w2498:dbl[])
        n1660 = Build Array (concatenate)(w2446, w2434) -> (w2502:dbl[])
        n1661 = Build Array (concatenate)(w2445, w2432) -> (w2501:dbl[])
        n1662 = Build Array (concatenate)(w2409, w2401) -> (w2411:dbl[])
        n1663 = Build Array (concatenate)(w2494, w2436) -> (w2503:dbl[])
        n1664 = Reshape Array(w2498, w2382, w2381) -> (w2464:dbl[][])
        n1665 = Reshape Array(w2411, w2382, w2381) -> (w2407:dbl[][])
        n1666 = Reshape Array(w2502, w2382, w2381) -> (w2456:dbl[][])
        n1667 = Reshape Array(w2501, w2382, w2381) -> (w2471:dbl[][])
        n1668 = Reshape Array(w2503, w2382, w2381) -> (w2481:dbl[][])
        n1669 = Array Subset(array=w2471, index (col)=0 ("index"), length (col)=w2396) -> (w2476:dbl[][])  [unwired: 2 in]
        n1670 = Array Subset(array=w2471, index (col)=w2396) -> (w2474:dbl[][])  [unwired: 3 in]
        n1671 = Array Subset(array=w2456, index (col)=0 ("index"), length (col)=w2396) -> (w2462:dbl[][])  [unwired: 2 in]
        n1672 = Array Subset(array=w2456, index (col)=w2396) -> (w2460:dbl[][])  [unwired: 3 in]
        n1673 = Array Subset(array=w2407, index (col)=0 ("index"), length (col)=w2396) -> (w2406:dbl[][])  [unwired: 2 in]
        n1674 = Array Subset(array=w2407, index (col)=w2396) -> (w2404:dbl[][])  [unwired: 3 in]
        n1675 = Array Subset(array=w2481, index (col)=0 ("index"), length (col)=w2396) -> (w2480:dbl[][])  [unwired: 2 in]
        n1676 = Array Subset(array=w2481, index (col)=w2396) -> (w2478:dbl[][])  [unwired: 3 in]
        n1677 = Array Subset(array=w2464, index (col)=0 ("index"), length (col)=w2396) -> (w2469:dbl[][])  [unwired: 2 in]
        n1678 = Array Subset(array=w2464, index (col)=w2396) -> (w2467:dbl[][])  [unwired: 3 in]
        n1679 = for {
          tunnel: w2476 -> [w2518] mode=indexing
          tunnel: [w2517] -> w2475 mode=indexing
          workers-P: _ -> [_]
          n1680 = Reverse 1D Array(array=w2518) -> (reversed array=w2517:dbl[])
        }
        n1681 = for {
          tunnel: w2462 -> [w2514] mode=indexing
          tunnel: [w2513] -> w2461 mode=indexing
          workers-P: _ -> [_]
          n1682 = Reverse 1D Array(array=w2514) -> (reversed array=w2513:dbl[])
        }
        n1683 = for {
          tunnel: w2406 -> [w2512] mode=indexing
          tunnel: [w2511] -> w2405 mode=indexing
          workers-P: _ -> [_]
          n1684 = Reverse 1D Array(array=w2512) -> (reversed array=w2511:dbl[])
        }
        n1685 = for {
          tunnel: w2480 -> [w2520] mode=indexing
          tunnel: [w2519] -> w2479 mode=indexing
          workers-P: _ -> [_]
          n1686 = Reverse 1D Array(array=w2520) -> (reversed array=w2519:dbl[])
        }
        n1687 = for {
          tunnel: w2469 -> [w2516] mode=indexing
          tunnel: [w2515] -> w2468 mode=indexing
          workers-P: _ -> [_]
          n1688 = Reverse 1D Array(array=w2516) -> (reversed array=w2515:dbl[])
        }
        n1689 = Index Array(array=w2481, index (row)=0) -> (element=→"Waveform Graph":dbl[])  [unwired: 1 in]
        n1690 = Add(x=w2475, y=w2474) -> (x+y=w2473:dbl[][])
        n1691 = Add(x=w2461, y=w2460) -> (x+y=w2459:dbl[][])
        n1692 = Add(x=w2405, y=w2404) -> (x+y=w2389:dbl[][])
        n1693 = Add(x=w2479, y=w2478) -> (x+y=w2453:dbl[][])
        n1694 = Add(x=w2468, y=w2467) -> (x+y=w2466:dbl[][])
        n1695 = Divide(x=w2459, y=2) -> (x/y=w2457:dbl[][])
        n1696 = Divide(x=w2473, y=2) -> (x/y=w2418:dbl[][])
        n1697 = Divide(x=w2466, y=2) -> (x/y=w2420:dbl[][])
        n1698 = To Single Precision Float(number=w2453) -> (single precision float=w2452:sgl[][])
        n1699 = Transpose 2D Array(2D array=w2457) -> (transposed array=→"Data map":dbl[][])
        n1700 = To Single Precision Float(number=w2389) -> (single precision float=w2393:sgl[][])
        n1701 = To Single Precision Float(number=w2418) -> (single precision float=w2424:sgl[][])
        n1702 = To Single Precision Float(number=w2420) -> (single precision float=w2421:sgl[][])
        n1703 = call "IMAQ ArrayToImage"("Image Pixels (Float)"=w2452, "Image"=w2386) -> ("Image Out"=w2455:T2)  [unwired: 8 in, 1 out]
        n1704 = call "IMAQ ArrayToImage"("Image Pixels (Float)"=w2393, "Image"=w2385) -> ("Image Out"=w2395:T2)  [unwired: 8 in, 1 out]
        n1705 = call "IMAQ ArrayToImage"("Image Pixels (Float)"=w2424, "Image"=w2384) -> ("Image Out"=w2426:T2)  [unwired: 8 in, 1 out]
        n1706 = call "IMAQ ArrayToImage"("Image Pixels (Float)"=w2421, "Image"=w2383) -> ("Image Out"=w2423:T2)  [unwired: 8 in, 1 out]
        n1707 = call "IMAQ Symmetry"("Type of Symmetry"=w2454, "Image Src"=w2455) -> ("Image Dst Out"=w2450:T2)  [unwired: 3 in, 1 out]
        n1708 = call "IMAQ Symmetry"("Type of Symmetry"=w2394, "Image Src"=w2395) -> ("Image Dst Out"=w2391:T2)  [unwired: 3 in, 1 out]
        n1709 = call "IMAQ Symmetry"("Type of Symmetry"=w2425, "Image Src"=w2426) -> ("Image Dst Out"=→"Detection Laser X":T2)  [unwired: 3 in, 1 out]
        n1710 = call "IMAQ Symmetry"("Type of Symmetry"=w2422, "Image Src"=w2423) -> ("Image Dst Out"=→"Detection Laser Y":T2)  [unwired: 3 in, 1 out]
        n1711 = call "IMAQ Set Simple Calibration"("Calibration Axis Info"=T36 {"Origin Pixel"={"X"=0.0, "Y"=0.0}, "Angle Relative to Horizontal (deg)"=0.0, "Axis Reference"=0}, "Grid Descriptor"=T37 {"X Step"=0.3, "Y Step"=0.3, "Unit"=enum."Undefined"}, "Image"=w2450) -> ("Calibrated Image"=→"APD 1":T2)  [unwired: 7 in, 1 out]
        n1712 = call "IMAQ Set Simple Calibration"("Calibration Axis Info"=T36 {"Origin Pixel"={"X"=0.0, "Y"=0.0}, "Angle Relative to Horizontal (deg)"=0.0, "Axis Reference"=0}, "Grid Descriptor"=T37 {"X Step"=0.3, "Y Step"=0.3, "Unit"=enum."Undefined"}, "Image"=w2391) -> ("Calibrated Image"=→"APD 2":T2)  [unwired: 7 in, 1 out]
      }
    }
    n1713 = Subtract(x=w2021, y="APD 2 Offset") -> (x-y=w2018:waveform(dbl))
    n1714 = Subtract(x=w2023, y="APD 1 Offset") -> (x-y=w2019:waveform(dbl))
    n1715 = Index Array(array=w2038, index=3) -> (element=w2107:waveform(dbl))
    n1716 = Index Array(array=w2038, index=6) -> (element=w2104:waveform(dbl))
    n1717 = Build Array(w2019, w2018) -> (→"APD Chart":waveform(dbl)[])
    n1718 = Array Size(array=w2096) -> (size(s)=w2151:i32)
    n1719 = call <vilib>:"Std Deviation and Variance.vi"("X"=w2031) -> ("standard deviation"=w2030:dbl)  [unwired: 1 in, 2 out]
    n1720 = Add Array Elements(numeric array=w2031) -> (sum=w2033:u32)
    n1721 = Add Array Elements(numeric array=w2096) -> (sum=w2161:u32)
    n1722 = call <vilib>:"Std Deviation and Variance.vi"("X"=w2096) -> ("standard deviation"=w2095:dbl)  [unwired: 1 in, 2 out]
    n1723 = Divide(x="T1 offset_x (mV)", y=1000.0) -> (x/y=w2108:dbl)
    n1724 = Divide(x=w2030, y=w2029) -> (x/y=w2026:dbl)
    "Rate sigma (Hz) 2" <- w2026
    n1725 = Multiply(x=w2029, y=w2151) -> (x*y=w2032:dbl)
    "Int. Time (s)" <- w2032
    n1726 = Divide(x=w2033, y=w2032) -> (x/y=w2027:dbl)
    "APD 2 Rate (Hz)" <- w2027
    n1727 = Divide(x=w2161, y=w2032) -> (x/y=w2093:dbl)
    "APD 1 Rate (Hz)" <- w2093
    n1728 = Divide(x=w2095, y=w2029) -> (x/y=w2094:dbl)
    "Rate sigma (Hz)" <- w2094
    n1729 = Divide(x=w2026, y=w2027) -> (x/y=→"Sigma/Mean 2":dbl)
    n1730 = Divide(x=w2094, y=w2093) -> (x/y=→"Sigma/Mean":dbl)
    n1731 = Divide(x="T2 offset_x (mV)", y=1000.0) -> (x/y=w2106:dbl)
    n1732 = case shown="1" "Calibration" {
      tunnel: "T1 alpha_x (nm/V)" -> [_ w2349 w2370]
      tunnel: "T1 kappa_x (pN/nm)" -> [_ _ w2360]
      tunnel: "T2 alpha_x (nm/V)" -> [_ w2348 w2368]
      tunnel: "T2 kappa_x (pN/nm)" -> [_ _ w2361]
      tunnel: w2107 -> [w2331 w2346 w2366]
      tunnel: w2104 -> [w2330 w2344 w2364]
      tunnel: [w2331 w2343 w2363] -> w2137
      tunnel: [w2330 w2342 w2362] -> w2136
      tunnel: ["T1 X (V)" ("Label.Text") "T1 X (nm)" ("Label.Text") "T1 X (pN)" ("Label.Text")] -> w2125
      tunnel: ["T2 X (V)" ("Label.Text") "T2 X (nm)" ("Label.Text") "T2 X (pN)" ("Label.Text")] -> w2124
      tunnel: ["Position (V)" ("Label.Text") "Position (nm)" ("Label.Text") "Force (pN)" ("Label.Text")] -> w2126
      tunnel: w2106 -> [_ w2334 w2353]
      tunnel: w2108 -> [_ w2337 w2355]
      tunnel: ["Mean (V)" ("Label.Text") "Mean (nm)" ("Label.Text") "Mean (pN)" ("Label.Text")] -> w2121
      tunnel: ["Difference (V)" ("Label.Text") "Difference (nm)" ("Label.Text") "Difference (pN)" ("Label.Text")] -> w2046
      frame 0, Default {
      }
      frame 1 {
        # "position"
        n1733 = Unbundle By Name(w2346) -> ("Y"=w2350:dbl[])
        n1734 = Unbundle By Name(w2344) -> ("Y"=w2335:dbl[])
        n1735 = Subtract(x=w2350, y=w2337) -> (x-y=w2338:dbl[])
        n1736 = Subtract(x=w2335, y=w2334) -> (x-y=w2336:dbl[])
        n1737 = Multiply(x=w2336, y=w2348) -> (x*y=w2345:dbl[])
        n1738 = Multiply(x=w2349, y=w2338) -> (x*y=w2347:dbl[])
        n1739 = Bundle By Name(cluster=w2344, "Y"=w2345) -> (w2342:waveform(dbl))
        n1740 = Bundle By Name(cluster=w2346, "Y"=w2347) -> (w2343:waveform(dbl))
      }
      frame 2 {
        # "force"
        n1741 = Unbundle By Name(w2366) -> ("Y"=w2371:dbl[])
        n1742 = Unbundle By Name(w2364) -> ("Y"=w2369:dbl[])
        n1743 = Subtract(x=w2369, y=w2353) -> (x-y=w2354:dbl[])
        n1744 = Subtract(x=w2371, y=w2355) -> (x-y=w2356:dbl[])
        n1745 = Compound Arithmetic op=MULTIPLY(w2354, w2368, w2361) -> (w2365:dbl[])
        n1746 = Compound Arithmetic op=MULTIPLY(w2360, w2370, w2356) -> (w2367:dbl[])
        n1747 = Bundle By Name(cluster=w2364, "Y"=w2365) -> (w2362:waveform(dbl))
        n1748 = Bundle By Name(cluster=w2366, "Y"=w2367) -> (w2363:waveform(dbl))
      }
    }
    n1749 = feedback-in #17("Calibration") -> ()
    n1750 = feedback #17(u16 1 ("Calibration")) -> (w2128:u16)
    n1751 = Not Equal?(x=w2128, y="Calibration") -> (x != y?=w2084:bool)
    n1752 = Unbundle By Name(w2107) -> ("Y"=w2110:dbl[])
    n1753 = Unbundle By Name(w2104) -> ("Y"=w2113:dbl[])
    n1754 = Subtract(x=w2110, y=w2108) -> (x-y=w2111:dbl[])
    n1755 = Subtract(x=w2113, y=w2106) -> (x-y=w2112:dbl[])
    n1756 = disable-structure shown="Enabled" {
      disable-tunnel: [-1.0 ("y") 1.0] -> w2114
      frame Disabled {
      }
      frame Enabled {
      }
    }
    n1757 = Multiply(x=w2112, y="T2 alpha_x (nm/V)") -> (x*y=w2103:dbl[])
    n1758 = Multiply(x="T1 alpha_x (nm/V)", y=w2111) -> (x*y=w2102:dbl[])
    n1759 = Multiply(x=w2136, y=w2114) -> (x*y=w2115:waveform(dbl))
    n1760 = case shown="True" "Read Lateness and Rel Phase" {
      tunnel: w1938 -> [w2297 w2319]
      tunnel: w1937 -> [w2298 w2318]
      tunnel: [w2297 w2317] -> w2099
      tunnel: [w2298 w2316] -> w2098
      frame False {
      }
      frame True {
        n1761 = xnode "Read/Write Control"("FPGA VI Reference In"=w2319, "error in"=w2318) -> ("FPGA VI Reference Out"=w2317:T19, "error out"=w2316:errorcluster, "GI Relative phase"=→"GI relative phase":i16, "Relative phase"=→"Relative phase (AI1)":i16, "AI Late Counter"=→"Late Counter (AI1)":u16, "GI Late Counter"=→"GI Late Counter":u16, "MCL Late Counter"=→"MCL Late Counter":u16, "MCL Relative Phase"=→"Relative Phase (MCL)":i16, "APD Acq Relative Phase"=→"APD Acq Relative Phase":i16, "APD 1 Gate Relative Phase"=→"APD 1 Gate Relative Phase":i16, "APD 2 Gate Relative Phase"=→"APD 2 Gate Relative Phase":i16, "APD Acq Late Counter"=→"APD Acq Late Counter":u16, "APD 1 Gate Late Counter"=→"APD 1 Gate Late Counter":u16, "APD 2 Gate Late Counter"=→"APD 2 Gate Late Counter":u16, "Green FB Relative Phase"=→"Relative phase (Green FB)":i16, "GI Relative phase 2"=→"GI relative phase 2":i16, "GI Late Counter 2"=→"GI Late Counter 2":u16, "Trap Pos FIFO Timeout"=→"Trap Pos FIFO Timeout":u16, "Trap AI FIFO Timeout"=→"Trap AI FIFO Timeout":u16)
      }
    }
    n1762 = Subtract(x=w2103, y=w2102) -> (x-y=w2101:dbl[])
    n1763 = Unbundle By Name(w2136) -> ("Y"=w2071:dbl[])
    n1764 = Unbundle By Name(w2137) -> ("Y"=w2072:dbl[])
    n1765 = Build Array(w2137, w2115) -> (→"Force":waveform(dbl)[])
    n1766 = Subtract(x=w2101, y="Offset (nm)") -> (x-y=w2069:dbl[])
    n1767 = call-poly <vilib>:"Mean.vi"("X"=w2071) -> ("mean"=w2050:dbl)  [unwired: 1 out]
    "T2 X" <- w2050
    n1768 = Absolute Value(x=w2072) -> (abs(x)=w2073:dbl[])
    n1769 = Absolute Value(x=w2071) -> (abs(x)=w2074:dbl[])
    n1770 = call-poly <vilib>:"Mean.vi"("X"=w2072) -> ("mean"=w2051:dbl)  [unwired: 1 out]
    "T1 X" <- w2051
    n1771 = Add(x=w2073, y=w2074) -> (x+y=w2075:dbl[])
    n1772 = Bundle By Name(cluster=w2107, "Y"=w2069) -> (w2037:waveform(dbl))
    "Bead Separation" <- w2037
    n1773 = Divide(x=w2075, y=2.0) -> (x/y=→"Vec Mean of T1 T2":dbl[])
    n1774 = case shown="True" w2084 {
      tunnel: w2126 -> [_ w2324]
      tunnel: w2125 -> [_ w2323]
      tunnel: w2124 -> [_ w2322]
      tunnel: w2121 -> [_ w2321]
      tunnel: w2046 -> [_ w2320]
      frame False {
      }
      frame True {
        n1775 = property on="Force" class="WFChart (strict)"("YScale.NameLbl.Text"=w2324) -> ()  [unwired: 2 in, 2 out]
        n1776 = property on="T2 X" class="DigNum (strict)"("Caption.Text"=w2322) -> ()  [unwired: 2 in, 2 out]
        n1777 = property on="T1 X" class="DigNum (strict)"("Caption.Text"=w2323) -> ()  [unwired: 2 in, 2 out]
        n1778 = property on="Mean" class="DigNum (strict)"("Caption.Text"=w2321) -> ()  [unwired: 2 in, 2 out]
        n1779 = property on="Difference" class="DigNum (strict)"("Caption.Text"=w2320) -> ()  [unwired: 2 in, 2 out]
      }
    }
    n1780 = local read "Tether"() -> (w2078:bool)
    n1781 = Absolute Value(x=w2051) -> (abs(x)=w2048:dbl)
    n1782 = Absolute Value(x=w2050) -> (abs(x)=w2047:dbl)
    n1783 = Add(x=w2048, y=w2047) -> (x+y=w2123:dbl)
    n1784 = Subtract(x=w2048, y=w2047) -> (x-y=→"Difference":dbl)
    n1785 = feedback #18(w2069) -> (w2068:dbl[])
    n1786 = Divide(x=w2123, y=2.0) -> (x/y=w2077:dbl)
    "Mean" <- w2077
    n1787 = case shown="True" w2078 {
      tunnel: w2077 -> [_ w2256]
      frame False {
      }
      frame True {
        n1788 = Greater?(x="Lost Tether Alarm Threshold (pN)", y=w2256) -> (0:w2254:bool)
        n1789 = case shown="True" w2254 {
          frame False {
          }
          frame True {
            n1790 = flat-sequence {
              frame #0 {
                # "stop only if saving"
                n1791 = local read "Saving..."() -> (w2269:bool)
                n1792 = And(x=w2269, y="TA Cancel Save?") -> (x .and. y?=w2268:bool)
                n1793 = local write "Stop Saving"(w2268) -> ()
              }
              frame #1 {
                n1794 = case shown="True" "TA Green Off?" {
                  frame False {
                  }
                  frame True {
                    w2272 = FALSE ("Fl. Triggered...")
                    n1795 = local write "Fl. Triggered..."(w2272) -> ()
                    n1796 = property on="Green Laser ON/Interlacing" class="Bool (strict)"("Val(Sgnl)"=w2272) -> ()  [unwired: 2 in, 2 out]
                  }
                }
              }
            }
            n1797 = local read "Time tether formed"() -> (w2263:timestamp)
            n1798 = Get Date/Time In Seconds() -> (seconds since 1Jan1904=w2264:timestamp)
            n1799 = Subtract(x=w2264, y=w2263) -> (x-y=w2262:dbl)
            n1800 = Number To Decimal String(number=w2262) -> (decimal integer string=w2259:string)  [unwired: 1 out]
            n1801 = local read "Messages"() -> (w2266:string)
            n1802 = call <vilib>:"Beep.vi"() -> ()  [unwired: 3 in, 9 out]
            n1803 = Concatenate Strings("Lost tether (" ("Message to add"), w2259, " s)." ("string")) -> (w2261:string)
            n1804 = local write "Tether"(FALSE ("Tether")) -> ()
            n1805 = call "Update messages.vi"("Message to add"=w2261, "Old message string"=w2266) -> ("New message string"=w2265:string)
            n1806 = local write "Messages"(w2265) -> ()
            n1807 = property on="Trap Pos. FB ON" class="Bool (strict)"("Val(Sgnl)"=FALSE ("Value (Signaling)")) -> ()  [unwired: 2 in, 2 out]
          }
        }
      }
    }
    n1808 = Build Array (concatenate)(w2069, w2068) -> (w2067:dbl[])
    n1809 = Split 1D Array(array=w2067, index=w1949) -> (first subarray=w2063:dbl[])  [unwired: 1 out]
    n1810 = feedback-in #18(w2063) -> ()
    n1811 = call-poly <vilib>:"Mean.vi"("X"=w2063) -> ("mean"=w2062:dbl)  [unwired: 1 out]
    "Bead Mean (nm)" <- w2062
    n1812 = Subtract(x=w2063, y=w2062) -> (x-y=w2061:dbl[])
    n1813 = Square(x=w2061) -> (x^2=w2060:dbl[])
    n1814 = call-poly <vilib>:"Mean.vi"("X"=w2060) -> ("mean"=w2059:dbl)  [unwired: 1 out]
    n1815 = Square Root(x=w2059) -> (sqrt(x)=w2058:dbl)
    n1816 = Multiply(x=10.0, y=w2058) -> (x*y=→"RMS (Ang)":dbl)
    n1817 = xnode "Read/Write Control"("FPGA VI Reference In"=w2099, "error in"=w2098) -> ("FPGA VI Reference Out"=w2217:T19, "error out"=w2211:errorcluster, "AI2 Y Sum Set 1"=w2207:i16, "AI2 Y Sum Set 2"=w2206:i16, "AI1 X Set 1"=w1983:fxp<+/-,16,1>, "AI1 X Set 2"=w1982:fxp<+/-,16,1>, "Trap Pos FB Int Signal"=→"Trap Pos FB Int Signal":fxp<+/-,24,9>, "Trap Pos FB Int-Norm Signal"=→"Trap Pos FB Int-Norm Signal":fxp<+/-,16,1>, "Trap Pos FB Action"=w1976:i64, "Scanning"=→"AOD Scanning":bool, "Scan I"=→"AOD Scan I":u64, "Scanning MCL"=w2209:bool, "Scan I (MCL)"=→"MCL Scan I":u64, "Green FB Signals"=w2146:T47)  [unwired: 1 out]
    "MCL Scanning" <- w2209
    "Trap Pos FB Action" <- w1976
    n1818 = local read "AI2 (V)"() -> (w2208:cluster{"Set 1":dbl, "Set 2":dbl})
    n1819 = Bundle By Name(cluster=w2208, "Set 1"=w2207, "Set 2"=w2206) -> (w2204:cluster{"Set 1":dbl, "Set 2":dbl})
    n1820 = Divide(x=w1976, y=327.67) -> (x/y=→"Action (%)":dbl)
    n1821 = local read "Trap X (AI1)"() -> (w1996:T10)
    n1822 = Divide(x=w2204, y=3276.7) -> (x/y=w2203:cluster{"Set 1":dbl, "Set 2":dbl})
    n1823 = local write "AI2 (V)"(w2203) -> ()
    n1824 = Bundle(cluster=w1996, "Trap 1"=w1983, "Trap 2"=w1982) -> (→"Trap X (AI1)":T10)
    n1825 = Divide(x=w2146, y=3276.7) -> (x/y=w2142:T48)
    n1826 = Unbundle By Name(w2142) -> ("Green FB Ch 0"=w2145:dbl, "Green FB Ch 1"=w2144:dbl, "Green FB Ch 2"=w2143:dbl)
    n1827 = Divide(x=w2145, y=w2143) -> (x/y=w2141:dbl)
    n1828 = Divide(x=w2144, y=w2143) -> (x/y=w2140:dbl)
    n1829 = flat-sequence "To save data" {
      tunnel: [w3146] -> w2228
      tunnel: [w3147] -> w2227
      tunnel: w2177 -> [w3140]
      tunnel: w2065 -> [w3144]
      tunnel: ["Save Calibration"] -> w2200
      tunnel: w2197 -> [w3143]
      tunnel: [w3136] -> w2196
      tunnel: [w3133] -> w2195
      tunnel: [w3130] -> w2194
      tunnel: w2176 -> [w3132]
      tunnel: w2082 -> [w3126]
      tunnel: [w3126] -> w2081
      tunnel: ["Start Saving"] -> w2039
      tunnel: [w3120] -> w1965
      tunnel: [w3119] -> w1964
      tunnel: w2228 -> [w3381]
      tunnel: w2227 -> [w3380]
      tunnel: w1966 -> [w3379]
      tunnel: w2200 -> [w3378]
      tunnel: w2196 -> [w3376]
      tunnel: w2195 -> [w3375]
      tunnel: w2194 -> [w3374]
      tunnel: w2052 -> [w3373]
      tunnel: w2091 -> [w3372]
      tunnel: w2081 -> [w3371]
      tunnel: w2039 -> [w3370]
      tunnel: w2037 -> [w3369]
      tunnel: w2013 -> [w3368]
      tunnel: w1965 -> [w3367]
      tunnel: w1964 -> [w3366]
      tunnel: w1963 -> [w3365]
      frame #0 {
        n1830 = Or(x="Save N Sets", y="Start Saving") -> (x .or. y?=w3127:bool)
        n1831 = To Double Precision Float(number=w3143) -> (double precision float=w3137:dbl)
        n1832 = Build Array(w3127, "Save Calibration", w3140, w3132) -> (w3142:bool[])
        n1833 = Compound Arithmetic op=OR("Save Calibration", w3140, w3127, w3132) -> (w3145:bool)
        n1834 = Boolean Array To Number(Boolean array=w3142) -> (number=w3139:u32)
        n1835 = feedback #19(FALSE ("Save APD Data\nwith Trap Data")) -> (w3121:bool)
        n1836 = feedback #20(refnum<k0> refnum) -> (w3148:refnum<file>)
        n1837 = feedback #21(refnum<k0> refnum) -> (w3123:refnum<file>)
        n1838 = feedback #22(FALSE ("Save APD Data\nwith Trap Data")) -> (w3131:bool)
        n1839 = feedback #23(refnum<k0> refnum) -> (w3134:refnum<file>)
        n1840 = feedback #24(0) -> (w3150:i32)
        n1841 = feedback #25() -> (w3138:u32)  [unwired: 1 out]
        n1842 = case shown="True" w3145 {
          tunnel: [w3157 1] -> w3146
          tunnel: w3150 -> [w3159 _]
          tunnel: [w3158 w3177] -> w3147
          tunnel: w3148 -> [w3158 _]
          tunnel: w3144 -> [_ w3197]
          tunnel: w3137 -> [_ w3195]
          tunnel: w3139 -> [_ w3198]
          tunnel: [w3156 w3176] -> w3136
          tunnel: w3138 -> [w3156 _]
          tunnel: [w3155 w3174] -> w3133
          tunnel: w3134 -> [w3155 _]
          tunnel: [w3154 w3173] -> w3130
          tunnel: w3131 -> [w3154 _]
          tunnel: "Start Saving" -> [_ w3171]
          tunnel: w3126 -> [_ w3170]
          tunnel: [w3153 w3161] -> w3119
          tunnel: w3123 -> [w3153 _]
          tunnel: [w3152 w3160] -> w3120
          tunnel: w3121 -> [w3152 _]
          frame False {
            n1843 = Increment(x=w3159) -> (x+1=w3157:i32)
          }
          frame True {
            w3167 = FALSE ("Start Saving")
            w3172 = 9.0  # File Version
            w3180 = FALSE ("prepend array or string size? (T)")
            w3178 = T29."big-endian, network order" ("byte order (0:big-endian, network order)")
            # "write file headers"
            n1844 = local read "BD 1 Frequency 1 (MHz)"() -> (w3194:dbl)
            n1845 = local read "BD 2 Frequency 1 (MHz)"() -> (w3193:dbl)
            n1846 = local read "BD 1 Frequency 2 (MHz)"() -> (w3192:dbl)
            n1847 = local read "BD 2 Frequency 2 (MHz)"() -> (w3191:dbl)
            n1848 = local read "BD 1 Frequency 3 (MHz)"() -> (w3190:dbl)
            n1849 = local read "BD 2 Frequency 3 (MHz)"() -> (w3189:dbl)
            n1850 = Array Size(array=w3170) -> (size(s)=w3169:i32)
            n1851 = To Double Precision Float(number=w3169) -> (double precision float=w3168:dbl)
            n1852 = local write "Save Calibration"(w3167) -> ()
            n1853 = local write "Start Saving"(w3167) -> ()
            n1854 = Build Array("Save APD Data\nwith Trap Data", "Save Trap Pos. Data") -> (w3164:bool[])
            n1855 = Boolean Array To Number(Boolean array=w3164) -> (number=w3163:u32)
            n1856 = Build Array(w3194, w3193, w3192, w3191, w3190, w3189) -> (w3188:dbl[])
            n1857 = case shown="4" w3198 {
              tunnel: w3197 -> [w3269 w3289 w3305 w3343]
              tunnel: w3168 -> [w3274 w3296 w3325 w3362]
              tunnel: w3195 -> [w3273 w3295 w3324 w3361]
              tunnel: [w3270 w3291 w3316 w3353] -> w3186
              tunnel: [w3261 "Cal sets to save" w3306 w3344] -> w3176
              tunnel: w3188 -> [w3271 w3292 w3318 w3355]
              tunnel: "Save APD Data\nwith Trap Data" -> [w3268 _ w3302 w3341]
              tunnel: [w3268 w3283 w3302 w3341] -> w3173
              tunnel: w3172 -> [w3264 w3284 w3300 w3339]
              tunnel: w3171 -> [w3263 _ _ _]
              tunnel: [w3254 w3283 w3299 w3329] -> w3160
              tunnel: "Save Trap Pos. Data" -> [w3254 _ w3299 w3329]
              tunnel: w3163 -> [w3253 _ w3298 w3328]
              frame 1, Default {
                # "timeseries"
                n1858 = case shown="True" "Profile" {
                  tunnel: [w3277 w3280] -> w3258
                  tunnel: [w3277 w3279] -> w3257
                  tunnel: [w3277 w3278] -> w3256
                  tunnel: [w3277 w3282] -> w3255
                  frame False {
                    w3277 = 0.0 ("f")
                  }
                  frame True {
                    n1859 = local read "Current Position"() -> (w3281:dbl[])
                    n1860 = local read "Y change (mm)"() -> (w3282:dbl)
                    n1861 = call "subVI_explode3array.vi"("Array"=w3281) -> ("x"=w3280:dbl, "y"=w3279:dbl, "z"=w3278:dbl)  [unwired: 12 in]
                  }
                }
                n1862 = local read "Save ave N"() -> (w3276:dbl)
                n1863 = Multiply(x=w3276, y=w3269) -> (x*y=w3275:dbl)
                n1864 = To Double Precision Float(number=w3253) -> (double precision float=w3267:dbl)
                n1865 = Build Array(w3264, w3269, w3275, w3274, w3273, 0.0 ("f")) -> (w3272:dbl[])
                n1866 = Build Array(w3267, w3258, w3257, w3256, w3255) -> (w3265:dbl[])
                n1867 = Select(t=u32 4000000000, s=w3263, f="N sets to save") -> (s? t:f=w3261:u32)
                n1868 = Build Array (concatenate)(w3272, w3271, w3265) -> (w3270:dbl[])
              }
              frame 2 {
                w3286 = 0.0 ("f")
                w3283 = FALSE ("Save APD Data\nwith Trap Data")
                # "calibration"
                n1869 = Boolean To (0,1)(Boolean=w3283) -> (0, 1=w3288:i16)
                n1870 = To Double Precision Float(number=w3288) -> (double precision float=w3287:dbl)
                n1871 = Build Array(w3287, w3286, w3286, w3286, w3286) -> (w3285:dbl[])
                n1872 = Build Array(w3284, w3289, w3289, w3296, w3295, 1.0 ("t")) -> (w3293:dbl[])
                n1873 = Build Array (concatenate)(w3293, w3292, w3285) -> (w3291:dbl[])
                "Calibrating Trap..." <- TRUE ("Calibrating...")
              }
              frame 4 {
                w3303 = 0.0 ("f")
                # "write file header for a trap \nraster scan"
                # "scan dir (x/y = 0/1)"
                # "cycles/step"
                # "n scans (f/b)"
                # "steps"
                # "freq. range"
                # "AOD raster scan"
                n1874 = local read "Number of F/B Scans (AOD)"() -> (w3310:u16)
                n1875 = local read "Cycles/step (AOD)"() -> (w3312:u64)
                n1876 = local read "Scan Range (MHz)"() -> (w3315:dbl)
                n1877 = local read "Scan steps (AOD)"() -> (w3314:u64)
                n1878 = local read "Scan BD"() -> (w3322:bool)
                n1879 = local read "Save ave N"() -> (w3327:dbl)
                n1880 = Boolean To (0,1)(Boolean=w3322) -> (0, 1=w3321:i16)
                n1881 = To Double Precision Float(number=w3310) -> (double precision float=w3309:dbl)
                n1882 = To Double Precision Float(number=w3314) -> (double precision float=w3313:dbl)
                n1883 = To Double Precision Float(number=w3312) -> (double precision float=w3311:dbl)
                n1884 = To Double Precision Float(number=w3321) -> (double precision float=w3320:dbl)
                n1885 = Multiply(x=w3327, y=w3305) -> (x*y=w3326:dbl)
                n1886 = To Double Precision Float(number=w3298) -> (double precision float=w3304:dbl)
                n1887 = Build Array(w3304, w3303, w3303, w3303, w3303) -> (w3301:dbl[])
                n1888 = local read "N sets should be saved"() -> (w3307:dbl)
                n1889 = Build Array(w3320, w3315, w3313, w3311, w3309) -> (w3317:dbl[])
                n1890 = Build Array(w3300, w3305, w3326, w3325, w3324, 2.0 ("t")) -> (w3319:dbl[])
                n1891 = Round Toward +Infinity(x=w3307) -> (ceil(x): smallest int >= x=w3308:dbl)
                n1892 = Build Array (concatenate)(w3319, w3318, w3301, w3317) -> (w3316:dbl[])
                n1893 = To Unsigned Long Integer(number=w3308) -> (unsigned 32bit integer=w3306:u32)
              }
              frame 8 {
                w3336 = 0.0 ("f")
                # "MCL raster scan"
                n1894 = local read "Number of scans (MCL)"() -> (w3331:u64)
                n1895 = local read "Scan lines (y)"() -> (w3330:u64)
                n1896 = local read "2D or 1D Scan"() -> (w3333:bool)
                n1897 = local read "Scan Range (V)\n(of steps)"() -> (w3352:dbl)
                n1898 = local read "Fast Scan Dir"() -> (w3359:bool)
                n1899 = local read "Cycles/step (MCL)"() -> (w3349:u64)
                n1900 = local read "Scan steps (MCL)"() -> (w3351:u64)
                n1901 = Select(t=w3330, s=w3333, f=w3331) -> (s? t:f=w3332:u64)
                n1902 = Boolean To (0,1)(Boolean=w3333) -> (0, 1=w3335:i16)
                n1903 = local read "Save ave N"() -> (w3364:dbl)
                n1904 = local read "Initial X"() -> (w3338:dbl)
                n1905 = local read "Initial Y"() -> (w3337:dbl)
                n1906 = To Double Precision Float(number=w3335) -> (double precision float=w3334:dbl)
                n1907 = Boolean To (0,1)(Boolean=w3359) -> (0, 1=w3358:i16)
                n1908 = To Double Precision Float(number=w3332) -> (double precision float=w3347:dbl)
                n1909 = To Double Precision Float(number=w3351) -> (double precision float=w3350:dbl)
                n1910 = To Double Precision Float(number=w3349) -> (double precision float=w3348:dbl)
                n1911 = To Double Precision Float(number=w3358) -> (double precision float=w3357:dbl)
                n1912 = Multiply(x=w3364, y=w3343) -> (x*y=w3363:dbl)
                n1913 = To Double Precision Float(number=w3328) -> (double precision float=w3342:dbl)
                n1914 = local read "N sets should be saved (MCL)"() -> (w3345:dbl)
                n1915 = Build Array(w3342, w3334, w3336, w3336, w3336) -> (w3340:dbl[])
                n1916 = Build Array(w3357, w3352, w3350, w3348, w3347, w3338, w3337) -> (w3354:dbl[])
                n1917 = Build Array(w3339, w3343, w3363, w3362, w3361, 3.0 ("t")) -> (w3356:dbl[])
                n1918 = Round Toward +Infinity(x=w3345) -> (ceil(x): smallest int >= x=w3346:dbl)
                n1919 = Build Array (concatenate)(w3356, w3355, w3340, w3354) -> (w3353:dbl[])
                n1920 = To Unsigned Long Integer(number=w3346) -> (unsigned 32bit integer=w3344:u32)
              }
            }
            n1921 = local read "Index"() -> (w3203:dbl)
            n1922 = call "Create new save file.vi"("Insert"="", "Ext"=".dat", "Index In"=w3203) -> ("Path Out"=w3162:path, "Index Out"=w3175:dbl)
            n1923 = local write "Save file name"(w3162) -> ()
            n1924 = local write "Index"(w3175) -> ()
            n1925 = local write "Save index"(w3175) -> ()
            n1926 = Array Size(array=w3186) -> (size(s)=w3187:i32)
            n1927 = Open/Create/Replace File(file path (use dialog)=w3162, operation (0:open)=T23."create", access (0:read/write)=enum16{"read/write", "read-only", "write-only"}."write-only") -> (refnum out=w3200:refnum<file>)  [unwired: 1 in, 4 out]
            n1928 = local write "Saving..."(TRUE ("Saving...")) -> ()
            n1929 = To Double Precision Float(number=w3187) -> (double precision float=w3185:dbl)
            n1930 = String Length(string="Comment (data description)") -> (length=w3183:i32)
            n1931 = To Double Precision Float(number=w3183) -> (double precision float=w3182:dbl)
            n1932 = Deny Access(7:w3200) -> (3:w3199:refnum<file>)  [unwired: 1 in, 2 out]
            n1933 = Build Array (concatenate)(w3185, w3186, w3182) -> (w3184:dbl[])
            n1934 = case "If fluorescence data to be saved" shown="True" w3173 {
              tunnel: w3162 -> [_ w3252]
              tunnel: [refnum<k0> refnum w3232] -> w3174
              frame False {
              }
              frame True {
                w3231 = 0.0
                n1935 = local read "APD Integration Time (s)"() -> (w3237:dbl)
                n1936 = local read "N APD Samp/step"() -> (w3230:dbl)
                n1937 = Path To String(path=w3252) -> (string=w3251:string)
                n1938 = String Length(string=w3251) -> (length=w3250:i32)
                n1939 = Subtract(x=w3250, y=4) -> (x-y=w3248:i32)
                n1940 = String Subset(string=w3251, length (rest)=w3248) -> (substring=w3247:string)  [unwired: 1 out]
                n1941 = Build Array(w3237, w3230, w3231, w3231, w3231, w3231, w3231, w3231) -> (w3234:dbl[])
                n1942 = Concatenate Strings(w3247, "_fl.dat" ("string")) -> (w3245:string)
                n1943 = Array Size(array=w3234) -> (size(s)=w3236:i32)
                n1944 = String To Path(string=w3245) -> (path=w3241:path)
                n1945 = Open/Create/Replace File(file path (use dialog)=w3241, operation (0:open)=T23."create", access (0:read/write)=enum16{"read/write", "read-only", "write-only"}."write-only") -> (refnum out=w3242:refnum<file>)  [unwired: 1 in, 4 out]
                n1946 = Deny Access(7:w3242) -> (3:w3238:refnum<file>)  [unwired: 1 in, 2 out]
                n1947 = To Double Precision Float(number=w3236) -> (double precision float=w3235:dbl)
                n1948 = Build Array (concatenate)(w3235, w3234) -> (w3233:dbl[])
                n1949 = Write to Binary File(file (use dialog)=w3238, data=w3233, 5:FALSE ("prepend array or string size? (T)"), 9:T29."big-endian, network order" ("byte order (0:big-endian, network order)")) -> (refnum out=w3232:refnum<file>)  [unwired: 1 in, 3 out]
              }
            }
            n1950 = case shown="True" w3160 {
              tunnel: w3162 -> [_ w3214]
              tunnel: [refnum<k0> refnum w3213] -> w3161
              frame False {
              }
              frame True {
                w3209 = 0.0 ("element")
                n1951 = Path To String(path=w3214) -> (string=w3228:string)
                n1952 = Build Array(w3209, w3209, w3209, w3209, w3209, w3209, w3209, w3209) -> (w3210:dbl[])
                n1953 = String Length(string=w3228) -> (length=w3227:i32)
                n1954 = Subtract(x=w3227, y=4) -> (x-y=w3225:i32)
                n1955 = Array Size(array=w3210) -> (size(s)=w3212:i32)
                n1956 = String Subset(string=w3228, length (rest)=w3225) -> (substring=w3224:string)  [unwired: 1 out]
                n1957 = To Double Precision Float(number=w3212) -> (double precision float=w3211:dbl)
                n1958 = Concatenate Strings(w3224, "_pos.dat" ("string")) -> (w3222:string)
                n1959 = Build Array (concatenate)(w3211, w3210) -> (w3208:dbl[])
                n1960 = String To Path(string=w3222) -> (path=w3218:path)
                n1961 = Open/Create/Replace File(file path (use dialog)=w3218, operation (0:open)=T23."create", access (0:read/write)=enum16{"read/write", "read-only", "write-only"}."write-only") -> (refnum out=w3219:refnum<file>)  [unwired: 1 in, 4 out]
                n1962 = Deny Access(7:w3219) -> (3:w3215:refnum<file>)  [unwired: 1 in, 2 out]
                n1963 = Write to Binary File(file (use dialog)=w3215, data=w3208, 5:FALSE ("prepend array or string size? (T)"), 9:T29."big-endian, network order" ("byte order (0:big-endian, network order)")) -> (refnum out=w3213:refnum<file>)  [unwired: 1 in, 3 out]
              }
            }
            n1964 = Write to Binary File(file (use dialog)=w3199, data=w3184, 5:w3180, 9:w3178) -> (refnum out=w3181:refnum<file>)  [unwired: 1 in, 3 out]
            n1965 = Write to Binary File(file (use dialog)=w3181, data="Comment (data description)", 5:w3180, 9:w3178) -> (refnum out=w3177:refnum<file>)  [unwired: 1 in, 3 out]
          }
        }
        n1966 = feedback-in #19(w3120) -> ()
        n1967 = feedback-in #20(w3147) -> ()
        n1968 = feedback-in #21(w3119) -> ()
        n1969 = feedback-in #22(w3130) -> ()
        n1970 = feedback-in #23(w3133) -> ()
        n1971 = feedback-in #24(w3146) -> ()
        n1972 = feedback-in #25(w3136) -> ()
      }
      frame #1 {
        n1973 = local read "Saving..."() -> (w3377:bool)
        n1974 = case shown="True" w3377 {
          tunnel: w3381 -> [_ w3391]
          tunnel: w3380 -> [_ w3405]
          tunnel: w3379 -> [_ w3401]
          tunnel: w3378 -> [_ w3400]
          tunnel: w3376 -> [_ w3399]
          tunnel: w3375 -> [_ w3394]
          tunnel: w3374 -> [_ w3393]
          tunnel: w3373 -> [_ w3392]
          tunnel: w3372 -> [_ w3390]
          tunnel: w3371 -> [_ w3388]
          tunnel: w3370 -> [_ w3387]
          tunnel: w3369 -> [_ w3386]
          tunnel: w3368 -> [_ w3385]
          tunnel: w3367 -> [_ w3384]
          tunnel: w3366 -> [_ w3383]
          tunnel: w3365 -> [_ w3382]
          frame False {
          }
          frame True {
            n1975 = Multiply(x=w3391, y=w3390) -> (x*y=→"Time (s)":dbl)
            n1976 = Less Or Equal?(x=w3391, y=w3399) -> (x <= y?=w3403:bool)
            n1977 = Or(x="Stop Saving", y="Abort save 2") -> (x .or. y?=w3395:bool)
            n1978 = Not(x=w3395) -> (.not. x?=w3404:bool)
            n1979 = And(x=w3403, y=w3404) -> (x .and. y?=w3402:bool)
            n1980 = case shown="False" w3402 {
              tunnel: w3405 -> [w3412 w3480]
              tunnel: [0.0 w3483] -> w3398
              tunnel: w3391 -> [_ w3481]
              tunnel: w3399 -> [_ w3482]
              tunnel: w3401 -> [_ w3477]
              tunnel: w3400 -> [_ _]
              tunnel: w3394 -> [w3410 w3470]
              tunnel: w3393 -> [w3409 w3471]
              tunnel: w3392 -> [_ w3469]
              tunnel: w3388 -> [_ w3468]
              tunnel: w3387 -> [_ w3422]
              tunnel: w3386 -> [_ w3461]
              tunnel: w3385 -> [_ w3439]
              tunnel: w3384 -> [w3407 w3420]
              tunnel: w3383 -> [w3408 w3419]
              tunnel: w3382 -> [_ w3416]
              frame False {
                w3406 = FALSE
                n1981 = Close File(refnum=w3412) -> ()  [unwired: 1 in, 2 out]
                n1982 = case shown="True" w3409 {
                  tunnel: w3410 -> [_ w3414]
                  frame False {
                  }
                  frame True {
                    n1983 = Close File(refnum=w3414) -> ()  [unwired: 1 in, 2 out]
                  }
                }
                n1984 = case shown="True" w3407 {
                  tunnel: w3408 -> [_ w3413]
                  frame False {
                  }
                  frame True {
                    n1985 = Close File(refnum=w3413) -> ()  [unwired: 1 in, 2 out]
                  }
                }
                n1986 = local write "Calibrating Trap..."(w3406) -> ()
                n1987 = call <vilib>:"Beep.vi"() -> ()  [unwired: 3 in, 9 out]
                n1988 = local write "Stop Saving"(w3406) -> ()
                n1989 = property on="Raster Scanning..." class="Bool (strict)"("Val(Sgnl)"=w3406) -> ()  [unwired: 2 in, 2 out]
                "Saving..." <- w3406
              }
              frame True {
                n1990 = local read "Calibrating Trap..."() -> (w3472:bool)
                n1991 = case "Write fl. data" shown="True" w3471 {
                  tunnel: w3470 -> [_ w3506]
                  tunnel: w3469 -> [_ w3505]
                  frame False {
                  }
                  frame True {
                    n1992 = Write to Binary File(file (use dialog)=w3506, data=w3505, 5:FALSE ("prepend array or string size? (T)"), 9:T29."big-endian, network order" ("byte order (0:big-endian, network order)")) -> ()  [unwired: 1 in, 4 out]
                  }
                }
                n1993 = Greater?(x="Save ave N", y=1.0) -> (0:w3475:bool)
                n1994 = Not(x=w3472) -> (.not. x?=w3474:bool)
                n1995 = And(x=w3474, y=w3475) -> (x .and. y?=w3417:bool)
                n1996 = case shown="True" w3417 {
                  tunnel: w3416 -> [w3486 w3497]
                  tunnel: [w3486 w3489] -> w3415
                  tunnel: "Save ave N" -> [_ w3490]
                  frame False {
                  }
                  frame True {
                    w3487 = 2 ("dimension size")
                    n1997 = Array Size(array=w3497) -> (size(s)=w3491:i32)
                    n1998 = Divide(x=w3491, y=w3487) -> (x/y=w3495:dbl)
                    n1999 = Reshape Array(w3497, w3495, w3487) -> (w3496:u64[][])
                    n2000 = Transpose 2D Array(2D array=w3496) -> (transposed array=w3494:u64[][])
                    n2001 = for {
                      tunnel: w3494 -> [w3499] mode=indexing
                      tunnel: [w3498] -> w3488 mode=indexing
                      tunnel: w3490 -> [w3500]
                      workers-P: _ -> [_]
                      n2002 = call "downsample 1D array - U64.vi"("Ave N"=w3500, "Array In"=w3499) -> ("Array Out"=w3498:u64[])  [unwired: 1 in]
                    }
                    n2003 = Transpose 2D Array(2D array=w3488) -> (transposed array=w3493:u64[][])
                    n2004 = Divide(x=w3491, y=w3490) -> (x/y=w3492:dbl)
                    n2005 = Reshape Array(w3493, w3492) -> (w3489:u64[])
                  }
                }
                n2006 = case shown="True" w3417 {
                  tunnel: w3477 -> [w3509 w3521]
                  tunnel: [w3509 w3513] -> w3473
                  tunnel: "Save ave N" -> [_ w3514]
                  tunnel: w3468 -> [_ w3512]
                  frame False {
                    # "don't downsample data for trap calibration"
                  }
                  frame True {
                    n2007 = Array Size(array=w3521) -> (size(s)=w3515:i32)
                    n2008 = Array Size(array=w3512) -> (size(s)=w3511:i32)
                    n2009 = Divide(x=w3515, y=w3511) -> (x/y=w3519:dbl)
                    n2010 = Reshape Array(w3521, w3519, w3511) -> (w3520:i16[][])
                    n2011 = Transpose 2D Array(2D array=w3520) -> (transposed array=w3518:i16[][])
                    n2012 = for {
                      tunnel: w3518 -> [w3524] mode=indexing
                      tunnel: [w3523] -> w3510 mode=indexing
                      tunnel: w3514 -> [w3522]
                      workers-P: _ -> [_]
                      n2013 = call "downsample 1D array - I16.vi"("Ave N"=w3522, "Array In"=w3524) -> ("Array Out"=w3523:i16[])  [unwired: 1 out]
                    }
                    n2014 = Transpose 2D Array(2D array=w3510) -> (transposed array=w3517:i16[][])
                    n2015 = Divide(x=w3515, y=w3514) -> (x/y=w3516:dbl)
                    n2016 = Reshape Array(w3517, w3516) -> (w3513:i16[])
                  }
                }
                n2017 = Index Array(array=w3439, index=1) -> (element=w3442:waveform(dbl))
                n2018 = Index Array(array=w3439, index=0) -> (element=w3444:waveform(dbl))
                n2019 = Unbundle By Name(w3442) -> ("Y"=w3446:dbl[])
                n2020 = Unbundle By Name(w3444) -> ("Y"=w3454:dbl[])
                n2021 = case "Write trap pos. data" shown="True" w3420 {
                  tunnel: w3419 -> [_ w3502]
                  tunnel: w3415 -> [_ w3501]
                  frame False {
                  }
                  frame True {
                    n2022 = Write to Binary File(file (use dialog)=w3502, data=w3501, 5:FALSE ("prepend array or string size? (T)"), 9:T29."big-endian, network order" ("byte order (0:big-endian, network order)")) -> ()  [unwired: 1 in, 4 out]
                  }
                }
                n2023 = Write to Binary File(file (use dialog)=w3480, data=w3473, 5:FALSE ("prepend array or string size? (T)"), 9:T29."big-endian, network order" ("byte order (0:big-endian, network order)")) -> ()  [unwired: 1 in, 4 out]
                n2024 = feedback #26(w3446) -> (w3448:dbl[])
                n2025 = Build Array (concatenate)(w3448, w3446) -> (w3447:dbl[])
                n2026 = Select(t=w3446, s=w3422, f=w3447) -> (s? t:f=w3432:dbl[])
                n2027 = feedback-in #26(w3432) -> ()
                n2028 = feedback #27(w3454) -> (w3467:dbl[])
                n2029 = Build Array (concatenate)(w3467, w3454) -> (w3466:dbl[])
                n2030 = Select(t=w3454, s=w3422, f=w3466) -> (s? t:f=w3441:dbl[])
                n2031 = feedback-in #27(w3441) -> ()
                n2032 = Divide(x=w3481, y=w3482) -> (x/y=w3484:dbl)
                n2033 = Multiply(x=w3484, y=100.0) -> (x*y=w3483:dbl)
                n2034 = Build Array(w3441, w3432) -> (→"Saved APD":dbl[][])
                n2035 = Array Size(array=w3441) -> (size(s)=w3459:i32)
                n2036 = Unbundle By Name(w3461) -> ("Y"=w3465:dbl[])
                n2037 = Subtract(x=w3459, y="N pts to average") -> (x-y=w3435:i32)
                n2038 = Multiply(x="N pts to average", y=u16 2) -> (x*y=w3436:u16)
                n2039 = Subtract(x=w3459, y=w3436) -> (x-y=w3434:i32)
                n2040 = feedback #28(w3465) -> (w3464:dbl[])
                n2041 = Build Array (concatenate)(w3464, w3465) -> (w3463:dbl[])
                n2042 = Select(t=w3465, s=w3422, f=w3463) -> (s? t:f=w3462:dbl[])
                "Trap Delta Graph" <- w3462
                n2043 = feedback-in #28(w3462) -> ()
                n2044 = Array Subset(array=w3441, index=w3435, length="N pts to average") -> (w3458:dbl[])
                n2045 = Array Subset(array=w3441, index=w3434, length="N pts to average") -> (w3457:dbl[])
                n2046 = Array Subset(array=w3432, index=w3435, length="N pts to average") -> (w3438:dbl[])
                n2047 = Array Subset(array=w3432, index=w3434, length="N pts to average") -> (w3437:dbl[])
                n2048 = call-poly <vilib>:"Mean.vi"("X"=w3458) -> ("mean"=w3456:dbl)  [unwired: 1 out]
                n2049 = call-poly <vilib>:"Mean.vi"("X"=w3438) -> ("mean"=w3431:dbl)  [unwired: 1 out]
                n2050 = call-poly <vilib>:"Mean.vi"("X"=w3457) -> ("mean"=w3455:dbl)  [unwired: 1 out]
                n2051 = call-poly <vilib>:"Mean.vi"("X"=w3437) -> ("mean"=w3430:dbl)  [unwired: 1 out]
                n2052 = Subtract(x=w3431, y=w3430) -> (x-y=w3421:dbl)
                "Delta Fl. 2" <- w3421
                n2053 = Subtract(x=w3456, y=w3455) -> (x-y=w3453:dbl)
                "Delta Fl. 1" <- w3453
                n2054 = Initialize Array(w3453, 1 ("dimension size")) -> (w3450:dbl[])
                n2055 = Initialize Array(w3421, 1 ("dimension size")) -> (w3427:dbl[])
                n2056 = feedback #29(w3450) -> (w3451:dbl[])
                n2057 = Build Array (concatenate)(w3451, w3450) -> (w3449:dbl[])
                n2058 = feedback #30(w3427) -> (w3428:dbl[])
                n2059 = Build Array (concatenate)(w3428, w3427) -> (w3426:dbl[])
                n2060 = Select(t=w3450, s=w3422, f=w3449) -> (s? t:f=w3425:dbl[])
                n2061 = feedback-in #29(w3425) -> ()
                n2062 = Select(t=w3427, s=w3422, f=w3426) -> (s? t:f=w3424:dbl[])
                n2063 = feedback-in #30(w3424) -> ()
                n2064 = Build Array(w3425, w3424) -> (→"Save APD Deriv":dbl[][])
              }
            }
            "Progress" <- w3398
            "Progress 2" <- w3398
          }
        }
      }
    }
    n2065 = Bundle By Name(cluster=w2142, "Green FB Ch 0"=w2141, "Green FB Ch 1"=w2140) -> (w2120:T48)
    "Green FB Signals (V)" <- w2120
    n2066 = Unbundle By Name(w2120) -> ("Green FB Ch 2"=→"Green FB Plot":dbl)
    n2067 = local read "wait to reset values"() -> (w2212:bool)
    n2068 = Not(x=w2209) -> (.not. x?=w2213:bool)
    n2069 = And(x=w2213, y=w2212) -> (x .and. y?=w2214:bool)
    n2070 = case "Part of MCL raster scanning: returns to initial positions after scan done" shown="True" w2214 {
      tunnel: w2217 -> [w2950 w2957]
      tunnel: [w2950 w2956] -> w2216
      tunnel: w2211 -> [w2949 w2955]
      tunnel: [w2949 w2954] -> w2210
      frame False {
      }
      frame True {
        w2965 = 10.0 ("y")
        w2964 = 32767.0 ("y")
        # "to return scan values\nafter a synchronous \nAOM scan"
        n2071 = local read "AO2"() -> (w2958:dbl)
        n2072 = local read "AO1"() -> (w2959:dbl)
        n2073 = local write "wait to reset values"(FALSE ("wait to reset values")) -> ()
        n2074 = Multiply(x=w2959, y=w2964) -> (x*y=w2961:dbl)
        n2075 = Multiply(x=w2958, y=w2964) -> (x*y=w2963:dbl)
        n2076 = Divide(x=w2961, y=w2965) -> (x/y=w2960:dbl)
        n2077 = Divide(x=w2963, y=w2965) -> (x/y=w2962:dbl)
        n2078 = To Word Integer(number=w2960) -> (16bit integer=w2966:i16)
        n2079 = To Word Integer(number=w2962) -> (16bit integer=w2967:i16)
        n2080 = local read "Total Counts (ticks)"() -> (w2951:u32)
        n2081 = xnode "Read/Write Control"("FPGA VI Reference In"=w2957, "error in"=w2955, "AO1"=w2966, "AO2"=w2967, "MCL count"=w2951) -> ("FPGA VI Reference Out"=w2956:T19, "error out"=w2954:errorcluster)
        n2082 = local read "Scan Range (V)\n(of steps)"() -> (w2952:dbl)
        n2083 = property on="Scan Range (V)\n(of steps)" class="DigNum (strict)"("Val(Sgnl)"=w2952) -> ()  [unwired: 2 in, 2 out]
      }
    }
    n2084 = node-c288() -> ()  [unwired: 2 out]
  }
  n2085 = node-c288(3 ("Processor")) -> (w74:T24)  [unwired: 3 out]
  n2086 = timed-loop "Oscillate AOD (debugging)" {
    tunnel: w24 -> [w3526]
    tunnel: [w3525] -> w36
    timing: w74 -> [_]
    timing-out: [_] -> w73
    stop <- w3525 stop-if-true
    n2087 = node-c288() -> ()  [unwired: 2 out]
    n2088 = event shown="[0] \"Oscillate Set 2\", \"Fish for Tether\": Value Change" {
      selector: _ -> [_ _ _]
      dyn-events: _ -> [_ _ _]
      timeout: _ -> [_ _ _]
      tunnel: w3526 -> [w3533 _ _]
      tunnel: [FALSE ("Stop All") _ w3801] -> w3525
      event "Oscillate Set 2", "Fish for Tether": Value Change {
        n2089 = event-data() -> ()  [unwired: 6 out]
        n2090 = local read "Oscillate Set 2"() -> (w3532:bool)
        n2091 = Or(x=w3532, y="Fish for Tether") -> (x .or. y?=w3530:bool)
        n2092 = case shown="True" w3530 {
          tunnel: w3533 -> [_ w3536]
          tunnel: "Fish for Tether" -> [_ w3535]
          frame False {
          }
          frame True {
            n2093 = case shown="True" w3535 {
              frame False {
              }
              frame True {
                n2094 = local write "Scan axis 2"(TRUE) -> ()
                n2095 = local write "Tether"(FALSE ("Tether")) -> ()
              }
            }
            n2096 = node-c288("Period") -> (w3538:T24)  [unwired: 3 out]
            n2097 = timed-loop "Oscillate AOD" {
              timing: w3538 -> [_]
              timing-out: [_] -> w3537
              tunnel: w3536 -> [w3548]
              tunnel: w3535 -> [w3547]
              i -> [w3550]
              stop <- w3546 stop-if-true
              n2098 = node-c288() -> (w3549:i64)  [unwired: 1 out]
              n2099 = flat-sequence {
                tunnel: w3550 -> [w3576]
                tunnel: w3549 -> [w3575]
                tunnel: w3548 -> [w3559]
                tunnel: w3547 -> [w3561]
                tunnel: [w3561] -> w3545
                tunnel: [w3560] -> w3544
                tunnel: [w3558] -> w3543
                tunnel: [w3555] -> w3541
                tunnel: w3545 -> [w3612]
                tunnel: w3544 -> [w3610]
                tunnel: w3543 -> [w3609]
                tunnel: [w3608] -> w3542
                tunnel: w3541 -> [w3607]
                tunnel: [w3676] -> w3546
                tunnel: w3542 -> [w3674]
                frame #0 {
                  n2100 = Divide(x=w3575, y=i64 1000) -> (x/y=w3570:dbl)
                  n2101 = Multiply(x=w3570, y=w3576) -> (x*y=w3572:dbl)
                  n2102 = Multiply(x="Osc. freq. (Hz)", y=6.283185307179586) -> (x*y=w3573:dbl)
                  n2103 = Multiply(x=w3573, y=w3572) -> (x*y=w3557:dbl)
                  n2104 = local read "BD 1 Frequency 2 (MHz)"() -> (w3554:dbl)
                  n2105 = local read "BD 1 Frequency 1 (MHz)"() -> (w3551:dbl)
                  n2106 = case shown="True" w3561 {
                    tunnel: w3557 -> [w3582 w3589]
                    tunnel: w3554 -> [_ w3599]
                    tunnel: [w3579 w3583] -> w3562
                    tunnel: [FALSE w3592] -> w3558
                    tunnel: [0.0 w3585] -> w3555
                    tunnel: w3551 -> [_ w3584]
                    frame False {
                      n2107 = Sine(x=w3582) -> (sin(x)=w3580:dbl)
                      n2108 = Multiply(x=w3580, y="Osc. amp. (MHz)") -> (x*y=w3579:dbl)
                    }
                    frame True {
                      n2109 = Cosine(x=w3589) -> (cos(x)=w3602:dbl)
                      n2110 = Subtract(x=w3599, y=w3584) -> (x-y=w3598:dbl)
                      n2111 = Decrement(x=w3602) -> (x-1=w3601:dbl)
                      n2112 = Subtract(x=w3598, y="Closest Delta (MHz)") -> (x-y=w3595:dbl)
                      n2113 = Divide(x=w3601, y=2.0) -> (x/y=w3596:dbl)
                      n2114 = Multiply(x=w3596, y=w3595) -> (x*y=w3583:dbl)
                      n2115 = local read "Vec Mean of T1 T2"() -> (w3591:dbl[])
                      n2116 = Greater?(x=w3591, y="Stop F (pN)") -> (0:w3593:bool[])
                      n2117 = Or Array Elements(Boolean array=w3593) -> (logical OR=w3592:bool)
                      n2118 = Divide(x=w3589, y=6.283185307179586) -> (x/y=w3588:dbl)
                      n2119 = Round Toward +Infinity(x=w3588) -> (ceil(x): smallest int >= x=w3585:dbl)
                      "Attempts" <- w3585
                      n2120 = Greater?(x=w3585, y="Attempt Limit") -> (0:w3587:bool)
                      n2121 = case shown="True" w3587 {
                        frame False {
                        }
                        frame True {
                          n2122 = local write "Fish for Tether"(FALSE ("Fish for Tether")) -> ()
                          n2123 = call <vilib>:"Beep.vi"() -> ()  [unwired: 3 in, 9 out]
                          n2124 = local read "Messages"() -> (w3604:string)
                          n2125 = call "Update messages.vi"("Message to add"="Tether fishing timeout." ("Messages"), "Old message string"=w3604) -> ("New message string"=→"Messages":string)
                        }
                      }
                    }
                  }
                  n2126 = local read "Y RF Frequency Limits (MHz)"() -> (w3563:T16)
                  n2127 = local read "X RF Frequency Limits (MHz)"() -> (w3564:T16)
                  n2128 = local read "BD 1 Frequency 3 (MHz)"() -> (w3569:dbl)
                  n2129 = local read "BD 2 Frequency 2 (MHz)"() -> (w3553:dbl)
                  n2130 = Select(t=w3554, s="Scan axis 2", f=w3553) -> (s? t:f=w3565:dbl)
                  n2131 = Add(x=w3562, y=w3565) -> (x+y=w3560:dbl)
                  n2132 = Select(t=w3560, s="Scan axis 2", f=w3554) -> (s? t:f=w3552:dbl)
                  n2133 = Select(t=w3553, s="Scan axis 2", f=w3560) -> (s? t:f=w3567:dbl)
                  n2134 = local read "BD 2 Frequency 3 (MHz)"() -> (w3568:dbl)
                  n2135 = call "set RF board frequency - interlace.vi"("Board 2 Frequency Limits"=w3563, "Board 1 Frequency Limits"=w3564, "FPGA VI Reference In"=w3559, "Board 2 Frequency 3 (MHz)"=w3568, "Board 1 Frequency 3 (MHz)"=w3569, "Board 2 Frequency 2 (MHz)"=w3553, "Board 2 Frequency 1 (MHz)"=w3567, "Board 1 Frequency 2 (MHz)"=w3552, "Board 1 Frequency 1  (MHz)"=w3551) -> ()  [unwired: 1 in, 2 out]
                }
                frame #1 {
                  n2136 = And(x=w3612, y=w3609) -> (x .and. y?=w3611:bool)
                  n2137 = case "Only if were fishing and now formed tether" shown="True" w3611 {
                    tunnel: w3610 -> [w3614 w3626]
                    tunnel: [w3613 w3625] -> w3608
                    tunnel: w3607 -> [_ w3621]
                    frame False {
                      n2138 = local read "Fish for Tether"() -> (w3613:bool)
                      n2139 = case shown="True" w3613 {
                        tunnel: w3614 -> [_ _]
                        frame False {
                        }
                        frame True {
                        }
                      }
                    }
                    frame True {
                      w3625 = FALSE ("Fish for Tether")
                      n2140 = call <vilib>:"Beep.vi"() -> ()  [unwired: 3 in, 9 out]
                      n2141 = Number To Decimal String(number=w3621, width (-)=i16 1) -> (decimal integer string=w3619:string)
                      n2142 = case shown="\"2\", \"3\", \"4\", \"5\", \"6\"" "Then..." {
                        selector: "Then..." -> [_ w3629]
                        tunnel: w3626 -> [w3628 _]
                        frame "1", Default {
                          # "do nothing"
                          n2143 = property on="BD 1 Frequency 1 (MHz)" class="DigNum (strict)"("Val(Sgnl)"=w3628) -> ()  [unwired: 2 in, 2 out]
                        }
                        frame "2", "3", "4", "5", "6" {
                          n2144 = flat-sequence {
                            tunnel: w3629 -> [w3631]
                            frame #0 {
                              n2145 = property on="Trap Delta (MHz)" class="DigNum (strict)"("Val(Sgnl)"="Move to Delta 1 (MHz)") -> ()  [unwired: 2 in, 2 out]
                            }
                            frame #1 {
                              n2146 = case shown="\"5\", \"6\"" w3631 {
                                selector: w3631 -> [w3634 w3644 _]
                                frame "3", "4" {
                                n2147 = flat-sequence {
                                tunnel: w3634 -> [w3635]
                                tunnel: [w3635] -> w3632
                                tunnel: [w3637] -> w3633
                                tunnel: w3632 -> [w3637]
                                tunnel: w3633 -> [w3641]
                                frame #0 {
                                n2148 = property on="Green Laser ON/Interlacing" class="Bool (strict)"("Val(Sgnl)"=TRUE ("Value (Signaling)")) -> ()  [unwired: 2 in, 2 out]
                                }
                                frame #1 {
                                n2149 = Multiply(x="Wait Before Save (s)", y=u32 1000 ("x")) -> (x*y=w3639:u32)
                                n2150 = Wait (ms)(milliseconds to wait=w3639) -> ()  [unwired: 1 out]
                                }
                                frame #2 {
                                n2151 = property on="Start Saving" class="Bool (strict)"("Value"=TRUE ("Start Saving")) -> ()  [unwired: 2 in, 2 out]
                                n2152 = case shown="Default" w3641 {
                                frame Default {
                                }
                                frame "4" {
                                n2153 = property on="Fl. Triggered..." class="Bool (strict)"("Val(Sgnl)"=TRUE ("Value (Signaling)")) -> ()  [unwired: 2 in, 2 out]
                                }
                                }
                                }
                                }
                                }
                                frame "5", "6" {
                                n2154 = stacked-sequence {
                                tunnel: w3644 -> [_ _ _ _ _ _ _ _ w3661 _ _]
                                frame #0 {
                                n2155 = Replace Array Subset(array=u32[] [0] ("Index Values"), new element="Raster Set Upon Tether", index=0) -> (w3645:u32[])
                                n2156 = property on="Saved AOD Raster Scan Parameter Sets" class="Arr (strict)"("Index Values"=w3645) -> ()  [unwired: 2 in, 2 out]
                                }
                                frame #1 {
                                n2157 = Wait (ms)(milliseconds to wait=u32 500) -> ()  [unwired: 1 out]
                                }
                                frame #2 {
                                n2158 = property on="Load parameters" class="Bool (strict)"("Val(Sgnl)"=TRUE ("Value (Signaling)")) -> ()  [unwired: 2 in, 2 out]
                                }
                                frame #3 {
                                n2159 = Wait (ms)(milliseconds to wait=u32 500) -> ()  [unwired: 1 out]
                                }
                                frame #4 {
                                n2160 = property on="Trap Raster Scan" class="Bool (strict)"("Val(Sgnl)"=TRUE ("Value (Signaling)")) -> ()  [unwired: 2 in, 2 out]
                                }
                                frame #5 {
                                n2161 = Wait (ms)(milliseconds to wait=u32 2000) -> ()  [unwired: 1 out]
                                }
                                frame #6 {
                                n2162 = while {
                                stop <- w3656 stop-if-true
                                n2163 = local read "Raster Scanning..."() -> (w3655:bool)
                                n2164 = local read "Saving..."() -> (w3658:bool)
                                n2165 = Wait (ms)(milliseconds to wait=u32 100) -> ()  [unwired: 1 out]
                                n2166 = Not(x=w3658) -> (.not. x?=w3657:bool)
                                n2167 = Not(x=w3655) -> (.not. x?=w3654:bool)
                                n2168 = And(x=w3657, y=w3654) -> (x .and. y?=w3656:bool)
                                }
                                }
                                frame #7 {
                                n2169 = property on="Trap Delta (MHz)" class="DigNum (strict)"("Val(Sgnl)"="Move to Delta 2 (MHz)") -> ()  [unwired: 2 in, 2 out]
                                }
                                frame #8 {
                                n2170 = local read "Tether"() -> (w3662:bool)
                                n2171 = case shown="True" w3662 {
                                tunnel: w3661 -> [_ w3663]
                                frame False {
                                }
                                frame True {
                                n2172 = flat-sequence {
                                tunnel: w3663 -> [w3665]
                                frame #0 {
                                n2173 = Wait (ms)(milliseconds to wait=u32 500) -> ()  [unwired: 1 out]
                                }
                                frame #1 {
                                n2174 = case shown="\"6\"" w3665 {
                                frame Default {
                                }
                                frame "6" {
                                n2175 = property on="Green Laser ON/Interlacing" class="Bool (strict)"("Val(Sgnl)"=TRUE ("Green Laser ON/Interlacing")) -> ()  [unwired: 2 in, 2 out]
                                }
                                }
                                }
                                frame #2 {
                                n2176 = Wait (ms)(milliseconds to wait=u32 500) -> ()  [unwired: 1 out]
                                }
                                frame #3 {
                                n2177 = local write "Start Saving"("Save at end (5, 6)") -> ()
                                }
                                }
                                }
                                }
                                }
                                frame #9 {
                                n2178 = local read "Bead Sep. Int. Time (s)"() -> (w3671:dbl)
                                n2179 = Multiply(x=w3671, y=1000.0) -> (x*y=w3670:dbl)
                                n2180 = Wait (ms)(milliseconds to wait=w3670) -> ()  [unwired: 1 out]
                                }
                                frame #10 {
                                n2181 = property on="Rescale on Mean" class="Bool (strict)"("Val(Sgnl)"=TRUE ("Value (Signaling)")) -> ()  [unwired: 2 in, 2 out]
                                }
                                }
                                }
                                frame "2", Default {
                                }
                              }
                            }
                          }
                        }
                      }
                      n2182 = Concatenate Strings("Formed tether in ", w3619, " attempt(s)." ("string")) -> (w3616:string)
                      n2183 = local read "Messages"() -> (w3623:string)
                      n2184 = local write "Fish for Tether"(w3625) -> ()
                      n2185 = call "Update messages.vi"("Message to add"=w3616, "Old message string"=w3623) -> ("New message string"=w3622:string)
                      n2186 = local write "Messages"(w3622) -> ()
                      n2187 = Get Date/Time In Seconds() -> (seconds since 1Jan1904=→"Time tether formed":timestamp)
                      "Tether" <- "Tether Alarm?"
                    }
                  }
                }
                frame #2 {
                  n2188 = local read "Oscillate Set 2"() -> (w3675:bool)
                  n2189 = local read "Stop All"() -> (w3677:bool)
                  n2190 = Not Or(1:w3674, 2:w3675) -> (0:w3673:bool)
                  n2191 = Compound Arithmetic op=OR(w3677, w3673) -> (w3676:bool)
                }
              }
              n2192 = node-c288() -> ()  [unwired: 2 out]
            }
            n2193 = node-c288(w3537) -> ()  [unwired: 1 out]
          }
        }
      }
      event "Fl. Triggered...": Value Change {
        n2194 = event-data() -> ()  [unwired: 7 out]
        n2195 = case shown="True" "Fl. Triggered..." {
          frame False {
          }
          frame True {
            n2196 = node-c288() -> (w3689:T24)  [unwired: 4 out]
            n2197 = timed-loop {
              timing: w3689 -> [_]
              timing-out: [_] -> w3688
              tunnel: "Action" -> [w3693]
              shift-right: [w3690] -> _
              shift-left: u8 255 -> [w3692]
              stop <- w3694 stop-if-true
              n2198 = node-c288() -> ()  [unwired: 2 out]
              n2199 = flat-sequence {
                tunnel: w3693 -> [w3706]
                tunnel: w3692 -> [w3703]
                tunnel: [w3702] -> w3691
                tunnel: [w3792] -> w3694
                tunnel: w3691 -> [w3791]
                tunnel: [w3791] -> w3690
                frame #0 {
                  n2200 = local read "Delta Fl. 2"() -> (w3697:dbl)
                  n2201 = local read "Delta Fl. 1"() -> (w3698:dbl)
                  n2202 = Select(t=w3698, s="APD to Watch", f=w3697) -> (s? t:f=w3696:dbl)
                  n2203 = Multiply(x="Fl. Delta Thresh. (kHz)", y=1000.0) -> (x*y=w3705:dbl)
                  n2204 = Greater?(x=w3696, y=w3705) -> (0:w3700:bool)
                  n2205 = Or(x="Force Yank", y=w3700) -> (x .or. y?=w3701:bool)
                  n2206 = case shown="True" w3701 {
                    tunnel: w3706 -> [_ w3716]
                    tunnel: w3703 -> [w3708 w3712]
                    tunnel: [w3708 w3709] -> w3702
                    frame False {
                    }
                    frame True {
                      n2207 = flat-sequence {
                        tunnel: w3713 -> [w3722]
                        tunnel: [w3722] -> w3717
                        tunnel: w3716 -> [w3721]
                        tunnel: [w3721] -> w3715
                        tunnel: [w3720] -> w3714
                        tunnel: w3712 -> [w3719]
                        tunnel: [w3718] -> w3711
                        tunnel: w3717 -> [w3747]
                        tunnel: w3715 -> [w3746]
                        tunnel: w3714 -> [w3745]
                        tunnel: w3711 -> [w3744]
                        tunnel: [w3744] -> w3710
                        tunnel: w3710 -> [w3789]
                        tunnel: [w3789] -> w3709
                        frame #0 {
                          n2208 = call <vilib>:"Beep.vi"() -> ()  [unwired: 3 in, 9 out]
                          n2209 = local write "Waiting"(FALSE ("Waiting")) -> ()
                          n2210 = Increment(x=w3719) -> (x+1=w3718:u8)
                          n2211 = case shown="\"Yank\"" w3721 {
                            tunnel: w3718 -> [_ _ w3728]
                            frame "Image" {
                              n2212 = property on="Confocal Image" class="Bool (strict)"("Val(Sgnl)"=TRUE ("Value (Signaling)")) -> ()  [unwired: 2 in, 2 out]
                            }
                            frame "Alarm", Default {
                            }
                            frame "Yank" {
                              n2213 = flat-sequence {
                                tunnel: w3728 -> [w3731]
                                tunnel: [w3730] -> w3727
                                tunnel: ["N Array El"] -> w3726
                                tunnel: w3727 -> [w3741]
                                tunnel: w3726 -> [w3737]
                                frame #0 {
                                n2214 = Multiply(x="Yank Delay (s)", y=1000.0) -> (x*y=w3734:dbl)
                                n2215 = Quotient & Remainder(x=w3731, y="N Array El") -> (x-y*floor(x/y)=w3730:u8)  [unwired: 1 out]
                                n2216 = Wait (ms)(milliseconds to wait=w3734) -> ()  [unwired: 1 out]
                                }
                                frame #1 {
                                n2217 = Random Number (0-1)() -> (number: 0 to 1=w3738:dbl)
                                n2218 = Multiply(x=w3737, y=w3738) -> (x*y=w3736:dbl)
                                n2219 = Round Toward -Infinity(1:w3736) -> (0:w3735:dbl)
                                n2220 = Select(t=w3735, s="Random Choice", f=w3741) -> (s? t:f=w3739:dbl)
                                n2221 = Index Array(array="Yank to Delta Array (MHz)", index=w3739) -> (element=w3742:dbl)
                                n2222 = property on="Trap Delta (MHz)" class="DigNum (strict)"("Val(Sgnl)"=w3742) -> ()  [unwired: 2 in, 2 out]
                                }
                              }
                            }
                          }
                          n2223 = local read "Time (s)"() -> (w3720:dbl)
                          "Fl. High" <- TRUE ("Yanking")
                        }
                        frame #1 {
                          n2224 = node-c288() -> (w3749:T24)  [unwired: 4 out]
                          n2225 = timed-loop {
                            timing: w3749 -> [_]
                            timing-out: [_] -> w3748
                            tunnel: w3747 -> [w3765]
                            tunnel: w3746 -> [w3763]
                            tunnel: w3745 -> [w3762]
                            stop <- w3764 stop-if-true
                            n2226 = node-c288() -> ()  [unwired: 2 out]
                            n2227 = local read "Fl. Delta Thresh. (kHz)"() -> (w3757:dbl)
                            n2228 = local read "Fl. Triggered..."() -> (w3766:bool)
                            n2229 = local read "Delta Fl. 1"() -> (w3753:dbl)
                            n2230 = local read "Delta Fl. 2"() -> (w3751:dbl)
                            n2231 = local read "Stop All"() -> (w3760:bool)
                            n2232 = local read "APD to Watch"() -> (w3752:bool)
                            n2233 = Select(t=w3753, s=w3752, f=w3751) -> (s? t:f=w3750:dbl)
                            n2234 = Not(x=w3766) -> (.not. x?=w3761:bool)
                            n2235 = Multiply(x=w3757, y=1000.0) -> (x*y=w3756:dbl)
                            n2236 = Negate(x=w3756) -> (-x=w3755:dbl)
                            n2237 = Less?(x=w3750, y=w3755) -> (x < y?=w3759:bool)
                            n2238 = Compound Arithmetic op=OR(w3759, w3760, w3761, "Force Reset") -> (w3764:bool)
                            n2239 = case shown="True" w3764 {
                              tunnel: w3765 -> [_ w3777]
                              tunnel: w3763 -> [_ w3776]
                              tunnel: w3762 -> [_ w3774]
                              frame False {
                              }
                              frame True {
                                n2240 = case shown="\"Yank\"" w3776 {
                                tunnel: w3777 -> [_ w3778]
                                frame "Image", Default {
                                }
                                frame "Yank" {
                                n2241 = flat-sequence {
                                tunnel: [w3783] -> w3779
                                tunnel: w3778 -> [w3783]
                                tunnel: w3779 -> [w3784]
                                frame #0 {
                                n2242 = local read "Yank Delay (s)"() -> (w3782:dbl)
                                n2243 = Multiply(x=w3782, y=1000.0) -> (x*y=w3780:dbl)
                                n2244 = Wait (ms)(milliseconds to wait=w3780) -> ()  [unwired: 1 out]
                                }
                                frame #1 {
                                n2245 = property on="Trap Delta (MHz)" class="DigNum (strict)"("Val(Sgnl)"=w3784) -> ()  [unwired: 2 in, 2 out]
                                }
                                }
                                }
                                }
                                n2246 = local read "Time (s)"() -> (w3775:dbl)
                                n2247 = Subtract(x=w3775, y=w3774) -> (x-y=w3771:dbl)
                                "Duration (s)" <- w3771
                                n2248 = Number To Decimal String(number=w3771, width (-)=i16 0) -> (decimal integer string=w3769:string)
                                n2249 = Concatenate Strings(w3769, " s fluorescence event." ("string")) -> (w3767:string)
                                n2250 = local read "Messages"() -> (w3773:string)
                                n2251 = call "Update messages.vi"("Message to add"=w3767, "Old message string"=w3773) -> ("New message string"=w3772:string)
                                n2252 = call <vilib>:"Beep.vi"() -> ()  [unwired: 3 in, 9 out]
                                n2253 = local write "Messages"(w3772) -> ()
                              }
                            }
                            n2254 = node-c288() -> ()  [unwired: 2 out]
                          }
                          n2255 = node-c288(w3748) -> ()  [unwired: 1 out]
                        }
                        frame #2 {
                          n2256 = local write "Fl. High"(FALSE ("Yanking")) -> ()
                        }
                      }
                      n2257 = local read "Trap Delta (MHz)"() -> (w3713:dbl)
                    }
                  }
                }
                frame #1 {
                  n2258 = local read "Stop All"() -> (w3795:bool)
                  n2259 = local read "Fl. Triggered..."() -> (w3793:bool)
                  n2260 = Not(x=w3793) -> (.not. x?=w3794:bool)
                  n2261 = Or(x=w3794, y=w3795) -> (x .or. y?=w3792:bool)
                  n2262 = Not(x=w3792) -> (.not. x?=→"Waiting":bool)
                }
              }
              n2263 = node-c288() -> ()  [unwired: 2 out]
            }
            n2264 = node-c288(w3688) -> ()  [unwired: 1 out]
          }
        }
      }
      event "Stop All": Value Change {
        n2265 = event-data() -> ()  [unwired: 7 out]
        n2266 = local read "Stop All"() -> (w3801:bool)
      }
    }
    n2267 = node-c288() -> ()  [unwired: 2 out]
  }
  n2268 = node-c288(w14) -> ()  [unwired: 1 out]
  n2269 = node-c288(w68) -> ()  [unwired: 1 out]
  n2270 = node-c288(w75) -> ()  [unwired: 1 out]
  n2271 = node-c288(w73) -> ()  [unwired: 1 out]
  n2272 = node-c288(w163) -> ()  [unwired: 1 out]
  n2273 = flat-sequence {
    tunnel: w33 -> [w3806]
    tunnel: [w3805] -> w39
    tunnel: [w3802] -> w38
    tunnel: w37 -> [_]
    tunnel: w36 -> [_]
    tunnel: w35 -> [_]
    tunnel: w34 -> [_]
    tunnel: w32 -> [w3803]
    tunnel: w39 -> [w3809]
    tunnel: w38 -> [w3808]
    frame #0 {
      w3804 = FALSE ("APD to FIFO")
      n2274 = xnode "Read/Write Control"("FPGA VI Reference In"=w3806, "error in"=w3803, "APD to FIFO"=w3804, "AI to FIFO"=w3804) -> ("FPGA VI Reference Out"=w3805:T19, "error out"=w3802:errorcluster)
    }
    frame #1 {
      n2275 = xnode "Invoke Method"("FPGA VI Reference In"=w3809, "error in"=w3808) -> ("FPGA VI Reference Out"=w3807:T19)  [unwired: 1 out]
      n2276 = xnode "Close FPGA VI Reference"("FPGA VI Reference In"=w3807) -> ()  [unwired: 1 in, 1 out]
    }
  }
